vi "LoadImage_Names.vi"(8 "First Image":i32=2098, 9 "Load in PCO Format":bool, 11 "Sample Image":path=path "C:/Analysis_from_Movie_for_RiboTrap_Dieter/Movie_Data_Lorenz/TPA-3rdplasmidconc1to1/tea4s15w_0_003565.tif") -> (0 "Image Filenames":string[](array[string])=["C:\\Analysis_from_Movie_for_RiboTrap_Dieter\\Movie_Data_Lorenz\\TPA-3rdplasmidconc1to1\\tea4s15w_0_002099.tif", "C:\\Analysis_from_Movie_for_RiboTrap_Dieter\\Movie_Data_Lorenz\\TPA-3rdplasmidconc1to1\\tea4s15w_0_002100.tif", "C:\\Analysis_from_Movie_for_RiboTrap_Dieter\\Movie_Data_Lorenz\\TPA-3rdplasmidconc1to1\\tea4s15w_0_002101.tif", "C:\\Analysis_from_Movie_for_RiboTrap_Dieter\\Movie_Data_Lorenz\\TPA-3rdplasmidconc1to1\\tea4s15w_0_002102.tif", "C:\\Analysis_from_Movie_for_RiboTrap_Dieter\\Movie_Data_Lorenz\\TPA-3rdplasmidconc1to1\\tea4s15w_0_002103.tif", "C:\\Analysis_from_Movie_for_RiboTrap_Dieter\\Movie_Data_Lorenz\\TPA-3rdplasmidconc1to1\\tea4s15w_0_002104.tif", "C:\\Analysis_from_Movie_for_RiboTrap_Dieter\\Movie_Data_Lorenz\\TPA-3rdplasmidconc1to1\\tea4s15w_0_002105.tif", "C:\\Analysis_from_Movie_for_RiboTrap_Dieter\\Movie_Data_Lorenz\\TPA-3rdplasmidconc1to1\\tea4s15w_0_002106.tif", "C:\\Analysis_from_Movie_for_RiboTrap_Dieter\\Movie_Data_Lorenz\\TPA-3rdplasmidconc1to1\\tea4s15w_0_002107.tif", "C:\\Analysis_from_Movie_for_RiboTrap_Dieter\\Movie_Data_Lorenz\\TPA-3rdplasmidconc1to1\\tea4s15w_0_002108.tif", "C:\\Analysis_from_Movie_for_RiboTrap_Dieter\\Movie_Data_Lorenz\\TPA-3rdplasmidconc1to1\\tea4s15w_0_002109.tif", "C:\\Analysis_from_Movie_for_RiboTrap_Dieter\\Movie_Data_Lorenz\\TPA-3rdplasmidconc1to1\\tea4s15w_0_002110.tif", "C:\\Analysis_from_Movie_for_RiboTrap_Dieter\\Movie_Data_Lorenz\\TPA-3rdplasmidconc1to1\\tea4s15w_0_002111.tif", "C:\\Analysis_from_Movie_for_RiboTrap_Dieter\\Movie_Data_Lorenz\\TPA-3rdplasmidconc1to1\\tea4s15w_0_002112.tif", "C:\\Analysis_from_Movie_for_RiboTrap_Dieter\\Movie_Data_Lorenz\\TPA-3rdplasmidconc1to1\\tea4s15w_0_002113.tif", "C:\\Analysis_from_Movie_for_RiboTrap_Dieter\\Movie_Data_Lorenz\\TPA-3rdplasmidconc1to1\\tea4s15w_0_002114.tif", "C:\\Analysis_from_Movie_for_RiboTrap_Dieter\\Movie_Data_Lorenz\\TPA-3rdplasmidconc1to1\\tea4s15w_0_002115.tif", "C:\\Analysis_from_Movie_for_RiboTrap_Dieter\\Movie_Data_Lorenz\\TPA-3rdplasmidconc1to1\\tea4s15w_0_002116.tif", "C:\\Analysis_from_Movie_for_RiboTrap_Dieter\\Movie_Data_Lorenz\\TPA-3rdplasmidconc1to1\\tea4s15w_0_002117.tif", "C:\\Analysis_from_Movie_for_RiboTrap_Dieter\\Movie_Data_Lorenz\\TPA-3rdplasmidconc1to1\\tea4s15w_0_002118.tif", "C:\\Analysis_from_Movie_for_RiboTrap_Dieter\\Movie_Data_Lorenz\\TPA-3rdplasmidconc1to1\\tea4s15w_0_002119.tif", "C:\\Analysis_from_Movie_for_RiboTrap_Dieter\\Movie_Data_Lorenz\\TPA-3rdplasmidconc1to1\\tea4s15w_0_002120.tif", "C:\\Analysis_from_Movie_for_RiboTrap_Dieter\\Movie_Data_Lorenz\\TPA-3rdplasmidconc1to1\\tea4s15w_0_002121.tif", "C:\\Analysis_from_Movie_for_RiboTrap_Dieter\\Movie_Data_Lorenz\\TPA-3rdplasmidconc1to1\\tea4s15w_0_002122.tif", "C:\\Analysis_from_Movie_for_RiboTrap_Dieter\\Movie_Data_Lorenz\\TPA-3rdplasmidconc1to1\\tea4s15w_0_002123.tif", "C:\\Analysis_from_Movie_for_RiboTrap_Dieter\\Movie_Data_Lorenz\\TPA-3rdplasmidconc1to1\\tea4s15w_0_002124.tif", "C:\\Analysis_from_Movie_for_RiboTrap_Dieter\\Movie_Data_Lorenz\\TPA-3rdplasmidconc1to1\\tea4s15w_0_002125.tif", "C:\\Analysis_from_Movie_for_RiboTrap_Dieter\\Movie_Data_Lorenz\\TPA-3rdplasmidconc1to1\\tea4s15w_0_002126.tif", "C:\\Analysis_from_Movie_for_RiboTrap_Dieter\\Movie_Data_Lorenz\\TPA-3rdplasmidconc1to1\\tea4s15w_0_002127.tif", "C:\\Analysis_from_Movie_for_RiboTrap_Dieter\\Movie_Data_Lorenz\\TPA-3rdplasmidconc1to1\\tea4s15w_0_002128.tif", "C:\\Analysis_from_Movie_for_RiboTrap_Dieter\\Movie_Data_Lorenz\\TPA-3rdplasmidconc1to1\\tea4s15w_0_002129.tif", "C:\\Analysis_from_Movie_for_RiboTrap_Dieter\\Movie_Data_Lorenz\\TPA-3rdplasmidconc1to1\\tea4s15w_0_002130.tif", "C:\\Analysis_from_Movie_for_RiboTrap_Dieter\\Movie_Data_Lorenz\\TPA-3rdplasmidconc1to1\\tea4s15w_0_002131.tif", "C:\\Analysis_from_Movie_for_RiboTrap_Dieter\\Movie_Data_Lorenz\\TPA-3rdplasmidconc1to1\\tea4s15w_0_002132.tif", "C:\\Analysis_from_Movie_for_RiboTrap_Dieter\\Movie_Data_Lorenz\\TPA-3rdplasmidconc1to1\\tea4s15w_0_002133.tif", "C:\\Analysis_from_Movie_for_RiboTrap_Dieter\\Movie_Data_Lorenz\\TPA-3rdplasmidconc1to1\\tea4s15w_0_002134.tif", "C:\\Analysis_from_Movie_for_RiboTrap_Dieter\\Movie_Data_Lorenz\\TPA-3rdplasmidconc1to1\\tea4s15w_0_002135.tif", "C:\\Analysis_from_Movie_for_RiboTrap_Dieter\\Movie_Data_Lorenz\\TPA-3rdplasmidconc1to1\\tea4s15w_0_002136.tif", "C:\\Analysis_from_Movie_for_RiboTrap_Dieter\\Movie_Data_Lorenz\\TPA-3rdplasmidconc1to1\\tea4s15w_0_002137.tif", "C:\\Analysis_from_Movie_for_RiboTrap_Dieter\\Movie_Data_Lorenz\\TPA-3rdplasmidconc1to1\\tea4s15w_0_002138.tif", "C:\\Analysis_from_Movie_for_RiboTrap_Dieter\\Movie_Data_Lorenz\\TPA-3rdplasmidconc1to1\\tea4s15w_0_002139.tif", "C:\\Analysis_from_Movie_for_RiboTrap_Dieter\\Movie_Data_Lorenz\\TPA-3rdplasmidconc1to1\\tea4s15w_0_002140.tif", "C:\\Analysis_from_Movie_for_RiboTrap_Dieter\\Movie_Data_Lorenz\\TPA-3rdplasmidconc1to1\\tea4s15w_0_002141.tif", "C:\\Analysis_from_Movie_for_RiboTrap_Dieter\\Movie_Data_Lorenz\\TPA-3rdplasmidconc1to1\\tea4s15w_0_002142.tif", "C:\\Analysis_from_Movie_for_RiboTrap_Dieter\\Movie_Data_Lorenz\\TPA-3rdplasmidconc1to1\\tea4s15w_0_002143.tif", "C:\\Analysis_from_Movie_for_RiboTrap_Dieter\\Movie_Data_Lorenz\\TPA-3rdplasmidconc1to1\\tea4s15w_0_002144.tif", "C:\\Analysis_from_Movie_for_RiboTrap_Dieter\\Movie_Data_Lorenz\\TPA-3rdplasmidconc1to1\\tea4s15w_0_002145.tif", "C:\\Analysis_from_Movie_for_RiboTrap_Dieter\\Movie_Data_Lorenz\\TPA-3rdplasmidconc1to1\\tea4s15w_0_002146.tif", "C:\\Analysis_from_Movie_for_RiboTrap_Dieter\\Movie_Data_Lorenz\\TPA-3rdplasmidconc1to1\\tea4s15w_0_002147.tif", "C:\\Analysis_from_Movie_for_RiboTrap_Dieter\\Movie_Data_Lorenz\\TPA-3rdplasmidconc1to1\\tea4s15w_0_002148.tif", "C:\\Analysis_from_Movie_for_RiboTrap_Dieter\\Movie_Data_Lorenz\\TPA-3rdplasmidconc1to1\\tea4s15w_0_002149.tif", "C:\\Analysis_from_Movie_for_RiboTrap_Dieter\\Movie_Data_Lorenz\\TPA-3rdplasmidconc1to1\\tea4s15w_0_002150.tif", "C:\\Analysis_from_Movie_for_RiboTrap_Dieter\\Movie_Data_Lorenz\\TPA-3rdplasmidconc1to1\\tea4s15w_0_002151.tif", "C:\\Analysis_from_Movie_for_RiboTrap_Dieter\\Movie_Data_Lorenz\\TPA-3rdplasmidconc1to1\\tea4s15w_0_002152.tif", "C:\\Analysis_from_Movie_for_RiboTrap_Dieter\\Movie_Data_Lorenz\\TPA-3rdplasmidconc1to1\\tea4s15w_0_002153.tif", "C:\\Analysis_from_Movie_for_RiboTrap_Dieter\\Movie_Data_Lorenz\\TPA-3rdplasmidconc1to1\\tea4s15w_0_002154.tif", "C:\\Analysis_from_Movie_for_RiboTrap_Dieter\\Movie_Data_Lorenz\\TPA-3rdplasmidconc1to1\\tea4s15w_0_002155.tif", "C:\\Analysis_from_Movie_for_RiboTrap_Dieter\\Movie_Data_Lorenz\\TPA-3rdplasmidconc1to1\\tea4s15w_0_002156.tif", "C:\\Analysis_from_Movie_for_RiboTrap_Dieter\\Movie_Data_Lorenz\\TPA-3rdplasmidconc1to1\\tea4s15w_0_002157.tif", "C:\\Analysis_from_Movie_for_RiboTrap_Dieter\\Movie_Data_Lorenz\\TPA-3rdplasmidconc1to1\\tea4s15w_0_002158.tif", "C:\\Analysis_from_Movie_for_RiboTrap_Dieter\\Movie_Data_Lorenz\\TPA-3rdplasmidconc1to1\\tea4s15w_0_002159.tif", "C:\\Analysis_from_Movie_for_RiboTrap_Dieter\\Movie_Data_Lorenz\\TPA-3rdplasmidconc1to1\\tea4s15w_0_002160.tif", "C:\\Analysis_from_Movie_for_RiboTrap_Dieter\\Movie_Data_Lorenz\\TPA-3rdplasmidconc1to1\\tea4s15w_0_002161.tif", "C:\\Analysis_from_Movie_for_RiboTrap_Dieter\\Movie_Data_Lorenz\\TPA-3rdplasmidconc1to1\\tea4s15w_0_002162.tif", "C:\\Analysis_from_Movie_for_RiboTrap_Dieter\\Movie_Data_Lorenz\\TPA-3rdplasmidconc1to1\\tea4s15w_0_002163.tif", "C:\\Analysis_from_Movie_for_RiboTrap_Dieter\\Movie_Data_Lorenz\\TPA-3rdplasmidconc1to1\\tea4s15w_0_002164.tif", "C:\\Analysis_from_Movie_for_RiboTrap_Dieter\\Movie_Data_Lorenz\\TPA-3rdplasmidconc1to1\\tea4s15w_0_002165.tif", "C:\\Analysis_from_Movie_for_RiboTrap_Dieter\\Movie_Data_Lorenz\\TPA-3rdplasmidconc1to1\\tea4s15w_0_002166.tif", "C:\\Analysis_from_Movie_for_RiboTrap_Dieter\\Movie_Data_Lorenz\\TPA-3rdplasmidconc1to1\\tea4s15w_0_002167.tif", "C:\\Analysis_from_Movie_for_RiboTrap_Dieter\\Movie_Data_Lorenz\\TPA-3rdplasmidconc1to1\\tea4s15w_0_002168.tif", "C:\\Analysis_from_Movie_for_RiboTrap_Dieter\\Movie_Data_Lorenz\\TPA-3rdplasmidconc1to1\\tea4s15w_0_002169.tif", "C:\\Analysis_from_Movie_for_RiboTrap_Dieter\\Movie_Data_Lorenz\\TPA-3rdplasmidconc1to1\\tea4s15w_0_002170.tif", "C:\\Analysis_from_Movie_for_RiboTrap_Dieter\\Movie_Data_Lorenz\\TPA-3rdplasmidconc1to1\\tea4s15w_0_002171.tif", "C:\\Analysis_from_Movie_for_RiboTrap_Dieter\\Movie_Data_Lorenz\\TPA-3rdplasmidconc1to1\\tea4s15w_0_002172.tif", "C:\\Analysis_from_Movie_for_RiboTrap_Dieter\\Movie_Data_Lorenz\\TPA-3rdplasmidconc1to1\\tea4s15w_0_002173.tif", "C:\\Analysis_from_Movie_for_RiboTrap_Dieter\\Movie_Data_Lorenz\\TPA-3rdplasmidconc1to1\\tea4s15w_0_002174.tif", "C:\\Analysis_from_Movie_for_RiboTrap_Dieter\\Movie_Data_Lorenz\\TPA-3rdplasmidconc1to1\\tea4s15w_0_002175.tif", "C:\\Analysis_from_Movie_for_RiboTrap_Dieter\\Movie_Data_Lorenz\\TPA-3rdplasmidconc1to1\\tea4s15w_0_002176.tif", "C:\\Analysis_from_Movie_for_RiboTrap_Dieter\\Movie_Data_Lorenz\\TPA-3rdplasmidconc1to1\\tea4s15w_0_002177.tif", "C:\\Analysis_from_Movie_for_RiboTrap_Dieter\\Movie_Data_Lorenz\\TPA-3rdplasmidconc1to1\\tea4s15w_0_002178.tif", "C:\\Analysis_from_Movie_for_RiboTrap_Dieter\\Movie_Data_Lorenz\\TPA-3rdplasmidconc1to1\\tea4s15w_0_002179.tif", "C:\\Analysis_from_Movie_for_RiboTrap_Dieter\\Movie_Data_Lorenz\\TPA-3rdplasmidconc1to1\\tea4s15w_0_002180.tif", "C:\\Analysis_from_Movie_for_RiboTrap_Dieter\\Movie_Data_Lorenz\\TPA-3rdplasmidconc1to1\\tea4s15w_0_002181.tif", "C:\\Analysis_from_Movie_for_RiboTrap_Dieter\\Movie_Data_Lorenz\\TPA-3rdplasmidconc1to1\\tea4s15w_0_002182.tif", "C:\\Analysis_from_Movie_for_RiboTrap_Dieter\\Movie_Data_Lorenz\\TPA-3rdplasmidconc1to1\\tea4s15w_0_002183.tif", "C:\\Analysis_from_Movie_for_RiboTrap_Dieter\\Movie_Data_Lorenz\\TPA-3rdplasmidconc1to1\\tea4s15w_0_002184.tif", "C:\\Analysis_from_Movie_for_RiboTrap_Dieter\\Movie_Data_Lorenz\\TPA-3rdplasmidconc1to1\\tea4s15w_0_002185.tif", "C:\\Analysis_from_Movie_for_RiboTrap_Dieter\\Movie_Data_Lorenz\\TPA-3rdplasmidconc1to1\\tea4s15w_0_002186.tif", "C:\\Analysis_from_Movie_for_RiboTrap_Dieter\\Movie_Data_Lorenz\\TPA-3rdplasmidconc1to1\\tea4s15w_0_002187.tif", "C:\\Analysis_from_Movie_for_RiboTrap_Dieter\\Movie_Data_Lorenz\\TPA-3rdplasmidconc1to1\\tea4s15w_0_002188.tif", "C:\\Analysis_from_Movie_for_RiboTrap_Dieter\\Movie_Data_Lorenz\\TPA-3rdplasmidconc1to1\\tea4s15w_0_002189.tif", "C:\\Analysis_from_Movie_for_RiboTrap_Dieter\\Movie_Data_Lorenz\\TPA-3rdplasmidconc1to1\\tea4s15w_0_002190.tif", "C:\\Analysis_from_Movie_for_RiboTrap_Dieter\\Movie_Data_Lorenz\\TPA-3rdplasmidconc1to1\\tea4s15w_0_002191.tif", "C:\\Analysis_from_Movie_for_RiboTrap_Dieter\\Movie_Data_Lorenz\\TPA-3rdplasmidconc1to1\\tea4s15w_0_002192.tif", "C:\\Analysis_from_Movie_for_RiboTrap_Dieter\\Movie_Data_Lorenz\\TPA-3rdplasmidconc1to1\\tea4s15w_0_002193.tif", "C:\\Analysis_from_Movie_for_RiboTrap_Dieter\\Movie_Data_Lorenz\\TPA-3rdplasmidconc1to1\\tea4s15w_0_002194.tif", "C:\\Analysis_from_Movie_for_RiboTrap_Dieter\\Movie_Data_Lorenz\\TPA-3rdplasmidconc1to1\\tea4s15w_0_002195.tif", "C:\\Analysis_from_Movie_for_RiboTrap_Dieter\\Movie_Data_Lorenz\\TPA-3rdplasmidconc1to1\\tea4s15w_0_002196.tif", "C:\\Analysis_from_Movie_for_RiboTrap_Dieter\\Movie_Data_Lorenz\\TPA-3rdplasmidconc1to1\\tea4s15w_0_002197.tif", "C:\\Analysis_from_Movie_for_RiboTrap_Dieter\\Movie_Data_Lorenz\\TPA-3rdplasmidconc1to1\\tea4s15w_0_002198.tif", "C:\\Analysis_from_Movie_for_RiboTrap_Dieter\\Movie_Data_Lorenz\\TPA-3rdplasmidconc1to1\\tea4s15w_0_002199.tif", "C:\\Analysis_from_Movie_for_RiboTrap_Dieter\\Movie_Data_Lorenz\\TPA-3rdplasmidconc1to1\\tea4s15w_0_002200.tif", "C:\\Analysis_from_Movie_for_RiboTrap_Dieter\\Movie_Data_Lorenz\\TPA-3rdplasmidconc1to1\\tea4s15w_0_002201.tif", "C:\\Analysis_from_Movie_for_RiboTrap_Dieter\\Movie_Data_Lorenz\\TPA-3rdplasmidconc1to1\\tea4s15w_0_002202.tif", "C:\\Analysis_from_Movie_for_RiboTrap_Dieter\\Movie_Data_Lorenz\\TPA-3rdplasmidconc1to1\\tea4s15w_0_002203.tif", "C:\\Analysis_from_Movie_for_RiboTrap_Dieter\\Movie_Data_Lorenz\\TPA-3rdplasmidconc1to1\\tea4s15w_0_002204.tif", "C:\\Analysis_from_Movie_for_RiboTrap_Dieter\\Movie_Data_Lorenz\\TPA-3rdplasmidconc1to1\\tea4s15w_0_002205.tif", "C:\\Analysis_from_Movie_for_RiboTrap_Dieter\\Movie_Data_Lorenz\\TPA-3rdplasmidconc1to1\\tea4s15w_0_002206.tif", "C:\\Analysis_from_Movie_for_RiboTrap_Dieter\\Movie_Data_Lorenz\\TPA-3rdplasmidconc1to1\\tea4s15w_0_002207.tif", "C:\\Analysis_from_Movie_for_RiboTrap_Dieter\\Movie_Data_Lorenz\\TPA-3rdplasmidconc1to1\\tea4s15w_0_002208.tif", "C:\\Analysis_from_Movie_for_RiboTrap_Dieter\\Movie_Data_Lorenz\\TPA-3rdplasmidconc1to1\\tea4s15w_0_002209.tif", "C:\\Analysis_from_Movie_for_RiboTrap_Dieter\\Movie_Data_Lorenz\\TPA-3rdplasmidconc1to1\\tea4s15w_0_002210.tif", "C:\\Analysis_from_Movie_for_RiboTrap_Dieter\\Movie_Data_Lorenz\\TPA-3rdplasmidconc1to1\\tea4s15w_0_002211.tif", "C:\\Analysis_from_Movie_for_RiboTrap_Dieter\\Movie_Data_Lorenz\\TPA-3rdplasmidconc1to1\\tea4s15w_0_002212.tif", "C:\\Analysis_from_Movie_for_RiboTrap_Dieter\\Movie_Data_Lorenz\\TPA-3rdplasmidconc1to1\\tea4s15w_0_002213.tif", "C:\\Analysis_from_Movie_for_RiboTrap_Dieter\\Movie_Data_Lorenz\\TPA-3rdplasmidconc1to1\\tea4s15w_0_002214.tif", "C:\\Analysis_from_Movie_for_RiboTrap_Dieter\\Movie_Data_Lorenz\\TPA-3rdplasmidconc1to1\\tea4s15w_0_002215.tif", "C:\\Analysis_from_Movie_for_RiboTrap_Dieter\\Movie_Data_Lorenz\\TPA-3rdplasmidconc1to1\\tea4s15w_0_002216.tif", "C:\\Analysis_from_Movie_for_RiboTrap_Dieter\\Movie_Data_Lorenz\\TPA-3rdplasmidconc1to1\\tea4s15w_0_002217.tif", "C:\\Analysis_from_Movie_for_RiboTrap_Dieter\\Movie_Data_Lorenz\\TPA-3rdplasmidconc1to1\\tea4s15w_0_002218.tif", "C:\\Analysis_from_Movie_for_RiboTrap_Dieter\\Movie_Data_Lorenz\\TPA-3rdplasmidconc1to1\\tea4s15w_0_002219.tif", "C:\\Analysis_from_Movie_for_RiboTrap_Dieter\\Movie_Data_Lorenz\\TPA-3rdplasmidconc1to1\\tea4s15w_0_002220.tif", "C:\\Analysis_from_Movie_for_RiboTrap_Dieter\\Movie_Data_Lorenz\\TPA-3rdplasmidconc1to1\\tea4s15w_0_002221.tif", "C:\\Analysis_from_Movie_for_RiboTrap_Dieter\\Movie_Data_Lorenz\\TPA-3rdplasmidconc1to1\\tea4s15w_0_002222.tif", "C:\\Analysis_from_Movie_for_RiboTrap_Dieter\\Movie_Data_Lorenz\\TPA-3rdplasmidconc1to1\\tea4s15w_0_002223.tif", "C:\\Analysis_from_Movie_for_RiboTrap_Dieter\\Movie_Data_Lorenz\\TPA-3rdplasmidconc1to1\\tea4s15w_0_002224.tif", "C:\\Analysis_from_Movie_for_RiboTrap_Dieter\\Movie_Data_Lorenz\\TPA-3rdplasmidconc1to1\\tea4s15w_0_002225.tif", "C:\\Analysis_from_Movie_for_RiboTrap_Dieter\\Movie_Data_Lorenz\\TPA-3rdplasmidconc1to1\\tea4s15w_0_002226.tif", "C:\\Analysis_from_Movie_for_RiboTrap_Dieter\\Movie_Data_Lorenz\\TPA-3rdplasmidconc1to1\\tea4s15w_0_002227.tif", "C:\\Analysis_from_Movie_for_RiboTrap_Dieter\\Movie_Data_Lorenz\\TPA-3rdplasmidconc1to1\\tea4s15w_0_002228.tif", "C:\\Analysis_from_Movie_for_RiboTrap_Dieter\\Movie_Data_Lorenz\\TPA-3rdplasmidconc1to1\\tea4s15w_0_002229.tif", "C:\\Analysis_from_Movie_for_RiboTrap_Dieter\\Movie_Data_Lorenz\\TPA-3rdplasmidconc1to1\\tea4s15w_0_002230.tif", "C:\\Analysis_from_Movie_for_RiboTrap_Dieter\\Movie_Data_Lorenz\\TPA-3rdplasmidconc1to1\\tea4s15w_0_002231.tif", "C:\\Analysis_from_Movie_for_RiboTrap_Dieter\\Movie_Data_Lorenz\\TPA-3rdplasmidconc1to1\\tea4s15w_0_002232.tif", "C:\\Analysis_from_Movie_for_RiboTrap_Dieter\\Movie_Data_Lorenz\\TPA-3rdplasmidconc1to1\\tea4s15w_0_002233.tif", "C:\\Analysis_from_Movie_for_RiboTrap_Dieter\\Movie_Data_Lorenz\\TPA-3rdplasmidconc1to1\\tea4s15w_0_002234.tif", "C:\\Analysis_from_Movie_for_RiboTrap_Dieter\\Movie_Data_Lorenz\\TPA-3rdplasmidconc1to1\\tea4s15w_0_002235.tif", "C:\\Analysis_from_Movie_for_RiboTrap_Dieter\\Movie_Data_Lorenz\\TPA-3rdplasmidconc1to1\\tea4s15w_0_002236.tif", "C:\\Analysis_from_Movie_for_RiboTrap_Dieter\\Movie_Data_Lorenz\\TPA-3rdplasmidconc1to1\\tea4s15w_0_002237.tif", "C:\\Analysis_from_Movie_for_RiboTrap_Dieter\\Movie_Data_Lorenz\\TPA-3rdplasmidconc1to1\\tea4s15w_0_002238.tif", "C:\\Analysis_from_Movie_for_RiboTrap_Dieter\\Movie_Data_Lorenz\\TPA-3rdplasmidconc1to1\\tea4s15w_0_002239.tif", "C:\\Analysis_from_Movie_for_RiboTrap_Dieter\\Movie_Data_Lorenz\\TPA-3rdplasmidconc1to1\\tea4s15w_0_002240.tif", "C:\\Analysis_from_Movie_for_RiboTrap_Dieter\\Movie_Data_Lorenz\\TPA-3rdplasmidconc1to1\\tea4s15w_0_002241.tif", "C:\\Analysis_from_Movie_for_RiboTrap_Dieter\\Movie_Data_Lorenz\\TPA-3rdplasmidconc1to1\\tea4s15w_0_002242.tif", "C:\\Analysis_from_Movie_for_RiboTrap_Dieter\\Movie_Data_Lorenz\\TPA-3rdplasmidconc1to1\\tea4s15w_0_002243.tif", "C:\\Analysis_from_Movie_for_RiboTrap_Dieter\\Movie_Data_Lorenz\\TPA-3rdplasmidconc1to1\\tea4s15w_0_002244.tif", "C:\\Analysis_from_Movie_for_RiboTrap_Dieter\\Movie_Data_Lorenz\\TPA-3rdplasmidconc1to1\\tea4s15w_0_002245.tif", "C:\\Analysis_from_Movie_for_RiboTrap_Dieter\\Movie_Data_Lorenz\\TPA-3rdplasmidconc1to1\\tea4s15w_0_002246.tif", "C:\\Analysis_from_Movie_for_RiboTrap_Dieter\\Movie_Data_Lorenz\\TPA-3rdplasmidconc1to1\\tea4s15w_0_002247.tif", "C:\\Analysis_from_Movie_for_RiboTrap_Dieter\\Movie_Data_Lorenz\\TPA-3rdplasmidconc1to1\\tea4s15w_0_002248.tif", "C:\\Analysis_from_Movie_for_RiboTrap_Dieter\\Movie_Data_Lorenz\\TPA-3rdplasmidconc1to1\\tea4s15w_0_002249.tif", "C:\\Analysis_from_Movie_for_RiboTrap_Dieter\\Movie_Data_Lorenz\\TPA-3rdplasmidconc1to1\\tea4s15w_0_002250.tif", "C:\\Analysis_from_Movie_for_RiboTrap_Dieter\\Movie_Data_Lorenz\\TPA-3rdplasmidconc1to1\\tea4s15w_0_002251.tif", "C:\\Analysis_from_Movie_for_RiboTrap_Dieter\\Movie_Data_Lorenz\\TPA-3rdplasmidconc1to1\\tea4s15w_0_002252.tif", "C:\\Analysis_from_Movie_for_RiboTrap_Dieter\\Movie_Data_Lorenz\\TPA-3rdplasmidconc1to1\\tea4s15w_0_002253.tif", "C:\\Analysis_from_Movie_for_RiboTrap_Dieter\\Movie_Data_Lorenz\\TPA-3rdplasmidconc1to1\\tea4s15w_0_002254.tif", "C:\\Analysis_from_Movie_for_RiboTrap_Dieter\\Movie_Data_Lorenz\\TPA-3rdplasmidconc1to1\\tea4s15w_0_002255.tif", "C:\\Analysis_from_Movie_for_RiboTrap_Dieter\\Movie_Data_Lorenz\\TPA-3rdplasmidconc1to1\\tea4s15w_0_002256.tif", "C:\\Analysis_from_Movie_for_RiboTrap_Dieter\\Movie_Data_Lorenz\\TPA-3rdplasmidconc1to1\\tea4s15w_0_002257.tif", "C:\\Analysis_from_Movie_for_RiboTrap_Dieter\\Movie_Data_Lorenz\\TPA-3rdplasmidconc1to1\\tea4s15w_0_002258.tif", "C:\\Analysis_from_Movie_for_RiboTrap_Dieter\\Movie_Data_Lorenz\\TPA-3rdplasmidconc1to1\\tea4s15w_0_002259.tif", "C:\\Analysis_from_Movie_for_RiboTrap_Dieter\\Movie_Data_Lorenz\\TPA-3rdplasmidconc1to1\\tea4s15w_0_002260.tif", "C:\\Analysis_from_Movie_for_RiboTrap_Dieter\\Movie_Data_Lorenz\\TPA-3rdplasmidconc1to1\\tea4s15w_0_002261.tif", "C:\\Analysis_from_Movie_for_RiboTrap_Dieter\\Movie_Data_Lorenz\\TPA-3rdplasmidconc1to1\\tea4s15w_0_002262.tif", "C:\\Analysis_from_Movie_for_RiboTrap_Dieter\\Movie_Data_Lorenz\\TPA-3rdplasmidconc1to1\\tea4s15w_0_002263.tif", "C:\\Analysis_from_Movie_for_RiboTrap_Dieter\\Movie_Data_Lorenz\\TPA-3rdplasmidconc1to1\\tea4s15w_0_002264.tif", "C:\\Analysis_from_Movie_for_RiboTrap_Dieter\\Movie_Data_Lorenz\\TPA-3rdplasmidconc1to1\\tea4s15w_0_002265.tif", "C:\\Analysis_from_Movie_for_RiboTrap_Dieter\\Movie_Data_Lorenz\\TPA-3rdplasmidconc1to1\\tea4s15w_0_002266.tif", "C:\\Analysis_from_Movie_for_RiboTrap_Dieter\\Movie_Data_Lorenz\\TPA-3rdplasmidconc1to1\\tea4s15w_0_002267.tif", "C:\\Analysis_from_Movie_for_RiboTrap_Dieter\\Movie_Data_Lorenz\\TPA-3rdplasmidconc1to1\\tea4s15w_0_002268.tif", "C:\\Analysis_from_Movie_for_RiboTrap_Dieter\\Movie_Data_Lorenz\\TPA-3rdplasmidconc1to1\\tea4s15w_0_002269.tif", "C:\\Analysis_from_Movie_for_RiboTrap_Dieter\\Movie_Data_Lorenz\\TPA-3rdplasmidconc1to1\\tea4s15w_0_002270.tif", "C:\\Analysis_from_Movie_for_RiboTrap_Dieter\\Movie_Data_Lorenz\\TPA-3rdplasmidconc1to1\\tea4s15w_0_002271.tif", "C:\\Analysis_from_Movie_for_RiboTrap_Dieter\\Movie_Data_Lorenz\\TPA-3rdplasmidconc1to1\\tea4s15w_0_002272.tif", "C:\\Analysis_from_Movie_for_RiboTrap_Dieter\\Movie_Data_Lorenz\\TPA-3rdplasmidconc1to1\\tea4s15w_0_002273.tif", "C:\\Analysis_from_Movie_for_RiboTrap_Dieter\\Movie_Data_Lorenz\\TPA-3rdplasmidconc1to1\\tea4s15w_0_002274.tif", "C:\\Analysis_from_Movie_for_RiboTrap_Dieter\\Movie_Data_Lorenz\\TPA-3rdplasmidconc1to1\\tea4s15w_0_002275.tif", "C:\\Analysis_from_Movie_for_RiboTrap_Dieter\\Movie_Data_Lorenz\\TPA-3rdplasmidconc1to1\\tea4s15w_0_002276.tif", "C:\\Analysis_from_Movie_for_RiboTrap_Dieter\\Movie_Data_Lorenz\\TPA-3rdplasmidconc1to1\\tea4s15w_0_002277.tif", "C:\\Analysis_from_Movie_for_RiboTrap_Dieter\\Movie_Data_Lorenz\\TPA-3rdplasmidconc1to1\\tea4s15w_0_002278.tif", "C:\\Analysis_from_Movie_for_RiboTrap_Dieter\\Movie_Data_Lorenz\\TPA-3rdplasmidconc1to1\\tea4s15w_0_002279.tif", "C:\\Analysis_from_Movie_for_RiboTrap_Dieter\\Movie_Data_Lorenz\\TPA-3rdplasmidconc1to1\\tea4s15w_0_002280.tif", "C:\\Analysis_from_Movie_for_RiboTrap_Dieter\\Movie_Data_Lorenz\\TPA-3rdplasmidconc1to1\\tea4s15w_0_002281.tif", "C:\\Analysis_from_Movie_for_RiboTrap_Dieter\\Movie_Data_Lorenz\\TPA-3rdplasmidconc1to1\\tea4s15w_0_002282.tif", "C:\\Analysis_from_Movie_for_RiboTrap_Dieter\\Movie_Data_Lorenz\\TPA-3rdplasmidconc1to1\\tea4s15w_0_002283.tif", "C:\\Analysis_from_Movie_for_RiboTrap_Dieter\\Movie_Data_Lorenz\\TPA-3rdplasmidconc1to1\\tea4s15w_0_002284.tif", "C:\\Analysis_from_Movie_for_RiboTrap_Dieter\\Movie_Data_Lorenz\\TPA-3rdplasmidconc1to1\\tea4s15w_0_002285.tif", "C:\\Analysis_from_Movie_for_RiboTrap_Dieter\\Movie_Data_Lorenz\\TPA-3rdplasmidconc1to1\\tea4s15w_0_002286.tif", "C:\\Analysis_from_Movie_for_RiboTrap_Dieter\\Movie_Data_Lorenz\\TPA-3rdplasmidconc1to1\\tea4s15w_0_002287.tif", "C:\\Analysis_from_Movie_for_RiboTrap_Dieter\\Movie_Data_Lorenz\\TPA-3rdplasmidconc1to1\\tea4s15w_0_002288.tif", "C:\\Analysis_from_Movie_for_RiboTrap_Dieter\\Movie_Data_Lorenz\\TPA-3rdplasmidconc1to1\\tea4s15w_0_002289.tif", "C:\\Analysis_from_Movie_for_RiboTrap_Dieter\\Movie_Data_Lorenz\\TPA-3rdplasmidconc1to1\\tea4s15w_0_002290.tif", "C:\\Analysis_from_Movie_for_RiboTrap_Dieter\\Movie_Data_Lorenz\\TPA-3rdplasmidconc1to1\\tea4s15w_0_002291.tif", "C:\\Analysis_from_Movie_for_RiboTrap_Dieter\\Movie_Data_Lorenz\\TPA-3rdplasmidconc1to1\\tea4s15w_0_002292.tif", "C:\\Analysis_from_Movie_for_RiboTrap_Dieter\\Movie_Data_Lorenz\\TPA-3rdplasmidconc1to1\\tea4s15w_0_002293.tif", "C:\\Analysis_from_Movie_for_RiboTrap_Dieter\\Movie_Data_Lorenz\\TPA-3rdplasmidconc1to1\\tea4s15w_0_002294.tif", "C:\\Analysis_from_Movie_for_RiboTrap_Dieter\\Movie_Data_Lorenz\\TPA-3rdplasmidconc1to1\\tea4s15w_0_002295.tif", "C:\\Analysis_from_Movie_for_RiboTrap_Dieter\\Movie_Data_Lorenz\\TPA-3rdplasmidconc1to1\\tea4s15w_0_002296.tif", "C:\\Analysis_from_Movie_for_RiboTrap_Dieter\\Movie_Data_Lorenz\\TPA-3rdplasmidconc1to1\\tea4s15w_0_002297.tif", "C:\\Analysis_from_Movie_for_RiboTrap_Dieter\\Movie_Data_Lorenz\\TPA-3rdplasmidconc1to1\\tea4s15w_0_002298.tif", "C:\\Analysis_from_Movie_for_RiboTrap_Dieter\\Movie_Data_Lorenz\\TPA-3rdplasmidconc1to1\\tea4s15w_0_002299.tif", "C:\\Analysis_from_Movie_for_RiboTrap_Dieter\\Movie_Data_Lorenz\\TPA-3rdplasmidconc1to1\\tea4s15w_0_002300.tif", "C:\\Analysis_from_Movie_for_RiboTrap_Dieter\\Movie_Data_Lorenz\\TPA-3rdplasmidconc1to1\\tea4s15w_0_002301.tif", "C:\\Analysis_from_Movie_for_RiboTrap_Dieter\\Movie_Data_Lorenz\\TPA-3rdplasmidconc1to1\\tea4s15w_0_002302.tif", "C:\\Analysis_from_Movie_for_RiboTrap_Dieter\\Movie_Data_Lorenz\\TPA-3rdplasmidconc1to1\\tea4s15w_0_002303.tif", "C:\\Analysis_from_Movie_for_RiboTrap_Dieter\\Movie_Data_Lorenz\\TPA-3rdplasmidconc1to1\\tea4s15w_0_002304.tif", "C:\\Analysis_from_Movie_for_RiboTrap_Dieter\\Movie_Data_Lorenz\\TPA-3rdplasmidconc1to1\\tea4s15w_0_002305.tif", "C:\\Analysis_from_Movie_for_RiboTrap_Dieter\\Movie_Data_Lorenz\\TPA-3rdplasmidconc1to1\\tea4s15w_0_002306.tif", "C:\\Analysis_from_Movie_for_RiboTrap_Dieter\\Movie_Data_Lorenz\\TPA-3rdplasmidconc1to1\\tea4s15w_0_002307.tif", "C:\\Analysis_from_Movie_for_RiboTrap_Dieter\\Movie_Data_Lorenz\\TPA-3rdplasmidconc1to1\\tea4s15w_0_002308.tif", "C:\\Analysis_from_Movie_for_RiboTrap_Dieter\\Movie_Data_Lorenz\\TPA-3rdplasmidconc1to1\\tea4s15w_0_002309.tif", "C:\\Analysis_from_Movie_for_RiboTrap_Dieter\\Movie_Data_Lorenz\\TPA-3rdplasmidconc1to1\\tea4s15w_0_002310.tif", "C:\\Analysis_from_Movie_for_RiboTrap_Dieter\\Movie_Data_Lorenz\\TPA-3rdplasmidconc1to1\\tea4s15w_0_002311.tif", "C:\\Analysis_from_Movie_for_RiboTrap_Dieter\\Movie_Data_Lorenz\\TPA-3rdplasmidconc1to1\\tea4s15w_0_002312.tif", "C:\\Analysis_from_Movie_for_RiboTrap_Dieter\\Movie_Data_Lorenz\\TPA-3rdplasmidconc1to1\\tea4s15w_0_002313.tif", "C:\\Analysis_from_Movie_for_RiboTrap_Dieter\\Movie_Data_Lorenz\\TPA-3rdplasmidconc1to1\\tea4s15w_0_002314.tif", "C:\\Analysis_from_Movie_for_RiboTrap_Dieter\\Movie_Data_Lorenz\\TPA-3rdplasmidconc1to1\\tea4s15w_0_002315.tif", "C:\\Analysis_from_Movie_for_RiboTrap_Dieter\\Movie_Data_Lorenz\\TPA-3rdplasmidconc1to1\\tea4s15w_0_002316.tif", "C:\\Analysis_from_Movie_for_RiboTrap_Dieter\\Movie_Data_Lorenz\\TPA-3rdplasmidconc1to1\\tea4s15w_0_002317.tif", "C:\\Analysis_from_Movie_for_RiboTrap_Dieter\\Movie_Data_Lorenz\\TPA-3rdplasmidconc1to1\\tea4s15w_0_002318.tif", "C:\\Analysis_from_Movie_for_RiboTrap_Dieter\\Movie_Data_Lorenz\\TPA-3rdplasmidconc1to1\\tea4s15w_0_002319.tif", "C:\\Analysis_from_Movie_for_RiboTrap_Dieter\\Movie_Data_Lorenz\\TPA-3rdplasmidconc1to1\\tea4s15w_0_002320.tif", "C:\\Analysis_from_Movie_for_RiboTrap_Dieter\\Movie_Data_Lorenz\\TPA-3rdplasmidconc1to1\\tea4s15w_0_002321.tif", "C:\\Analysis_from_Movie_for_RiboTrap_Dieter\\Movie_Data_Lorenz\\TPA-3rdplasmidconc1to1\\tea4s15w_0_002322.tif", "C:\\Analysis_from_Movie_for_RiboTrap_Dieter\\Movie_Data_Lorenz\\TPA-3rdplasmidconc1to1\\tea4s15w_0_002323.tif", "C:\\Analysis_from_Movie_for_RiboTrap_Dieter\\Movie_Data_Lorenz\\TPA-3rdplasmidconc1to1\\tea4s15w_0_002324.tif", "C:\\Analysis_from_Movie_for_RiboTrap_Dieter\\Movie_Data_Lorenz\\TPA-3rdplasmidconc1to1\\tea4s15w_0_002325.tif", "C:\\Analysis_from_Movie_for_RiboTrap_Dieter\\Movie_Data_Lorenz\\TPA-3rdplasmidconc1to1\\tea4s15w_0_002326.tif", "C:\\Analysis_from_Movie_for_RiboTrap_Dieter\\Movie_Data_Lorenz\\TPA-3rdplasmidconc1to1\\tea4s15w_0_002327.tif", "C:\\Analysis_from_Movie_for_RiboTrap_Dieter\\Movie_Data_Lorenz\\TPA-3rdplasmidconc1to1\\tea4s15w_0_002328.tif", "C:\\Analysis_from_Movie_for_RiboTrap_Dieter\\Movie_Data_Lorenz\\TPA-3rdplasmidconc1to1\\tea4s15w_0_002329.tif", "C:\\Analysis_from_Movie_for_RiboTrap_Dieter\\Movie_Data_Lorenz\\TPA-3rdplasmidconc1to1\\tea4s15w_0_002330.tif", "C:\\Analysis_from_Movie_for_RiboTrap_Dieter\\Movie_Data_Lorenz\\TPA-3rdplasmidconc1to1\\tea4s15w_0_002331.tif", "C:\\Analysis_from_Movie_for_RiboTrap_Dieter\\Movie_Data_Lorenz\\TPA-3rdplasmidconc1to1\\tea4s15w_0_002332.tif", "C:\\Analysis_from_Movie_for_RiboTrap_Dieter\\Movie_Data_Lorenz\\TPA-3rdplasmidconc1to1\\tea4s15w_0_002333.tif", "C:\\Analysis_from_Movie_for_RiboTrap_Dieter\\Movie_Data_Lorenz\\TPA-3rdplasmidconc1to1\\tea4s15w_0_002334.tif", "C:\\Analysis_from_Movie_for_RiboTrap_Dieter\\Movie_Data_Lorenz\\TPA-3rdplasmidconc1to1\\tea4s15w_0_002335.tif", "C:\\Analysis_from_Movie_for_RiboTrap_Dieter\\Movie_Data_Lorenz\\TPA-3rdplasmidconc1to1\\tea4s15w_0_002336.tif", "C:\\Analysis_from_Movie_for_RiboTrap_Dieter\\Movie_Data_Lorenz\\TPA-3rdplasmidconc1to1\\tea4s15w_0_002337.tif", "C:\\Analysis_from_Movie_for_RiboTrap_Dieter\\Movie_Data_Lorenz\\TPA-3rdplasmidconc1to1\\tea4s15w_0_002338.tif", "C:\\Analysis_from_Movie_for_RiboTrap_Dieter\\Movie_Data_Lorenz\\TPA-3rdplasmidconc1to1\\tea4s15w_0_002339.tif", "C:\\Analysis_from_Movie_for_RiboTrap_Dieter\\Movie_Data_Lorenz\\TPA-3rdplasmidconc1to1\\tea4s15w_0_002340.tif", "C:\\Analysis_from_Movie_for_RiboTrap_Dieter\\Movie_Data_Lorenz\\TPA-3rdplasmidconc1to1\\tea4s15w_0_002341.tif", "C:\\Analysis_from_Movie_for_RiboTrap_Dieter\\Movie_Data_Lorenz\\TPA-3rdplasmidconc1to1\\tea4s15w_0_002342.tif", "C:\\Analysis_from_Movie_for_RiboTrap_Dieter\\Movie_Data_Lorenz\\TPA-3rdplasmidconc1to1\\tea4s15w_0_002343.tif", "C:\\Analysis_from_Movie_for_RiboTrap_Dieter\\Movie_Data_Lorenz\\TPA-3rdplasmidconc1to1\\tea4s15w_0_002344.tif", "C:\\Analysis_from_Movie_for_RiboTrap_Dieter\\Movie_Data_Lorenz\\TPA-3rdplasmidconc1to1\\tea4s15w_0_002345.tif", "C:\\Analysis_from_Movie_for_RiboTrap_Dieter\\Movie_Data_Lorenz\\TPA-3rdplasmidconc1to1\\tea4s15w_0_002346.tif", "C:\\Analysis_from_Movie_for_RiboTrap_Dieter\\Movie_Data_Lorenz\\TPA-3rdplasmidconc1to1\\tea4s15w_0_002347.tif", "C:\\Analysis_from_Movie_for_RiboTrap_Dieter\\Movie_Data_Lorenz\\TPA-3rdplasmidconc1to1\\tea4s15w_0_002348.tif", "C:\\Analysis_from_Movie_for_RiboTrap_Dieter\\Movie_Data_Lorenz\\TPA-3rdplasmidconc1to1\\tea4s15w_0_002349.tif", "C:\\Analysis_from_Movie_for_RiboTrap_Dieter\\Movie_Data_Lorenz\\TPA-3rdplasmidconc1to1\\tea4s15w_0_002350.tif", "C:\\Analysis_from_Movie_for_RiboTrap_Dieter\\Movie_Data_Lorenz\\TPA-3rdplasmidconc1to1\\tea4s15w_0_002351.tif", "C:\\Analysis_from_Movie_for_RiboTrap_Dieter\\Movie_Data_Lorenz\\TPA-3rdplasmidconc1to1\\tea4s15w_0_002352.tif", "C:\\Analysis_from_Movie_for_RiboTrap_Dieter\\Movie_Data_Lorenz\\TPA-3rdplasmidconc1to1\\tea4s15w_0_002353.tif", "C:\\Analysis_from_Movie_for_RiboTrap_Dieter\\Movie_Data_Lorenz\\TPA-3rdplasmidconc1to1\\tea4s15w_0_002354.tif", "C:\\Analysis_from_Movie_for_RiboTrap_Dieter\\Movie_Data_Lorenz\\TPA-3rdplasmidconc1to1\\tea4s15w_0_002355.tif", "C:\\Analysis_from_Movie_for_RiboTrap_Dieter\\Movie_Data_Lorenz\\TPA-3rdplasmidconc1to1\\tea4s15w_0_002356.tif", "C:\\Analysis_from_Movie_for_RiboTrap_Dieter\\Movie_Data_Lorenz\\TPA-3rdplasmidconc1to1\\tea4s15w_0_002357.tif", "C:\\Analysis_from_Movie_for_RiboTrap_Dieter\\Movie_Data_Lorenz\\TPA-3rdplasmidconc1to1\\tea4s15w_0_002358.tif", "C:\\Analysis_from_Movie_for_RiboTrap_Dieter\\Movie_Data_Lorenz\\TPA-3rdplasmidconc1to1\\tea4s15w_0_002359.tif", "C:\\Analysis_from_Movie_for_RiboTrap_Dieter\\Movie_Data_Lorenz\\TPA-3rdplasmidconc1to1\\tea4s15w_0_002360.tif", "C:\\Analysis_from_Movie_for_RiboTrap_Dieter\\Movie_Data_Lorenz\\TPA-3rdplasmidconc1to1\\tea4s15w_0_002361.tif", "C:\\Analysis_from_Movie_for_RiboTrap_Dieter\\Movie_Data_Lorenz\\TPA-3rdplasmidconc1to1\\tea4s15w_0_002362.tif", "C:\\Analysis_from_Movie_for_RiboTrap_Dieter\\Movie_Data_Lorenz\\TPA-3rdplasmidconc1to1\\tea4s15w_0_002363.tif", "C:\\Analysis_from_Movie_for_RiboTrap_Dieter\\Movie_Data_Lorenz\\TPA-3rdplasmidconc1to1\\tea4s15w_0_002364.tif", "C:\\Analysis_from_Movie_for_RiboTrap_Dieter\\Movie_Data_Lorenz\\TPA-3rdplasmidconc1to1\\tea4s15w_0_002365.tif", "C:\\Analysis_from_Movie_for_RiboTrap_Dieter\\Movie_Data_Lorenz\\TPA-3rdplasmidconc1to1\\tea4s15w_0_002366.tif", "C:\\Analysis_from_Movie_for_RiboTrap_Dieter\\Movie_Data_Lorenz\\TPA-3rdplasmidconc1to1\\tea4s15w_0_002367.tif", "C:\\Analysis_from_Movie_for_RiboTrap_Dieter\\Movie_Data_Lorenz\\TPA-3rdplasmidconc1to1\\tea4s15w_0_002368.tif", "C:\\Analysis_from_Movie_for_RiboTrap_Dieter\\Movie_Data_Lorenz\\TPA-3rdplasmidconc1to1\\tea4s15w_0_002369.tif", "C:\\Analysis_from_Movie_for_RiboTrap_Dieter\\Movie_Data_Lorenz\\TPA-3rdplasmidconc1to1\\tea4s15w_0_002370.tif", "C:\\Analysis_from_Movie_for_RiboTrap_Dieter\\Movie_Data_Lorenz\\TPA-3rdplasmidconc1to1\\tea4s15w_0_002371.tif", "C:\\Analysis_from_Movie_for_RiboTrap_Dieter\\Movie_Data_Lorenz\\TPA-3rdplasmidconc1to1\\tea4s15w_0_002372.tif", "C:\\Analysis_from_Movie_for_RiboTrap_Dieter\\Movie_Data_Lorenz\\TPA-3rdplasmidconc1to1\\tea4s15w_0_002373.tif", "C:\\Analysis_from_Movie_for_RiboTrap_Dieter\\Movie_Data_Lorenz\\TPA-3rdplasmidconc1to1\\tea4s15w_0_002374.tif", "C:\\Analysis_from_Movie_for_RiboTrap_Dieter\\Movie_Data_Lorenz\\TPA-3rdplasmidconc1to1\\tea4s15w_0_002375.tif", "C:\\Analysis_from_Movie_for_RiboTrap_Dieter\\Movie_Data_Lorenz\\TPA-3rdplasmidconc1to1\\tea4s15w_0_002376.tif", "C:\\Analysis_from_Movie_for_RiboTrap_Dieter\\Movie_Data_Lorenz\\TPA-3rdplasmidconc1to1\\tea4s15w_0_002377.tif", "C:\\Analysis_from_Movie_for_RiboTrap_Dieter\\Movie_Data_Lorenz\\TPA-3rdplasmidconc1to1\\tea4s15w_0_002378.tif", "C:\\Analysis_from_Movie_for_RiboTrap_Dieter\\Movie_Data_Lorenz\\TPA-3rdplasmidconc1to1\\tea4s15w_0_002379.tif", "C:\\Analysis_from_Movie_for_RiboTrap_Dieter\\Movie_Data_Lorenz\\TPA-3rdplasmidconc1to1\\tea4s15w_0_002380.tif", "C:\\Analysis_from_Movie_for_RiboTrap_Dieter\\Movie_Data_Lorenz\\TPA-3rdplasmidconc1to1\\tea4s15w_0_002381.tif", "C:\\Analysis_from_Movie_for_RiboTrap_Dieter\\Movie_Data_Lorenz\\TPA-3rdplasmidconc1to1\\tea4s15w_0_002382.tif", "C:\\Analysis_from_Movie_for_RiboTrap_Dieter\\Movie_Data_Lorenz\\TPA-3rdplasmidconc1to1\\tea4s15w_0_002383.tif", "C:\\Analysis_from_Movie_for_RiboTrap_Dieter\\Movie_Data_Lorenz\\TPA-3rdplasmidconc1to1\\tea4s15w_0_002384.tif", "C:\\Analysis_from_Movie_for_RiboTrap_Dieter\\Movie_Data_Lorenz\\TPA-3rdplasmidconc1to1\\tea4s15w_0_002385.tif", "C:\\Analysis_from_Movie_for_RiboTrap_Dieter\\Movie_Data_Lorenz\\TPA-3rdplasmidconc1to1\\tea4s15w_0_002386.tif", "C:\\Analysis_from_Movie_for_RiboTrap_Dieter\\Movie_Data_Lorenz\\TPA-3rdplasmidconc1to1\\tea4s15w_0_002387.tif", "C:\\Analysis_from_Movie_for_RiboTrap_Dieter\\Movie_Data_Lorenz\\TPA-3rdplasmidconc1to1\\tea4s15w_0_002388.tif", "C:\\Analysis_from_Movie_for_RiboTrap_Dieter\\Movie_Data_Lorenz\\TPA-3rdplasmidconc1to1\\tea4s15w_0_002389.tif", "C:\\Analysis_from_Movie_for_RiboTrap_Dieter\\Movie_Data_Lorenz\\TPA-3rdplasmidconc1to1\\tea4s15w_0_002390.tif", "C:\\Analysis_from_Movie_for_RiboTrap_Dieter\\Movie_Data_Lorenz\\TPA-3rdplasmidconc1to1\\tea4s15w_0_002391.tif", "C:\\Analysis_from_Movie_for_RiboTrap_Dieter\\Movie_Data_Lorenz\\TPA-3rdplasmidconc1to1\\tea4s15w_0_002392.tif", "C:\\Analysis_from_Movie_for_RiboTrap_Dieter\\Movie_Data_Lorenz\\TPA-3rdplasmidconc1to1\\tea4s15w_0_002393.tif", "C:\\Analysis_from_Movie_for_RiboTrap_Dieter\\Movie_Data_Lorenz\\TPA-3rdplasmidconc1to1\\tea4s15w_0_002394.tif", "C:\\Analysis_from_Movie_for_RiboTrap_Dieter\\Movie_Data_Lorenz\\TPA-3rdplasmidconc1to1\\tea4s15w_0_002395.tif", "C:\\Analysis_from_Movie_for_RiboTrap_Dieter\\Movie_Data_Lorenz\\TPA-3rdplasmidconc1to1\\tea4s15w_0_002396.tif", "C:\\Analysis_from_Movie_for_RiboTrap_Dieter\\Movie_Data_Lorenz\\TPA-3rdplasmidconc1to1\\tea4s15w_0_002397.tif", "C:\\Analysis_from_Movie_for_RiboTrap_Dieter\\Movie_Data_Lorenz\\TPA-3rdplasmidconc1to1\\tea4s15w_0_002398.tif", "C:\\Analysis_from_Movie_for_RiboTrap_Dieter\\Movie_Data_Lorenz\\TPA-3rdplasmidconc1to1\\tea4s15w_0_002399.tif", "C:\\Analysis_from_Movie_for_RiboTrap_Dieter\\Movie_Data_Lorenz\\TPA-3rdplasmidconc1to1\\tea4s15w_0_002400.tif", "C:\\Analysis_from_Movie_for_RiboTrap_Dieter\\Movie_Data_Lorenz\\TPA-3rdplasmidconc1to1\\tea4s15w_0_002401.tif", "C:\\Analysis_from_Movie_for_RiboTrap_Dieter\\Movie_Data_Lorenz\\TPA-3rdplasmidconc1to1\\tea4s15w_0_002402.tif", "C:\\Analysis_from_Movie_for_RiboTrap_Dieter\\Movie_Data_Lorenz\\TPA-3rdplasmidconc1to1\\tea4s15w_0_002403.tif", "C:\\Analysis_from_Movie_for_RiboTrap_Dieter\\Movie_Data_Lorenz\\TPA-3rdplasmidconc1to1\\tea4s15w_0_002404.tif", "C:\\Analysis_from_Movie_for_RiboTrap_Dieter\\Movie_Data_Lorenz\\TPA-3rdplasmidconc1to1\\tea4s15w_0_002405.tif", "C:\\Analysis_from_Movie_for_RiboTrap_Dieter\\Movie_Data_Lorenz\\TPA-3rdplasmidconc1to1\\tea4s15w_0_002406.tif", "C:\\Analysis_from_Movie_for_RiboTrap_Dieter\\Movie_Data_Lorenz\\TPA-3rdplasmidconc1to1\\tea4s15w_0_002407.tif", "C:\\Analysis_from_Movie_for_RiboTrap_Dieter\\Movie_Data_Lorenz\\TPA-3rdplasmidconc1to1\\tea4s15w_0_002408.tif", "C:\\Analysis_from_Movie_for_RiboTrap_Dieter\\Movie_Data_Lorenz\\TPA-3rdplasmidconc1to1\\tea4s15w_0_002409.tif", "C:\\Analysis_from_Movie_for_RiboTrap_Dieter\\Movie_Data_Lorenz\\TPA-3rdplasmidconc1to1\\tea4s15w_0_002410.tif", "C:\\Analysis_from_Movie_for_RiboTrap_Dieter\\Movie_Data_Lorenz\\TPA-3rdplasmidconc1to1\\tea4s15w_0_002411.tif", "C:\\Analysis_from_Movie_for_RiboTrap_Dieter\\Movie_Data_Lorenz\\TPA-3rdplasmidconc1to1\\tea4s15w_0_002412.tif", "C:\\Analysis_from_Movie_for_RiboTrap_Dieter\\Movie_Data_Lorenz\\TPA-3rdplasmidconc1to1\\tea4s15w_0_002413.tif", "C:\\Analysis_from_Movie_for_RiboTrap_Dieter\\Movie_Data_Lorenz\\TPA-3rdplasmidconc1to1\\tea4s15w_0_002414.tif", "C:\\Analysis_from_Movie_for_RiboTrap_Dieter\\Movie_Data_Lorenz\\TPA-3rdplasmidconc1to1\\tea4s15w_0_002415.tif", "C:\\Analysis_from_Movie_for_RiboTrap_Dieter\\Movie_Data_Lorenz\\TPA-3rdplasmidconc1to1\\tea4s15w_0_002416.tif", "C:\\Analysis_from_Movie_for_RiboTrap_Dieter\\Movie_Data_Lorenz\\TPA-3rdplasmidconc1to1\\tea4s15w_0_002417.tif", "C:\\Analysis_from_Movie_for_RiboTrap_Dieter\\Movie_Data_Lorenz\\TPA-3rdplasmidconc1to1\\tea4s15w_0_002418.tif", "C:\\Analysis_from_Movie_for_RiboTrap_Dieter\\Movie_Data_Lorenz\\TPA-3rdplasmidconc1to1\\tea4s15w_0_002419.tif", "C:\\Analysis_from_Movie_for_RiboTrap_Dieter\\Movie_Data_Lorenz\\TPA-3rdplasmidconc1to1\\tea4s15w_0_002420.tif", "C:\\Analysis_from_Movie_for_RiboTrap_Dieter\\Movie_Data_Lorenz\\TPA-3rdplasmidconc1to1\\tea4s15w_0_002421.tif", "C:\\Analysis_from_Movie_for_RiboTrap_Dieter\\Movie_Data_Lorenz\\TPA-3rdplasmidconc1to1\\tea4s15w_0_002422.tif", "C:\\Analysis_from_Movie_for_RiboTrap_Dieter\\Movie_Data_Lorenz\\TPA-3rdplasmidconc1to1\\tea4s15w_0_002423.tif", "C:\\Analysis_from_Movie_for_RiboTrap_Dieter\\Movie_Data_Lorenz\\TPA-3rdplasmidconc1to1\\tea4s15w_0_002424.tif", "C:\\Analysis_from_Movie_for_RiboTrap_Dieter\\Movie_Data_Lorenz\\TPA-3rdplasmidconc1to1\\tea4s15w_0_002425.tif", "C:\\Analysis_from_Movie_for_RiboTrap_Dieter\\Movie_Data_Lorenz\\TPA-3rdplasmidconc1to1\\tea4s15w_0_002426.tif", "C:\\Analysis_from_Movie_for_RiboTrap_Dieter\\Movie_Data_Lorenz\\TPA-3rdplasmidconc1to1\\tea4s15w_0_002427.tif", "C:\\Analysis_from_Movie_for_RiboTrap_Dieter\\Movie_Data_Lorenz\\TPA-3rdplasmidconc1to1\\tea4s15w_0_002428.tif", "C:\\Analysis_from_Movie_for_RiboTrap_Dieter\\Movie_Data_Lorenz\\TPA-3rdplasmidconc1to1\\tea4s15w_0_002429.tif", "C:\\Analysis_from_Movie_for_RiboTrap_Dieter\\Movie_Data_Lorenz\\TPA-3rdplasmidconc1to1\\tea4s15w_0_002430.tif", "C:\\Analysis_from_Movie_for_RiboTrap_Dieter\\Movie_Data_Lorenz\\TPA-3rdplasmidconc1to1\\tea4s15w_0_002431.tif", "C:\\Analysis_from_Movie_for_RiboTrap_Dieter\\Movie_Data_Lorenz\\TPA-3rdplasmidconc1to1\\tea4s15w_0_002432.tif", "C:\\Analysis_from_Movie_for_RiboTrap_Dieter\\Movie_Data_Lorenz\\TPA-3rdplasmidconc1to1\\tea4s15w_0_002433.tif", "C:\\Analysis_from_Movie_for_RiboTrap_Dieter\\Movie_Data_Lorenz\\TPA-3rdplasmidconc1to1\\tea4s15w_0_002434.tif", "C:\\Analysis_from_Movie_for_RiboTrap_Dieter\\Movie_Data_Lorenz\\TPA-3rdplasmidconc1to1\\tea4s15w_0_002435.tif", "C:\\Analysis_from_Movie_for_RiboTrap_Dieter\\Movie_Data_Lorenz\\TPA-3rdplasmidconc1to1\\tea4s15w_0_002436.tif", "C:\\Analysis_from_Movie_for_RiboTrap_Dieter\\Movie_Data_Lorenz\\TPA-3rdplasmidconc1to1\\tea4s15w_0_002437.tif", "C:\\Analysis_from_Movie_for_RiboTrap_Dieter\\Movie_Data_Lorenz\\TPA-3rdplasmidconc1to1\\tea4s15w_0_002438.tif", "C:\\Analysis_from_Movie_for_RiboTrap_Dieter\\Movie_Data_Lorenz\\TPA-3rdplasmidconc1to1\\tea4s15w_0_002439.tif", "C:\\Analysis_from_Movie_for_RiboTrap_Dieter\\Movie_Data_Lorenz\\TPA-3rdplasmidconc1to1\\tea4s15w_0_002440.tif", "C:\\Analysis_from_Movie_for_RiboTrap_Dieter\\Movie_Data_Lorenz\\TPA-3rdplasmidconc1to1\\tea4s15w_0_002441.tif", "C:\\Analysis_from_Movie_for_RiboTrap_Dieter\\Movie_Data_Lorenz\\TPA-3rdplasmidconc1to1\\tea4s15w_0_002442.tif", "C:\\Analysis_from_Movie_for_RiboTrap_Dieter\\Movie_Data_Lorenz\\TPA-3rdplasmidconc1to1\\tea4s15w_0_002443.tif", "C:\\Analysis_from_Movie_for_RiboTrap_Dieter\\Movie_Data_Lorenz\\TPA-3rdplasmidconc1to1\\tea4s15w_0_002444.tif", "C:\\Analysis_from_Movie_for_RiboTrap_Dieter\\Movie_Data_Lorenz\\TPA-3rdplasmidconc1to1\\tea4s15w_0_002445.tif", "C:\\Analysis_from_Movie_for_RiboTrap_Dieter\\Movie_Data_Lorenz\\TPA-3rdplasmidconc1to1\\tea4s15w_0_002446.tif", "C:\\Analysis_from_Movie_for_RiboTrap_Dieter\\Movie_Data_Lorenz\\TPA-3rdplasmidconc1to1\\tea4s15w_0_002447.tif", "C:\\Analysis_from_Movie_for_RiboTrap_Dieter\\Movie_Data_Lorenz\\TPA-3rdplasmidconc1to1\\tea4s15w_0_002448.tif", "C:\\Analysis_from_Movie_for_RiboTrap_Dieter\\Movie_Data_Lorenz\\TPA-3rdplasmidconc1to1\\tea4s15w_0_002449.tif", "C:\\Analysis_from_Movie_for_RiboTrap_Dieter\\Movie_Data_Lorenz\\TPA-3rdplasmidconc1to1\\tea4s15w_0_002450.tif", "C:\\Analysis_from_Movie_for_RiboTrap_Dieter\\Movie_Data_Lorenz\\TPA-3rdplasmidconc1to1\\tea4s15w_0_002451.tif", "C:\\Analysis_from_Movie_for_RiboTrap_Dieter\\Movie_Data_Lorenz\\TPA-3rdplasmidconc1to1\\tea4s15w_0_002452.tif", "C:\\Analysis_from_Movie_for_RiboTrap_Dieter\\Movie_Data_Lorenz\\TPA-3rdplasmidconc1to1\\tea4s15w_0_002453.tif", "C:\\Analysis_from_Movie_for_RiboTrap_Dieter\\Movie_Data_Lorenz\\TPA-3rdplasmidconc1to1\\tea4s15w_0_002454.tif", "C:\\Analysis_from_Movie_for_RiboTrap_Dieter\\Movie_Data_Lorenz\\TPA-3rdplasmidconc1to1\\tea4s15w_0_002455.tif", "C:\\Analysis_from_Movie_for_RiboTrap_Dieter\\Movie_Data_Lorenz\\TPA-3rdplasmidconc1to1\\tea4s15w_0_002456.tif", "C:\\Analysis_from_Movie_for_RiboTrap_Dieter\\Movie_Data_Lorenz\\TPA-3rdplasmidconc1to1\\tea4s15w_0_002457.tif", "C:\\Analysis_from_Movie_for_RiboTrap_Dieter\\Movie_Data_Lorenz\\TPA-3rdplasmidconc1to1\\tea4s15w_0_002458.tif", "C:\\Analysis_from_Movie_for_RiboTrap_Dieter\\Movie_Data_Lorenz\\TPA-3rdplasmidconc1to1\\tea4s15w_0_002459.tif", "C:\\Analysis_from_Movie_for_RiboTrap_Dieter\\Movie_Data_Lorenz\\TPA-3rdplasmidconc1to1\\tea4s15w_0_002460.tif", "C:\\Analysis_from_Movie_for_RiboTrap_Dieter\\Movie_Data_Lorenz\\TPA-3rdplasmidconc1to1\\tea4s15w_0_002461.tif", "C:\\Analysis_from_Movie_for_RiboTrap_Dieter\\Movie_Data_Lorenz\\TPA-3rdplasmidconc1to1\\tea4s15w_0_002462.tif", "C:\\Analysis_from_Movie_for_RiboTrap_Dieter\\Movie_Data_Lorenz\\TPA-3rdplasmidconc1to1\\tea4s15w_0_002463.tif", "C:\\Analysis_from_Movie_for_RiboTrap_Dieter\\Movie_Data_Lorenz\\TPA-3rdplasmidconc1to1\\tea4s15w_0_002464.tif", "C:\\Analysis_from_Movie_for_RiboTrap_Dieter\\Movie_Data_Lorenz\\TPA-3rdplasmidconc1to1\\tea4s15w_0_002465.tif", "C:\\Analysis_from_Movie_for_RiboTrap_Dieter\\Movie_Data_Lorenz\\TPA-3rdplasmidconc1to1\\tea4s15w_0_002466.tif", "C:\\Analysis_from_Movie_for_RiboTrap_Dieter\\Movie_Data_Lorenz\\TPA-3rdplasmidconc1to1\\tea4s15w_0_002467.tif", "C:\\Analysis_from_Movie_for_RiboTrap_Dieter\\Movie_Data_Lorenz\\TPA-3rdplasmidconc1to1\\tea4s15w_0_002468.tif", "C:\\Analysis_from_Movie_for_RiboTrap_Dieter\\Movie_Data_Lorenz\\TPA-3rdplasmidconc1to1\\tea4s15w_0_002469.tif", "C:\\Analysis_from_Movie_for_RiboTrap_Dieter\\Movie_Data_Lorenz\\TPA-3rdplasmidconc1to1\\tea4s15w_0_002470.tif", "C:\\Analysis_from_Movie_for_RiboTrap_Dieter\\Movie_Data_Lorenz\\TPA-3rdplasmidconc1to1\\tea4s15w_0_002471.tif", "C:\\Analysis_from_Movie_for_RiboTrap_Dieter\\Movie_Data_Lorenz\\TPA-3rdplasmidconc1to1\\tea4s15w_0_002472.tif", "C:\\Analysis_from_Movie_for_RiboTrap_Dieter\\Movie_Data_Lorenz\\TPA-3rdplasmidconc1to1\\tea4s15w_0_002473.tif", "C:\\Analysis_from_Movie_for_RiboTrap_Dieter\\Movie_Data_Lorenz\\TPA-3rdplasmidconc1to1\\tea4s15w_0_002474.tif", "C:\\Analysis_from_Movie_for_RiboTrap_Dieter\\Movie_Data_Lorenz\\TPA-3rdplasmidconc1to1\\tea4s15w_0_002475.tif", "C:\\Analysis_from_Movie_for_RiboTrap_Dieter\\Movie_Data_Lorenz\\TPA-3rdplasmidconc1to1\\tea4s15w_0_002476.tif", "C:\\Analysis_from_Movie_for_RiboTrap_Dieter\\Movie_Data_Lorenz\\TPA-3rdplasmidconc1to1\\tea4s15w_0_002477.tif", "C:\\Analysis_from_Movie_for_RiboTrap_Dieter\\Movie_Data_Lorenz\\TPA-3rdplasmidconc1to1\\tea4s15w_0_002478.tif", "C:\\Analysis_from_Movie_for_RiboTrap_Dieter\\Movie_Data_Lorenz\\TPA-3rdplasmidconc1to1\\tea4s15w_0_002479.tif", "C:\\Analysis_from_Movie_for_RiboTrap_Dieter\\Movie_Data_Lorenz\\TPA-3rdplasmidconc1to1\\tea4s15w_0_002480.tif", "C:\\Analysis_from_Movie_for_RiboTrap_Dieter\\Movie_Data_Lorenz\\TPA-3rdplasmidconc1to1\\tea4s15w_0_002481.tif", "C:\\Analysis_from_Movie_for_RiboTrap_Dieter\\Movie_Data_Lorenz\\TPA-3rdplasmidconc1to1\\tea4s15w_0_002482.tif", "C:\\Analysis_from_Movie_for_RiboTrap_Dieter\\Movie_Data_Lorenz\\TPA-3rdplasmidconc1to1\\tea4s15w_0_002483.tif", "C:\\Analysis_from_Movie_for_RiboTrap_Dieter\\Movie_Data_Lorenz\\TPA-3rdplasmidconc1to1\\tea4s15w_0_002484.tif", "C:\\Analysis_from_Movie_for_RiboTrap_Dieter\\Movie_Data_Lorenz\\TPA-3rdplasmidconc1to1\\tea4s15w_0_002485.tif", "C:\\Analysis_from_Movie_for_RiboTrap_Dieter\\Movie_Data_Lorenz\\TPA-3rdplasmidconc1to1\\tea4s15w_0_002486.tif", "C:\\Analysis_from_Movie_for_RiboTrap_Dieter\\Movie_Data_Lorenz\\TPA-3rdplasmidconc1to1\\tea4s15w_0_002487.tif", "C:\\Analysis_from_Movie_for_RiboTrap_Dieter\\Movie_Data_Lorenz\\TPA-3rdplasmidconc1to1\\tea4s15w_0_002488.tif", "C:\\Analysis_from_Movie_for_RiboTrap_Dieter\\Movie_Data_Lorenz\\TPA-3rdplasmidconc1to1\\tea4s15w_0_002489.tif", "C:\\Analysis_from_Movie_for_RiboTrap_Dieter\\Movie_Data_Lorenz\\TPA-3rdplasmidconc1to1\\tea4s15w_0_002490.tif", "C:\\Analysis_from_Movie_for_RiboTrap_Dieter\\Movie_Data_Lorenz\\TPA-3rdplasmidconc1to1\\tea4s15w_0_002491.tif", "C:\\Analysis_from_Movie_for_RiboTrap_Dieter\\Movie_Data_Lorenz\\TPA-3rdplasmidconc1to1\\tea4s15w_0_002492.tif", "C:\\Analysis_from_Movie_for_RiboTrap_Dieter\\Movie_Data_Lorenz\\TPA-3rdplasmidconc1to1\\tea4s15w_0_002493.tif", "C:\\Analysis_from_Movie_for_RiboTrap_Dieter\\Movie_Data_Lorenz\\TPA-3rdplasmidconc1to1\\tea4s15w_0_002494.tif", "C:\\Analysis_from_Movie_for_RiboTrap_Dieter\\Movie_Data_Lorenz\\TPA-3rdplasmidconc1to1\\tea4s15w_0_002495.tif", "C:\\Analysis_from_Movie_for_RiboTrap_Dieter\\Movie_Data_Lorenz\\TPA-3rdplasmidconc1to1\\tea4s15w_0_002496.tif", "C:\\Analysis_from_Movie_for_RiboTrap_Dieter\\Movie_Data_Lorenz\\TPA-3rdplasmidconc1to1\\tea4s15w_0_002497.tif", "C:\\Analysis_from_Movie_for_RiboTrap_Dieter\\Movie_Data_Lorenz\\TPA-3rdplasmidconc1to1\\tea4s15w_0_002498.tif", "C:\\Analysis_from_Movie_for_RiboTrap_Dieter\\Movie_Data_Lorenz\\TPA-3rdplasmidconc1to1\\tea4s15w_0_002499.tif", "C:\\Analysis_from_Movie_for_RiboTrap_Dieter\\Movie_Data_Lorenz\\TPA-3rdplasmidconc1to1\\tea4s15w_0_002500.tif", "C:\\Analysis_from_Movie_for_RiboTrap_Dieter\\Movie_Data_Lorenz\\TPA-3rdplasmidconc1to1\\tea4s15w_0_002501.tif", "C:\\Analysis_from_Movie_for_RiboTrap_Dieter\\Movie_Data_Lorenz\\TPA-3rdplasmidconc1to1\\tea4s15w_0_002502.tif", "C:\\Analysis_from_Movie_for_RiboTrap_Dieter\\Movie_Data_Lorenz\\TPA-3rdplasmidconc1to1\\tea4s15w_0_002503.tif", "C:\\Analysis_from_Movie_for_RiboTrap_Dieter\\Movie_Data_Lorenz\\TPA-3rdplasmidconc1to1\\tea4s15w_0_002504.tif", "C:\\Analysis_from_Movie_for_RiboTrap_Dieter\\Movie_Data_Lorenz\\TPA-3rdplasmidconc1to1\\tea4s15w_0_002505.tif", "C:\\Analysis_from_Movie_for_RiboTrap_Dieter\\Movie_Data_Lorenz\\TPA-3rdplasmidconc1to1\\tea4s15w_0_002506.tif", "C:\\Analysis_from_Movie_for_RiboTrap_Dieter\\Movie_Data_Lorenz\\TPA-3rdplasmidconc1to1\\tea4s15w_0_002507.tif", "C:\\Analysis_from_Movie_for_RiboTrap_Dieter\\Movie_Data_Lorenz\\TPA-3rdplasmidconc1to1\\tea4s15w_0_002508.tif", "C:\\Analysis_from_Movie_for_RiboTrap_Dieter\\Movie_Data_Lorenz\\TPA-3rdplasmidconc1to1\\tea4s15w_0_002509.tif", "C:\\Analysis_from_Movie_for_RiboTrap_Dieter\\Movie_Data_Lorenz\\TPA-3rdplasmidconc1to1\\tea4s15w_0_002510.tif", "C:\\Analysis_from_Movie_for_RiboTrap_Dieter\\Movie_Data_Lorenz\\TPA-3rdplasmidconc1to1\\tea4s15w_0_002511.tif", "C:\\Analysis_from_Movie_for_RiboTrap_Dieter\\Movie_Data_Lorenz\\TPA-3rdplasmidconc1to1\\tea4s15w_0_002512.tif", "C:\\Analysis_from_Movie_for_RiboTrap_Dieter\\Movie_Data_Lorenz\\TPA-3rdplasmidconc1to1\\tea4s15w_0_002513.tif", "C:\\Analysis_from_Movie_for_RiboTrap_Dieter\\Movie_Data_Lorenz\\TPA-3rdplasmidconc1to1\\tea4s15w_0_002514.tif", "C:\\Analysis_from_Movie_for_RiboTrap_Dieter\\Movie_Data_Lorenz\\TPA-3rdplasmidconc1to1\\tea4s15w_0_002515.tif", "C:\\Analysis_from_Movie_for_RiboTrap_Dieter\\Movie_Data_Lorenz\\TPA-3rdplasmidconc1to1\\tea4s15w_0_002516.tif", "C:\\Analysis_from_Movie_for_RiboTrap_Dieter\\Movie_Data_Lorenz\\TPA-3rdplasmidconc1to1\\tea4s15w_0_002517.tif", "C:\\Analysis_from_Movie_for_RiboTrap_Dieter\\Movie_Data_Lorenz\\TPA-3rdplasmidconc1to1\\tea4s15w_0_002518.tif", "C:\\Analysis_from_Movie_for_RiboTrap_Dieter\\Movie_Data_Lorenz\\TPA-3rdplasmidconc1to1\\tea4s15w_0_002519.tif", "C:\\Analysis_from_Movie_for_RiboTrap_Dieter\\Movie_Data_Lorenz\\TPA-3rdplasmidconc1to1\\tea4s15w_0_002520.tif", "C:\\Analysis_from_Movie_for_RiboTrap_Dieter\\Movie_Data_Lorenz\\TPA-3rdplasmidconc1to1\\tea4s15w_0_002521.tif", "C:\\Analysis_from_Movie_for_RiboTrap_Dieter\\Movie_Data_Lorenz\\TPA-3rdplasmidconc1to1\\tea4s15w_0_002522.tif", "C:\\Analysis_from_Movie_for_RiboTrap_Dieter\\Movie_Data_Lorenz\\TPA-3rdplasmidconc1to1\\tea4s15w_0_002523.tif", "C:\\Analysis_from_Movie_for_RiboTrap_Dieter\\Movie_Data_Lorenz\\TPA-3rdplasmidconc1to1\\tea4s15w_0_002524.tif", "C:\\Analysis_from_Movie_for_RiboTrap_Dieter\\Movie_Data_Lorenz\\TPA-3rdplasmidconc1to1\\tea4s15w_0_002525.tif", "C:\\Analysis_from_Movie_for_RiboTrap_Dieter\\Movie_Data_Lorenz\\TPA-3rdplasmidconc1to1\\tea4s15w_0_002526.tif", "C:\\Analysis_from_Movie_for_RiboTrap_Dieter\\Movie_Data_Lorenz\\TPA-3rdplasmidconc1to1\\tea4s15w_0_002527.tif", "C:\\Analysis_from_Movie_for_RiboTrap_Dieter\\Movie_Data_Lorenz\\TPA-3rdplasmidconc1to1\\tea4s15w_0_002528.tif", "C:\\Analysis_from_Movie_for_RiboTrap_Dieter\\Movie_Data_Lorenz\\TPA-3rdplasmidconc1to1\\tea4s15w_0_002529.tif", "C:\\Analysis_from_Movie_for_RiboTrap_Dieter\\Movie_Data_Lorenz\\TPA-3rdplasmidconc1to1\\tea4s15w_0_002530.tif", "C:\\Analysis_from_Movie_for_RiboTrap_Dieter\\Movie_Data_Lorenz\\TPA-3rdplasmidconc1to1\\tea4s15w_0_002531.tif", "C:\\Analysis_from_Movie_for_RiboTrap_Dieter\\Movie_Data_Lorenz\\TPA-3rdplasmidconc1to1\\tea4s15w_0_002532.tif", "C:\\Analysis_from_Movie_for_RiboTrap_Dieter\\Movie_Data_Lorenz\\TPA-3rdplasmidconc1to1\\tea4s15w_0_002533.tif", "C:\\Analysis_from_Movie_for_RiboTrap_Dieter\\Movie_Data_Lorenz\\TPA-3rdplasmidconc1to1\\tea4s15w_0_002534.tif", "C:\\Analysis_from_Movie_for_RiboTrap_Dieter\\Movie_Data_Lorenz\\TPA-3rdplasmidconc1to1\\tea4s15w_0_002535.tif", "C:\\Analysis_from_Movie_for_RiboTrap_Dieter\\Movie_Data_Lorenz\\TPA-3rdplasmidconc1to1\\tea4s15w_0_002536.tif", "C:\\Analysis_from_Movie_for_RiboTrap_Dieter\\Movie_Data_Lorenz\\TPA-3rdplasmidconc1to1\\tea4s15w_0_002537.tif", "C:\\Analysis_from_Movie_for_RiboTrap_Dieter\\Movie_Data_Lorenz\\TPA-3rdplasmidconc1to1\\tea4s15w_0_002538.tif", "C:\\Analysis_from_Movie_for_RiboTrap_Dieter\\Movie_Data_Lorenz\\TPA-3rdplasmidconc1to1\\tea4s15w_0_002539.tif", "C:\\Analysis_from_Movie_for_RiboTrap_Dieter\\Movie_Data_Lorenz\\TPA-3rdplasmidconc1to1\\tea4s15w_0_002540.tif", "C:\\Analysis_from_Movie_for_RiboTrap_Dieter\\Movie_Data_Lorenz\\TPA-3rdplasmidconc1to1\\tea4s15w_0_002541.tif", "C:\\Analysis_from_Movie_for_RiboTrap_Dieter\\Movie_Data_Lorenz\\TPA-3rdplasmidconc1to1\\tea4s15w_0_002542.tif", "C:\\Analysis_from_Movie_for_RiboTrap_Dieter\\Movie_Data_Lorenz\\TPA-3rdplasmidconc1to1\\tea4s15w_0_002543.tif", "C:\\Analysis_from_Movie_for_RiboTrap_Dieter\\Movie_Data_Lorenz\\TPA-3rdplasmidconc1to1\\tea4s15w_0_002544.tif", "C:\\Analysis_from_Movie_for_RiboTrap_Dieter\\Movie_Data_Lorenz\\TPA-3rdplasmidconc1to1\\tea4s15w_0_002545.tif", "C:\\Analysis_from_Movie_for_RiboTrap_Dieter\\Movie_Data_Lorenz\\TPA-3rdplasmidconc1to1\\tea4s15w_0_002546.tif", "C:\\Analysis_from_Movie_for_RiboTrap_Dieter\\Movie_Data_Lorenz\\TPA-3rdplasmidconc1to1\\tea4s15w_0_002547.tif", "C:\\Analysis_from_Movie_for_RiboTrap_Dieter\\Movie_Data_Lorenz\\TPA-3rdplasmidconc1to1\\tea4s15w_0_002548.tif", "C:\\Analysis_from_Movie_for_RiboTrap_Dieter\\Movie_Data_Lorenz\\TPA-3rdplasmidconc1to1\\tea4s15w_0_002549.tif", "C:\\Analysis_from_Movie_for_RiboTrap_Dieter\\Movie_Data_Lorenz\\TPA-3rdplasmidconc1to1\\tea4s15w_0_002550.tif", "C:\\Analysis_from_Movie_for_RiboTrap_Dieter\\Movie_Data_Lorenz\\TPA-3rdplasmidconc1to1\\tea4s15w_0_002551.tif", "C:\\Analysis_from_Movie_for_RiboTrap_Dieter\\Movie_Data_Lorenz\\TPA-3rdplasmidconc1to1\\tea4s15w_0_002552.tif", "C:\\Analysis_from_Movie_for_RiboTrap_Dieter\\Movie_Data_Lorenz\\TPA-3rdplasmidconc1to1\\tea4s15w_0_002553.tif", "C:\\Analysis_from_Movie_for_RiboTrap_Dieter\\Movie_Data_Lorenz\\TPA-3rdplasmidconc1to1\\tea4s15w_0_002554.tif", "C:\\Analysis_from_Movie_for_RiboTrap_Dieter\\Movie_Data_Lorenz\\TPA-3rdplasmidconc1to1\\tea4s15w_0_002555.tif", "C:\\Analysis_from_Movie_for_RiboTrap_Dieter\\Movie_Data_Lorenz\\TPA-3rdplasmidconc1to1\\tea4s15w_0_002556.tif", "C:\\Analysis_from_Movie_for_RiboTrap_Dieter\\Movie_Data_Lorenz\\TPA-3rdplasmidconc1to1\\tea4s15w_0_002557.tif", "C:\\Analysis_from_Movie_for_RiboTrap_Dieter\\Movie_Data_Lorenz\\TPA-3rdplasmidconc1to1\\tea4s15w_0_002558.tif", "C:\\Analysis_from_Movie_for_RiboTrap_Dieter\\Movie_Data_Lorenz\\TPA-3rdplasmidconc1to1\\tea4s15w_0_002559.tif", "C:\\Analysis_from_Movie_for_RiboTrap_Dieter\\Movie_Data_Lorenz\\TPA-3rdplasmidconc1to1\\tea4s15w_0_002560.tif", "C:\\Analysis_from_Movie_for_RiboTrap_Dieter\\Movie_Data_Lorenz\\TPA-3rdplasmidconc1to1\\tea4s15w_0_002561.tif", "C:\\Analysis_from_Movie_for_RiboTrap_Dieter\\Movie_Data_Lorenz\\TPA-3rdplasmidconc1to1\\tea4s15w_0_002562.tif", "C:\\Analysis_from_Movie_for_RiboTrap_Dieter\\Movie_Data_Lorenz\\TPA-3rdplasmidconc1to1\\tea4s15w_0_002563.tif", "C:\\Analysis_from_Movie_for_RiboTrap_Dieter\\Movie_Data_Lorenz\\TPA-3rdplasmidconc1to1\\tea4s15w_0_002564.tif", "C:\\Analysis_from_Movie_for_RiboTrap_Dieter\\Movie_Data_Lorenz\\TPA-3rdplasmidconc1to1\\tea4s15w_0_002565.tif", "C:\\Analysis_from_Movie_for_RiboTrap_Dieter\\Movie_Data_Lorenz\\TPA-3rdplasmidconc1to1\\tea4s15w_0_002566.tif", "C:\\Analysis_from_Movie_for_RiboTrap_Dieter\\Movie_Data_Lorenz\\TPA-3rdplasmidconc1to1\\tea4s15w_0_002567.tif", "C:\\Analysis_from_Movie_for_RiboTrap_Dieter\\Movie_Data_Lorenz\\TPA-3rdplasmidconc1to1\\tea4s15w_0_002568.tif", "C:\\Analysis_from_Movie_for_RiboTrap_Dieter\\Movie_Data_Lorenz\\TPA-3rdplasmidconc1to1\\tea4s15w_0_002569.tif", "C:\\Analysis_from_Movie_for_RiboTrap_Dieter\\Movie_Data_Lorenz\\TPA-3rdplasmidconc1to1\\tea4s15w_0_002570.tif", "C:\\Analysis_from_Movie_for_RiboTrap_Dieter\\Movie_Data_Lorenz\\TPA-3rdplasmidconc1to1\\tea4s15w_0_002571.tif", "C:\\Analysis_from_Movie_for_RiboTrap_Dieter\\Movie_Data_Lorenz\\TPA-3rdplasmidconc1to1\\tea4s15w_0_002572.tif", "C:\\Analysis_from_Movie_for_RiboTrap_Dieter\\Movie_Data_Lorenz\\TPA-3rdplasmidconc1to1\\tea4s15w_0_002573.tif", "C:\\Analysis_from_Movie_for_RiboTrap_Dieter\\Movie_Data_Lorenz\\TPA-3rdplasmidconc1to1\\tea4s15w_0_002574.tif", "C:\\Analysis_from_Movie_for_RiboTrap_Dieter\\Movie_Data_Lorenz\\TPA-3rdplasmidconc1to1\\tea4s15w_0_002575.tif", "C:\\Analysis_from_Movie_for_RiboTrap_Dieter\\Movie_Data_Lorenz\\TPA-3rdplasmidconc1to1\\tea4s15w_0_002576.tif", "C:\\Analysis_from_Movie_for_RiboTrap_Dieter\\Movie_Data_Lorenz\\TPA-3rdplasmidconc1to1\\tea4s15w_0_002577.tif", "C:\\Analysis_from_Movie_for_RiboTrap_Dieter\\Movie_Data_Lorenz\\TPA-3rdplasmidconc1to1\\tea4s15w_0_002578.tif", "C:\\Analysis_from_Movie_for_RiboTrap_Dieter\\Movie_Data_Lorenz\\TPA-3rdplasmidconc1to1\\tea4s15w_0_002579.tif", "C:\\Analysis_from_Movie_for_RiboTrap_Dieter\\Movie_Data_Lorenz\\TPA-3rdplasmidconc1to1\\tea4s15w_0_002580.tif", "C:\\Analysis_from_Movie_for_RiboTrap_Dieter\\Movie_Data_Lorenz\\TPA-3rdplasmidconc1to1\\tea4s15w_0_002581.tif", "C:\\Analysis_from_Movie_for_RiboTrap_Dieter\\Movie_Data_Lorenz\\TPA-3rdplasmidconc1to1\\tea4s15w_0_002582.tif", "C:\\Analysis_from_Movie_for_RiboTrap_Dieter\\Movie_Data_Lorenz\\TPA-3rdplasmidconc1to1\\tea4s15w_0_002583.tif", "C:\\Analysis_from_Movie_for_RiboTrap_Dieter\\Movie_Data_Lorenz\\TPA-3rdplasmidconc1to1\\tea4s15w_0_002584.tif", "C:\\Analysis_from_Movie_for_RiboTrap_Dieter\\Movie_Data_Lorenz\\TPA-3rdplasmidconc1to1\\tea4s15w_0_002585.tif", "C:\\Analysis_from_Movie_for_RiboTrap_Dieter\\Movie_Data_Lorenz\\TPA-3rdplasmidconc1to1\\tea4s15w_0_002586.tif", "C:\\Analysis_from_Movie_for_RiboTrap_Dieter\\Movie_Data_Lorenz\\TPA-3rdplasmidconc1to1\\tea4s15w_0_002587.tif", "C:\\Analysis_from_Movie_for_RiboTrap_Dieter\\Movie_Data_Lorenz\\TPA-3rdplasmidconc1to1\\tea4s15w_0_002588.tif", "C:\\Analysis_from_Movie_for_RiboTrap_Dieter\\Movie_Data_Lorenz\\TPA-3rdplasmidconc1to1\\tea4s15w_0_002589.tif", "C:\\Analysis_from_Movie_for_RiboTrap_Dieter\\Movie_Data_Lorenz\\TPA-3rdplasmidconc1to1\\tea4s15w_0_002590.tif", "C:\\Analysis_from_Movie_for_RiboTrap_Dieter\\Movie_Data_Lorenz\\TPA-3rdplasmidconc1to1\\tea4s15w_0_002591.tif", "C:\\Analysis_from_Movie_for_RiboTrap_Dieter\\Movie_Data_Lorenz\\TPA-3rdplasmidconc1to1\\tea4s15w_0_002592.tif", "C:\\Analysis_from_Movie_for_RiboTrap_Dieter\\Movie_Data_Lorenz\\TPA-3rdplasmidconc1to1\\tea4s15w_0_002593.tif", "C:\\Analysis_from_Movie_for_RiboTrap_Dieter\\Movie_Data_Lorenz\\TPA-3rdplasmidconc1to1\\tea4s15w_0_002594.tif", "C:\\Analysis_from_Movie_for_RiboTrap_Dieter\\Movie_Data_Lorenz\\TPA-3rdplasmidconc1to1\\tea4s15w_0_002595.tif", "C:\\Analysis_from_Movie_for_RiboTrap_Dieter\\Movie_Data_Lorenz\\TPA-3rdplasmidconc1to1\\tea4s15w_0_002596.tif", "C:\\Analysis_from_Movie_for_RiboTrap_Dieter\\Movie_Data_Lorenz\\TPA-3rdplasmidconc1to1\\tea4s15w_0_002597.tif", "C:\\Analysis_from_Movie_for_RiboTrap_Dieter\\Movie_Data_Lorenz\\TPA-3rdplasmidconc1to1\\tea4s15w_0_002598.tif", "C:\\Analysis_from_Movie_for_RiboTrap_Dieter\\Movie_Data_Lorenz\\TPA-3rdplasmidconc1to1\\tea4s15w_0_002599.tif", "C:\\Analysis_from_Movie_for_RiboTrap_Dieter\\Movie_Data_Lorenz\\TPA-3rdplasmidconc1to1\\tea4s15w_0_002600.tif", "C:\\Analysis_from_Movie_for_RiboTrap_Dieter\\Movie_Data_Lorenz\\TPA-3rdplasmidconc1to1\\tea4s15w_0_002601.tif", "C:\\Analysis_from_Movie_for_RiboTrap_Dieter\\Movie_Data_Lorenz\\TPA-3rdplasmidconc1to1\\tea4s15w_0_002602.tif", "C:\\Analysis_from_Movie_for_RiboTrap_Dieter\\Movie_Data_Lorenz\\TPA-3rdplasmidconc1to1\\tea4s15w_0_002603.tif", "C:\\Analysis_from_Movie_for_RiboTrap_Dieter\\Movie_Data_Lorenz\\TPA-3rdplasmidconc1to1\\tea4s15w_0_002604.tif", "C:\\Analysis_from_Movie_for_RiboTrap_Dieter\\Movie_Data_Lorenz\\TPA-3rdplasmidconc1to1\\tea4s15w_0_002605.tif", "C:\\Analysis_from_Movie_for_RiboTrap_Dieter\\Movie_Data_Lorenz\\TPA-3rdplasmidconc1to1\\tea4s15w_0_002606.tif", "C:\\Analysis_from_Movie_for_RiboTrap_Dieter\\Movie_Data_Lorenz\\TPA-3rdplasmidconc1to1\\tea4s15w_0_002607.tif", "C:\\Analysis_from_Movie_for_RiboTrap_Dieter\\Movie_Data_Lorenz\\TPA-3rdplasmidconc1to1\\tea4s15w_0_002608.tif", "C:\\Analysis_from_Movie_for_RiboTrap_Dieter\\Movie_Data_Lorenz\\TPA-3rdplasmidconc1to1\\tea4s15w_0_002609.tif", "C:\\Analysis_from_Movie_for_RiboTrap_Dieter\\Movie_Data_Lorenz\\TPA-3rdplasmidconc1to1\\tea4s15w_0_002610.tif", "C:\\Analysis_from_Movie_for_RiboTrap_Dieter\\Movie_Data_Lorenz\\TPA-3rdplasmidconc1to1\\tea4s15w_0_002611.tif", "C:\\Analysis_from_Movie_for_RiboTrap_Dieter\\Movie_Data_Lorenz\\TPA-3rdplasmidconc1to1\\tea4s15w_0_002612.tif", "C:\\Analysis_from_Movie_for_RiboTrap_Dieter\\Movie_Data_Lorenz\\TPA-3rdplasmidconc1to1\\tea4s15w_0_002613.tif", "C:\\Analysis_from_Movie_for_RiboTrap_Dieter\\Movie_Data_Lorenz\\TPA-3rdplasmidconc1to1\\tea4s15w_0_002614.tif", "C:\\Analysis_from_Movie_for_RiboTrap_Dieter\\Movie_Data_Lorenz\\TPA-3rdplasmidconc1to1\\tea4s15w_0_002615.tif", "C:\\Analysis_from_Movie_for_RiboTrap_Dieter\\Movie_Data_Lorenz\\TPA-3rdplasmidconc1to1\\tea4s15w_0_002616.tif", "C:\\Analysis_from_Movie_for_RiboTrap_Dieter\\Movie_Data_Lorenz\\TPA-3rdplasmidconc1to1\\tea4s15w_0_002617.tif", "C:\\Analysis_from_Movie_for_RiboTrap_Dieter\\Movie_Data_Lorenz\\TPA-3rdplasmidconc1to1\\tea4s15w_0_002618.tif", "C:\\Analysis_from_Movie_for_RiboTrap_Dieter\\Movie_Data_Lorenz\\TPA-3rdplasmidconc1to1\\tea4s15w_0_002619.tif", "C:\\Analysis_from_Movie_for_RiboTrap_Dieter\\Movie_Data_Lorenz\\TPA-3rdplasmidconc1to1\\tea4s15w_0_002620.tif", "C:\\Analysis_from_Movie_for_RiboTrap_Dieter\\Movie_Data_Lorenz\\TPA-3rdplasmidconc1to1\\tea4s15w_0_002621.tif", "C:\\Analysis_from_Movie_for_RiboTrap_Dieter\\Movie_Data_Lorenz\\TPA-3rdplasmidconc1to1\\tea4s15w_0_002622.tif", "C:\\Analysis_from_Movie_for_RiboTrap_Dieter\\Movie_Data_Lorenz\\TPA-3rdplasmidconc1to1\\tea4s15w_0_002623.tif", "C:\\Analysis_from_Movie_for_RiboTrap_Dieter\\Movie_Data_Lorenz\\TPA-3rdplasmidconc1to1\\tea4s15w_0_002624.tif", "C:\\Analysis_from_Movie_for_RiboTrap_Dieter\\Movie_Data_Lorenz\\TPA-3rdplasmidconc1to1\\tea4s15w_0_002625.tif", "C:\\Analysis_from_Movie_for_RiboTrap_Dieter\\Movie_Data_Lorenz\\TPA-3rdplasmidconc1to1\\tea4s15w_0_002626.tif", "C:\\Analysis_from_Movie_for_RiboTrap_Dieter\\Movie_Data_Lorenz\\TPA-3rdplasmidconc1to1\\tea4s15w_0_002627.tif", "C:\\Analysis_from_Movie_for_RiboTrap_Dieter\\Movie_Data_Lorenz\\TPA-3rdplasmidconc1to1\\tea4s15w_0_002628.tif", "C:\\Analysis_from_Movie_for_RiboTrap_Dieter\\Movie_Data_Lorenz\\TPA-3rdplasmidconc1to1\\tea4s15w_0_002629.tif", "C:\\Analysis_from_Movie_for_RiboTrap_Dieter\\Movie_Data_Lorenz\\TPA-3rdplasmidconc1to1\\tea4s15w_0_002630.tif", "C:\\Analysis_from_Movie_for_RiboTrap_Dieter\\Movie_Data_Lorenz\\TPA-3rdplasmidconc1to1\\tea4s15w_0_002631.tif", "C:\\Analysis_from_Movie_for_RiboTrap_Dieter\\Movie_Data_Lorenz\\TPA-3rdplasmidconc1to1\\tea4s15w_0_002632.tif", "C:\\Analysis_from_Movie_for_RiboTrap_Dieter\\Movie_Data_Lorenz\\TPA-3rdplasmidconc1to1\\tea4s15w_0_002633.tif", "C:\\Analysis_from_Movie_for_RiboTrap_Dieter\\Movie_Data_Lorenz\\TPA-3rdplasmidconc1to1\\tea4s15w_0_002634.tif", "C:\\Analysis_from_Movie_for_RiboTrap_Dieter\\Movie_Data_Lorenz\\TPA-3rdplasmidconc1to1\\tea4s15w_0_002635.tif", "C:\\Analysis_from_Movie_for_RiboTrap_Dieter\\Movie_Data_Lorenz\\TPA-3rdplasmidconc1to1\\tea4s15w_0_002636.tif", "C:\\Analysis_from_Movie_for_RiboTrap_Dieter\\Movie_Data_Lorenz\\TPA-3rdplasmidconc1to1\\tea4s15w_0_002637.tif", "C:\\Analysis_from_Movie_for_RiboTrap_Dieter\\Movie_Data_Lorenz\\TPA-3rdplasmidconc1to1\\tea4s15w_0_002638.tif", "C:\\Analysis_from_Movie_for_RiboTrap_Dieter\\Movie_Data_Lorenz\\TPA-3rdplasmidconc1to1\\tea4s15w_0_002639.tif", "C:\\Analysis_from_Movie_for_RiboTrap_Dieter\\Movie_Data_Lorenz\\TPA-3rdplasmidconc1to1\\tea4s15w_0_002640.tif", "C:\\Analysis_from_Movie_for_RiboTrap_Dieter\\Movie_Data_Lorenz\\TPA-3rdplasmidconc1to1\\tea4s15w_0_002641.tif", "C:\\Analysis_from_Movie_for_RiboTrap_Dieter\\Movie_Data_Lorenz\\TPA-3rdplasmidconc1to1\\tea4s15w_0_002642.tif", "C:\\Analysis_from_Movie_for_RiboTrap_Dieter\\Movie_Data_Lorenz\\TPA-3rdplasmidconc1to1\\tea4s15w_0_002643.tif", "C:\\Analysis_from_Movie_for_RiboTrap_Dieter\\Movie_Data_Lorenz\\TPA-3rdplasmidconc1to1\\tea4s15w_0_002644.tif", "C:\\Analysis_from_Movie_for_RiboTrap_Dieter\\Movie_Data_Lorenz\\TPA-3rdplasmidconc1to1\\tea4s15w_0_002645.tif", "C:\\Analysis_from_Movie_for_RiboTrap_Dieter\\Movie_Data_Lorenz\\TPA-3rdplasmidconc1to1\\tea4s15w_0_002646.tif", "C:\\Analysis_from_Movie_for_RiboTrap_Dieter\\Movie_Data_Lorenz\\TPA-3rdplasmidconc1to1\\tea4s15w_0_002647.tif", "C:\\Analysis_from_Movie_for_RiboTrap_Dieter\\Movie_Data_Lorenz\\TPA-3rdplasmidconc1to1\\tea4s15w_0_002648.tif", "C:\\Analysis_from_Movie_for_RiboTrap_Dieter\\Movie_Data_Lorenz\\TPA-3rdplasmidconc1to1\\tea4s15w_0_002649.tif", "C:\\Analysis_from_Movie_for_RiboTrap_Dieter\\Movie_Data_Lorenz\\TPA-3rdplasmidconc1to1\\tea4s15w_0_002650.tif", "C:\\Analysis_from_Movie_for_RiboTrap_Dieter\\Movie_Data_Lorenz\\TPA-3rdplasmidconc1to1\\tea4s15w_0_002651.tif", "C:\\Analysis_from_Movie_for_RiboTrap_Dieter\\Movie_Data_Lorenz\\TPA-3rdplasmidconc1to1\\tea4s15w_0_002652.tif", "C:\\Analysis_from_Movie_for_RiboTrap_Dieter\\Movie_Data_Lorenz\\TPA-3rdplasmidconc1to1\\tea4s15w_0_002653.tif", "C:\\Analysis_from_Movie_for_RiboTrap_Dieter\\Movie_Data_Lorenz\\TPA-3rdplasmidconc1to1\\tea4s15w_0_002654.tif", "C:\\Analysis_from_Movie_for_RiboTrap_Dieter\\Movie_Data_Lorenz\\TPA-3rdplasmidconc1to1\\tea4s15w_0_002655.tif", "C:\\Analysis_from_Movie_for_RiboTrap_Dieter\\Movie_Data_Lorenz\\TPA-3rdplasmidconc1to1\\tea4s15w_0_002656.tif", "C:\\Analysis_from_Movie_for_RiboTrap_Dieter\\Movie_Data_Lorenz\\TPA-3rdplasmidconc1to1\\tea4s15w_0_002657.tif", "C:\\Analysis_from_Movie_for_RiboTrap_Dieter\\Movie_Data_Lorenz\\TPA-3rdplasmidconc1to1\\tea4s15w_0_002658.tif", "C:\\Analysis_from_Movie_for_RiboTrap_Dieter\\Movie_Data_Lorenz\\TPA-3rdplasmidconc1to1\\tea4s15w_0_002659.tif", "C:\\Analysis_from_Movie_for_RiboTrap_Dieter\\Movie_Data_Lorenz\\TPA-3rdplasmidconc1to1\\tea4s15w_0_002660.tif", "C:\\Analysis_from_Movie_for_RiboTrap_Dieter\\Movie_Data_Lorenz\\TPA-3rdplasmidconc1to1\\tea4s15w_0_002661.tif", "C:\\Analysis_from_Movie_for_RiboTrap_Dieter\\Movie_Data_Lorenz\\TPA-3rdplasmidconc1to1\\tea4s15w_0_002662.tif", "C:\\Analysis_from_Movie_for_RiboTrap_Dieter\\Movie_Data_Lorenz\\TPA-3rdplasmidconc1to1\\tea4s15w_0_002663.tif", "C:\\Analysis_from_Movie_for_RiboTrap_Dieter\\Movie_Data_Lorenz\\TPA-3rdplasmidconc1to1\\tea4s15w_0_002664.tif", "C:\\Analysis_from_Movie_for_RiboTrap_Dieter\\Movie_Data_Lorenz\\TPA-3rdplasmidconc1to1\\tea4s15w_0_002665.tif", "C:\\Analysis_from_Movie_for_RiboTrap_Dieter\\Movie_Data_Lorenz\\TPA-3rdplasmidconc1to1\\tea4s15w_0_002666.tif", "C:\\Analysis_from_Movie_for_RiboTrap_Dieter\\Movie_Data_Lorenz\\TPA-3rdplasmidconc1to1\\tea4s15w_0_002667.tif", "C:\\Analysis_from_Movie_for_RiboTrap_Dieter\\Movie_Data_Lorenz\\TPA-3rdplasmidconc1to1\\tea4s15w_0_002668.tif", "C:\\Analysis_from_Movie_for_RiboTrap_Dieter\\Movie_Data_Lorenz\\TPA-3rdplasmidconc1to1\\tea4s15w_0_002669.tif", "C:\\Analysis_from_Movie_for_RiboTrap_Dieter\\Movie_Data_Lorenz\\TPA-3rdplasmidconc1to1\\tea4s15w_0_002670.tif", "C:\\Analysis_from_Movie_for_RiboTrap_Dieter\\Movie_Data_Lorenz\\TPA-3rdplasmidconc1to1\\tea4s15w_0_002671.tif", "C:\\Analysis_from_Movie_for_RiboTrap_Dieter\\Movie_Data_Lorenz\\TPA-3rdplasmidconc1to1\\tea4s15w_0_002672.tif", "C:\\Analysis_from_Movie_for_RiboTrap_Dieter\\Movie_Data_Lorenz\\TPA-3rdplasmidconc1to1\\tea4s15w_0_002673.tif", "C:\\Analysis_from_Movie_for_RiboTrap_Dieter\\Movie_Data_Lorenz\\TPA-3rdplasmidconc1to1\\tea4s15w_0_002674.tif", "C:\\Analysis_from_Movie_for_RiboTrap_Dieter\\Movie_Data_Lorenz\\TPA-3rdplasmidconc1to1\\tea4s15w_0_002675.tif", "C:\\Analysis_from_Movie_for_RiboTrap_Dieter\\Movie_Data_Lorenz\\TPA-3rdplasmidconc1to1\\tea4s15w_0_002676.tif", "C:\\Analysis_from_Movie_for_RiboTrap_Dieter\\Movie_Data_Lorenz\\TPA-3rdplasmidconc1to1\\tea4s15w_0_002677.tif", "C:\\Analysis_from_Movie_for_RiboTrap_Dieter\\Movie_Data_Lorenz\\TPA-3rdplasmidconc1to1\\tea4s15w_0_002678.tif", "C:\\Analysis_from_Movie_for_RiboTrap_Dieter\\Movie_Data_Lorenz\\TPA-3rdplasmidconc1to1\\tea4s15w_0_002679.tif", "C:\\Analysis_from_Movie_for_RiboTrap_Dieter\\Movie_Data_Lorenz\\TPA-3rdplasmidconc1to1\\tea4s15w_0_002680.tif", "C:\\Analysis_from_Movie_for_RiboTrap_Dieter\\Movie_Data_Lorenz\\TPA-3rdplasmidconc1to1\\tea4s15w_0_002681.tif", "C:\\Analysis_from_Movie_for_RiboTrap_Dieter\\Movie_Data_Lorenz\\TPA-3rdplasmidconc1to1\\tea4s15w_0_002682.tif", "C:\\Analysis_from_Movie_for_RiboTrap_Dieter\\Movie_Data_Lorenz\\TPA-3rdplasmidconc1to1\\tea4s15w_0_002683.tif", "C:\\Analysis_from_Movie_for_RiboTrap_Dieter\\Movie_Data_Lorenz\\TPA-3rdplasmidconc1to1\\tea4s15w_0_002684.tif", "C:\\Analysis_from_Movie_for_RiboTrap_Dieter\\Movie_Data_Lorenz\\TPA-3rdplasmidconc1to1\\tea4s15w_0_002685.tif", "C:\\Analysis_from_Movie_for_RiboTrap_Dieter\\Movie_Data_Lorenz\\TPA-3rdplasmidconc1to1\\tea4s15w_0_002686.tif", "C:\\Analysis_from_Movie_for_RiboTrap_Dieter\\Movie_Data_Lorenz\\TPA-3rdplasmidconc1to1\\tea4s15w_0_002687.tif", "C:\\Analysis_from_Movie_for_RiboTrap_Dieter\\Movie_Data_Lorenz\\TPA-3rdplasmidconc1to1\\tea4s15w_0_002688.tif", "C:\\Analysis_from_Movie_for_RiboTrap_Dieter\\Movie_Data_Lorenz\\TPA-3rdplasmidconc1to1\\tea4s15w_0_002689.tif", "C:\\Analysis_from_Movie_for_RiboTrap_Dieter\\Movie_Data_Lorenz\\TPA-3rdplasmidconc1to1\\tea4s15w_0_002690.tif", "C:\\Analysis_from_Movie_for_RiboTrap_Dieter\\Movie_Data_Lorenz\\TPA-3rdplasmidconc1to1\\tea4s15w_0_002691.tif", "C:\\Analysis_from_Movie_for_RiboTrap_Dieter\\Movie_Data_Lorenz\\TPA-3rdplasmidconc1to1\\tea4s15w_0_002692.tif", "C:\\Analysis_from_Movie_for_RiboTrap_Dieter\\Movie_Data_Lorenz\\TPA-3rdplasmidconc1to1\\tea4s15w_0_002693.tif", "C:\\Analysis_from_Movie_for_RiboTrap_Dieter\\Movie_Data_Lorenz\\TPA-3rdplasmidconc1to1\\tea4s15w_0_002694.tif", "C:\\Analysis_from_Movie_for_RiboTrap_Dieter\\Movie_Data_Lorenz\\TPA-3rdplasmidconc1to1\\tea4s15w_0_002695.tif", "C:\\Analysis_from_Movie_for_RiboTrap_Dieter\\Movie_Data_Lorenz\\TPA-3rdplasmidconc1to1\\tea4s15w_0_002696.tif", "C:\\Analysis_from_Movie_for_RiboTrap_Dieter\\Movie_Data_Lorenz\\TPA-3rdplasmidconc1to1\\tea4s15w_0_002697.tif", "C:\\Analysis_from_Movie_for_RiboTrap_Dieter\\Movie_Data_Lorenz\\TPA-3rdplasmidconc1to1\\tea4s15w_0_002698.tif", "C:\\Analysis_from_Movie_for_RiboTrap_Dieter\\Movie_Data_Lorenz\\TPA-3rdplasmidconc1to1\\tea4s15w_0_002699.tif", "C:\\Analysis_from_Movie_for_RiboTrap_Dieter\\Movie_Data_Lorenz\\TPA-3rdplasmidconc1to1\\tea4s15w_0_002700.tif", "C:\\Analysis_from_Movie_for_RiboTrap_Dieter\\Movie_Data_Lorenz\\TPA-3rdplasmidconc1to1\\tea4s15w_0_002701.tif", "C:\\Analysis_from_Movie_for_RiboTrap_Dieter\\Movie_Data_Lorenz\\TPA-3rdplasmidconc1to1\\tea4s15w_0_002702.tif", "C:\\Analysis_from_Movie_for_RiboTrap_Dieter\\Movie_Data_Lorenz\\TPA-3rdplasmidconc1to1\\tea4s15w_0_002703.tif", "C:\\Analysis_from_Movie_for_RiboTrap_Dieter\\Movie_Data_Lorenz\\TPA-3rdplasmidconc1to1\\tea4s15w_0_002704.tif", "C:\\Analysis_from_Movie_for_RiboTrap_Dieter\\Movie_Data_Lorenz\\TPA-3rdplasmidconc1to1\\tea4s15w_0_002705.tif", "C:\\Analysis_from_Movie_for_RiboTrap_Dieter\\Movie_Data_Lorenz\\TPA-3rdplasmidconc1to1\\tea4s15w_0_002706.tif", "C:\\Analysis_from_Movie_for_RiboTrap_Dieter\\Movie_Data_Lorenz\\TPA-3rdplasmidconc1to1\\tea4s15w_0_002707.tif", "C:\\Analysis_from_Movie_for_RiboTrap_Dieter\\Movie_Data_Lorenz\\TPA-3rdplasmidconc1to1\\tea4s15w_0_002708.tif", "C:\\Analysis_from_Movie_for_RiboTrap_Dieter\\Movie_Data_Lorenz\\TPA-3rdplasmidconc1to1\\tea4s15w_0_002709.tif", "C:\\Analysis_from_Movie_for_RiboTrap_Dieter\\Movie_Data_Lorenz\\TPA-3rdplasmidconc1to1\\tea4s15w_0_002710.tif", "C:\\Analysis_from_Movie_for_RiboTrap_Dieter\\Movie_Data_Lorenz\\TPA-3rdplasmidconc1to1\\tea4s15w_0_002711.tif", "C:\\Analysis_from_Movie_for_RiboTrap_Dieter\\Movie_Data_Lorenz\\TPA-3rdplasmidconc1to1\\tea4s15w_0_002712.tif", "C:\\Analysis_from_Movie_for_RiboTrap_Dieter\\Movie_Data_Lorenz\\TPA-3rdplasmidconc1to1\\tea4s15w_0_002713.tif", "C:\\Analysis_from_Movie_for_RiboTrap_Dieter\\Movie_Data_Lorenz\\TPA-3rdplasmidconc1to1\\tea4s15w_0_002714.tif", "C:\\Analysis_from_Movie_for_RiboTrap_Dieter\\Movie_Data_Lorenz\\TPA-3rdplasmidconc1to1\\tea4s15w_0_002715.tif", "C:\\Analysis_from_Movie_for_RiboTrap_Dieter\\Movie_Data_Lorenz\\TPA-3rdplasmidconc1to1\\tea4s15w_0_002716.tif", "C:\\Analysis_from_Movie_for_RiboTrap_Dieter\\Movie_Data_Lorenz\\TPA-3rdplasmidconc1to1\\tea4s15w_0_002717.tif", "C:\\Analysis_from_Movie_for_RiboTrap_Dieter\\Movie_Data_Lorenz\\TPA-3rdplasmidconc1to1\\tea4s15w_0_002718.tif", "C:\\Analysis_from_Movie_for_RiboTrap_Dieter\\Movie_Data_Lorenz\\TPA-3rdplasmidconc1to1\\tea4s15w_0_002719.tif", "C:\\Analysis_from_Movie_for_RiboTrap_Dieter\\Movie_Data_Lorenz\\TPA-3rdplasmidconc1to1\\tea4s15w_0_002720.tif", "C:\\Analysis_from_Movie_for_RiboTrap_Dieter\\Movie_Data_Lorenz\\TPA-3rdplasmidconc1to1\\tea4s15w_0_002721.tif", "C:\\Analysis_from_Movie_for_RiboTrap_Dieter\\Movie_Data_Lorenz\\TPA-3rdplasmidconc1to1\\tea4s15w_0_002722.tif", "C:\\Analysis_from_Movie_for_RiboTrap_Dieter\\Movie_Data_Lorenz\\TPA-3rdplasmidconc1to1\\tea4s15w_0_002723.tif", "C:\\Analysis_from_Movie_for_RiboTrap_Dieter\\Movie_Data_Lorenz\\TPA-3rdplasmidconc1to1\\tea4s15w_0_002724.tif", "C:\\Analysis_from_Movie_for_RiboTrap_Dieter\\Movie_Data_Lorenz\\TPA-3rdplasmidconc1to1\\tea4s15w_0_002725.tif", "C:\\Analysis_from_Movie_for_RiboTrap_Dieter\\Movie_Data_Lorenz\\TPA-3rdplasmidconc1to1\\tea4s15w_0_002726.tif", "C:\\Analysis_from_Movie_for_RiboTrap_Dieter\\Movie_Data_Lorenz\\TPA-3rdplasmidconc1to1\\tea4s15w_0_002727.tif", "C:\\Analysis_from_Movie_for_RiboTrap_Dieter\\Movie_Data_Lorenz\\TPA-3rdplasmidconc1to1\\tea4s15w_0_002728.tif", "C:\\Analysis_from_Movie_for_RiboTrap_Dieter\\Movie_Data_Lorenz\\TPA-3rdplasmidconc1to1\\tea4s15w_0_002729.tif", "C:\\Analysis_from_Movie_for_RiboTrap_Dieter\\Movie_Data_Lorenz\\TPA-3rdplasmidconc1to1\\tea4s15w_0_002730.tif", "C:\\Analysis_from_Movie_for_RiboTrap_Dieter\\Movie_Data_Lorenz\\TPA-3rdplasmidconc1to1\\tea4s15w_0_002731.tif", "C:\\Analysis_from_Movie_for_RiboTrap_Dieter\\Movie_Data_Lorenz\\TPA-3rdplasmidconc1to1\\tea4s15w_0_002732.tif", "C:\\Analysis_from_Movie_for_RiboTrap_Dieter\\Movie_Data_Lorenz\\TPA-3rdplasmidconc1to1\\tea4s15w_0_002733.tif", "C:\\Analysis_from_Movie_for_RiboTrap_Dieter\\Movie_Data_Lorenz\\TPA-3rdplasmidconc1to1\\tea4s15w_0_002734.tif", "C:\\Analysis_from_Movie_for_RiboTrap_Dieter\\Movie_Data_Lorenz\\TPA-3rdplasmidconc1to1\\tea4s15w_0_002735.tif", "C:\\Analysis_from_Movie_for_RiboTrap_Dieter\\Movie_Data_Lorenz\\TPA-3rdplasmidconc1to1\\tea4s15w_0_002736.tif", "C:\\Analysis_from_Movie_for_RiboTrap_Dieter\\Movie_Data_Lorenz\\TPA-3rdplasmidconc1to1\\tea4s15w_0_002737.tif", "C:\\Analysis_from_Movie_for_RiboTrap_Dieter\\Movie_Data_Lorenz\\TPA-3rdplasmidconc1to1\\tea4s15w_0_002738.tif", "C:\\Analysis_from_Movie_for_RiboTrap_Dieter\\Movie_Data_Lorenz\\TPA-3rdplasmidconc1to1\\tea4s15w_0_002739.tif", "C:\\Analysis_from_Movie_for_RiboTrap_Dieter\\Movie_Data_Lorenz\\TPA-3rdplasmidconc1to1\\tea4s15w_0_002740.tif", "C:\\Analysis_from_Movie_for_RiboTrap_Dieter\\Movie_Data_Lorenz\\TPA-3rdplasmidconc1to1\\tea4s15w_0_002741.tif", "C:\\Analysis_from_Movie_for_RiboTrap_Dieter\\Movie_Data_Lorenz\\TPA-3rdplasmidconc1to1\\tea4s15w_0_002742.tif", "C:\\Analysis_from_Movie_for_RiboTrap_Dieter\\Movie_Data_Lorenz\\TPA-3rdplasmidconc1to1\\tea4s15w_0_002743.tif", "C:\\Analysis_from_Movie_for_RiboTrap_Dieter\\Movie_Data_Lorenz\\TPA-3rdplasmidconc1to1\\tea4s15w_0_002744.tif", "C:\\Analysis_from_Movie_for_RiboTrap_Dieter\\Movie_Data_Lorenz\\TPA-3rdplasmidconc1to1\\tea4s15w_0_002745.tif", "C:\\Analysis_from_Movie_for_RiboTrap_Dieter\\Movie_Data_Lorenz\\TPA-3rdplasmidconc1to1\\tea4s15w_0_002746.tif", "C:\\Analysis_from_Movie_for_RiboTrap_Dieter\\Movie_Data_Lorenz\\TPA-3rdplasmidconc1to1\\tea4s15w_0_002747.tif", "C:\\Analysis_from_Movie_for_RiboTrap_Dieter\\Movie_Data_Lorenz\\TPA-3rdplasmidconc1to1\\tea4s15w_0_002748.tif", "C:\\Analysis_from_Movie_for_RiboTrap_Dieter\\Movie_Data_Lorenz\\TPA-3rdplasmidconc1to1\\tea4s15w_0_002749.tif", "C:\\Analysis_from_Movie_for_RiboTrap_Dieter\\Movie_Data_Lorenz\\TPA-3rdplasmidconc1to1\\tea4s15w_0_002750.tif", "C:\\Analysis_from_Movie_for_RiboTrap_Dieter\\Movie_Data_Lorenz\\TPA-3rdplasmidconc1to1\\tea4s15w_0_002751.tif", "C:\\Analysis_from_Movie_for_RiboTrap_Dieter\\Movie_Data_Lorenz\\TPA-3rdplasmidconc1to1\\tea4s15w_0_002752.tif", "C:\\Analysis_from_Movie_for_RiboTrap_Dieter\\Movie_Data_Lorenz\\TPA-3rdplasmidconc1to1\\tea4s15w_0_002753.tif", "C:\\Analysis_from_Movie_for_RiboTrap_Dieter\\Movie_Data_Lorenz\\TPA-3rdplasmidconc1to1\\tea4s15w_0_002754.tif", "C:\\Analysis_from_Movie_for_RiboTrap_Dieter\\Movie_Data_Lorenz\\TPA-3rdplasmidconc1to1\\tea4s15w_0_002755.tif", "C:\\Analysis_from_Movie_for_RiboTrap_Dieter\\Movie_Data_Lorenz\\TPA-3rdplasmidconc1to1\\tea4s15w_0_002756.tif", "C:\\Analysis_from_Movie_for_RiboTrap_Dieter\\Movie_Data_Lorenz\\TPA-3rdplasmidconc1to1\\tea4s15w_0_002757.tif", "C:\\Analysis_from_Movie_for_RiboTrap_Dieter\\Movie_Data_Lorenz\\TPA-3rdplasmidconc1to1\\tea4s15w_0_002758.tif", "C:\\Analysis_from_Movie_for_RiboTrap_Dieter\\Movie_Data_Lorenz\\TPA-3rdplasmidconc1to1\\tea4s15w_0_002759.tif", "C:\\Analysis_from_Movie_for_RiboTrap_Dieter\\Movie_Data_Lorenz\\TPA-3rdplasmidconc1to1\\tea4s15w_0_002760.tif", "C:\\Analysis_from_Movie_for_RiboTrap_Dieter\\Movie_Data_Lorenz\\TPA-3rdplasmidconc1to1\\tea4s15w_0_002761.tif", "C:\\Analysis_from_Movie_for_RiboTrap_Dieter\\Movie_Data_Lorenz\\TPA-3rdplasmidconc1to1\\tea4s15w_0_002762.tif", "C:\\Analysis_from_Movie_for_RiboTrap_Dieter\\Movie_Data_Lorenz\\TPA-3rdplasmidconc1to1\\tea4s15w_0_002763.tif", "C:\\Analysis_from_Movie_for_RiboTrap_Dieter\\Movie_Data_Lorenz\\TPA-3rdplasmidconc1to1\\tea4s15w_0_002764.tif", "C:\\Analysis_from_Movie_for_RiboTrap_Dieter\\Movie_Data_Lorenz\\TPA-3rdplasmidconc1to1\\tea4s15w_0_002765.tif", "C:\\Analysis_from_Movie_for_RiboTrap_Dieter\\Movie_Data_Lorenz\\TPA-3rdplasmidconc1to1\\tea4s15w_0_002766.tif", "C:\\Analysis_from_Movie_for_RiboTrap_Dieter\\Movie_Data_Lorenz\\TPA-3rdplasmidconc1to1\\tea4s15w_0_002767.tif", "C:\\Analysis_from_Movie_for_RiboTrap_Dieter\\Movie_Data_Lorenz\\TPA-3rdplasmidconc1to1\\tea4s15w_0_002768.tif", "C:\\Analysis_from_Movie_for_RiboTrap_Dieter\\Movie_Data_Lorenz\\TPA-3rdplasmidconc1to1\\tea4s15w_0_002769.tif", "C:\\Analysis_from_Movie_for_RiboTrap_Dieter\\Movie_Data_Lorenz\\TPA-3rdplasmidconc1to1\\tea4s15w_0_002770.tif", "C:\\Analysis_from_Movie_for_RiboTrap_Dieter\\Movie_Data_Lorenz\\TPA-3rdplasmidconc1to1\\tea4s15w_0_002771.tif", "C:\\Analysis_from_Movie_for_RiboTrap_Dieter\\Movie_Data_Lorenz\\TPA-3rdplasmidconc1to1\\tea4s15w_0_002772.tif", "C:\\Analysis_from_Movie_for_RiboTrap_Dieter\\Movie_Data_Lorenz\\TPA-3rdplasmidconc1to1\\tea4s15w_0_002773.tif", "C:\\Analysis_from_Movie_for_RiboTrap_Dieter\\Movie_Data_Lorenz\\TPA-3rdplasmidconc1to1\\tea4s15w_0_002774.tif", "C:\\Analysis_from_Movie_for_RiboTrap_Dieter\\Movie_Data_Lorenz\\TPA-3rdplasmidconc1to1\\tea4s15w_0_002775.tif", "C:\\Analysis_from_Movie_for_RiboTrap_Dieter\\Movie_Data_Lorenz\\TPA-3rdplasmidconc1to1\\tea4s15w_0_002776.tif", "C:\\Analysis_from_Movie_for_RiboTrap_Dieter\\Movie_Data_Lorenz\\TPA-3rdplasmidconc1to1\\tea4s15w_0_002777.tif", "C:\\Analysis_from_Movie_for_RiboTrap_Dieter\\Movie_Data_Lorenz\\TPA-3rdplasmidconc1to1\\tea4s15w_0_002778.tif", "C:\\Analysis_from_Movie_for_RiboTrap_Dieter\\Movie_Data_Lorenz\\TPA-3rdplasmidconc1to1\\tea4s15w_0_002779.tif", "C:\\Analysis_from_Movie_for_RiboTrap_Dieter\\Movie_Data_Lorenz\\TPA-3rdplasmidconc1to1\\tea4s15w_0_002780.tif", "C:\\Analysis_from_Movie_for_RiboTrap_Dieter\\Movie_Data_Lorenz\\TPA-3rdplasmidconc1to1\\tea4s15w_0_002781.tif", "C:\\Analysis_from_Movie_for_RiboTrap_Dieter\\Movie_Data_Lorenz\\TPA-3rdplasmidconc1to1\\tea4s15w_0_002782.tif", "C:\\Analysis_from_Movie_for_RiboTrap_Dieter\\Movie_Data_Lorenz\\TPA-3rdplasmidconc1to1\\tea4s15w_0_002783.tif", "C:\\Analysis_from_Movie_for_RiboTrap_Dieter\\Movie_Data_Lorenz\\TPA-3rdplasmidconc1to1\\tea4s15w_0_002784.tif", "C:\\Analysis_from_Movie_for_RiboTrap_Dieter\\Movie_Data_Lorenz\\TPA-3rdplasmidconc1to1\\tea4s15w_0_002785.tif", "C:\\Analysis_from_Movie_for_RiboTrap_Dieter\\Movie_Data_Lorenz\\TPA-3rdplasmidconc1to1\\tea4s15w_0_002786.tif", "C:\\Analysis_from_Movie_for_RiboTrap_Dieter\\Movie_Data_Lorenz\\TPA-3rdplasmidconc1to1\\tea4s15w_0_002787.tif", "C:\\Analysis_from_Movie_for_RiboTrap_Dieter\\Movie_Data_Lorenz\\TPA-3rdplasmidconc1to1\\tea4s15w_0_002788.tif", "C:\\Analysis_from_Movie_for_RiboTrap_Dieter\\Movie_Data_Lorenz\\TPA-3rdplasmidconc1to1\\tea4s15w_0_002789.tif", "C:\\Analysis_from_Movie_for_RiboTrap_Dieter\\Movie_Data_Lorenz\\TPA-3rdplasmidconc1to1\\tea4s15w_0_002790.tif", "C:\\Analysis_from_Movie_for_RiboTrap_Dieter\\Movie_Data_Lorenz\\TPA-3rdplasmidconc1to1\\tea4s15w_0_002791.tif", "C:\\Analysis_from_Movie_for_RiboTrap_Dieter\\Movie_Data_Lorenz\\TPA-3rdplasmidconc1to1\\tea4s15w_0_002792.tif", "C:\\Analysis_from_Movie_for_RiboTrap_Dieter\\Movie_Data_Lorenz\\TPA-3rdplasmidconc1to1\\tea4s15w_0_002793.tif", "C:\\Analysis_from_Movie_for_RiboTrap_Dieter\\Movie_Data_Lorenz\\TPA-3rdplasmidconc1to1\\tea4s15w_0_002794.tif", "C:\\Analysis_from_Movie_for_RiboTrap_Dieter\\Movie_Data_Lorenz\\TPA-3rdplasmidconc1to1\\tea4s15w_0_002795.tif", "C:\\Analysis_from_Movie_for_RiboTrap_Dieter\\Movie_Data_Lorenz\\TPA-3rdplasmidconc1to1\\tea4s15w_0_002796.tif", "C:\\Analysis_from_Movie_for_RiboTrap_Dieter\\Movie_Data_Lorenz\\TPA-3rdplasmidconc1to1\\tea4s15w_0_002797.tif", "C:\\Analysis_from_Movie_for_RiboTrap_Dieter\\Movie_Data_Lorenz\\TPA-3rdplasmidconc1to1\\tea4s15w_0_002798.tif", "C:\\Analysis_from_Movie_for_RiboTrap_Dieter\\Movie_Data_Lorenz\\TPA-3rdplasmidconc1to1\\tea4s15w_0_002799.tif", "C:\\Analysis_from_Movie_for_RiboTrap_Dieter\\Movie_Data_Lorenz\\TPA-3rdplasmidconc1to1\\tea4s15w_0_002800.tif", "C:\\Analysis_from_Movie_for_RiboTrap_Dieter\\Movie_Data_Lorenz\\TPA-3rdplasmidconc1to1\\tea4s15w_0_002801.tif", "C:\\Analysis_from_Movie_for_RiboTrap_Dieter\\Movie_Data_Lorenz\\TPA-3rdplasmidconc1to1\\tea4s15w_0_002802.tif", "C:\\Analysis_from_Movie_for_RiboTrap_Dieter\\Movie_Data_Lorenz\\TPA-3rdplasmidconc1to1\\tea4s15w_0_002803.tif", "C:\\Analysis_from_Movie_for_RiboTrap_Dieter\\Movie_Data_Lorenz\\TPA-3rdplasmidconc1to1\\tea4s15w_0_002804.tif", "C:\\Analysis_from_Movie_for_RiboTrap_Dieter\\Movie_Data_Lorenz\\TPA-3rdplasmidconc1to1\\tea4s15w_0_002805.tif", "C:\\Analysis_from_Movie_for_RiboTrap_Dieter\\Movie_Data_Lorenz\\TPA-3rdplasmidconc1to1\\tea4s15w_0_002806.tif", "C:\\Analysis_from_Movie_for_RiboTrap_Dieter\\Movie_Data_Lorenz\\TPA-3rdplasmidconc1to1\\tea4s15w_0_002807.tif", "C:\\Analysis_from_Movie_for_RiboTrap_Dieter\\Movie_Data_Lorenz\\TPA-3rdplasmidconc1to1\\tea4s15w_0_002808.tif", "C:\\Analysis_from_Movie_for_RiboTrap_Dieter\\Movie_Data_Lorenz\\TPA-3rdplasmidconc1to1\\tea4s15w_0_002809.tif", "C:\\Analysis_from_Movie_for_RiboTrap_Dieter\\Movie_Data_Lorenz\\TPA-3rdplasmidconc1to1\\tea4s15w_0_002810.tif", "C:\\Analysis_from_Movie_for_RiboTrap_Dieter\\Movie_Data_Lorenz\\TPA-3rdplasmidconc1to1\\tea4s15w_0_002811.tif", "C:\\Analysis_from_Movie_for_RiboTrap_Dieter\\Movie_Data_Lorenz\\TPA-3rdplasmidconc1to1\\tea4s15w_0_002812.tif", "C:\\Analysis_from_Movie_for_RiboTrap_Dieter\\Movie_Data_Lorenz\\TPA-3rdplasmidconc1to1\\tea4s15w_0_002813.tif", "C:\\Analysis_from_Movie_for_RiboTrap_Dieter\\Movie_Data_Lorenz\\TPA-3rdplasmidconc1to1\\tea4s15w_0_002814.tif", "C:\\Analysis_from_Movie_for_RiboTrap_Dieter\\Movie_Data_Lorenz\\TPA-3rdplasmidconc1to1\\tea4s15w_0_002815.tif", "C:\\Analysis_from_Movie_for_RiboTrap_Dieter\\Movie_Data_Lorenz\\TPA-3rdplasmidconc1to1\\tea4s15w_0_002816.tif", "C:\\Analysis_from_Movie_for_RiboTrap_Dieter\\Movie_Data_Lorenz\\TPA-3rdplasmidconc1to1\\tea4s15w_0_002817.tif", "C:\\Analysis_from_Movie_for_RiboTrap_Dieter\\Movie_Data_Lorenz\\TPA-3rdplasmidconc1to1\\tea4s15w_0_002818.tif", "C:\\Analysis_from_Movie_for_RiboTrap_Dieter\\Movie_Data_Lorenz\\TPA-3rdplasmidconc1to1\\tea4s15w_0_002819.tif", "C:\\Analysis_from_Movie_for_RiboTrap_Dieter\\Movie_Data_Lorenz\\TPA-3rdplasmidconc1to1\\tea4s15w_0_002820.tif", "C:\\Analysis_from_Movie_for_RiboTrap_Dieter\\Movie_Data_Lorenz\\TPA-3rdplasmidconc1to1\\tea4s15w_0_002821.tif", "C:\\Analysis_from_Movie_for_RiboTrap_Dieter\\Movie_Data_Lorenz\\TPA-3rdplasmidconc1to1\\tea4s15w_0_002822.tif", "C:\\Analysis_from_Movie_for_RiboTrap_Dieter\\Movie_Data_Lorenz\\TPA-3rdplasmidconc1to1\\tea4s15w_0_002823.tif", "C:\\Analysis_from_Movie_for_RiboTrap_Dieter\\Movie_Data_Lorenz\\TPA-3rdplasmidconc1to1\\tea4s15w_0_002824.tif", "C:\\Analysis_from_Movie_for_RiboTrap_Dieter\\Movie_Data_Lorenz\\TPA-3rdplasmidconc1to1\\tea4s15w_0_002825.tif", "C:\\Analysis_from_Movie_for_RiboTrap_Dieter\\Movie_Data_Lorenz\\TPA-3rdplasmidconc1to1\\tea4s15w_0_002826.tif", "C:\\Analysis_from_Movie_for_RiboTrap_Dieter\\Movie_Data_Lorenz\\TPA-3rdplasmidconc1to1\\tea4s15w_0_002827.tif", "C:\\Analysis_from_Movie_for_RiboTrap_Dieter\\Movie_Data_Lorenz\\TPA-3rdplasmidconc1to1\\tea4s15w_0_002828.tif", "C:\\Analysis_from_Movie_for_RiboTrap_Dieter\\Movie_Data_Lorenz\\TPA-3rdplasmidconc1to1\\tea4s15w_0_002829.tif", "C:\\Analysis_from_Movie_for_RiboTrap_Dieter\\Movie_Data_Lorenz\\TPA-3rdplasmidconc1to1\\tea4s15w_0_002830.tif", "C:\\Analysis_from_Movie_for_RiboTrap_Dieter\\Movie_Data_Lorenz\\TPA-3rdplasmidconc1to1\\tea4s15w_0_002831.tif", "C:\\Analysis_from_Movie_for_RiboTrap_Dieter\\Movie_Data_Lorenz\\TPA-3rdplasmidconc1to1\\tea4s15w_0_002832.tif", "C:\\Analysis_from_Movie_for_RiboTrap_Dieter\\Movie_Data_Lorenz\\TPA-3rdplasmidconc1to1\\tea4s15w_0_002833.tif", "C:\\Analysis_from_Movie_for_RiboTrap_Dieter\\Movie_Data_Lorenz\\TPA-3rdplasmidconc1to1\\tea4s15w_0_002834.tif", "C:\\Analysis_from_Movie_for_RiboTrap_Dieter\\Movie_Data_Lorenz\\TPA-3rdplasmidconc1to1\\tea4s15w_0_002835.tif", "C:\\Analysis_from_Movie_for_RiboTrap_Dieter\\Movie_Data_Lorenz\\TPA-3rdplasmidconc1to1\\tea4s15w_0_002836.tif", "C:\\Analysis_from_Movie_for_RiboTrap_Dieter\\Movie_Data_Lorenz\\TPA-3rdplasmidconc1to1\\tea4s15w_0_002837.tif", "C:\\Analysis_from_Movie_for_RiboTrap_Dieter\\Movie_Data_Lorenz\\TPA-3rdplasmidconc1to1\\tea4s15w_0_002838.tif", "C:\\Analysis_from_Movie_for_RiboTrap_Dieter\\Movie_Data_Lorenz\\TPA-3rdplasmidconc1to1\\tea4s15w_0_002839.tif", "C:\\Analysis_from_Movie_for_RiboTrap_Dieter\\Movie_Data_Lorenz\\TPA-3rdplasmidconc1to1\\tea4s15w_0_002840.tif", "C:\\Analysis_from_Movie_for_RiboTrap_Dieter\\Movie_Data_Lorenz\\TPA-3rdplasmidconc1to1\\tea4s15w_0_002841.tif", "C:\\Analysis_from_Movie_for_RiboTrap_Dieter\\Movie_Data_Lorenz\\TPA-3rdplasmidconc1to1\\tea4s15w_0_002842.tif", "C:\\Analysis_from_Movie_for_RiboTrap_Dieter\\Movie_Data_Lorenz\\TPA-3rdplasmidconc1to1\\tea4s15w_0_002843.tif", "C:\\Analysis_from_Movie_for_RiboTrap_Dieter\\Movie_Data_Lorenz\\TPA-3rdplasmidconc1to1\\tea4s15w_0_002844.tif", "C:\\Analysis_from_Movie_for_RiboTrap_Dieter\\Movie_Data_Lorenz\\TPA-3rdplasmidconc1to1\\tea4s15w_0_002845.tif", "C:\\Analysis_from_Movie_for_RiboTrap_Dieter\\Movie_Data_Lorenz\\TPA-3rdplasmidconc1to1\\tea4s15w_0_002846.tif", "C:\\Analysis_from_Movie_for_RiboTrap_Dieter\\Movie_Data_Lorenz\\TPA-3rdplasmidconc1to1\\tea4s15w_0_002847.tif", "C:\\Analysis_from_Movie_for_RiboTrap_Dieter\\Movie_Data_Lorenz\\TPA-3rdplasmidconc1to1\\tea4s15w_0_002848.tif", "C:\\Analysis_from_Movie_for_RiboTrap_Dieter\\Movie_Data_Lorenz\\TPA-3rdplasmidconc1to1\\tea4s15w_0_002849.tif", "C:\\Analysis_from_Movie_for_RiboTrap_Dieter\\Movie_Data_Lorenz\\TPA-3rdplasmidconc1to1\\tea4s15w_0_002850.tif", "C:\\Analysis_from_Movie_for_RiboTrap_Dieter\\Movie_Data_Lorenz\\TPA-3rdplasmidconc1to1\\tea4s15w_0_002851.tif", "C:\\Analysis_from_Movie_for_RiboTrap_Dieter\\Movie_Data_Lorenz\\TPA-3rdplasmidconc1to1\\tea4s15w_0_002852.tif", "C:\\Analysis_from_Movie_for_RiboTrap_Dieter\\Movie_Data_Lorenz\\TPA-3rdplasmidconc1to1\\tea4s15w_0_002853.tif", "C:\\Analysis_from_Movie_for_RiboTrap_Dieter\\Movie_Data_Lorenz\\TPA-3rdplasmidconc1to1\\tea4s15w_0_002854.tif", "C:\\Analysis_from_Movie_for_RiboTrap_Dieter\\Movie_Data_Lorenz\\TPA-3rdplasmidconc1to1\\tea4s15w_0_002855.tif", "C:\\Analysis_from_Movie_for_RiboTrap_Dieter\\Movie_Data_Lorenz\\TPA-3rdplasmidconc1to1\\tea4s15w_0_002856.tif", "C:\\Analysis_from_Movie_for_RiboTrap_Dieter\\Movie_Data_Lorenz\\TPA-3rdplasmidconc1to1\\tea4s15w_0_002857.tif", "C:\\Analysis_from_Movie_for_RiboTrap_Dieter\\Movie_Data_Lorenz\\TPA-3rdplasmidconc1to1\\tea4s15w_0_002858.tif", "C:\\Analysis_from_Movie_for_RiboTrap_Dieter\\Movie_Data_Lorenz\\TPA-3rdplasmidconc1to1\\tea4s15w_0_002859.tif", "C:\\Analysis_from_Movie_for_RiboTrap_Dieter\\Movie_Data_Lorenz\\TPA-3rdplasmidconc1to1\\tea4s15w_0_002860.tif", "C:\\Analysis_from_Movie_for_RiboTrap_Dieter\\Movie_Data_Lorenz\\TPA-3rdplasmidconc1to1\\tea4s15w_0_002861.tif", "C:\\Analysis_from_Movie_for_RiboTrap_Dieter\\Movie_Data_Lorenz\\TPA-3rdplasmidconc1to1\\tea4s15w_0_002862.tif", "C:\\Analysis_from_Movie_for_RiboTrap_Dieter\\Movie_Data_Lorenz\\TPA-3rdplasmidconc1to1\\tea4s15w_0_002863.tif", "C:\\Analysis_from_Movie_for_RiboTrap_Dieter\\Movie_Data_Lorenz\\TPA-3rdplasmidconc1to1\\tea4s15w_0_002864.tif", "C:\\Analysis_from_Movie_for_RiboTrap_Dieter\\Movie_Data_Lorenz\\TPA-3rdplasmidconc1to1\\tea4s15w_0_002865.tif", "C:\\Analysis_from_Movie_for_RiboTrap_Dieter\\Movie_Data_Lorenz\\TPA-3rdplasmidconc1to1\\tea4s15w_0_002866.tif", "C:\\Analysis_from_Movie_for_RiboTrap_Dieter\\Movie_Data_Lorenz\\TPA-3rdplasmidconc1to1\\tea4s15w_0_002867.tif", "C:\\Analysis_from_Movie_for_RiboTrap_Dieter\\Movie_Data_Lorenz\\TPA-3rdplasmidconc1to1\\tea4s15w_0_002868.tif", "C:\\Analysis_from_Movie_for_RiboTrap_Dieter\\Movie_Data_Lorenz\\TPA-3rdplasmidconc1to1\\tea4s15w_0_002869.tif", "C:\\Analysis_from_Movie_for_RiboTrap_Dieter\\Movie_Data_Lorenz\\TPA-3rdplasmidconc1to1\\tea4s15w_0_002870.tif", "C:\\Analysis_from_Movie_for_RiboTrap_Dieter\\Movie_Data_Lorenz\\TPA-3rdplasmidconc1to1\\tea4s15w_0_002871.tif", "C:\\Analysis_from_Movie_for_RiboTrap_Dieter\\Movie_Data_Lorenz\\TPA-3rdplasmidconc1to1\\tea4s15w_0_002872.tif", "C:\\Analysis_from_Movie_for_RiboTrap_Dieter\\Movie_Data_Lorenz\\TPA-3rdplasmidconc1to1\\tea4s15w_0_002873.tif", "C:\\Analysis_from_Movie_for_RiboTrap_Dieter\\Movie_Data_Lorenz\\TPA-3rdplasmidconc1to1\\tea4s15w_0_002874.tif", "C:\\Analysis_from_Movie_for_RiboTrap_Dieter\\Movie_Data_Lorenz\\TPA-3rdplasmidconc1to1\\tea4s15w_0_002875.tif", "C:\\Analysis_from_Movie_for_RiboTrap_Dieter\\Movie_Data_Lorenz\\TPA-3rdplasmidconc1to1\\tea4s15w_0_002876.tif", "C:\\Analysis_from_Movie_for_RiboTrap_Dieter\\Movie_Data_Lorenz\\TPA-3rdplasmidconc1to1\\tea4s15w_0_002877.tif", "C:\\Analysis_from_Movie_for_RiboTrap_Dieter\\Movie_Data_Lorenz\\TPA-3rdplasmidconc1to1\\tea4s15w_0_002878.tif", "C:\\Analysis_from_Movie_for_RiboTrap_Dieter\\Movie_Data_Lorenz\\TPA-3rdplasmidconc1to1\\tea4s15w_0_002879.tif", "C:\\Analysis_from_Movie_for_RiboTrap_Dieter\\Movie_Data_Lorenz\\TPA-3rdplasmidconc1to1\\tea4s15w_0_002880.tif", "C:\\Analysis_from_Movie_for_RiboTrap_Dieter\\Movie_Data_Lorenz\\TPA-3rdplasmidconc1to1\\tea4s15w_0_002881.tif", "C:\\Analysis_from_Movie_for_RiboTrap_Dieter\\Movie_Data_Lorenz\\TPA-3rdplasmidconc1to1\\tea4s15w_0_002882.tif", "C:\\Analysis_from_Movie_for_RiboTrap_Dieter\\Movie_Data_Lorenz\\TPA-3rdplasmidconc1to1\\tea4s15w_0_002883.tif", "C:\\Analysis_from_Movie_for_RiboTrap_Dieter\\Movie_Data_Lorenz\\TPA-3rdplasmidconc1to1\\tea4s15w_0_002884.tif", "C:\\Analysis_from_Movie_for_RiboTrap_Dieter\\Movie_Data_Lorenz\\TPA-3rdplasmidconc1to1\\tea4s15w_0_002885.tif", "C:\\Analysis_from_Movie_for_RiboTrap_Dieter\\Movie_Data_Lorenz\\TPA-3rdplasmidconc1to1\\tea4s15w_0_002886.tif", "C:\\Analysis_from_Movie_for_RiboTrap_Dieter\\Movie_Data_Lorenz\\TPA-3rdplasmidconc1to1\\tea4s15w_0_002887.tif", "C:\\Analysis_from_Movie_for_RiboTrap_Dieter\\Movie_Data_Lorenz\\TPA-3rdplasmidconc1to1\\tea4s15w_0_002888.tif", "C:\\Analysis_from_Movie_for_RiboTrap_Dieter\\Movie_Data_Lorenz\\TPA-3rdplasmidconc1to1\\tea4s15w_0_002889.tif", "C:\\Analysis_from_Movie_for_RiboTrap_Dieter\\Movie_Data_Lorenz\\TPA-3rdplasmidconc1to1\\tea4s15w_0_002890.tif", "C:\\Analysis_from_Movie_for_RiboTrap_Dieter\\Movie_Data_Lorenz\\TPA-3rdplasmidconc1to1\\tea4s15w_0_002891.tif", "C:\\Analysis_from_Movie_for_RiboTrap_Dieter\\Movie_Data_Lorenz\\TPA-3rdplasmidconc1to1\\tea4s15w_0_002892.tif", "C:\\Analysis_from_Movie_for_RiboTrap_Dieter\\Movie_Data_Lorenz\\TPA-3rdplasmidconc1to1\\tea4s15w_0_002893.tif", "C:\\Analysis_from_Movie_for_RiboTrap_Dieter\\Movie_Data_Lorenz\\TPA-3rdplasmidconc1to1\\tea4s15w_0_002894.tif", "C:\\Analysis_from_Movie_for_RiboTrap_Dieter\\Movie_Data_Lorenz\\TPA-3rdplasmidconc1to1\\tea4s15w_0_002895.tif", "C:\\Analysis_from_Movie_for_RiboTrap_Dieter\\Movie_Data_Lorenz\\TPA-3rdplasmidconc1to1\\tea4s15w_0_002896.tif", "C:\\Analysis_from_Movie_for_RiboTrap_Dieter\\Movie_Data_Lorenz\\TPA-3rdplasmidconc1to1\\tea4s15w_0_002897.tif", "C:\\Analysis_from_Movie_for_RiboTrap_Dieter\\Movie_Data_Lorenz\\TPA-3rdplasmidconc1to1\\tea4s15w_0_002898.tif", "C:\\Analysis_from_Movie_for_RiboTrap_Dieter\\Movie_Data_Lorenz\\TPA-3rdplasmidconc1to1\\tea4s15w_0_002899.tif", "C:\\Analysis_from_Movie_for_RiboTrap_Dieter\\Movie_Data_Lorenz\\TPA-3rdplasmidconc1to1\\tea4s15w_0_002900.tif", "C:\\Analysis_from_Movie_for_RiboTrap_Dieter\\Movie_Data_Lorenz\\TPA-3rdplasmidconc1to1\\tea4s15w_0_002901.tif", "C:\\Analysis_from_Movie_for_RiboTrap_Dieter\\Movie_Data_Lorenz\\TPA-3rdplasmidconc1to1\\tea4s15w_0_002902.tif", "C:\\Analysis_from_Movie_for_RiboTrap_Dieter\\Movie_Data_Lorenz\\TPA-3rdplasmidconc1to1\\tea4s15w_0_002903.tif", "C:\\Analysis_from_Movie_for_RiboTrap_Dieter\\Movie_Data_Lorenz\\TPA-3rdplasmidconc1to1\\tea4s15w_0_002904.tif", "C:\\Analysis_from_Movie_for_RiboTrap_Dieter\\Movie_Data_Lorenz\\TPA-3rdplasmidconc1to1\\tea4s15w_0_002905.tif", "C:\\Analysis_from_Movie_for_RiboTrap_Dieter\\Movie_Data_Lorenz\\TPA-3rdplasmidconc1to1\\tea4s15w_0_002906.tif", "C:\\Analysis_from_Movie_for_RiboTrap_Dieter\\Movie_Data_Lorenz\\TPA-3rdplasmidconc1to1\\tea4s15w_0_002907.tif", "C:\\Analysis_from_Movie_for_RiboTrap_Dieter\\Movie_Data_Lorenz\\TPA-3rdplasmidconc1to1\\tea4s15w_0_002908.tif", "C:\\Analysis_from_Movie_for_RiboTrap_Dieter\\Movie_Data_Lorenz\\TPA-3rdplasmidconc1to1\\tea4s15w_0_002909.tif", "C:\\Analysis_from_Movie_for_RiboTrap_Dieter\\Movie_Data_Lorenz\\TPA-3rdplasmidconc1to1\\tea4s15w_0_002910.tif", "C:\\Analysis_from_Movie_for_RiboTrap_Dieter\\Movie_Data_Lorenz\\TPA-3rdplasmidconc1to1\\tea4s15w_0_002911.tif", "C:\\Analysis_from_Movie_for_RiboTrap_Dieter\\Movie_Data_Lorenz\\TPA-3rdplasmidconc1to1\\tea4s15w_0_002912.tif", "C:\\Analysis_from_Movie_for_RiboTrap_Dieter\\Movie_Data_Lorenz\\TPA-3rdplasmidconc1to1\\tea4s15w_0_002913.tif", "C:\\Analysis_from_Movie_for_RiboTrap_Dieter\\Movie_Data_Lorenz\\TPA-3rdplasmidconc1to1\\tea4s15w_0_002914.tif", "C:\\Analysis_from_Movie_for_RiboTrap_Dieter\\Movie_Data_Lorenz\\TPA-3rdplasmidconc1to1\\tea4s15w_0_002915.tif", "C:\\Analysis_from_Movie_for_RiboTrap_Dieter\\Movie_Data_Lorenz\\TPA-3rdplasmidconc1to1\\tea4s15w_0_002916.tif", "C:\\Analysis_from_Movie_for_RiboTrap_Dieter\\Movie_Data_Lorenz\\TPA-3rdplasmidconc1to1\\tea4s15w_0_002917.tif", "C:\\Analysis_from_Movie_for_RiboTrap_Dieter\\Movie_Data_Lorenz\\TPA-3rdplasmidconc1to1\\tea4s15w_0_002918.tif", "C:\\Analysis_from_Movie_for_RiboTrap_Dieter\\Movie_Data_Lorenz\\TPA-3rdplasmidconc1to1\\tea4s15w_0_002919.tif", "C:\\Analysis_from_Movie_for_RiboTrap_Dieter\\Movie_Data_Lorenz\\TPA-3rdplasmidconc1to1\\tea4s15w_0_002920.tif", "C:\\Analysis_from_Movie_for_RiboTrap_Dieter\\Movie_Data_Lorenz\\TPA-3rdplasmidconc1to1\\tea4s15w_0_002921.tif", "C:\\Analysis_from_Movie_for_RiboTrap_Dieter\\Movie_Data_Lorenz\\TPA-3rdplasmidconc1to1\\tea4s15w_0_002922.tif", "C:\\Analysis_from_Movie_for_RiboTrap_Dieter\\Movie_Data_Lorenz\\TPA-3rdplasmidconc1to1\\tea4s15w_0_002923.tif", "C:\\Analysis_from_Movie_for_RiboTrap_Dieter\\Movie_Data_Lorenz\\TPA-3rdplasmidconc1to1\\tea4s15w_0_002924.tif", "C:\\Analysis_from_Movie_for_RiboTrap_Dieter\\Movie_Data_Lorenz\\TPA-3rdplasmidconc1to1\\tea4s15w_0_002925.tif", "C:\\Analysis_from_Movie_for_RiboTrap_Dieter\\Movie_Data_Lorenz\\TPA-3rdplasmidconc1to1\\tea4s15w_0_002926.tif", "C:\\Analysis_from_Movie_for_RiboTrap_Dieter\\Movie_Data_Lorenz\\TPA-3rdplasmidconc1to1\\tea4s15w_0_002927.tif", "C:\\Analysis_from_Movie_for_RiboTrap_Dieter\\Movie_Data_Lorenz\\TPA-3rdplasmidconc1to1\\tea4s15w_0_002928.tif", "C:\\Analysis_from_Movie_for_RiboTrap_Dieter\\Movie_Data_Lorenz\\TPA-3rdplasmidconc1to1\\tea4s15w_0_002929.tif", "C:\\Analysis_from_Movie_for_RiboTrap_Dieter\\Movie_Data_Lorenz\\TPA-3rdplasmidconc1to1\\tea4s15w_0_002930.tif", "C:\\Analysis_from_Movie_for_RiboTrap_Dieter\\Movie_Data_Lorenz\\TPA-3rdplasmidconc1to1\\tea4s15w_0_002931.tif", "C:\\Analysis_from_Movie_for_RiboTrap_Dieter\\Movie_Data_Lorenz\\TPA-3rdplasmidconc1to1\\tea4s15w_0_002932.tif", "C:\\Analysis_from_Movie_for_RiboTrap_Dieter\\Movie_Data_Lorenz\\TPA-3rdplasmidconc1to1\\tea4s15w_0_002933.tif", "C:\\Analysis_from_Movie_for_RiboTrap_Dieter\\Movie_Data_Lorenz\\TPA-3rdplasmidconc1to1\\tea4s15w_0_002934.tif", "C:\\Analysis_from_Movie_for_RiboTrap_Dieter\\Movie_Data_Lorenz\\TPA-3rdplasmidconc1to1\\tea4s15w_0_002935.tif", "C:\\Analysis_from_Movie_for_RiboTrap_Dieter\\Movie_Data_Lorenz\\TPA-3rdplasmidconc1to1\\tea4s15w_0_002936.tif", "C:\\Analysis_from_Movie_for_RiboTrap_Dieter\\Movie_Data_Lorenz\\TPA-3rdplasmidconc1to1\\tea4s15w_0_002937.tif", "C:\\Analysis_from_Movie_for_RiboTrap_Dieter\\Movie_Data_Lorenz\\TPA-3rdplasmidconc1to1\\tea4s15w_0_002938.tif", "C:\\Analysis_from_Movie_for_RiboTrap_Dieter\\Movie_Data_Lorenz\\TPA-3rdplasmidconc1to1\\tea4s15w_0_002939.tif", "C:\\Analysis_from_Movie_for_RiboTrap_Dieter\\Movie_Data_Lorenz\\TPA-3rdplasmidconc1to1\\tea4s15w_0_002940.tif", "C:\\Analysis_from_Movie_for_RiboTrap_Dieter\\Movie_Data_Lorenz\\TPA-3rdplasmidconc1to1\\tea4s15w_0_002941.tif", "C:\\Analysis_from_Movie_for_RiboTrap_Dieter\\Movie_Data_Lorenz\\TPA-3rdplasmidconc1to1\\tea4s15w_0_002942.tif", "C:\\Analysis_from_Movie_for_RiboTrap_Dieter\\Movie_Data_Lorenz\\TPA-3rdplasmidconc1to1\\tea4s15w_0_002943.tif", "C:\\Analysis_from_Movie_for_RiboTrap_Dieter\\Movie_Data_Lorenz\\TPA-3rdplasmidconc1to1\\tea4s15w_0_002944.tif", "C:\\Analysis_from_Movie_for_RiboTrap_Dieter\\Movie_Data_Lorenz\\TPA-3rdplasmidconc1to1\\tea4s15w_0_002945.tif", "C:\\Analysis_from_Movie_for_RiboTrap_Dieter\\Movie_Data_Lorenz\\TPA-3rdplasmidconc1to1\\tea4s15w_0_002946.tif", "C:\\Analysis_from_Movie_for_RiboTrap_Dieter\\Movie_Data_Lorenz\\TPA-3rdplasmidconc1to1\\tea4s15w_0_002947.tif", "C:\\Analysis_from_Movie_for_RiboTrap_Dieter\\Movie_Data_Lorenz\\TPA-3rdplasmidconc1to1\\tea4s15w_0_002948.tif", "C:\\Analysis_from_Movie_for_RiboTrap_Dieter\\Movie_Data_Lorenz\\TPA-3rdplasmidconc1to1\\tea4s15w_0_002949.tif", "C:\\Analysis_from_Movie_for_RiboTrap_Dieter\\Movie_Data_Lorenz\\TPA-3rdplasmidconc1to1\\tea4s15w_0_002950.tif", "C:\\Analysis_from_Movie_for_RiboTrap_Dieter\\Movie_Data_Lorenz\\TPA-3rdplasmidconc1to1\\tea4s15w_0_002951.tif", "C:\\Analysis_from_Movie_for_RiboTrap_Dieter\\Movie_Data_Lorenz\\TPA-3rdplasmidconc1to1\\tea4s15w_0_002952.tif", "C:\\Analysis_from_Movie_for_RiboTrap_Dieter\\Movie_Data_Lorenz\\TPA-3rdplasmidconc1to1\\tea4s15w_0_002953.tif", "C:\\Analysis_from_Movie_for_RiboTrap_Dieter\\Movie_Data_Lorenz\\TPA-3rdplasmidconc1to1\\tea4s15w_0_002954.tif", "C:\\Analysis_from_Movie_for_RiboTrap_Dieter\\Movie_Data_Lorenz\\TPA-3rdplasmidconc1to1\\tea4s15w_0_002955.tif", "C:\\Analysis_from_Movie_for_RiboTrap_Dieter\\Movie_Data_Lorenz\\TPA-3rdplasmidconc1to1\\tea4s15w_0_002956.tif", "C:\\Analysis_from_Movie_for_RiboTrap_Dieter\\Movie_Data_Lorenz\\TPA-3rdplasmidconc1to1\\tea4s15w_0_002957.tif", "C:\\Analysis_from_Movie_for_RiboTrap_Dieter\\Movie_Data_Lorenz\\TPA-3rdplasmidconc1to1\\tea4s15w_0_002958.tif", "C:\\Analysis_from_Movie_for_RiboTrap_Dieter\\Movie_Data_Lorenz\\TPA-3rdplasmidconc1to1\\tea4s15w_0_002959.tif", "C:\\Analysis_from_Movie_for_RiboTrap_Dieter\\Movie_Data_Lorenz\\TPA-3rdplasmidconc1to1\\tea4s15w_0_002960.tif", "C:\\Analysis_from_Movie_for_RiboTrap_Dieter\\Movie_Data_Lorenz\\TPA-3rdplasmidconc1to1\\tea4s15w_0_002961.tif", "C:\\Analysis_from_Movie_for_RiboTrap_Dieter\\Movie_Data_Lorenz\\TPA-3rdplasmidconc1to1\\tea4s15w_0_002962.tif", "C:\\Analysis_from_Movie_for_RiboTrap_Dieter\\Movie_Data_Lorenz\\TPA-3rdplasmidconc1to1\\tea4s15w_0_002963.tif", "C:\\Analysis_from_Movie_for_RiboTrap_Dieter\\Movie_Data_Lorenz\\TPA-3rdplasmidconc1to1\\tea4s15w_0_002964.tif", "C:\\Analysis_from_Movie_for_RiboTrap_Dieter\\Movie_Data_Lorenz\\TPA-3rdplasmidconc1to1\\tea4s15w_0_002965.tif", "C:\\Analysis_from_Movie_for_RiboTrap_Dieter\\Movie_Data_Lorenz\\TPA-3rdplasmidconc1to1\\tea4s15w_0_002966.tif", "C:\\Analysis_from_Movie_for_RiboTrap_Dieter\\Movie_Data_Lorenz\\TPA-3rdplasmidconc1to1\\tea4s15w_0_002967.tif", "C:\\Analysis_from_Movie_for_RiboTrap_Dieter\\Movie_Data_Lorenz\\TPA-3rdplasmidconc1to1\\tea4s15w_0_002968.tif", "C:\\Analysis_from_Movie_for_RiboTrap_Dieter\\Movie_Data_Lorenz\\TPA-3rdplasmidconc1to1\\tea4s15w_0_002969.tif", "C:\\Analysis_from_Movie_for_RiboTrap_Dieter\\Movie_Data_Lorenz\\TPA-3rdplasmidconc1to1\\tea4s15w_0_002970.tif", "C:\\Analysis_from_Movie_for_RiboTrap_Dieter\\Movie_Data_Lorenz\\TPA-3rdplasmidconc1to1\\tea4s15w_0_002971.tif", "C:\\Analysis_from_Movie_for_RiboTrap_Dieter\\Movie_Data_Lorenz\\TPA-3rdplasmidconc1to1\\tea4s15w_0_002972.tif", "C:\\Analysis_from_Movie_for_RiboTrap_Dieter\\Movie_Data_Lorenz\\TPA-3rdplasmidconc1to1\\tea4s15w_0_002973.tif", "C:\\Analysis_from_Movie_for_RiboTrap_Dieter\\Movie_Data_Lorenz\\TPA-3rdplasmidconc1to1\\tea4s15w_0_002974.tif", "C:\\Analysis_from_Movie_for_RiboTrap_Dieter\\Movie_Data_Lorenz\\TPA-3rdplasmidconc1to1\\tea4s15w_0_002975.tif", "C:\\Analysis_from_Movie_for_RiboTrap_Dieter\\Movie_Data_Lorenz\\TPA-3rdplasmidconc1to1\\tea4s15w_0_002976.tif", "C:\\Analysis_from_Movie_for_RiboTrap_Dieter\\Movie_Data_Lorenz\\TPA-3rdplasmidconc1to1\\tea4s15w_0_002977.tif", "C:\\Analysis_from_Movie_for_RiboTrap_Dieter\\Movie_Data_Lorenz\\TPA-3rdplasmidconc1to1\\tea4s15w_0_002978.tif", "C:\\Analysis_from_Movie_for_RiboTrap_Dieter\\Movie_Data_Lorenz\\TPA-3rdplasmidconc1to1\\tea4s15w_0_002979.tif", "C:\\Analysis_from_Movie_for_RiboTrap_Dieter\\Movie_Data_Lorenz\\TPA-3rdplasmidconc1to1\\tea4s15w_0_002980.tif", "C:\\Analysis_from_Movie_for_RiboTrap_Dieter\\Movie_Data_Lorenz\\TPA-3rdplasmidconc1to1\\tea4s15w_0_002981.tif", "C:\\Analysis_from_Movie_for_RiboTrap_Dieter\\Movie_Data_Lorenz\\TPA-3rdplasmidconc1to1\\tea4s15w_0_002982.tif", "C:\\Analysis_from_Movie_for_RiboTrap_Dieter\\Movie_Data_Lorenz\\TPA-3rdplasmidconc1to1\\tea4s15w_0_002983.tif", "C:\\Analysis_from_Movie_for_RiboTrap_Dieter\\Movie_Data_Lorenz\\TPA-3rdplasmidconc1to1\\tea4s15w_0_002984.tif", "C:\\Analysis_from_Movie_for_RiboTrap_Dieter\\Movie_Data_Lorenz\\TPA-3rdplasmidconc1to1\\tea4s15w_0_002985.tif", "C:\\Analysis_from_Movie_for_RiboTrap_Dieter\\Movie_Data_Lorenz\\TPA-3rdplasmidconc1to1\\tea4s15w_0_002986.tif", "C:\\Analysis_from_Movie_for_RiboTrap_Dieter\\Movie_Data_Lorenz\\TPA-3rdplasmidconc1to1\\tea4s15w_0_002987.tif", "C:\\Analysis_from_Movie_for_RiboTrap_Dieter\\Movie_Data_Lorenz\\TPA-3rdplasmidconc1to1\\tea4s15w_0_002988.tif", "C:\\Analysis_from_Movie_for_RiboTrap_Dieter\\Movie_Data_Lorenz\\TPA-3rdplasmidconc1to1\\tea4s15w_0_002989.tif", "C:\\Analysis_from_Movie_for_RiboTrap_Dieter\\Movie_Data_Lorenz\\TPA-3rdplasmidconc1to1\\tea4s15w_0_002990.tif", "C:\\Analysis_from_Movie_for_RiboTrap_Dieter\\Movie_Data_Lorenz\\TPA-3rdplasmidconc1to1\\tea4s15w_0_002991.tif", "C:\\Analysis_from_Movie_for_RiboTrap_Dieter\\Movie_Data_Lorenz\\TPA-3rdplasmidconc1to1\\tea4s15w_0_002992.tif", "C:\\Analysis_from_Movie_for_RiboTrap_Dieter\\Movie_Data_Lorenz\\TPA-3rdplasmidconc1to1\\tea4s15w_0_002993.tif", "C:\\Analysis_from_Movie_for_RiboTrap_Dieter\\Movie_Data_Lorenz\\TPA-3rdplasmidconc1to1\\tea4s15w_0_002994.tif", "C:\\Analysis_from_Movie_for_RiboTrap_Dieter\\Movie_Data_Lorenz\\TPA-3rdplasmidconc1to1\\tea4s15w_0_002995.tif", "C:\\Analysis_from_Movie_for_RiboTrap_Dieter\\Movie_Data_Lorenz\\TPA-3rdplasmidconc1to1\\tea4s15w_0_002996.tif", "C:\\Analysis_from_Movie_for_RiboTrap_Dieter\\Movie_Data_Lorenz\\TPA-3rdplasmidconc1to1\\tea4s15w_0_002997.tif", "C:\\Analysis_from_Movie_for_RiboTrap_Dieter\\Movie_Data_Lorenz\\TPA-3rdplasmidconc1to1\\tea4s15w_0_002998.tif", "C:\\Analysis_from_Movie_for_RiboTrap_Dieter\\Movie_Data_Lorenz\\TPA-3rdplasmidconc1to1\\tea4s15w_0_002999.tif", "C:\\Analysis_from_Movie_for_RiboTrap_Dieter\\Movie_Data_Lorenz\\TPA-3rdplasmidconc1to1\\tea4s15w_0_003000.tif", "C:\\Analysis_from_Movie_for_RiboTrap_Dieter\\Movie_Data_Lorenz\\TPA-3rdplasmidconc1to1\\tea4s15w_0_003001.tif", "C:\\Analysis_from_Movie_for_RiboTrap_Dieter\\Movie_Data_Lorenz\\TPA-3rdplasmidconc1to1\\tea4s15w_0_003002.tif", "C:\\Analysis_from_Movie_for_RiboTrap_Dieter\\Movie_Data_Lorenz\\TPA-3rdplasmidconc1to1\\tea4s15w_0_003003.tif", "C:\\Analysis_from_Movie_for_RiboTrap_Dieter\\Movie_Data_Lorenz\\TPA-3rdplasmidconc1to1\\tea4s15w_0_003004.tif", "C:\\Analysis_from_Movie_for_RiboTrap_Dieter\\Movie_Data_Lorenz\\TPA-3rdplasmidconc1to1\\tea4s15w_0_003005.tif", "C:\\Analysis_from_Movie_for_RiboTrap_Dieter\\Movie_Data_Lorenz\\TPA-3rdplasmidconc1to1\\tea4s15w_0_003006.tif", "C:\\Analysis_from_Movie_for_RiboTrap_Dieter\\Movie_Data_Lorenz\\TPA-3rdplasmidconc1to1\\tea4s15w_0_003007.tif", "C:\\Analysis_from_Movie_for_RiboTrap_Dieter\\Movie_Data_Lorenz\\TPA-3rdplasmidconc1to1\\tea4s15w_0_003008.tif", "C:\\Analysis_from_Movie_for_RiboTrap_Dieter\\Movie_Data_Lorenz\\TPA-3rdplasmidconc1to1\\tea4s15w_0_003009.tif", "C:\\Analysis_from_Movie_for_RiboTrap_Dieter\\Movie_Data_Lorenz\\TPA-3rdplasmidconc1to1\\tea4s15w_0_003010.tif", "C:\\Analysis_from_Movie_for_RiboTrap_Dieter\\Movie_Data_Lorenz\\TPA-3rdplasmidconc1to1\\tea4s15w_0_003011.tif", "C:\\Analysis_from_Movie_for_RiboTrap_Dieter\\Movie_Data_Lorenz\\TPA-3rdplasmidconc1to1\\tea4s15w_0_003012.tif", "C:\\Analysis_from_Movie_for_RiboTrap_Dieter\\Movie_Data_Lorenz\\TPA-3rdplasmidconc1to1\\tea4s15w_0_003013.tif", "C:\\Analysis_from_Movie_for_RiboTrap_Dieter\\Movie_Data_Lorenz\\TPA-3rdplasmidconc1to1\\tea4s15w_0_003014.tif", "C:\\Analysis_from_Movie_for_RiboTrap_Dieter\\Movie_Data_Lorenz\\TPA-3rdplasmidconc1to1\\tea4s15w_0_003015.tif", "C:\\Analysis_from_Movie_for_RiboTrap_Dieter\\Movie_Data_Lorenz\\TPA-3rdplasmidconc1to1\\tea4s15w_0_003016.tif", "C:\\Analysis_from_Movie_for_RiboTrap_Dieter\\Movie_Data_Lorenz\\TPA-3rdplasmidconc1to1\\tea4s15w_0_003017.tif", "C:\\Analysis_from_Movie_for_RiboTrap_Dieter\\Movie_Data_Lorenz\\TPA-3rdplasmidconc1to1\\tea4s15w_0_003018.tif", "C:\\Analysis_from_Movie_for_RiboTrap_Dieter\\Movie_Data_Lorenz\\TPA-3rdplasmidconc1to1\\tea4s15w_0_003019.tif", "C:\\Analysis_from_Movie_for_RiboTrap_Dieter\\Movie_Data_Lorenz\\TPA-3rdplasmidconc1to1\\tea4s15w_0_003020.tif", "C:\\Analysis_from_Movie_for_RiboTrap_Dieter\\Movie_Data_Lorenz\\TPA-3rdplasmidconc1to1\\tea4s15w_0_003021.tif", "C:\\Analysis_from_Movie_for_RiboTrap_Dieter\\Movie_Data_Lorenz\\TPA-3rdplasmidconc1to1\\tea4s15w_0_003022.tif", "C:\\Analysis_from_Movie_for_RiboTrap_Dieter\\Movie_Data_Lorenz\\TPA-3rdplasmidconc1to1\\tea4s15w_0_003023.tif", "C:\\Analysis_from_Movie_for_RiboTrap_Dieter\\Movie_Data_Lorenz\\TPA-3rdplasmidconc1to1\\tea4s15w_0_003024.tif", "C:\\Analysis_from_Movie_for_RiboTrap_Dieter\\Movie_Data_Lorenz\\TPA-3rdplasmidconc1to1\\tea4s15w_0_003025.tif", "C:\\Analysis_from_Movie_for_RiboTrap_Dieter\\Movie_Data_Lorenz\\TPA-3rdplasmidconc1to1\\tea4s15w_0_003026.tif", "C:\\Analysis_from_Movie_for_RiboTrap_Dieter\\Movie_Data_Lorenz\\TPA-3rdplasmidconc1to1\\tea4s15w_0_003027.tif", "C:\\Analysis_from_Movie_for_RiboTrap_Dieter\\Movie_Data_Lorenz\\TPA-3rdplasmidconc1to1\\tea4s15w_0_003028.tif", "C:\\Analysis_from_Movie_for_RiboTrap_Dieter\\Movie_Data_Lorenz\\TPA-3rdplasmidconc1to1\\tea4s15w_0_003029.tif", "C:\\Analysis_from_Movie_for_RiboTrap_Dieter\\Movie_Data_Lorenz\\TPA-3rdplasmidconc1to1\\tea4s15w_0_003030.tif", "C:\\Analysis_from_Movie_for_RiboTrap_Dieter\\Movie_Data_Lorenz\\TPA-3rdplasmidconc1to1\\tea4s15w_0_003031.tif", "C:\\Analysis_from_Movie_for_RiboTrap_Dieter\\Movie_Data_Lorenz\\TPA-3rdplasmidconc1to1\\tea4s15w_0_003032.tif", "C:\\Analysis_from_Movie_for_RiboTrap_Dieter\\Movie_Data_Lorenz\\TPA-3rdplasmidconc1to1\\tea4s15w_0_003033.tif", "C:\\Analysis_from_Movie_for_RiboTrap_Dieter\\Movie_Data_Lorenz\\TPA-3rdplasmidconc1to1\\tea4s15w_0_003034.tif", "C:\\Analysis_from_Movie_for_RiboTrap_Dieter\\Movie_Data_Lorenz\\TPA-3rdplasmidconc1to1\\tea4s15w_0_003035.tif", "C:\\Analysis_from_Movie_for_RiboTrap_Dieter\\Movie_Data_Lorenz\\TPA-3rdplasmidconc1to1\\tea4s15w_0_003036.tif", "C:\\Analysis_from_Movie_for_RiboTrap_Dieter\\Movie_Data_Lorenz\\TPA-3rdplasmidconc1to1\\tea4s15w_0_003037.tif", "C:\\Analysis_from_Movie_for_RiboTrap_Dieter\\Movie_Data_Lorenz\\TPA-3rdplasmidconc1to1\\tea4s15w_0_003038.tif", "C:\\Analysis_from_Movie_for_RiboTrap_Dieter\\Movie_Data_Lorenz\\TPA-3rdplasmidconc1to1\\tea4s15w_0_003039.tif", "C:\\Analysis_from_Movie_for_RiboTrap_Dieter\\Movie_Data_Lorenz\\TPA-3rdplasmidconc1to1\\tea4s15w_0_003040.tif", "C:\\Analysis_from_Movie_for_RiboTrap_Dieter\\Movie_Data_Lorenz\\TPA-3rdplasmidconc1to1\\tea4s15w_0_003041.tif", "C:\\Analysis_from_Movie_for_RiboTrap_Dieter\\Movie_Data_Lorenz\\TPA-3rdplasmidconc1to1\\tea4s15w_0_003042.tif", "C:\\Analysis_from_Movie_for_RiboTrap_Dieter\\Movie_Data_Lorenz\\TPA-3rdplasmidconc1to1\\tea4s15w_0_003043.tif", "C:\\Analysis_from_Movie_for_RiboTrap_Dieter\\Movie_Data_Lorenz\\TPA-3rdplasmidconc1to1\\tea4s15w_0_003044.tif", "C:\\Analysis_from_Movie_for_RiboTrap_Dieter\\Movie_Data_Lorenz\\TPA-3rdplasmidconc1to1\\tea4s15w_0_003045.tif", "C:\\Analysis_from_Movie_for_RiboTrap_Dieter\\Movie_Data_Lorenz\\TPA-3rdplasmidconc1to1\\tea4s15w_0_003046.tif", "C:\\Analysis_from_Movie_for_RiboTrap_Dieter\\Movie_Data_Lorenz\\TPA-3rdplasmidconc1to1\\tea4s15w_0_003047.tif", "C:\\Analysis_from_Movie_for_RiboTrap_Dieter\\Movie_Data_Lorenz\\TPA-3rdplasmidconc1to1\\tea4s15w_0_003048.tif", "C:\\Analysis_from_Movie_for_RiboTrap_Dieter\\Movie_Data_Lorenz\\TPA-3rdplasmidconc1to1\\tea4s15w_0_003049.tif", "C:\\Analysis_from_Movie_for_RiboTrap_Dieter\\Movie_Data_Lorenz\\TPA-3rdplasmidconc1to1\\tea4s15w_0_003050.tif", "C:\\Analysis_from_Movie_for_RiboTrap_Dieter\\Movie_Data_Lorenz\\TPA-3rdplasmidconc1to1\\tea4s15w_0_003051.tif", "C:\\Analysis_from_Movie_for_RiboTrap_Dieter\\Movie_Data_Lorenz\\TPA-3rdplasmidconc1to1\\tea4s15w_0_003052.tif", "C:\\Analysis_from_Movie_for_RiboTrap_Dieter\\Movie_Data_Lorenz\\TPA-3rdplasmidconc1to1\\tea4s15w_0_003053.tif", "C:\\Analysis_from_Movie_for_RiboTrap_Dieter\\Movie_Data_Lorenz\\TPA-3rdplasmidconc1to1\\tea4s15w_0_003054.tif", "C:\\Analysis_from_Movie_for_RiboTrap_Dieter\\Movie_Data_Lorenz\\TPA-3rdplasmidconc1to1\\tea4s15w_0_003055.tif", "C:\\Analysis_from_Movie_for_RiboTrap_Dieter\\Movie_Data_Lorenz\\TPA-3rdplasmidconc1to1\\tea4s15w_0_003056.tif", "C:\\Analysis_from_Movie_for_RiboTrap_Dieter\\Movie_Data_Lorenz\\TPA-3rdplasmidconc1to1\\tea4s15w_0_003057.tif", "C:\\Analysis_from_Movie_for_RiboTrap_Dieter\\Movie_Data_Lorenz\\TPA-3rdplasmidconc1to1\\tea4s15w_0_003058.tif", "C:\\Analysis_from_Movie_for_RiboTrap_Dieter\\Movie_Data_Lorenz\\TPA-3rdplasmidconc1to1\\tea4s15w_0_003059.tif", "C:\\Analysis_from_Movie_for_RiboTrap_Dieter\\Movie_Data_Lorenz\\TPA-3rdplasmidconc1to1\\tea4s15w_0_003060.tif", "C:\\Analysis_from_Movie_for_RiboTrap_Dieter\\Movie_Data_Lorenz\\TPA-3rdplasmidconc1to1\\tea4s15w_0_003061.tif", "C:\\Analysis_from_Movie_for_RiboTrap_Dieter\\Movie_Data_Lorenz\\TPA-3rdplasmidconc1to1\\tea4s15w_0_003062.tif", "C:\\Analysis_from_Movie_for_RiboTrap_Dieter\\Movie_Data_Lorenz\\TPA-3rdplasmidconc1to1\\tea4s15w_0_003063.tif", "C:\\Analysis_from_Movie_for_RiboTrap_Dieter\\Movie_Data_Lorenz\\TPA-3rdplasmidconc1to1\\tea4s15w_0_003064.tif", "C:\\Analysis_from_Movie_for_RiboTrap_Dieter\\Movie_Data_Lorenz\\TPA-3rdplasmidconc1to1\\tea4s15w_0_003065.tif", "C:\\Analysis_from_Movie_for_RiboTrap_Dieter\\Movie_Data_Lorenz\\TPA-3rdplasmidconc1to1\\tea4s15w_0_003066.tif", "C:\\Analysis_from_Movie_for_RiboTrap_Dieter\\Movie_Data_Lorenz\\TPA-3rdplasmidconc1to1\\tea4s15w_0_003067.tif", "C:\\Analysis_from_Movie_for_RiboTrap_Dieter\\Movie_Data_Lorenz\\TPA-3rdplasmidconc1to1\\tea4s15w_0_003068.tif", "C:\\Analysis_from_Movie_for_RiboTrap_Dieter\\Movie_Data_Lorenz\\TPA-3rdplasmidconc1to1\\tea4s15w_0_003069.tif", "C:\\Analysis_from_Movie_for_RiboTrap_Dieter\\Movie_Data_Lorenz\\TPA-3rdplasmidconc1to1\\tea4s15w_0_003070.tif", "C:\\Analysis_from_Movie_for_RiboTrap_Dieter\\Movie_Data_Lorenz\\TPA-3rdplasmidconc1to1\\tea4s15w_0_003071.tif", "C:\\Analysis_from_Movie_for_RiboTrap_Dieter\\Movie_Data_Lorenz\\TPA-3rdplasmidconc1to1\\tea4s15w_0_003072.tif", "C:\\Analysis_from_Movie_for_RiboTrap_Dieter\\Movie_Data_Lorenz\\TPA-3rdplasmidconc1to1\\tea4s15w_0_003073.tif", "C:\\Analysis_from_Movie_for_RiboTrap_Dieter\\Movie_Data_Lorenz\\TPA-3rdplasmidconc1to1\\tea4s15w_0_003074.tif", "C:\\Analysis_from_Movie_for_RiboTrap_Dieter\\Movie_Data_Lorenz\\TPA-3rdplasmidconc1to1\\tea4s15w_0_003075.tif", "C:\\Analysis_from_Movie_for_RiboTrap_Dieter\\Movie_Data_Lorenz\\TPA-3rdplasmidconc1to1\\tea4s15w_0_003076.tif", "C:\\Analysis_from_Movie_for_RiboTrap_Dieter\\Movie_Data_Lorenz\\TPA-3rdplasmidconc1to1\\tea4s15w_0_003077.tif", "C:\\Analysis_from_Movie_for_RiboTrap_Dieter\\Movie_Data_Lorenz\\TPA-3rdplasmidconc1to1\\tea4s15w_0_003078.tif", "C:\\Analysis_from_Movie_for_RiboTrap_Dieter\\Movie_Data_Lorenz\\TPA-3rdplasmidconc1to1\\tea4s15w_0_003079.tif", "C:\\Analysis_from_Movie_for_RiboTrap_Dieter\\Movie_Data_Lorenz\\TPA-3rdplasmidconc1to1\\tea4s15w_0_003080.tif", "C:\\Analysis_from_Movie_for_RiboTrap_Dieter\\Movie_Data_Lorenz\\TPA-3rdplasmidconc1to1\\tea4s15w_0_003081.tif", "C:\\Analysis_from_Movie_for_RiboTrap_Dieter\\Movie_Data_Lorenz\\TPA-3rdplasmidconc1to1\\tea4s15w_0_003082.tif", "C:\\Analysis_from_Movie_for_RiboTrap_Dieter\\Movie_Data_Lorenz\\TPA-3rdplasmidconc1to1\\tea4s15w_0_003083.tif", "C:\\Analysis_from_Movie_for_RiboTrap_Dieter\\Movie_Data_Lorenz\\TPA-3rdplasmidconc1to1\\tea4s15w_0_003084.tif", "C:\\Analysis_from_Movie_for_RiboTrap_Dieter\\Movie_Data_Lorenz\\TPA-3rdplasmidconc1to1\\tea4s15w_0_003085.tif", "C:\\Analysis_from_Movie_for_RiboTrap_Dieter\\Movie_Data_Lorenz\\TPA-3rdplasmidconc1to1\\tea4s15w_0_003086.tif", "C:\\Analysis_from_Movie_for_RiboTrap_Dieter\\Movie_Data_Lorenz\\TPA-3rdplasmidconc1to1\\tea4s15w_0_003087.tif", "C:\\Analysis_from_Movie_for_RiboTrap_Dieter\\Movie_Data_Lorenz\\TPA-3rdplasmidconc1to1\\tea4s15w_0_003088.tif", "C:\\Analysis_from_Movie_for_RiboTrap_Dieter\\Movie_Data_Lorenz\\TPA-3rdplasmidconc1to1\\tea4s15w_0_003089.tif", "C:\\Analysis_from_Movie_for_RiboTrap_Dieter\\Movie_Data_Lorenz\\TPA-3rdplasmidconc1to1\\tea4s15w_0_003090.tif", "C:\\Analysis_from_Movie_for_RiboTrap_Dieter\\Movie_Data_Lorenz\\TPA-3rdplasmidconc1to1\\tea4s15w_0_003091.tif", "C:\\Analysis_from_Movie_for_RiboTrap_Dieter\\Movie_Data_Lorenz\\TPA-3rdplasmidconc1to1\\tea4s15w_0_003092.tif", "C:\\Analysis_from_Movie_for_RiboTrap_Dieter\\Movie_Data_Lorenz\\TPA-3rdplasmidconc1to1\\tea4s15w_0_003093.tif", "C:\\Analysis_from_Movie_for_RiboTrap_Dieter\\Movie_Data_Lorenz\\TPA-3rdplasmidconc1to1\\tea4s15w_0_003094.tif", "C:\\Analysis_from_Movie_for_RiboTrap_Dieter\\Movie_Data_Lorenz\\TPA-3rdplasmidconc1to1\\tea4s15w_0_003095.tif", "C:\\Analysis_from_Movie_for_RiboTrap_Dieter\\Movie_Data_Lorenz\\TPA-3rdplasmidconc1to1\\tea4s15w_0_003096.tif", "C:\\Analysis_from_Movie_for_RiboTrap_Dieter\\Movie_Data_Lorenz\\TPA-3rdplasmidconc1to1\\tea4s15w_0_003097.tif", "C:\\Analysis_from_Movie_for_RiboTrap_Dieter\\Movie_Data_Lorenz\\TPA-3rdplasmidconc1to1\\tea4s15w_0_003098.tif", "C:\\Analysis_from_Movie_for_RiboTrap_Dieter\\Movie_Data_Lorenz\\TPA-3rdplasmidconc1to1\\tea4s15w_0_003099.tif", "C:\\Analysis_from_Movie_for_RiboTrap_Dieter\\Movie_Data_Lorenz\\TPA-3rdplasmidconc1to1\\tea4s15w_0_003100.tif", "C:\\Analysis_from_Movie_for_RiboTrap_Dieter\\Movie_Data_Lorenz\\TPA-3rdplasmidconc1to1\\tea4s15w_0_003101.tif", "C:\\Analysis_from_Movie_for_RiboTrap_Dieter\\Movie_Data_Lorenz\\TPA-3rdplasmidconc1to1\\tea4s15w_0_003102.tif", "C:\\Analysis_from_Movie_for_RiboTrap_Dieter\\Movie_Data_Lorenz\\TPA-3rdplasmidconc1to1\\tea4s15w_0_003103.tif", "C:\\Analysis_from_Movie_for_RiboTrap_Dieter\\Movie_Data_Lorenz\\TPA-3rdplasmidconc1to1\\tea4s15w_0_003104.tif", "C:\\Analysis_from_Movie_for_RiboTrap_Dieter\\Movie_Data_Lorenz\\TPA-3rdplasmidconc1to1\\tea4s15w_0_003105.tif", "C:\\Analysis_from_Movie_for_RiboTrap_Dieter\\Movie_Data_Lorenz\\TPA-3rdplasmidconc1to1\\tea4s15w_0_003106.tif", "C:\\Analysis_from_Movie_for_RiboTrap_Dieter\\Movie_Data_Lorenz\\TPA-3rdplasmidconc1to1\\tea4s15w_0_003107.tif", "C:\\Analysis_from_Movie_for_RiboTrap_Dieter\\Movie_Data_Lorenz\\TPA-3rdplasmidconc1to1\\tea4s15w_0_003108.tif", "C:\\Analysis_from_Movie_for_RiboTrap_Dieter\\Movie_Data_Lorenz\\TPA-3rdplasmidconc1to1\\tea4s15w_0_003109.tif", "C:\\Analysis_from_Movie_for_RiboTrap_Dieter\\Movie_Data_Lorenz\\TPA-3rdplasmidconc1to1\\tea4s15w_0_003110.tif", "C:\\Analysis_from_Movie_for_RiboTrap_Dieter\\Movie_Data_Lorenz\\TPA-3rdplasmidconc1to1\\tea4s15w_0_003111.tif", "C:\\Analysis_from_Movie_for_RiboTrap_Dieter\\Movie_Data_Lorenz\\TPA-3rdplasmidconc1to1\\tea4s15w_0_003112.tif", "C:\\Analysis_from_Movie_for_RiboTrap_Dieter\\Movie_Data_Lorenz\\TPA-3rdplasmidconc1to1\\tea4s15w_0_003113.tif", "C:\\Analysis_from_Movie_for_RiboTrap_Dieter\\Movie_Data_Lorenz\\TPA-3rdplasmidconc1to1\\tea4s15w_0_003114.tif", "C:\\Analysis_from_Movie_for_RiboTrap_Dieter\\Movie_Data_Lorenz\\TPA-3rdplasmidconc1to1\\tea4s15w_0_003115.tif", "C:\\Analysis_from_Movie_for_RiboTrap_Dieter\\Movie_Data_Lorenz\\TPA-3rdplasmidconc1to1\\tea4s15w_0_003116.tif", "C:\\Analysis_from_Movie_for_RiboTrap_Dieter\\Movie_Data_Lorenz\\TPA-3rdplasmidconc1to1\\tea4s15w_0_003117.tif", "C:\\Analysis_from_Movie_for_RiboTrap_Dieter\\Movie_Data_Lorenz\\TPA-3rdplasmidconc1to1\\tea4s15w_0_003118.tif", "C:\\Analysis_from_Movie_for_RiboTrap_Dieter\\Movie_Data_Lorenz\\TPA-3rdplasmidconc1to1\\tea4s15w_0_003119.tif", "C:\\Analysis_from_Movie_for_RiboTrap_Dieter\\Movie_Data_Lorenz\\TPA-3rdplasmidconc1to1\\tea4s15w_0_003120.tif", "C:\\Analysis_from_Movie_for_RiboTrap_Dieter\\Movie_Data_Lorenz\\TPA-3rdplasmidconc1to1\\tea4s15w_0_003121.tif", "C:\\Analysis_from_Movie_for_RiboTrap_Dieter\\Movie_Data_Lorenz\\TPA-3rdplasmidconc1to1\\tea4s15w_0_003122.tif", "C:\\Analysis_from_Movie_for_RiboTrap_Dieter\\Movie_Data_Lorenz\\TPA-3rdplasmidconc1to1\\tea4s15w_0_003123.tif", "C:\\Analysis_from_Movie_for_RiboTrap_Dieter\\Movie_Data_Lorenz\\TPA-3rdplasmidconc1to1\\tea4s15w_0_003124.tif", "C:\\Analysis_from_Movie_for_RiboTrap_Dieter\\Movie_Data_Lorenz\\TPA-3rdplasmidconc1to1\\tea4s15w_0_003125.tif", "C:\\Analysis_from_Movie_for_RiboTrap_Dieter\\Movie_Data_Lorenz\\TPA-3rdplasmidconc1to1\\tea4s15w_0_003126.tif", "C:\\Analysis_from_Movie_for_RiboTrap_Dieter\\Movie_Data_Lorenz\\TPA-3rdplasmidconc1to1\\tea4s15w_0_003127.tif", "C:\\Analysis_from_Movie_for_RiboTrap_Dieter\\Movie_Data_Lorenz\\TPA-3rdplasmidconc1to1\\tea4s15w_0_003128.tif", "C:\\Analysis_from_Movie_for_RiboTrap_Dieter\\Movie_Data_Lorenz\\TPA-3rdplasmidconc1to1\\tea4s15w_0_003129.tif", "C:\\Analysis_from_Movie_for_RiboTrap_Dieter\\Movie_Data_Lorenz\\TPA-3rdplasmidconc1to1\\tea4s15w_0_003130.tif", "C:\\Analysis_from_Movie_for_RiboTrap_Dieter\\Movie_Data_Lorenz\\TPA-3rdplasmidconc1to1\\tea4s15w_0_003131.tif", "C:\\Analysis_from_Movie_for_RiboTrap_Dieter\\Movie_Data_Lorenz\\TPA-3rdplasmidconc1to1\\tea4s15w_0_003132.tif", "C:\\Analysis_from_Movie_for_RiboTrap_Dieter\\Movie_Data_Lorenz\\TPA-3rdplasmidconc1to1\\tea4s15w_0_003133.tif", "C:\\Analysis_from_Movie_for_RiboTrap_Dieter\\Movie_Data_Lorenz\\TPA-3rdplasmidconc1to1\\tea4s15w_0_003134.tif", "C:\\Analysis_from_Movie_for_RiboTrap_Dieter\\Movie_Data_Lorenz\\TPA-3rdplasmidconc1to1\\tea4s15w_0_003135.tif", "C:\\Analysis_from_Movie_for_RiboTrap_Dieter\\Movie_Data_Lorenz\\TPA-3rdplasmidconc1to1\\tea4s15w_0_003136.tif", "C:\\Analysis_from_Movie_for_RiboTrap_Dieter\\Movie_Data_Lorenz\\TPA-3rdplasmidconc1to1\\tea4s15w_0_003137.tif", "C:\\Analysis_from_Movie_for_RiboTrap_Dieter\\Movie_Data_Lorenz\\TPA-3rdplasmidconc1to1\\tea4s15w_0_003138.tif", "C:\\Analysis_from_Movie_for_RiboTrap_Dieter\\Movie_Data_Lorenz\\TPA-3rdplasmidconc1to1\\tea4s15w_0_003139.tif", "C:\\Analysis_from_Movie_for_RiboTrap_Dieter\\Movie_Data_Lorenz\\TPA-3rdplasmidconc1to1\\tea4s15w_0_003140.tif", "C:\\Analysis_from_Movie_for_RiboTrap_Dieter\\Movie_Data_Lorenz\\TPA-3rdplasmidconc1to1\\tea4s15w_0_003141.tif", "C:\\Analysis_from_Movie_for_RiboTrap_Dieter\\Movie_Data_Lorenz\\TPA-3rdplasmidconc1to1\\tea4s15w_0_003142.tif", "C:\\Analysis_from_Movie_for_RiboTrap_Dieter\\Movie_Data_Lorenz\\TPA-3rdplasmidconc1to1\\tea4s15w_0_003143.tif", "C:\\Analysis_from_Movie_for_RiboTrap_Dieter\\Movie_Data_Lorenz\\TPA-3rdplasmidconc1to1\\tea4s15w_0_003144.tif", "C:\\Analysis_from_Movie_for_RiboTrap_Dieter\\Movie_Data_Lorenz\\TPA-3rdplasmidconc1to1\\tea4s15w_0_003145.tif", "C:\\Analysis_from_Movie_for_RiboTrap_Dieter\\Movie_Data_Lorenz\\TPA-3rdplasmidconc1to1\\tea4s15w_0_003146.tif", "C:\\Analysis_from_Movie_for_RiboTrap_Dieter\\Movie_Data_Lorenz\\TPA-3rdplasmidconc1to1\\tea4s15w_0_003147.tif", "C:\\Analysis_from_Movie_for_RiboTrap_Dieter\\Movie_Data_Lorenz\\TPA-3rdplasmidconc1to1\\tea4s15w_0_003148.tif", "C:\\Analysis_from_Movie_for_RiboTrap_Dieter\\Movie_Data_Lorenz\\TPA-3rdplasmidconc1to1\\tea4s15w_0_003149.tif", "C:\\Analysis_from_Movie_for_RiboTrap_Dieter\\Movie_Data_Lorenz\\TPA-3rdplasmidconc1to1\\tea4s15w_0_003150.tif", "C:\\Analysis_from_Movie_for_RiboTrap_Dieter\\Movie_Data_Lorenz\\TPA-3rdplasmidconc1to1\\tea4s15w_0_003151.tif", "C:\\Analysis_from_Movie_for_RiboTrap_Dieter\\Movie_Data_Lorenz\\TPA-3rdplasmidconc1to1\\tea4s15w_0_003152.tif", "C:\\Analysis_from_Movie_for_RiboTrap_Dieter\\Movie_Data_Lorenz\\TPA-3rdplasmidconc1to1\\tea4s15w_0_003153.tif", "C:\\Analysis_from_Movie_for_RiboTrap_Dieter\\Movie_Data_Lorenz\\TPA-3rdplasmidconc1to1\\tea4s15w_0_003154.tif", "C:\\Analysis_from_Movie_for_RiboTrap_Dieter\\Movie_Data_Lorenz\\TPA-3rdplasmidconc1to1\\tea4s15w_0_003155.tif", "C:\\Analysis_from_Movie_for_RiboTrap_Dieter\\Movie_Data_Lorenz\\TPA-3rdplasmidconc1to1\\tea4s15w_0_003156.tif", "C:\\Analysis_from_Movie_for_RiboTrap_Dieter\\Movie_Data_Lorenz\\TPA-3rdplasmidconc1to1\\tea4s15w_0_003157.tif", "C:\\Analysis_from_Movie_for_RiboTrap_Dieter\\Movie_Data_Lorenz\\TPA-3rdplasmidconc1to1\\tea4s15w_0_003158.tif", "C:\\Analysis_from_Movie_for_RiboTrap_Dieter\\Movie_Data_Lorenz\\TPA-3rdplasmidconc1to1\\tea4s15w_0_003159.tif", "C:\\Analysis_from_Movie_for_RiboTrap_Dieter\\Movie_Data_Lorenz\\TPA-3rdplasmidconc1to1\\tea4s15w_0_003160.tif", "C:\\Analysis_from_Movie_for_RiboTrap_Dieter\\Movie_Data_Lorenz\\TPA-3rdplasmidconc1to1\\tea4s15w_0_003161.tif", "C:\\Analysis_from_Movie_for_RiboTrap_Dieter\\Movie_Data_Lorenz\\TPA-3rdplasmidconc1to1\\tea4s15w_0_003162.tif", "C:\\Analysis_from_Movie_for_RiboTrap_Dieter\\Movie_Data_Lorenz\\TPA-3rdplasmidconc1to1\\tea4s15w_0_003163.tif", "C:\\Analysis_from_Movie_for_RiboTrap_Dieter\\Movie_Data_Lorenz\\TPA-3rdplasmidconc1to1\\tea4s15w_0_003164.tif", "C:\\Analysis_from_Movie_for_RiboTrap_Dieter\\Movie_Data_Lorenz\\TPA-3rdplasmidconc1to1\\tea4s15w_0_003165.tif", "C:\\Analysis_from_Movie_for_RiboTrap_Dieter\\Movie_Data_Lorenz\\TPA-3rdplasmidconc1to1\\tea4s15w_0_003166.tif", "C:\\Analysis_from_Movie_for_RiboTrap_Dieter\\Movie_Data_Lorenz\\TPA-3rdplasmidconc1to1\\tea4s15w_0_003167.tif", "C:\\Analysis_from_Movie_for_RiboTrap_Dieter\\Movie_Data_Lorenz\\TPA-3rdplasmidconc1to1\\tea4s15w_0_003168.tif", "C:\\Analysis_from_Movie_for_RiboTrap_Dieter\\Movie_Data_Lorenz\\TPA-3rdplasmidconc1to1\\tea4s15w_0_003169.tif", "C:\\Analysis_from_Movie_for_RiboTrap_Dieter\\Movie_Data_Lorenz\\TPA-3rdplasmidconc1to1\\tea4s15w_0_003170.tif", "C:\\Analysis_from_Movie_for_RiboTrap_Dieter\\Movie_Data_Lorenz\\TPA-3rdplasmidconc1to1\\tea4s15w_0_003171.tif", "C:\\Analysis_from_Movie_for_RiboTrap_Dieter\\Movie_Data_Lorenz\\TPA-3rdplasmidconc1to1\\tea4s15w_0_003172.tif", "C:\\Analysis_from_Movie_for_RiboTrap_Dieter\\Movie_Data_Lorenz\\TPA-3rdplasmidconc1to1\\tea4s15w_0_003173.tif", "C:\\Analysis_from_Movie_for_RiboTrap_Dieter\\Movie_Data_Lorenz\\TPA-3rdplasmidconc1to1\\tea4s15w_0_003174.tif", "C:\\Analysis_from_Movie_for_RiboTrap_Dieter\\Movie_Data_Lorenz\\TPA-3rdplasmidconc1to1\\tea4s15w_0_003175.tif", "C:\\Analysis_from_Movie_for_RiboTrap_Dieter\\Movie_Data_Lorenz\\TPA-3rdplasmidconc1to1\\tea4s15w_0_003176.tif", "C:\\Analysis_from_Movie_for_RiboTrap_Dieter\\Movie_Data_Lorenz\\TPA-3rdplasmidconc1to1\\tea4s15w_0_003177.tif", "C:\\Analysis_from_Movie_for_RiboTrap_Dieter\\Movie_Data_Lorenz\\TPA-3rdplasmidconc1to1\\tea4s15w_0_003178.tif", "C:\\Analysis_from_Movie_for_RiboTrap_Dieter\\Movie_Data_Lorenz\\TPA-3rdplasmidconc1to1\\tea4s15w_0_003179.tif", "C:\\Analysis_from_Movie_for_RiboTrap_Dieter\\Movie_Data_Lorenz\\TPA-3rdplasmidconc1to1\\tea4s15w_0_003180.tif", "C:\\Analysis_from_Movie_for_RiboTrap_Dieter\\Movie_Data_Lorenz\\TPA-3rdplasmidconc1to1\\tea4s15w_0_003181.tif", "C:\\Analysis_from_Movie_for_RiboTrap_Dieter\\Movie_Data_Lorenz\\TPA-3rdplasmidconc1to1\\tea4s15w_0_003182.tif", "C:\\Analysis_from_Movie_for_RiboTrap_Dieter\\Movie_Data_Lorenz\\TPA-3rdplasmidconc1to1\\tea4s15w_0_003183.tif", "C:\\Analysis_from_Movie_for_RiboTrap_Dieter\\Movie_Data_Lorenz\\TPA-3rdplasmidconc1to1\\tea4s15w_0_003184.tif", "C:\\Analysis_from_Movie_for_RiboTrap_Dieter\\Movie_Data_Lorenz\\TPA-3rdplasmidconc1to1\\tea4s15w_0_003185.tif", "C:\\Analysis_from_Movie_for_RiboTrap_Dieter\\Movie_Data_Lorenz\\TPA-3rdplasmidconc1to1\\tea4s15w_0_003186.tif", "C:\\Analysis_from_Movie_for_RiboTrap_Dieter\\Movie_Data_Lorenz\\TPA-3rdplasmidconc1to1\\tea4s15w_0_003187.tif", "C:\\Analysis_from_Movie_for_RiboTrap_Dieter\\Movie_Data_Lorenz\\TPA-3rdplasmidconc1to1\\tea4s15w_0_003188.tif", "C:\\Analysis_from_Movie_for_RiboTrap_Dieter\\Movie_Data_Lorenz\\TPA-3rdplasmidconc1to1\\tea4s15w_0_003189.tif", "C:\\Analysis_from_Movie_for_RiboTrap_Dieter\\Movie_Data_Lorenz\\TPA-3rdplasmidconc1to1\\tea4s15w_0_003190.tif", "C:\\Analysis_from_Movie_for_RiboTrap_Dieter\\Movie_Data_Lorenz\\TPA-3rdplasmidconc1to1\\tea4s15w_0_003191.tif", "C:\\Analysis_from_Movie_for_RiboTrap_Dieter\\Movie_Data_Lorenz\\TPA-3rdplasmidconc1to1\\tea4s15w_0_003192.tif", "C:\\Analysis_from_Movie_for_RiboTrap_Dieter\\Movie_Data_Lorenz\\TPA-3rdplasmidconc1to1\\tea4s15w_0_003193.tif", "C:\\Analysis_from_Movie_for_RiboTrap_Dieter\\Movie_Data_Lorenz\\TPA-3rdplasmidconc1to1\\tea4s15w_0_003194.tif", "C:\\Analysis_from_Movie_for_RiboTrap_Dieter\\Movie_Data_Lorenz\\TPA-3rdplasmidconc1to1\\tea4s15w_0_003195.tif", "C:\\Analysis_from_Movie_for_RiboTrap_Dieter\\Movie_Data_Lorenz\\TPA-3rdplasmidconc1to1\\tea4s15w_0_003196.tif", "C:\\Analysis_from_Movie_for_RiboTrap_Dieter\\Movie_Data_Lorenz\\TPA-3rdplasmidconc1to1\\tea4s15w_0_003197.tif", "C:\\Analysis_from_Movie_for_RiboTrap_Dieter\\Movie_Data_Lorenz\\TPA-3rdplasmidconc1to1\\tea4s15w_0_003198.tif", "C:\\Analysis_from_Movie_for_RiboTrap_Dieter\\Movie_Data_Lorenz\\TPA-3rdplasmidconc1to1\\tea4s15w_0_003199.tif", "C:\\Analysis_from_Movie_for_RiboTrap_Dieter\\Movie_Data_Lorenz\\TPA-3rdplasmidconc1to1\\tea4s15w_0_003200.tif", "C:\\Analysis_from_Movie_for_RiboTrap_Dieter\\Movie_Data_Lorenz\\TPA-3rdplasmidconc1to1\\tea4s15w_0_003201.tif", "C:\\Analysis_from_Movie_for_RiboTrap_Dieter\\Movie_Data_Lorenz\\TPA-3rdplasmidconc1to1\\tea4s15w_0_003202.tif", "C:\\Analysis_from_Movie_for_RiboTrap_Dieter\\Movie_Data_Lorenz\\TPA-3rdplasmidconc1to1\\tea4s15w_0_003203.tif", "C:\\Analysis_from_Movie_for_RiboTrap_Dieter\\Movie_Data_Lorenz\\TPA-3rdplasmidconc1to1\\tea4s15w_0_003204.tif", "C:\\Analysis_from_Movie_for_RiboTrap_Dieter\\Movie_Data_Lorenz\\TPA-3rdplasmidconc1to1\\tea4s15w_0_003205.tif", "C:\\Analysis_from_Movie_for_RiboTrap_Dieter\\Movie_Data_Lorenz\\TPA-3rdplasmidconc1to1\\tea4s15w_0_003206.tif", "C:\\Analysis_from_Movie_for_RiboTrap_Dieter\\Movie_Data_Lorenz\\TPA-3rdplasmidconc1to1\\tea4s15w_0_003207.tif", "C:\\Analysis_from_Movie_for_RiboTrap_Dieter\\Movie_Data_Lorenz\\TPA-3rdplasmidconc1to1\\tea4s15w_0_003208.tif", "C:\\Analysis_from_Movie_for_RiboTrap_Dieter\\Movie_Data_Lorenz\\TPA-3rdplasmidconc1to1\\tea4s15w_0_003209.tif", "C:\\Analysis_from_Movie_for_RiboTrap_Dieter\\Movie_Data_Lorenz\\TPA-3rdplasmidconc1to1\\tea4s15w_0_003210.tif", "C:\\Analysis_from_Movie_for_RiboTrap_Dieter\\Movie_Data_Lorenz\\TPA-3rdplasmidconc1to1\\tea4s15w_0_003211.tif", "C:\\Analysis_from_Movie_for_RiboTrap_Dieter\\Movie_Data_Lorenz\\TPA-3rdplasmidconc1to1\\tea4s15w_0_003212.tif", "C:\\Analysis_from_Movie_for_RiboTrap_Dieter\\Movie_Data_Lorenz\\TPA-3rdplasmidconc1to1\\tea4s15w_0_003213.tif", "C:\\Analysis_from_Movie_for_RiboTrap_Dieter\\Movie_Data_Lorenz\\TPA-3rdplasmidconc1to1\\tea4s15w_0_003214.tif", "C:\\Analysis_from_Movie_for_RiboTrap_Dieter\\Movie_Data_Lorenz\\TPA-3rdplasmidconc1to1\\tea4s15w_0_003215.tif", "C:\\Analysis_from_Movie_for_RiboTrap_Dieter\\Movie_Data_Lorenz\\TPA-3rdplasmidconc1to1\\tea4s15w_0_003216.tif", "C:\\Analysis_from_Movie_for_RiboTrap_Dieter\\Movie_Data_Lorenz\\TPA-3rdplasmidconc1to1\\tea4s15w_0_003217.tif", "C:\\Analysis_from_Movie_for_RiboTrap_Dieter\\Movie_Data_Lorenz\\TPA-3rdplasmidconc1to1\\tea4s15w_0_003218.tif", "C:\\Analysis_from_Movie_for_RiboTrap_Dieter\\Movie_Data_Lorenz\\TPA-3rdplasmidconc1to1\\tea4s15w_0_003219.tif", "C:\\Analysis_from_Movie_for_RiboTrap_Dieter\\Movie_Data_Lorenz\\TPA-3rdplasmidconc1to1\\tea4s15w_0_003220.tif", "C:\\Analysis_from_Movie_for_RiboTrap_Dieter\\Movie_Data_Lorenz\\TPA-3rdplasmidconc1to1\\tea4s15w_0_003221.tif", "C:\\Analysis_from_Movie_for_RiboTrap_Dieter\\Movie_Data_Lorenz\\TPA-3rdplasmidconc1to1\\tea4s15w_0_003222.tif", "C:\\Analysis_from_Movie_for_RiboTrap_Dieter\\Movie_Data_Lorenz\\TPA-3rdplasmidconc1to1\\tea4s15w_0_003223.tif", "C:\\Analysis_from_Movie_for_RiboTrap_Dieter\\Movie_Data_Lorenz\\TPA-3rdplasmidconc1to1\\tea4s15w_0_003224.tif", "C:\\Analysis_from_Movie_for_RiboTrap_Dieter\\Movie_Data_Lorenz\\TPA-3rdplasmidconc1to1\\tea4s15w_0_003225.tif", "C:\\Analysis_from_Movie_for_RiboTrap_Dieter\\Movie_Data_Lorenz\\TPA-3rdplasmidconc1to1\\tea4s15w_0_003226.tif", "C:\\Analysis_from_Movie_for_RiboTrap_Dieter\\Movie_Data_Lorenz\\TPA-3rdplasmidconc1to1\\tea4s15w_0_003227.tif", "C:\\Analysis_from_Movie_for_RiboTrap_Dieter\\Movie_Data_Lorenz\\TPA-3rdplasmidconc1to1\\tea4s15w_0_003228.tif", "C:\\Analysis_from_Movie_for_RiboTrap_Dieter\\Movie_Data_Lorenz\\TPA-3rdplasmidconc1to1\\tea4s15w_0_003229.tif", "C:\\Analysis_from_Movie_for_RiboTrap_Dieter\\Movie_Data_Lorenz\\TPA-3rdplasmidconc1to1\\tea4s15w_0_003230.tif", "C:\\Analysis_from_Movie_for_RiboTrap_Dieter\\Movie_Data_Lorenz\\TPA-3rdplasmidconc1to1\\tea4s15w_0_003231.tif", "C:\\Analysis_from_Movie_for_RiboTrap_Dieter\\Movie_Data_Lorenz\\TPA-3rdplasmidconc1to1\\tea4s15w_0_003232.tif", "C:\\Analysis_from_Movie_for_RiboTrap_Dieter\\Movie_Data_Lorenz\\TPA-3rdplasmidconc1to1\\tea4s15w_0_003233.tif", "C:\\Analysis_from_Movie_for_RiboTrap_Dieter\\Movie_Data_Lorenz\\TPA-3rdplasmidconc1to1\\tea4s15w_0_003234.tif", "C:\\Analysis_from_Movie_for_RiboTrap_Dieter\\Movie_Data_Lorenz\\TPA-3rdplasmidconc1to1\\tea4s15w_0_003235.tif", "C:\\Analysis_from_Movie_for_RiboTrap_Dieter\\Movie_Data_Lorenz\\TPA-3rdplasmidconc1to1\\tea4s15w_0_003236.tif", "C:\\Analysis_from_Movie_for_RiboTrap_Dieter\\Movie_Data_Lorenz\\TPA-3rdplasmidconc1to1\\tea4s15w_0_003237.tif", "C:\\Analysis_from_Movie_for_RiboTrap_Dieter\\Movie_Data_Lorenz\\TPA-3rdplasmidconc1to1\\tea4s15w_0_003238.tif", "C:\\Analysis_from_Movie_for_RiboTrap_Dieter\\Movie_Data_Lorenz\\TPA-3rdplasmidconc1to1\\tea4s15w_0_003239.tif", "C:\\Analysis_from_Movie_for_RiboTrap_Dieter\\Movie_Data_Lorenz\\TPA-3rdplasmidconc1to1\\tea4s15w_0_003240.tif", "C:\\Analysis_from_Movie_for_RiboTrap_Dieter\\Movie_Data_Lorenz\\TPA-3rdplasmidconc1to1\\tea4s15w_0_003241.tif", "C:\\Analysis_from_Movie_for_RiboTrap_Dieter\\Movie_Data_Lorenz\\TPA-3rdplasmidconc1to1\\tea4s15w_0_003242.tif", "C:\\Analysis_from_Movie_for_RiboTrap_Dieter\\Movie_Data_Lorenz\\TPA-3rdplasmidconc1to1\\tea4s15w_0_003243.tif", "C:\\Analysis_from_Movie_for_RiboTrap_Dieter\\Movie_Data_Lorenz\\TPA-3rdplasmidconc1to1\\tea4s15w_0_003244.tif", "C:\\Analysis_from_Movie_for_RiboTrap_Dieter\\Movie_Data_Lorenz\\TPA-3rdplasmidconc1to1\\tea4s15w_0_003245.tif", "C:\\Analysis_from_Movie_for_RiboTrap_Dieter\\Movie_Data_Lorenz\\TPA-3rdplasmidconc1to1\\tea4s15w_0_003246.tif", "C:\\Analysis_from_Movie_for_RiboTrap_Dieter\\Movie_Data_Lorenz\\TPA-3rdplasmidconc1to1\\tea4s15w_0_003247.tif", "C:\\Analysis_from_Movie_for_RiboTrap_Dieter\\Movie_Data_Lorenz\\TPA-3rdplasmidconc1to1\\tea4s15w_0_003248.tif", "C:\\Analysis_from_Movie_for_RiboTrap_Dieter\\Movie_Data_Lorenz\\TPA-3rdplasmidconc1to1\\tea4s15w_0_003249.tif", "C:\\Analysis_from_Movie_for_RiboTrap_Dieter\\Movie_Data_Lorenz\\TPA-3rdplasmidconc1to1\\tea4s15w_0_003250.tif", "C:\\Analysis_from_Movie_for_RiboTrap_Dieter\\Movie_Data_Lorenz\\TPA-3rdplasmidconc1to1\\tea4s15w_0_003251.tif", "C:\\Analysis_from_Movie_for_RiboTrap_Dieter\\Movie_Data_Lorenz\\TPA-3rdplasmidconc1to1\\tea4s15w_0_003252.tif", "C:\\Analysis_from_Movie_for_RiboTrap_Dieter\\Movie_Data_Lorenz\\TPA-3rdplasmidconc1to1\\tea4s15w_0_003253.tif", "C:\\Analysis_from_Movie_for_RiboTrap_Dieter\\Movie_Data_Lorenz\\TPA-3rdplasmidconc1to1\\tea4s15w_0_003254.tif", "C:\\Analysis_from_Movie_for_RiboTrap_Dieter\\Movie_Data_Lorenz\\TPA-3rdplasmidconc1to1\\tea4s15w_0_003255.tif", "C:\\Analysis_from_Movie_for_RiboTrap_Dieter\\Movie_Data_Lorenz\\TPA-3rdplasmidconc1to1\\tea4s15w_0_003256.tif", "C:\\Analysis_from_Movie_for_RiboTrap_Dieter\\Movie_Data_Lorenz\\TPA-3rdplasmidconc1to1\\tea4s15w_0_003257.tif", "C:\\Analysis_from_Movie_for_RiboTrap_Dieter\\Movie_Data_Lorenz\\TPA-3rdplasmidconc1to1\\tea4s15w_0_003258.tif", "C:\\Analysis_from_Movie_for_RiboTrap_Dieter\\Movie_Data_Lorenz\\TPA-3rdplasmidconc1to1\\tea4s15w_0_003259.tif", "C:\\Analysis_from_Movie_for_RiboTrap_Dieter\\Movie_Data_Lorenz\\TPA-3rdplasmidconc1to1\\tea4s15w_0_003260.tif", "C:\\Analysis_from_Movie_for_RiboTrap_Dieter\\Movie_Data_Lorenz\\TPA-3rdplasmidconc1to1\\tea4s15w_0_003261.tif", "C:\\Analysis_from_Movie_for_RiboTrap_Dieter\\Movie_Data_Lorenz\\TPA-3rdplasmidconc1to1\\tea4s15w_0_003262.tif", "C:\\Analysis_from_Movie_for_RiboTrap_Dieter\\Movie_Data_Lorenz\\TPA-3rdplasmidconc1to1\\tea4s15w_0_003263.tif", "C:\\Analysis_from_Movie_for_RiboTrap_Dieter\\Movie_Data_Lorenz\\TPA-3rdplasmidconc1to1\\tea4s15w_0_003264.tif", "C:\\Analysis_from_Movie_for_RiboTrap_Dieter\\Movie_Data_Lorenz\\TPA-3rdplasmidconc1to1\\tea4s15w_0_003265.tif", "C:\\Analysis_from_Movie_for_RiboTrap_Dieter\\Movie_Data_Lorenz\\TPA-3rdplasmidconc1to1\\tea4s15w_0_003266.tif", "C:\\Analysis_from_Movie_for_RiboTrap_Dieter\\Movie_Data_Lorenz\\TPA-3rdplasmidconc1to1\\tea4s15w_0_003267.tif", "C:\\Analysis_from_Movie_for_RiboTrap_Dieter\\Movie_Data_Lorenz\\TPA-3rdplasmidconc1to1\\tea4s15w_0_003268.tif", "C:\\Analysis_from_Movie_for_RiboTrap_Dieter\\Movie_Data_Lorenz\\TPA-3rdplasmidconc1to1\\tea4s15w_0_003269.tif", "C:\\Analysis_from_Movie_for_RiboTrap_Dieter\\Movie_Data_Lorenz\\TPA-3rdplasmidconc1to1\\tea4s15w_0_003270.tif", "C:\\Analysis_from_Movie_for_RiboTrap_Dieter\\Movie_Data_Lorenz\\TPA-3rdplasmidconc1to1\\tea4s15w_0_003271.tif", "C:\\Analysis_from_Movie_for_RiboTrap_Dieter\\Movie_Data_Lorenz\\TPA-3rdplasmidconc1to1\\tea4s15w_0_003272.tif", "C:\\Analysis_from_Movie_for_RiboTrap_Dieter\\Movie_Data_Lorenz\\TPA-3rdplasmidconc1to1\\tea4s15w_0_003273.tif", "C:\\Analysis_from_Movie_for_RiboTrap_Dieter\\Movie_Data_Lorenz\\TPA-3rdplasmidconc1to1\\tea4s15w_0_003274.tif", "C:\\Analysis_from_Movie_for_RiboTrap_Dieter\\Movie_Data_Lorenz\\TPA-3rdplasmidconc1to1\\tea4s15w_0_003275.tif", "C:\\Analysis_from_Movie_for_RiboTrap_Dieter\\Movie_Data_Lorenz\\TPA-3rdplasmidconc1to1\\tea4s15w_0_003276.tif", "C:\\Analysis_from_Movie_for_RiboTrap_Dieter\\Movie_Data_Lorenz\\TPA-3rdplasmidconc1to1\\tea4s15w_0_003277.tif", "C:\\Analysis_from_Movie_for_RiboTrap_Dieter\\Movie_Data_Lorenz\\TPA-3rdplasmidconc1to1\\tea4s15w_0_003278.tif", "C:\\Analysis_from_Movie_for_RiboTrap_Dieter\\Movie_Data_Lorenz\\TPA-3rdplasmidconc1to1\\tea4s15w_0_003279.tif", "C:\\Analysis_from_Movie_for_RiboTrap_Dieter\\Movie_Data_Lorenz\\TPA-3rdplasmidconc1to1\\tea4s15w_0_003280.tif", "C:\\Analysis_from_Movie_for_RiboTrap_Dieter\\Movie_Data_Lorenz\\TPA-3rdplasmidconc1to1\\tea4s15w_0_003281.tif", "C:\\Analysis_from_Movie_for_RiboTrap_Dieter\\Movie_Data_Lorenz\\TPA-3rdplasmidconc1to1\\tea4s15w_0_003282.tif", "C:\\Analysis_from_Movie_for_RiboTrap_Dieter\\Movie_Data_Lorenz\\TPA-3rdplasmidconc1to1\\tea4s15w_0_003283.tif", "C:\\Analysis_from_Movie_for_RiboTrap_Dieter\\Movie_Data_Lorenz\\TPA-3rdplasmidconc1to1\\tea4s15w_0_003284.tif", "C:\\Analysis_from_Movie_for_RiboTrap_Dieter\\Movie_Data_Lorenz\\TPA-3rdplasmidconc1to1\\tea4s15w_0_003285.tif", "C:\\Analysis_from_Movie_for_RiboTrap_Dieter\\Movie_Data_Lorenz\\TPA-3rdplasmidconc1to1\\tea4s15w_0_003286.tif", "C:\\Analysis_from_Movie_for_RiboTrap_Dieter\\Movie_Data_Lorenz\\TPA-3rdplasmidconc1to1\\tea4s15w_0_003287.tif", "C:\\Analysis_from_Movie_for_RiboTrap_Dieter\\Movie_Data_Lorenz\\TPA-3rdplasmidconc1to1\\tea4s15w_0_003288.tif", "C:\\Analysis_from_Movie_for_RiboTrap_Dieter\\Movie_Data_Lorenz\\TPA-3rdplasmidconc1to1\\tea4s15w_0_003289.tif", "C:\\Analysis_from_Movie_for_RiboTrap_Dieter\\Movie_Data_Lorenz\\TPA-3rdplasmidconc1to1\\tea4s15w_0_003290.tif", "C:\\Analysis_from_Movie_for_RiboTrap_Dieter\\Movie_Data_Lorenz\\TPA-3rdplasmidconc1to1\\tea4s15w_0_003291.tif", "C:\\Analysis_from_Movie_for_RiboTrap_Dieter\\Movie_Data_Lorenz\\TPA-3rdplasmidconc1to1\\tea4s15w_0_003292.tif", "C:\\Analysis_from_Movie_for_RiboTrap_Dieter\\Movie_Data_Lorenz\\TPA-3rdplasmidconc1to1\\tea4s15w_0_003293.tif", "C:\\Analysis_from_Movie_for_RiboTrap_Dieter\\Movie_Data_Lorenz\\TPA-3rdplasmidconc1to1\\tea4s15w_0_003294.tif", "C:\\Analysis_from_Movie_for_RiboTrap_Dieter\\Movie_Data_Lorenz\\TPA-3rdplasmidconc1to1\\tea4s15w_0_003295.tif", "C:\\Analysis_from_Movie_for_RiboTrap_Dieter\\Movie_Data_Lorenz\\TPA-3rdplasmidconc1to1\\tea4s15w_0_003296.tif", "C:\\Analysis_from_Movie_for_RiboTrap_Dieter\\Movie_Data_Lorenz\\TPA-3rdplasmidconc1to1\\tea4s15w_0_003297.tif", "C:\\Analysis_from_Movie_for_RiboTrap_Dieter\\Movie_Data_Lorenz\\TPA-3rdplasmidconc1to1\\tea4s15w_0_003298.tif", "C:\\Analysis_from_Movie_for_RiboTrap_Dieter\\Movie_Data_Lorenz\\TPA-3rdplasmidconc1to1\\tea4s15w_0_003299.tif", "C:\\Analysis_from_Movie_for_RiboTrap_Dieter\\Movie_Data_Lorenz\\TPA-3rdplasmidconc1to1\\tea4s15w_0_003300.tif", "C:\\Analysis_from_Movie_for_RiboTrap_Dieter\\Movie_Data_Lorenz\\TPA-3rdplasmidconc1to1\\tea4s15w_0_003301.tif", "C:\\Analysis_from_Movie_for_RiboTrap_Dieter\\Movie_Data_Lorenz\\TPA-3rdplasmidconc1to1\\tea4s15w_0_003302.tif", "C:\\Analysis_from_Movie_for_RiboTrap_Dieter\\Movie_Data_Lorenz\\TPA-3rdplasmidconc1to1\\tea4s15w_0_003303.tif", "C:\\Analysis_from_Movie_for_RiboTrap_Dieter\\Movie_Data_Lorenz\\TPA-3rdplasmidconc1to1\\tea4s15w_0_003304.tif", "C:\\Analysis_from_Movie_for_RiboTrap_Dieter\\Movie_Data_Lorenz\\TPA-3rdplasmidconc1to1\\tea4s15w_0_003305.tif", "C:\\Analysis_from_Movie_for_RiboTrap_Dieter\\Movie_Data_Lorenz\\TPA-3rdplasmidconc1to1\\tea4s15w_0_003306.tif", "C:\\Analysis_from_Movie_for_RiboTrap_Dieter\\Movie_Data_Lorenz\\TPA-3rdplasmidconc1to1\\tea4s15w_0_003307.tif", "C:\\Analysis_from_Movie_for_RiboTrap_Dieter\\Movie_Data_Lorenz\\TPA-3rdplasmidconc1to1\\tea4s15w_0_003308.tif", "C:\\Analysis_from_Movie_for_RiboTrap_Dieter\\Movie_Data_Lorenz\\TPA-3rdplasmidconc1to1\\tea4s15w_0_003309.tif", "C:\\Analysis_from_Movie_for_RiboTrap_Dieter\\Movie_Data_Lorenz\\TPA-3rdplasmidconc1to1\\tea4s15w_0_003310.tif", "C:\\Analysis_from_Movie_for_RiboTrap_Dieter\\Movie_Data_Lorenz\\TPA-3rdplasmidconc1to1\\tea4s15w_0_003311.tif", "C:\\Analysis_from_Movie_for_RiboTrap_Dieter\\Movie_Data_Lorenz\\TPA-3rdplasmidconc1to1\\tea4s15w_0_003312.tif", "C:\\Analysis_from_Movie_for_RiboTrap_Dieter\\Movie_Data_Lorenz\\TPA-3rdplasmidconc1to1\\tea4s15w_0_003313.tif", "C:\\Analysis_from_Movie_for_RiboTrap_Dieter\\Movie_Data_Lorenz\\TPA-3rdplasmidconc1to1\\tea4s15w_0_003314.tif", "C:\\Analysis_from_Movie_for_RiboTrap_Dieter\\Movie_Data_Lorenz\\TPA-3rdplasmidconc1to1\\tea4s15w_0_003315.tif", "C:\\Analysis_from_Movie_for_RiboTrap_Dieter\\Movie_Data_Lorenz\\TPA-3rdplasmidconc1to1\\tea4s15w_0_003316.tif", "C:\\Analysis_from_Movie_for_RiboTrap_Dieter\\Movie_Data_Lorenz\\TPA-3rdplasmidconc1to1\\tea4s15w_0_003317.tif", "C:\\Analysis_from_Movie_for_RiboTrap_Dieter\\Movie_Data_Lorenz\\TPA-3rdplasmidconc1to1\\tea4s15w_0_003318.tif", "C:\\Analysis_from_Movie_for_RiboTrap_Dieter\\Movie_Data_Lorenz\\TPA-3rdplasmidconc1to1\\tea4s15w_0_003319.tif", "C:\\Analysis_from_Movie_for_RiboTrap_Dieter\\Movie_Data_Lorenz\\TPA-3rdplasmidconc1to1\\tea4s15w_0_003320.tif", "C:\\Analysis_from_Movie_for_RiboTrap_Dieter\\Movie_Data_Lorenz\\TPA-3rdplasmidconc1to1\\tea4s15w_0_003321.tif", "C:\\Analysis_from_Movie_for_RiboTrap_Dieter\\Movie_Data_Lorenz\\TPA-3rdplasmidconc1to1\\tea4s15w_0_003322.tif", "C:\\Analysis_from_Movie_for_RiboTrap_Dieter\\Movie_Data_Lorenz\\TPA-3rdplasmidconc1to1\\tea4s15w_0_003323.tif", "C:\\Analysis_from_Movie_for_RiboTrap_Dieter\\Movie_Data_Lorenz\\TPA-3rdplasmidconc1to1\\tea4s15w_0_003324.tif", "C:\\Analysis_from_Movie_for_RiboTrap_Dieter\\Movie_Data_Lorenz\\TPA-3rdplasmidconc1to1\\tea4s15w_0_003325.tif", "C:\\Analysis_from_Movie_for_RiboTrap_Dieter\\Movie_Data_Lorenz\\TPA-3rdplasmidconc1to1\\tea4s15w_0_003326.tif", "C:\\Analysis_from_Movie_for_RiboTrap_Dieter\\Movie_Data_Lorenz\\TPA-3rdplasmidconc1to1\\tea4s15w_0_003327.tif", "C:\\Analysis_from_Movie_for_RiboTrap_Dieter\\Movie_Data_Lorenz\\TPA-3rdplasmidconc1to1\\tea4s15w_0_003328.tif", "C:\\Analysis_from_Movie_for_RiboTrap_Dieter\\Movie_Data_Lorenz\\TPA-3rdplasmidconc1to1\\tea4s15w_0_003329.tif", "C:\\Analysis_from_Movie_for_RiboTrap_Dieter\\Movie_Data_Lorenz\\TPA-3rdplasmidconc1to1\\tea4s15w_0_003330.tif", "C:\\Analysis_from_Movie_for_RiboTrap_Dieter\\Movie_Data_Lorenz\\TPA-3rdplasmidconc1to1\\tea4s15w_0_003331.tif", "C:\\Analysis_from_Movie_for_RiboTrap_Dieter\\Movie_Data_Lorenz\\TPA-3rdplasmidconc1to1\\tea4s15w_0_003332.tif", "C:\\Analysis_from_Movie_for_RiboTrap_Dieter\\Movie_Data_Lorenz\\TPA-3rdplasmidconc1to1\\tea4s15w_0_003333.tif", "C:\\Analysis_from_Movie_for_RiboTrap_Dieter\\Movie_Data_Lorenz\\TPA-3rdplasmidconc1to1\\tea4s15w_0_003334.tif", "C:\\Analysis_from_Movie_for_RiboTrap_Dieter\\Movie_Data_Lorenz\\TPA-3rdplasmidconc1to1\\tea4s15w_0_003335.tif", "C:\\Analysis_from_Movie_for_RiboTrap_Dieter\\Movie_Data_Lorenz\\TPA-3rdplasmidconc1to1\\tea4s15w_0_003336.tif", "C:\\Analysis_from_Movie_for_RiboTrap_Dieter\\Movie_Data_Lorenz\\TPA-3rdplasmidconc1to1\\tea4s15w_0_003337.tif", "C:\\Analysis_from_Movie_for_RiboTrap_Dieter\\Movie_Data_Lorenz\\TPA-3rdplasmidconc1to1\\tea4s15w_0_003338.tif", "C:\\Analysis_from_Movie_for_RiboTrap_Dieter\\Movie_Data_Lorenz\\TPA-3rdplasmidconc1to1\\tea4s15w_0_003339.tif", "C:\\Analysis_from_Movie_for_RiboTrap_Dieter\\Movie_Data_Lorenz\\TPA-3rdplasmidconc1to1\\tea4s15w_0_003340.tif", "C:\\Analysis_from_Movie_for_RiboTrap_Dieter\\Movie_Data_Lorenz\\TPA-3rdplasmidconc1to1\\tea4s15w_0_003341.tif", "C:\\Analysis_from_Movie_for_RiboTrap_Dieter\\Movie_Data_Lorenz\\TPA-3rdplasmidconc1to1\\tea4s15w_0_003342.tif", "C:\\Analysis_from_Movie_for_RiboTrap_Dieter\\Movie_Data_Lorenz\\TPA-3rdplasmidconc1to1\\tea4s15w_0_003343.tif", "C:\\Analysis_from_Movie_for_RiboTrap_Dieter\\Movie_Data_Lorenz\\TPA-3rdplasmidconc1to1\\tea4s15w_0_003344.tif", "C:\\Analysis_from_Movie_for_RiboTrap_Dieter\\Movie_Data_Lorenz\\TPA-3rdplasmidconc1to1\\tea4s15w_0_003345.tif", "C:\\Analysis_from_Movie_for_RiboTrap_Dieter\\Movie_Data_Lorenz\\TPA-3rdplasmidconc1to1\\tea4s15w_0_003346.tif", "C:\\Analysis_from_Movie_for_RiboTrap_Dieter\\Movie_Data_Lorenz\\TPA-3rdplasmidconc1to1\\tea4s15w_0_003347.tif", "C:\\Analysis_from_Movie_for_RiboTrap_Dieter\\Movie_Data_Lorenz\\TPA-3rdplasmidconc1to1\\tea4s15w_0_003348.tif", "C:\\Analysis_from_Movie_for_RiboTrap_Dieter\\Movie_Data_Lorenz\\TPA-3rdplasmidconc1to1\\tea4s15w_0_003349.tif", "C:\\Analysis_from_Movie_for_RiboTrap_Dieter\\Movie_Data_Lorenz\\TPA-3rdplasmidconc1to1\\tea4s15w_0_003350.tif", "C:\\Analysis_from_Movie_for_RiboTrap_Dieter\\Movie_Data_Lorenz\\TPA-3rdplasmidconc1to1\\tea4s15w_0_003351.tif", "C:\\Analysis_from_Movie_for_RiboTrap_Dieter\\Movie_Data_Lorenz\\TPA-3rdplasmidconc1to1\\tea4s15w_0_003352.tif", "C:\\Analysis_from_Movie_for_RiboTrap_Dieter\\Movie_Data_Lorenz\\TPA-3rdplasmidconc1to1\\tea4s15w_0_003353.tif", "C:\\Analysis_from_Movie_for_RiboTrap_Dieter\\Movie_Data_Lorenz\\TPA-3rdplasmidconc1to1\\tea4s15w_0_003354.tif", "C:\\Analysis_from_Movie_for_RiboTrap_Dieter\\Movie_Data_Lorenz\\TPA-3rdplasmidconc1to1\\tea4s15w_0_003355.tif", "C:\\Analysis_from_Movie_for_RiboTrap_Dieter\\Movie_Data_Lorenz\\TPA-3rdplasmidconc1to1\\tea4s15w_0_003356.tif", "C:\\Analysis_from_Movie_for_RiboTrap_Dieter\\Movie_Data_Lorenz\\TPA-3rdplasmidconc1to1\\tea4s15w_0_003357.tif", "C:\\Analysis_from_Movie_for_RiboTrap_Dieter\\Movie_Data_Lorenz\\TPA-3rdplasmidconc1to1\\tea4s15w_0_003358.tif", "C:\\Analysis_from_Movie_for_RiboTrap_Dieter\\Movie_Data_Lorenz\\TPA-3rdplasmidconc1to1\\tea4s15w_0_003359.tif", "C:\\Analysis_from_Movie_for_RiboTrap_Dieter\\Movie_Data_Lorenz\\TPA-3rdplasmidconc1to1\\tea4s15w_0_003360.tif", "C:\\Analysis_from_Movie_for_RiboTrap_Dieter\\Movie_Data_Lorenz\\TPA-3rdplasmidconc1to1\\tea4s15w_0_003361.tif", "C:\\Analysis_from_Movie_for_RiboTrap_Dieter\\Movie_Data_Lorenz\\TPA-3rdplasmidconc1to1\\tea4s15w_0_003362.tif", "C:\\Analysis_from_Movie_for_RiboTrap_Dieter\\Movie_Data_Lorenz\\TPA-3rdplasmidconc1to1\\tea4s15w_0_003363.tif", "C:\\Analysis_from_Movie_for_RiboTrap_Dieter\\Movie_Data_Lorenz\\TPA-3rdplasmidconc1to1\\tea4s15w_0_003364.tif", "C:\\Analysis_from_Movie_for_RiboTrap_Dieter\\Movie_Data_Lorenz\\TPA-3rdplasmidconc1to1\\tea4s15w_0_003365.tif", "C:\\Analysis_from_Movie_for_RiboTrap_Dieter\\Movie_Data_Lorenz\\TPA-3rdplasmidconc1to1\\tea4s15w_0_003366.tif", "C:\\Analysis_from_Movie_for_RiboTrap_Dieter\\Movie_Data_Lorenz\\TPA-3rdplasmidconc1to1\\tea4s15w_0_003367.tif", "C:\\Analysis_from_Movie_for_RiboTrap_Dieter\\Movie_Data_Lorenz\\TPA-3rdplasmidconc1to1\\tea4s15w_0_003368.tif", "C:\\Analysis_from_Movie_for_RiboTrap_Dieter\\Movie_Data_Lorenz\\TPA-3rdplasmidconc1to1\\tea4s15w_0_003369.tif", "C:\\Analysis_from_Movie_for_RiboTrap_Dieter\\Movie_Data_Lorenz\\TPA-3rdplasmidconc1to1\\tea4s15w_0_003370.tif", "C:\\Analysis_from_Movie_for_RiboTrap_Dieter\\Movie_Data_Lorenz\\TPA-3rdplasmidconc1to1\\tea4s15w_0_003371.tif", "C:\\Analysis_from_Movie_for_RiboTrap_Dieter\\Movie_Data_Lorenz\\TPA-3rdplasmidconc1to1\\tea4s15w_0_003372.tif", "C:\\Analysis_from_Movie_for_RiboTrap_Dieter\\Movie_Data_Lorenz\\TPA-3rdplasmidconc1to1\\tea4s15w_0_003373.tif", "C:\\Analysis_from_Movie_for_RiboTrap_Dieter\\Movie_Data_Lorenz\\TPA-3rdplasmidconc1to1\\tea4s15w_0_003374.tif", "C:\\Analysis_from_Movie_for_RiboTrap_Dieter\\Movie_Data_Lorenz\\TPA-3rdplasmidconc1to1\\tea4s15w_0_003375.tif", "C:\\Analysis_from_Movie_for_RiboTrap_Dieter\\Movie_Data_Lorenz\\TPA-3rdplasmidconc1to1\\tea4s15w_0_003376.tif", "C:\\Analysis_from_Movie_for_RiboTrap_Dieter\\Movie_Data_Lorenz\\TPA-3rdplasmidconc1to1\\tea4s15w_0_003377.tif", "C:\\Analysis_from_Movie_for_RiboTrap_Dieter\\Movie_Data_Lorenz\\TPA-3rdplasmidconc1to1\\tea4s15w_0_003378.tif", "C:\\Analysis_from_Movie_for_RiboTrap_Dieter\\Movie_Data_Lorenz\\TPA-3rdplasmidconc1to1\\tea4s15w_0_003379.tif", "C:\\Analysis_from_Movie_for_RiboTrap_Dieter\\Movie_Data_Lorenz\\TPA-3rdplasmidconc1to1\\tea4s15w_0_003380.tif", "C:\\Analysis_from_Movie_for_RiboTrap_Dieter\\Movie_Data_Lorenz\\TPA-3rdplasmidconc1to1\\tea4s15w_0_003381.tif", "C:\\Analysis_from_Movie_for_RiboTrap_Dieter\\Movie_Data_Lorenz\\TPA-3rdplasmidconc1to1\\tea4s15w_0_003382.tif", "C:\\Analysis_from_Movie_for_RiboTrap_Dieter\\Movie_Data_Lorenz\\TPA-3rdplasmidconc1to1\\tea4s15w_0_003383.tif", "C:\\Analysis_from_Movie_for_RiboTrap_Dieter\\Movie_Data_Lorenz\\TPA-3rdplasmidconc1to1\\tea4s15w_0_003384.tif", "C:\\Analysis_from_Movie_for_RiboTrap_Dieter\\Movie_Data_Lorenz\\TPA-3rdplasmidconc1to1\\tea4s15w_0_003385.tif", "C:\\Analysis_from_Movie_for_RiboTrap_Dieter\\Movie_Data_Lorenz\\TPA-3rdplasmidconc1to1\\tea4s15w_0_003386.tif", "C:\\Analysis_from_Movie_for_RiboTrap_Dieter\\Movie_Data_Lorenz\\TPA-3rdplasmidconc1to1\\tea4s15w_0_003387.tif", "C:\\Analysis_from_Movie_for_RiboTrap_Dieter\\Movie_Data_Lorenz\\TPA-3rdplasmidconc1to1\\tea4s15w_0_003388.tif", "C:\\Analysis_from_Movie_for_RiboTrap_Dieter\\Movie_Data_Lorenz\\TPA-3rdplasmidconc1to1\\tea4s15w_0_003389.tif", "C:\\Analysis_from_Movie_for_RiboTrap_Dieter\\Movie_Data_Lorenz\\TPA-3rdplasmidconc1to1\\tea4s15w_0_003390.tif", "C:\\Analysis_from_Movie_for_RiboTrap_Dieter\\Movie_Data_Lorenz\\TPA-3rdplasmidconc1to1\\tea4s15w_0_003391.tif", "C:\\Analysis_from_Movie_for_RiboTrap_Dieter\\Movie_Data_Lorenz\\TPA-3rdplasmidconc1to1\\tea4s15w_0_003392.tif", "C:\\Analysis_from_Movie_for_RiboTrap_Dieter\\Movie_Data_Lorenz\\TPA-3rdplasmidconc1to1\\tea4s15w_0_003393.tif", "C:\\Analysis_from_Movie_for_RiboTrap_Dieter\\Movie_Data_Lorenz\\TPA-3rdplasmidconc1to1\\tea4s15w_0_003394.tif", "C:\\Analysis_from_Movie_for_RiboTrap_Dieter\\Movie_Data_Lorenz\\TPA-3rdplasmidconc1to1\\tea4s15w_0_003395.tif", "C:\\Analysis_from_Movie_for_RiboTrap_Dieter\\Movie_Data_Lorenz\\TPA-3rdplasmidconc1to1\\tea4s15w_0_003396.tif", "C:\\Analysis_from_Movie_for_RiboTrap_Dieter\\Movie_Data_Lorenz\\TPA-3rdplasmidconc1to1\\tea4s15w_0_003397.tif", "C:\\Analysis_from_Movie_for_RiboTrap_Dieter\\Movie_Data_Lorenz\\TPA-3rdplasmidconc1to1\\tea4s15w_0_003398.tif", "C:\\Analysis_from_Movie_for_RiboTrap_Dieter\\Movie_Data_Lorenz\\TPA-3rdplasmidconc1to1\\tea4s15w_0_003399.tif", "C:\\Analysis_from_Movie_for_RiboTrap_Dieter\\Movie_Data_Lorenz\\TPA-3rdplasmidconc1to1\\tea4s15w_0_003400.tif", "C:\\Analysis_from_Movie_for_RiboTrap_Dieter\\Movie_Data_Lorenz\\TPA-3rdplasmidconc1to1\\tea4s15w_0_003401.tif", "C:\\Analysis_from_Movie_for_RiboTrap_Dieter\\Movie_Data_Lorenz\\TPA-3rdplasmidconc1to1\\tea4s15w_0_003402.tif", "C:\\Analysis_from_Movie_for_RiboTrap_Dieter\\Movie_Data_Lorenz\\TPA-3rdplasmidconc1to1\\tea4s15w_0_003403.tif", "C:\\Analysis_from_Movie_for_RiboTrap_Dieter\\Movie_Data_Lorenz\\TPA-3rdplasmidconc1to1\\tea4s15w_0_003404.tif", "C:\\Analysis_from_Movie_for_RiboTrap_Dieter\\Movie_Data_Lorenz\\TPA-3rdplasmidconc1to1\\tea4s15w_0_003405.tif", "C:\\Analysis_from_Movie_for_RiboTrap_Dieter\\Movie_Data_Lorenz\\TPA-3rdplasmidconc1to1\\tea4s15w_0_003406.tif", "C:\\Analysis_from_Movie_for_RiboTrap_Dieter\\Movie_Data_Lorenz\\TPA-3rdplasmidconc1to1\\tea4s15w_0_003407.tif", "C:\\Analysis_from_Movie_for_RiboTrap_Dieter\\Movie_Data_Lorenz\\TPA-3rdplasmidconc1to1\\tea4s15w_0_003408.tif", "C:\\Analysis_from_Movie_for_RiboTrap_Dieter\\Movie_Data_Lorenz\\TPA-3rdplasmidconc1to1\\tea4s15w_0_003409.tif", "C:\\Analysis_from_Movie_for_RiboTrap_Dieter\\Movie_Data_Lorenz\\TPA-3rdplasmidconc1to1\\tea4s15w_0_003410.tif", "C:\\Analysis_from_Movie_for_RiboTrap_Dieter\\Movie_Data_Lorenz\\TPA-3rdplasmidconc1to1\\tea4s15w_0_003411.tif", "C:\\Analysis_from_Movie_for_RiboTrap_Dieter\\Movie_Data_Lorenz\\TPA-3rdplasmidconc1to1\\tea4s15w_0_003412.tif", "C:\\Analysis_from_Movie_for_RiboTrap_Dieter\\Movie_Data_Lorenz\\TPA-3rdplasmidconc1to1\\tea4s15w_0_003413.tif", "C:\\Analysis_from_Movie_for_RiboTrap_Dieter\\Movie_Data_Lorenz\\TPA-3rdplasmidconc1to1\\tea4s15w_0_003414.tif", "C:\\Analysis_from_Movie_for_RiboTrap_Dieter\\Movie_Data_Lorenz\\TPA-3rdplasmidconc1to1\\tea4s15w_0_003415.tif", "C:\\Analysis_from_Movie_for_RiboTrap_Dieter\\Movie_Data_Lorenz\\TPA-3rdplasmidconc1to1\\tea4s15w_0_003416.tif", "C:\\Analysis_from_Movie_for_RiboTrap_Dieter\\Movie_Data_Lorenz\\TPA-3rdplasmidconc1to1\\tea4s15w_0_003417.tif", "C:\\Analysis_from_Movie_for_RiboTrap_Dieter\\Movie_Data_Lorenz\\TPA-3rdplasmidconc1to1\\tea4s15w_0_003418.tif", "C:\\Analysis_from_Movie_for_RiboTrap_Dieter\\Movie_Data_Lorenz\\TPA-3rdplasmidconc1to1\\tea4s15w_0_003419.tif", "C:\\Analysis_from_Movie_for_RiboTrap_Dieter\\Movie_Data_Lorenz\\TPA-3rdplasmidconc1to1\\tea4s15w_0_003420.tif", "C:\\Analysis_from_Movie_for_RiboTrap_Dieter\\Movie_Data_Lorenz\\TPA-3rdplasmidconc1to1\\tea4s15w_0_003421.tif", "C:\\Analysis_from_Movie_for_RiboTrap_Dieter\\Movie_Data_Lorenz\\TPA-3rdplasmidconc1to1\\tea4s15w_0_003422.tif", "C:\\Analysis_from_Movie_for_RiboTrap_Dieter\\Movie_Data_Lorenz\\TPA-3rdplasmidconc1to1\\tea4s15w_0_003423.tif", "C:\\Analysis_from_Movie_for_RiboTrap_Dieter\\Movie_Data_Lorenz\\TPA-3rdplasmidconc1to1\\tea4s15w_0_003424.tif", "C:\\Analysis_from_Movie_for_RiboTrap_Dieter\\Movie_Data_Lorenz\\TPA-3rdplasmidconc1to1\\tea4s15w_0_003425.tif", "C:\\Analysis_from_Movie_for_RiboTrap_Dieter\\Movie_Data_Lorenz\\TPA-3rdplasmidconc1to1\\tea4s15w_0_003426.tif", "C:\\Analysis_from_Movie_for_RiboTrap_Dieter\\Movie_Data_Lorenz\\TPA-3rdplasmidconc1to1\\tea4s15w_0_003427.tif", "C:\\Analysis_from_Movie_for_RiboTrap_Dieter\\Movie_Data_Lorenz\\TPA-3rdplasmidconc1to1\\tea4s15w_0_003428.tif", "C:\\Analysis_from_Movie_for_RiboTrap_Dieter\\Movie_Data_Lorenz\\TPA-3rdplasmidconc1to1\\tea4s15w_0_003429.tif", "C:\\Analysis_from_Movie_for_RiboTrap_Dieter\\Movie_Data_Lorenz\\TPA-3rdplasmidconc1to1\\tea4s15w_0_003430.tif", "C:\\Analysis_from_Movie_for_RiboTrap_Dieter\\Movie_Data_Lorenz\\TPA-3rdplasmidconc1to1\\tea4s15w_0_003431.tif", "C:\\Analysis_from_Movie_for_RiboTrap_Dieter\\Movie_Data_Lorenz\\TPA-3rdplasmidconc1to1\\tea4s15w_0_003432.tif", "C:\\Analysis_from_Movie_for_RiboTrap_Dieter\\Movie_Data_Lorenz\\TPA-3rdplasmidconc1to1\\tea4s15w_0_003433.tif", "C:\\Analysis_from_Movie_for_RiboTrap_Dieter\\Movie_Data_Lorenz\\TPA-3rdplasmidconc1to1\\tea4s15w_0_003434.tif", "C:\\Analysis_from_Movie_for_RiboTrap_Dieter\\Movie_Data_Lorenz\\TPA-3rdplasmidconc1to1\\tea4s15w_0_003435.tif", "C:\\Analysis_from_Movie_for_RiboTrap_Dieter\\Movie_Data_Lorenz\\TPA-3rdplasmidconc1to1\\tea4s15w_0_003436.tif", "C:\\Analysis_from_Movie_for_RiboTrap_Dieter\\Movie_Data_Lorenz\\TPA-3rdplasmidconc1to1\\tea4s15w_0_003437.tif", "C:\\Analysis_from_Movie_for_RiboTrap_Dieter\\Movie_Data_Lorenz\\TPA-3rdplasmidconc1to1\\tea4s15w_0_003438.tif", "C:\\Analysis_from_Movie_for_RiboTrap_Dieter\\Movie_Data_Lorenz\\TPA-3rdplasmidconc1to1\\tea4s15w_0_003439.tif", "C:\\Analysis_from_Movie_for_RiboTrap_Dieter\\Movie_Data_Lorenz\\TPA-3rdplasmidconc1to1\\tea4s15w_0_003440.tif", "C:\\Analysis_from_Movie_for_RiboTrap_Dieter\\Movie_Data_Lorenz\\TPA-3rdplasmidconc1to1\\tea4s15w_0_003441.tif", "C:\\Analysis_from_Movie_for_RiboTrap_Dieter\\Movie_Data_Lorenz\\TPA-3rdplasmidconc1to1\\tea4s15w_0_003442.tif", "C:\\Analysis_from_Movie_for_RiboTrap_Dieter\\Movie_Data_Lorenz\\TPA-3rdplasmidconc1to1\\tea4s15w_0_003443.tif", "C:\\Analysis_from_Movie_for_RiboTrap_Dieter\\Movie_Data_Lorenz\\TPA-3rdplasmidconc1to1\\tea4s15w_0_003444.tif", "C:\\Analysis_from_Movie_for_RiboTrap_Dieter\\Movie_Data_Lorenz\\TPA-3rdplasmidconc1to1\\tea4s15w_0_003445.tif", "C:\\Analysis_from_Movie_for_RiboTrap_Dieter\\Movie_Data_Lorenz\\TPA-3rdplasmidconc1to1\\tea4s15w_0_003446.tif", "C:\\Analysis_from_Movie_for_RiboTrap_Dieter\\Movie_Data_Lorenz\\TPA-3rdplasmidconc1to1\\tea4s15w_0_003447.tif", "C:\\Analysis_from_Movie_for_RiboTrap_Dieter\\Movie_Data_Lorenz\\TPA-3rdplasmidconc1to1\\tea4s15w_0_003448.tif", "C:\\Analysis_from_Movie_for_RiboTrap_Dieter\\Movie_Data_Lorenz\\TPA-3rdplasmidconc1to1\\tea4s15w_0_003449.tif", "C:\\Analysis_from_Movie_for_RiboTrap_Dieter\\Movie_Data_Lorenz\\TPA-3rdplasmidconc1to1\\tea4s15w_0_003450.tif", "C:\\Analysis_from_Movie_for_RiboTrap_Dieter\\Movie_Data_Lorenz\\TPA-3rdplasmidconc1to1\\tea4s15w_0_003451.tif", "C:\\Analysis_from_Movie_for_RiboTrap_Dieter\\Movie_Data_Lorenz\\TPA-3rdplasmidconc1to1\\tea4s15w_0_003452.tif", "C:\\Analysis_from_Movie_for_RiboTrap_Dieter\\Movie_Data_Lorenz\\TPA-3rdplasmidconc1to1\\tea4s15w_0_003453.tif", "C:\\Analysis_from_Movie_for_RiboTrap_Dieter\\Movie_Data_Lorenz\\TPA-3rdplasmidconc1to1\\tea4s15w_0_003454.tif", "C:\\Analysis_from_Movie_for_RiboTrap_Dieter\\Movie_Data_Lorenz\\TPA-3rdplasmidconc1to1\\tea4s15w_0_003455.tif", "C:\\Analysis_from_Movie_for_RiboTrap_Dieter\\Movie_Data_Lorenz\\TPA-3rdplasmidconc1to1\\tea4s15w_0_003456.tif", "C:\\Analysis_from_Movie_for_RiboTrap_Dieter\\Movie_Data_Lorenz\\TPA-3rdplasmidconc1to1\\tea4s15w_0_003457.tif", "C:\\Analysis_from_Movie_for_RiboTrap_Dieter\\Movie_Data_Lorenz\\TPA-3rdplasmidconc1to1\\tea4s15w_0_003458.tif", "C:\\Analysis_from_Movie_for_RiboTrap_Dieter\\Movie_Data_Lorenz\\TPA-3rdplasmidconc1to1\\tea4s15w_0_003459.tif", "C:\\Analysis_from_Movie_for_RiboTrap_Dieter\\Movie_Data_Lorenz\\TPA-3rdplasmidconc1to1\\tea4s15w_0_003460.tif", "C:\\Analysis_from_Movie_for_RiboTrap_Dieter\\Movie_Data_Lorenz\\TPA-3rdplasmidconc1to1\\tea4s15w_0_003461.tif", "C:\\Analysis_from_Movie_for_RiboTrap_Dieter\\Movie_Data_Lorenz\\TPA-3rdplasmidconc1to1\\tea4s15w_0_003462.tif", "C:\\Analysis_from_Movie_for_RiboTrap_Dieter\\Movie_Data_Lorenz\\TPA-3rdplasmidconc1to1\\tea4s15w_0_003463.tif", "C:\\Analysis_from_Movie_for_RiboTrap_Dieter\\Movie_Data_Lorenz\\TPA-3rdplasmidconc1to1\\tea4s15w_0_003464.tif", "C:\\Analysis_from_Movie_for_RiboTrap_Dieter\\Movie_Data_Lorenz\\TPA-3rdplasmidconc1to1\\tea4s15w_0_003465.tif", "C:\\Analysis_from_Movie_for_RiboTrap_Dieter\\Movie_Data_Lorenz\\TPA-3rdplasmidconc1to1\\tea4s15w_0_003466.tif", "C:\\Analysis_from_Movie_for_RiboTrap_Dieter\\Movie_Data_Lorenz\\TPA-3rdplasmidconc1to1\\tea4s15w_0_003467.tif", "C:\\Analysis_from_Movie_for_RiboTrap_Dieter\\Movie_Data_Lorenz\\TPA-3rdplasmidconc1to1\\tea4s15w_0_003468.tif", "C:\\Analysis_from_Movie_for_RiboTrap_Dieter\\Movie_Data_Lorenz\\TPA-3rdplasmidconc1to1\\tea4s15w_0_003469.tif", "C:\\Analysis_from_Movie_for_RiboTrap_Dieter\\Movie_Data_Lorenz\\TPA-3rdplasmidconc1to1\\tea4s15w_0_003470.tif", "C:\\Analysis_from_Movie_for_RiboTrap_Dieter\\Movie_Data_Lorenz\\TPA-3rdplasmidconc1to1\\tea4s15w_0_003471.tif", "C:\\Analysis_from_Movie_for_RiboTrap_Dieter\\Movie_Data_Lorenz\\TPA-3rdplasmidconc1to1\\tea4s15w_0_003472.tif", "C:\\Analysis_from_Movie_for_RiboTrap_Dieter\\Movie_Data_Lorenz\\TPA-3rdplasmidconc1to1\\tea4s15w_0_003473.tif", "C:\\Analysis_from_Movie_for_RiboTrap_Dieter\\Movie_Data_Lorenz\\TPA-3rdplasmidconc1to1\\tea4s15w_0_003474.tif", "C:\\Analysis_from_Movie_for_RiboTrap_Dieter\\Movie_Data_Lorenz\\TPA-3rdplasmidconc1to1\\tea4s15w_0_003475.tif", "C:\\Analysis_from_Movie_for_RiboTrap_Dieter\\Movie_Data_Lorenz\\TPA-3rdplasmidconc1to1\\tea4s15w_0_003476.tif", "C:\\Analysis_from_Movie_for_RiboTrap_Dieter\\Movie_Data_Lorenz\\TPA-3rdplasmidconc1to1\\tea4s15w_0_003477.tif", "C:\\Analysis_from_Movie_for_RiboTrap_Dieter\\Movie_Data_Lorenz\\TPA-3rdplasmidconc1to1\\tea4s15w_0_003478.tif", "C:\\Analysis_from_Movie_for_RiboTrap_Dieter\\Movie_Data_Lorenz\\TPA-3rdplasmidconc1to1\\tea4s15w_0_003479.tif", "C:\\Analysis_from_Movie_for_RiboTrap_Dieter\\Movie_Data_Lorenz\\TPA-3rdplasmidconc1to1\\tea4s15w_0_003480.tif", "C:\\Analysis_from_Movie_for_RiboTrap_Dieter\\Movie_Data_Lorenz\\TPA-3rdplasmidconc1to1\\tea4s15w_0_003481.tif", "C:\\Analysis_from_Movie_for_RiboTrap_Dieter\\Movie_Data_Lorenz\\TPA-3rdplasmidconc1to1\\tea4s15w_0_003482.tif", "C:\\Analysis_from_Movie_for_RiboTrap_Dieter\\Movie_Data_Lorenz\\TPA-3rdplasmidconc1to1\\tea4s15w_0_003483.tif", "C:\\Analysis_from_Movie_for_RiboTrap_Dieter\\Movie_Data_Lorenz\\TPA-3rdplasmidconc1to1\\tea4s15w_0_003484.tif", "C:\\Analysis_from_Movie_for_RiboTrap_Dieter\\Movie_Data_Lorenz\\TPA-3rdplasmidconc1to1\\tea4s15w_0_003485.tif", "C:\\Analysis_from_Movie_for_RiboTrap_Dieter\\Movie_Data_Lorenz\\TPA-3rdplasmidconc1to1\\tea4s15w_0_003486.tif", "C:\\Analysis_from_Movie_for_RiboTrap_Dieter\\Movie_Data_Lorenz\\TPA-3rdplasmidconc1to1\\tea4s15w_0_003487.tif", "C:\\Analysis_from_Movie_for_RiboTrap_Dieter\\Movie_Data_Lorenz\\TPA-3rdplasmidconc1to1\\tea4s15w_0_003488.tif", "C:\\Analysis_from_Movie_for_RiboTrap_Dieter\\Movie_Data_Lorenz\\TPA-3rdplasmidconc1to1\\tea4s15w_0_003489.tif", "C:\\Analysis_from_Movie_for_RiboTrap_Dieter\\Movie_Data_Lorenz\\TPA-3rdplasmidconc1to1\\tea4s15w_0_003490.tif", "C:\\Analysis_from_Movie_for_RiboTrap_Dieter\\Movie_Data_Lorenz\\TPA-3rdplasmidconc1to1\\tea4s15w_0_003491.tif", "C:\\Analysis_from_Movie_for_RiboTrap_Dieter\\Movie_Data_Lorenz\\TPA-3rdplasmidconc1to1\\tea4s15w_0_003492.tif", "C:\\Analysis_from_Movie_for_RiboTrap_Dieter\\Movie_Data_Lorenz\\TPA-3rdplasmidconc1to1\\tea4s15w_0_003493.tif", "C:\\Analysis_from_Movie_for_RiboTrap_Dieter\\Movie_Data_Lorenz\\TPA-3rdplasmidconc1to1\\tea4s15w_0_003494.tif", "C:\\Analysis_from_Movie_for_RiboTrap_Dieter\\Movie_Data_Lorenz\\TPA-3rdplasmidconc1to1\\tea4s15w_0_003495.tif", "C:\\Analysis_from_Movie_for_RiboTrap_Dieter\\Movie_Data_Lorenz\\TPA-3rdplasmidconc1to1\\tea4s15w_0_003496.tif", "C:\\Analysis_from_Movie_for_RiboTrap_Dieter\\Movie_Data_Lorenz\\TPA-3rdplasmidconc1to1\\tea4s15w_0_003497.tif", "C:\\Analysis_from_Movie_for_RiboTrap_Dieter\\Movie_Data_Lorenz\\TPA-3rdplasmidconc1to1\\tea4s15w_0_003498.tif", "C:\\Analysis_from_Movie_for_RiboTrap_Dieter\\Movie_Data_Lorenz\\TPA-3rdplasmidconc1to1\\tea4s15w_0_003499.tif", "C:\\Analysis_from_Movie_for_RiboTrap_Dieter\\Movie_Data_Lorenz\\TPA-3rdplasmidconc1to1\\tea4s15w_0_003500.tif", "C:\\Analysis_from_Movie_for_RiboTrap_Dieter\\Movie_Data_Lorenz\\TPA-3rdplasmidconc1to1\\tea4s15w_0_003501.tif", "C:\\Analysis_from_Movie_for_RiboTrap_Dieter\\Movie_Data_Lorenz\\TPA-3rdplasmidconc1to1\\tea4s15w_0_003502.tif", "C:\\Analysis_from_Movie_for_RiboTrap_Dieter\\Movie_Data_Lorenz\\TPA-3rdplasmidconc1to1\\tea4s15w_0_003503.tif", "C:\\Analysis_from_Movie_for_RiboTrap_Dieter\\Movie_Data_Lorenz\\TPA-3rdplasmidconc1to1\\tea4s15w_0_003504.tif", "C:\\Analysis_from_Movie_for_RiboTrap_Dieter\\Movie_Data_Lorenz\\TPA-3rdplasmidconc1to1\\tea4s15w_0_003505.tif", "C:\\Analysis_from_Movie_for_RiboTrap_Dieter\\Movie_Data_Lorenz\\TPA-3rdplasmidconc1to1\\tea4s15w_0_003506.tif", "C:\\Analysis_from_Movie_for_RiboTrap_Dieter\\Movie_Data_Lorenz\\TPA-3rdplasmidconc1to1\\tea4s15w_0_003507.tif", "C:\\Analysis_from_Movie_for_RiboTrap_Dieter\\Movie_Data_Lorenz\\TPA-3rdplasmidconc1to1\\tea4s15w_0_003508.tif", "C:\\Analysis_from_Movie_for_RiboTrap_Dieter\\Movie_Data_Lorenz\\TPA-3rdplasmidconc1to1\\tea4s15w_0_003509.tif", "C:\\Analysis_from_Movie_for_RiboTrap_Dieter\\Movie_Data_Lorenz\\TPA-3rdplasmidconc1to1\\tea4s15w_0_003510.tif", "C:\\Analysis_from_Movie_for_RiboTrap_Dieter\\Movie_Data_Lorenz\\TPA-3rdplasmidconc1to1\\tea4s15w_0_003511.tif", "C:\\Analysis_from_Movie_for_RiboTrap_Dieter\\Movie_Data_Lorenz\\TPA-3rdplasmidconc1to1\\tea4s15w_0_003512.tif", "C:\\Analysis_from_Movie_for_RiboTrap_Dieter\\Movie_Data_Lorenz\\TPA-3rdplasmidconc1to1\\tea4s15w_0_003513.tif", "C:\\Analysis_from_Movie_for_RiboTrap_Dieter\\Movie_Data_Lorenz\\TPA-3rdplasmidconc1to1\\tea4s15w_0_003514.tif", "C:\\Analysis_from_Movie_for_RiboTrap_Dieter\\Movie_Data_Lorenz\\TPA-3rdplasmidconc1to1\\tea4s15w_0_003515.tif", "C:\\Analysis_from_Movie_for_RiboTrap_Dieter\\Movie_Data_Lorenz\\TPA-3rdplasmidconc1to1\\tea4s15w_0_003516.tif", "C:\\Analysis_from_Movie_for_RiboTrap_Dieter\\Movie_Data_Lorenz\\TPA-3rdplasmidconc1to1\\tea4s15w_0_003517.tif", "C:\\Analysis_from_Movie_for_RiboTrap_Dieter\\Movie_Data_Lorenz\\TPA-3rdplasmidconc1to1\\tea4s15w_0_003518.tif", "C:\\Analysis_from_Movie_for_RiboTrap_Dieter\\Movie_Data_Lorenz\\TPA-3rdplasmidconc1to1\\tea4s15w_0_003519.tif", "C:\\Analysis_from_Movie_for_RiboTrap_Dieter\\Movie_Data_Lorenz\\TPA-3rdplasmidconc1to1\\tea4s15w_0_003520.tif", "C:\\Analysis_from_Movie_for_RiboTrap_Dieter\\Movie_Data_Lorenz\\TPA-3rdplasmidconc1to1\\tea4s15w_0_003521.tif", "C:\\Analysis_from_Movie_for_RiboTrap_Dieter\\Movie_Data_Lorenz\\TPA-3rdplasmidconc1to1\\tea4s15w_0_003522.tif", "C:\\Analysis_from_Movie_for_RiboTrap_Dieter\\Movie_Data_Lorenz\\TPA-3rdplasmidconc1to1\\tea4s15w_0_003523.tif", "C:\\Analysis_from_Movie_for_RiboTrap_Dieter\\Movie_Data_Lorenz\\TPA-3rdplasmidconc1to1\\tea4s15w_0_003524.tif", "C:\\Analysis_from_Movie_for_RiboTrap_Dieter\\Movie_Data_Lorenz\\TPA-3rdplasmidconc1to1\\tea4s15w_0_003525.tif", "C:\\Analysis_from_Movie_for_RiboTrap_Dieter\\Movie_Data_Lorenz\\TPA-3rdplasmidconc1to1\\tea4s15w_0_003526.tif", "C:\\Analysis_from_Movie_for_RiboTrap_Dieter\\Movie_Data_Lorenz\\TPA-3rdplasmidconc1to1\\tea4s15w_0_003527.tif", "C:\\Analysis_from_Movie_for_RiboTrap_Dieter\\Movie_Data_Lorenz\\TPA-3rdplasmidconc1to1\\tea4s15w_0_003528.tif", "C:\\Analysis_from_Movie_for_RiboTrap_Dieter\\Movie_Data_Lorenz\\TPA-3rdplasmidconc1to1\\tea4s15w_0_003529.tif", "C:\\Analysis_from_Movie_for_RiboTrap_Dieter\\Movie_Data_Lorenz\\TPA-3rdplasmidconc1to1\\tea4s15w_0_003530.tif", "C:\\Analysis_from_Movie_for_RiboTrap_Dieter\\Movie_Data_Lorenz\\TPA-3rdplasmidconc1to1\\tea4s15w_0_003531.tif", "C:\\Analysis_from_Movie_for_RiboTrap_Dieter\\Movie_Data_Lorenz\\TPA-3rdplasmidconc1to1\\tea4s15w_0_003532.tif", "C:\\Analysis_from_Movie_for_RiboTrap_Dieter\\Movie_Data_Lorenz\\TPA-3rdplasmidconc1to1\\tea4s15w_0_003533.tif", "C:\\Analysis_from_Movie_for_RiboTrap_Dieter\\Movie_Data_Lorenz\\TPA-3rdplasmidconc1to1\\tea4s15w_0_003534.tif", "C:\\Analysis_from_Movie_for_RiboTrap_Dieter\\Movie_Data_Lorenz\\TPA-3rdplasmidconc1to1\\tea4s15w_0_003535.tif", "C:\\Analysis_from_Movie_for_RiboTrap_Dieter\\Movie_Data_Lorenz\\TPA-3rdplasmidconc1to1\\tea4s15w_0_003536.tif", "C:\\Analysis_from_Movie_for_RiboTrap_Dieter\\Movie_Data_Lorenz\\TPA-3rdplasmidconc1to1\\tea4s15w_0_003537.tif", "C:\\Analysis_from_Movie_for_RiboTrap_Dieter\\Movie_Data_Lorenz\\TPA-3rdplasmidconc1to1\\tea4s15w_0_003538.tif", "C:\\Analysis_from_Movie_for_RiboTrap_Dieter\\Movie_Data_Lorenz\\TPA-3rdplasmidconc1to1\\tea4s15w_0_003539.tif", "C:\\Analysis_from_Movie_for_RiboTrap_Dieter\\Movie_Data_Lorenz\\TPA-3rdplasmidconc1to1\\tea4s15w_0_003540.tif", "C:\\Analysis_from_Movie_for_RiboTrap_Dieter\\Movie_Data_Lorenz\\TPA-3rdplasmidconc1to1\\tea4s15w_0_003541.tif", "C:\\Analysis_from_Movie_for_RiboTrap_Dieter\\Movie_Data_Lorenz\\TPA-3rdplasmidconc1to1\\tea4s15w_0_003542.tif", "C:\\Analysis_from_Movie_for_RiboTrap_Dieter\\Movie_Data_Lorenz\\TPA-3rdplasmidconc1to1\\tea4s15w_0_003543.tif", "C:\\Analysis_from_Movie_for_RiboTrap_Dieter\\Movie_Data_Lorenz\\TPA-3rdplasmidconc1to1\\tea4s15w_0_003544.tif", "C:\\Analysis_from_Movie_for_RiboTrap_Dieter\\Movie_Data_Lorenz\\TPA-3rdplasmidconc1to1\\tea4s15w_0_003545.tif", "C:\\Analysis_from_Movie_for_RiboTrap_Dieter\\Movie_Data_Lorenz\\TPA-3rdplasmidconc1to1\\tea4s15w_0_003546.tif", "C:\\Analysis_from_Movie_for_RiboTrap_Dieter\\Movie_Data_Lorenz\\TPA-3rdplasmidconc1to1\\tea4s15w_0_003547.tif", "C:\\Analysis_from_Movie_for_RiboTrap_Dieter\\Movie_Data_Lorenz\\TPA-3rdplasmidconc1to1\\tea4s15w_0_003548.tif", "C:\\Analysis_from_Movie_for_RiboTrap_Dieter\\Movie_Data_Lorenz\\TPA-3rdplasmidconc1to1\\tea4s15w_0_003549.tif", "C:\\Analysis_from_Movie_for_RiboTrap_Dieter\\Movie_Data_Lorenz\\TPA-3rdplasmidconc1to1\\tea4s15w_0_003550.tif", "C:\\Analysis_from_Movie_for_RiboTrap_Dieter\\Movie_Data_Lorenz\\TPA-3rdplasmidconc1to1\\tea4s15w_0_003551.tif", "C:\\Analysis_from_Movie_for_RiboTrap_Dieter\\Movie_Data_Lorenz\\TPA-3rdplasmidconc1to1\\tea4s15w_0_003552.tif", "C:\\Analysis_from_Movie_for_RiboTrap_Dieter\\Movie_Data_Lorenz\\TPA-3rdplasmidconc1to1\\tea4s15w_0_003553.tif", "C:\\Analysis_from_Movie_for_RiboTrap_Dieter\\Movie_Data_Lorenz\\TPA-3rdplasmidconc1to1\\tea4s15w_0_003554.tif", "C:\\Analysis_from_Movie_for_RiboTrap_Dieter\\Movie_Data_Lorenz\\TPA-3rdplasmidconc1to1\\tea4s15w_0_003555.tif", "C:\\Analysis_from_Movie_for_RiboTrap_Dieter\\Movie_Data_Lorenz\\TPA-3rdplasmidconc1to1\\tea4s15w_0_003556.tif", "C:\\Analysis_from_Movie_for_RiboTrap_Dieter\\Movie_Data_Lorenz\\TPA-3rdplasmidconc1to1\\tea4s15w_0_003557.tif", "C:\\Analysis_from_Movie_for_RiboTrap_Dieter\\Movie_Data_Lorenz\\TPA-3rdplasmidconc1to1\\tea4s15w_0_003558.tif", "C:\\Analysis_from_Movie_for_RiboTrap_Dieter\\Movie_Data_Lorenz\\TPA-3rdplasmidconc1to1\\tea4s15w_0_003559.tif", "C:\\Analysis_from_Movie_for_RiboTrap_Dieter\\Movie_Data_Lorenz\\TPA-3rdplasmidconc1to1\\tea4s15w_0_003560.tif", "C:\\Analysis_from_Movie_for_RiboTrap_Dieter\\Movie_Data_Lorenz\\TPA-3rdplasmidconc1to1\\tea4s15w_0_003561.tif", "C:\\Analysis_from_Movie_for_RiboTrap_Dieter\\Movie_Data_Lorenz\\TPA-3rdplasmidconc1to1\\tea4s15w_0_003562.tif", "C:\\Analysis_from_Movie_for_RiboTrap_Dieter\\Movie_Data_Lorenz\\TPA-3rdplasmidconc1to1\\tea4s15w_0_003563.tif", "C:\\Analysis_from_Movie_for_RiboTrap_Dieter\\Movie_Data_Lorenz\\TPA-3rdplasmidconc1to1\\tea4s15w_0_003564.tif", "C:\\Analysis_from_Movie_for_RiboTrap_Dieter\\Movie_Data_Lorenz\\TPA-3rdplasmidconc1to1\\tea4s15w_0_003565.tif"], 1 "Paths":path[](array[path])=[path "C:/Analysis_from_Movie_for_RiboTrap_Dieter/Movie_Data_Lorenz/TPA-3rdplasmidconc1to1/tea4s15w_0_002099.tif", path "C:/Analysis_from_Movie_for_RiboTrap_Dieter/Movie_Data_Lorenz/TPA-3rdplasmidconc1to1/tea4s15w_0_002100.tif", path "C:/Analysis_from_Movie_for_RiboTrap_Dieter/Movie_Data_Lorenz/TPA-3rdplasmidconc1to1/tea4s15w_0_002101.tif", path "C:/Analysis_from_Movie_for_RiboTrap_Dieter/Movie_Data_Lorenz/TPA-3rdplasmidconc1to1/tea4s15w_0_002102.tif", path "C:/Analysis_from_Movie_for_RiboTrap_Dieter/Movie_Data_Lorenz/TPA-3rdplasmidconc1to1/tea4s15w_0_002103.tif", path "C:/Analysis_from_Movie_for_RiboTrap_Dieter/Movie_Data_Lorenz/TPA-3rdplasmidconc1to1/tea4s15w_0_002104.tif", path "C:/Analysis_from_Movie_for_RiboTrap_Dieter/Movie_Data_Lorenz/TPA-3rdplasmidconc1to1/tea4s15w_0_002105.tif", path "C:/Analysis_from_Movie_for_RiboTrap_Dieter/Movie_Data_Lorenz/TPA-3rdplasmidconc1to1/tea4s15w_0_002106.tif", path "C:/Analysis_from_Movie_for_RiboTrap_Dieter/Movie_Data_Lorenz/TPA-3rdplasmidconc1to1/tea4s15w_0_002107.tif", path "C:/Analysis_from_Movie_for_RiboTrap_Dieter/Movie_Data_Lorenz/TPA-3rdplasmidconc1to1/tea4s15w_0_002108.tif", path "C:/Analysis_from_Movie_for_RiboTrap_Dieter/Movie_Data_Lorenz/TPA-3rdplasmidconc1to1/tea4s15w_0_002109.tif", path "C:/Analysis_from_Movie_for_RiboTrap_Dieter/Movie_Data_Lorenz/TPA-3rdplasmidconc1to1/tea4s15w_0_002110.tif", path "C:/Analysis_from_Movie_for_RiboTrap_Dieter/Movie_Data_Lorenz/TPA-3rdplasmidconc1to1/tea4s15w_0_002111.tif", path "C:/Analysis_from_Movie_for_RiboTrap_Dieter/Movie_Data_Lorenz/TPA-3rdplasmidconc1to1/tea4s15w_0_002112.tif", path "C:/Analysis_from_Movie_for_RiboTrap_Dieter/Movie_Data_Lorenz/TPA-3rdplasmidconc1to1/tea4s15w_0_002113.tif", path "C:/Analysis_from_Movie_for_RiboTrap_Dieter/Movie_Data_Lorenz/TPA-3rdplasmidconc1to1/tea4s15w_0_002114.tif", path "C:/Analysis_from_Movie_for_RiboTrap_Dieter/Movie_Data_Lorenz/TPA-3rdplasmidconc1to1/tea4s15w_0_002115.tif", path "C:/Analysis_from_Movie_for_RiboTrap_Dieter/Movie_Data_Lorenz/TPA-3rdplasmidconc1to1/tea4s15w_0_002116.tif", path "C:/Analysis_from_Movie_for_RiboTrap_Dieter/Movie_Data_Lorenz/TPA-3rdplasmidconc1to1/tea4s15w_0_002117.tif", path "C:/Analysis_from_Movie_for_RiboTrap_Dieter/Movie_Data_Lorenz/TPA-3rdplasmidconc1to1/tea4s15w_0_002118.tif", path "C:/Analysis_from_Movie_for_RiboTrap_Dieter/Movie_Data_Lorenz/TPA-3rdplasmidconc1to1/tea4s15w_0_002119.tif", path "C:/Analysis_from_Movie_for_RiboTrap_Dieter/Movie_Data_Lorenz/TPA-3rdplasmidconc1to1/tea4s15w_0_002120.tif", path "C:/Analysis_from_Movie_for_RiboTrap_Dieter/Movie_Data_Lorenz/TPA-3rdplasmidconc1to1/tea4s15w_0_002121.tif", path "C:/Analysis_from_Movie_for_RiboTrap_Dieter/Movie_Data_Lorenz/TPA-3rdplasmidconc1to1/tea4s15w_0_002122.tif", path "C:/Analysis_from_Movie_for_RiboTrap_Dieter/Movie_Data_Lorenz/TPA-3rdplasmidconc1to1/tea4s15w_0_002123.tif", path "C:/Analysis_from_Movie_for_RiboTrap_Dieter/Movie_Data_Lorenz/TPA-3rdplasmidconc1to1/tea4s15w_0_002124.tif", path "C:/Analysis_from_Movie_for_RiboTrap_Dieter/Movie_Data_Lorenz/TPA-3rdplasmidconc1to1/tea4s15w_0_002125.tif", path "C:/Analysis_from_Movie_for_RiboTrap_Dieter/Movie_Data_Lorenz/TPA-3rdplasmidconc1to1/tea4s15w_0_002126.tif", path "C:/Analysis_from_Movie_for_RiboTrap_Dieter/Movie_Data_Lorenz/TPA-3rdplasmidconc1to1/tea4s15w_0_002127.tif", path "C:/Analysis_from_Movie_for_RiboTrap_Dieter/Movie_Data_Lorenz/TPA-3rdplasmidconc1to1/tea4s15w_0_002128.tif", path "C:/Analysis_from_Movie_for_RiboTrap_Dieter/Movie_Data_Lorenz/TPA-3rdplasmidconc1to1/tea4s15w_0_002129.tif", path "C:/Analysis_from_Movie_for_RiboTrap_Dieter/Movie_Data_Lorenz/TPA-3rdplasmidconc1to1/tea4s15w_0_002130.tif", path "C:/Analysis_from_Movie_for_RiboTrap_Dieter/Movie_Data_Lorenz/TPA-3rdplasmidconc1to1/tea4s15w_0_002131.tif", path "C:/Analysis_from_Movie_for_RiboTrap_Dieter/Movie_Data_Lorenz/TPA-3rdplasmidconc1to1/tea4s15w_0_002132.tif", path "C:/Analysis_from_Movie_for_RiboTrap_Dieter/Movie_Data_Lorenz/TPA-3rdplasmidconc1to1/tea4s15w_0_002133.tif", path "C:/Analysis_from_Movie_for_RiboTrap_Dieter/Movie_Data_Lorenz/TPA-3rdplasmidconc1to1/tea4s15w_0_002134.tif", path "C:/Analysis_from_Movie_for_RiboTrap_Dieter/Movie_Data_Lorenz/TPA-3rdplasmidconc1to1/tea4s15w_0_002135.tif", path "C:/Analysis_from_Movie_for_RiboTrap_Dieter/Movie_Data_Lorenz/TPA-3rdplasmidconc1to1/tea4s15w_0_002136.tif", path "C:/Analysis_from_Movie_for_RiboTrap_Dieter/Movie_Data_Lorenz/TPA-3rdplasmidconc1to1/tea4s15w_0_002137.tif", path "C:/Analysis_from_Movie_for_RiboTrap_Dieter/Movie_Data_Lorenz/TPA-3rdplasmidconc1to1/tea4s15w_0_002138.tif", path "C:/Analysis_from_Movie_for_RiboTrap_Dieter/Movie_Data_Lorenz/TPA-3rdplasmidconc1to1/tea4s15w_0_002139.tif", path "C:/Analysis_from_Movie_for_RiboTrap_Dieter/Movie_Data_Lorenz/TPA-3rdplasmidconc1to1/tea4s15w_0_002140.tif", path "C:/Analysis_from_Movie_for_RiboTrap_Dieter/Movie_Data_Lorenz/TPA-3rdplasmidconc1to1/tea4s15w_0_002141.tif", path "C:/Analysis_from_Movie_for_RiboTrap_Dieter/Movie_Data_Lorenz/TPA-3rdplasmidconc1to1/tea4s15w_0_002142.tif", path "C:/Analysis_from_Movie_for_RiboTrap_Dieter/Movie_Data_Lorenz/TPA-3rdplasmidconc1to1/tea4s15w_0_002143.tif", path "C:/Analysis_from_Movie_for_RiboTrap_Dieter/Movie_Data_Lorenz/TPA-3rdplasmidconc1to1/tea4s15w_0_002144.tif", path "C:/Analysis_from_Movie_for_RiboTrap_Dieter/Movie_Data_Lorenz/TPA-3rdplasmidconc1to1/tea4s15w_0_002145.tif", path "C:/Analysis_from_Movie_for_RiboTrap_Dieter/Movie_Data_Lorenz/TPA-3rdplasmidconc1to1/tea4s15w_0_002146.tif", path "C:/Analysis_from_Movie_for_RiboTrap_Dieter/Movie_Data_Lorenz/TPA-3rdplasmidconc1to1/tea4s15w_0_002147.tif", path "C:/Analysis_from_Movie_for_RiboTrap_Dieter/Movie_Data_Lorenz/TPA-3rdplasmidconc1to1/tea4s15w_0_002148.tif", path "C:/Analysis_from_Movie_for_RiboTrap_Dieter/Movie_Data_Lorenz/TPA-3rdplasmidconc1to1/tea4s15w_0_002149.tif", path "C:/Analysis_from_Movie_for_RiboTrap_Dieter/Movie_Data_Lorenz/TPA-3rdplasmidconc1to1/tea4s15w_0_002150.tif", path "C:/Analysis_from_Movie_for_RiboTrap_Dieter/Movie_Data_Lorenz/TPA-3rdplasmidconc1to1/tea4s15w_0_002151.tif", path "C:/Analysis_from_Movie_for_RiboTrap_Dieter/Movie_Data_Lorenz/TPA-3rdplasmidconc1to1/tea4s15w_0_002152.tif", path "C:/Analysis_from_Movie_for_RiboTrap_Dieter/Movie_Data_Lorenz/TPA-3rdplasmidconc1to1/tea4s15w_0_002153.tif", path "C:/Analysis_from_Movie_for_RiboTrap_Dieter/Movie_Data_Lorenz/TPA-3rdplasmidconc1to1/tea4s15w_0_002154.tif", path "C:/Analysis_from_Movie_for_RiboTrap_Dieter/Movie_Data_Lorenz/TPA-3rdplasmidconc1to1/tea4s15w_0_002155.tif", path "C:/Analysis_from_Movie_for_RiboTrap_Dieter/Movie_Data_Lorenz/TPA-3rdplasmidconc1to1/tea4s15w_0_002156.tif", path "C:/Analysis_from_Movie_for_RiboTrap_Dieter/Movie_Data_Lorenz/TPA-3rdplasmidconc1to1/tea4s15w_0_002157.tif", path "C:/Analysis_from_Movie_for_RiboTrap_Dieter/Movie_Data_Lorenz/TPA-3rdplasmidconc1to1/tea4s15w_0_002158.tif", path "C:/Analysis_from_Movie_for_RiboTrap_Dieter/Movie_Data_Lorenz/TPA-3rdplasmidconc1to1/tea4s15w_0_002159.tif", path "C:/Analysis_from_Movie_for_RiboTrap_Dieter/Movie_Data_Lorenz/TPA-3rdplasmidconc1to1/tea4s15w_0_002160.tif", path "C:/Analysis_from_Movie_for_RiboTrap_Dieter/Movie_Data_Lorenz/TPA-3rdplasmidconc1to1/tea4s15w_0_002161.tif", path "C:/Analysis_from_Movie_for_RiboTrap_Dieter/Movie_Data_Lorenz/TPA-3rdplasmidconc1to1/tea4s15w_0_002162.tif", path "C:/Analysis_from_Movie_for_RiboTrap_Dieter/Movie_Data_Lorenz/TPA-3rdplasmidconc1to1/tea4s15w_0_002163.tif", path "C:/Analysis_from_Movie_for_RiboTrap_Dieter/Movie_Data_Lorenz/TPA-3rdplasmidconc1to1/tea4s15w_0_002164.tif", path "C:/Analysis_from_Movie_for_RiboTrap_Dieter/Movie_Data_Lorenz/TPA-3rdplasmidconc1to1/tea4s15w_0_002165.tif", path "C:/Analysis_from_Movie_for_RiboTrap_Dieter/Movie_Data_Lorenz/TPA-3rdplasmidconc1to1/tea4s15w_0_002166.tif", path "C:/Analysis_from_Movie_for_RiboTrap_Dieter/Movie_Data_Lorenz/TPA-3rdplasmidconc1to1/tea4s15w_0_002167.tif", path "C:/Analysis_from_Movie_for_RiboTrap_Dieter/Movie_Data_Lorenz/TPA-3rdplasmidconc1to1/tea4s15w_0_002168.tif", path "C:/Analysis_from_Movie_for_RiboTrap_Dieter/Movie_Data_Lorenz/TPA-3rdplasmidconc1to1/tea4s15w_0_002169.tif", path "C:/Analysis_from_Movie_for_RiboTrap_Dieter/Movie_Data_Lorenz/TPA-3rdplasmidconc1to1/tea4s15w_0_002170.tif", path "C:/Analysis_from_Movie_for_RiboTrap_Dieter/Movie_Data_Lorenz/TPA-3rdplasmidconc1to1/tea4s15w_0_002171.tif", path "C:/Analysis_from_Movie_for_RiboTrap_Dieter/Movie_Data_Lorenz/TPA-3rdplasmidconc1to1/tea4s15w_0_002172.tif", path "C:/Analysis_from_Movie_for_RiboTrap_Dieter/Movie_Data_Lorenz/TPA-3rdplasmidconc1to1/tea4s15w_0_002173.tif", path "C:/Analysis_from_Movie_for_RiboTrap_Dieter/Movie_Data_Lorenz/TPA-3rdplasmidconc1to1/tea4s15w_0_002174.tif", path "C:/Analysis_from_Movie_for_RiboTrap_Dieter/Movie_Data_Lorenz/TPA-3rdplasmidconc1to1/tea4s15w_0_002175.tif", path "C:/Analysis_from_Movie_for_RiboTrap_Dieter/Movie_Data_Lorenz/TPA-3rdplasmidconc1to1/tea4s15w_0_002176.tif", path "C:/Analysis_from_Movie_for_RiboTrap_Dieter/Movie_Data_Lorenz/TPA-3rdplasmidconc1to1/tea4s15w_0_002177.tif", path "C:/Analysis_from_Movie_for_RiboTrap_Dieter/Movie_Data_Lorenz/TPA-3rdplasmidconc1to1/tea4s15w_0_002178.tif", path "C:/Analysis_from_Movie_for_RiboTrap_Dieter/Movie_Data_Lorenz/TPA-3rdplasmidconc1to1/tea4s15w_0_002179.tif", path "C:/Analysis_from_Movie_for_RiboTrap_Dieter/Movie_Data_Lorenz/TPA-3rdplasmidconc1to1/tea4s15w_0_002180.tif", path "C:/Analysis_from_Movie_for_RiboTrap_Dieter/Movie_Data_Lorenz/TPA-3rdplasmidconc1to1/tea4s15w_0_002181.tif", path "C:/Analysis_from_Movie_for_RiboTrap_Dieter/Movie_Data_Lorenz/TPA-3rdplasmidconc1to1/tea4s15w_0_002182.tif", path "C:/Analysis_from_Movie_for_RiboTrap_Dieter/Movie_Data_Lorenz/TPA-3rdplasmidconc1to1/tea4s15w_0_002183.tif", path "C:/Analysis_from_Movie_for_RiboTrap_Dieter/Movie_Data_Lorenz/TPA-3rdplasmidconc1to1/tea4s15w_0_002184.tif", path "C:/Analysis_from_Movie_for_RiboTrap_Dieter/Movie_Data_Lorenz/TPA-3rdplasmidconc1to1/tea4s15w_0_002185.tif", path "C:/Analysis_from_Movie_for_RiboTrap_Dieter/Movie_Data_Lorenz/TPA-3rdplasmidconc1to1/tea4s15w_0_002186.tif", path "C:/Analysis_from_Movie_for_RiboTrap_Dieter/Movie_Data_Lorenz/TPA-3rdplasmidconc1to1/tea4s15w_0_002187.tif", path "C:/Analysis_from_Movie_for_RiboTrap_Dieter/Movie_Data_Lorenz/TPA-3rdplasmidconc1to1/tea4s15w_0_002188.tif", path "C:/Analysis_from_Movie_for_RiboTrap_Dieter/Movie_Data_Lorenz/TPA-3rdplasmidconc1to1/tea4s15w_0_002189.tif", path "C:/Analysis_from_Movie_for_RiboTrap_Dieter/Movie_Data_Lorenz/TPA-3rdplasmidconc1to1/tea4s15w_0_002190.tif", path "C:/Analysis_from_Movie_for_RiboTrap_Dieter/Movie_Data_Lorenz/TPA-3rdplasmidconc1to1/tea4s15w_0_002191.tif", path "C:/Analysis_from_Movie_for_RiboTrap_Dieter/Movie_Data_Lorenz/TPA-3rdplasmidconc1to1/tea4s15w_0_002192.tif", path "C:/Analysis_from_Movie_for_RiboTrap_Dieter/Movie_Data_Lorenz/TPA-3rdplasmidconc1to1/tea4s15w_0_002193.tif", path "C:/Analysis_from_Movie_for_RiboTrap_Dieter/Movie_Data_Lorenz/TPA-3rdplasmidconc1to1/tea4s15w_0_002194.tif", path "C:/Analysis_from_Movie_for_RiboTrap_Dieter/Movie_Data_Lorenz/TPA-3rdplasmidconc1to1/tea4s15w_0_002195.tif", path "C:/Analysis_from_Movie_for_RiboTrap_Dieter/Movie_Data_Lorenz/TPA-3rdplasmidconc1to1/tea4s15w_0_002196.tif", path "C:/Analysis_from_Movie_for_RiboTrap_Dieter/Movie_Data_Lorenz/TPA-3rdplasmidconc1to1/tea4s15w_0_002197.tif", path "C:/Analysis_from_Movie_for_RiboTrap_Dieter/Movie_Data_Lorenz/TPA-3rdplasmidconc1to1/tea4s15w_0_002198.tif", path "C:/Analysis_from_Movie_for_RiboTrap_Dieter/Movie_Data_Lorenz/TPA-3rdplasmidconc1to1/tea4s15w_0_002199.tif", path "C:/Analysis_from_Movie_for_RiboTrap_Dieter/Movie_Data_Lorenz/TPA-3rdplasmidconc1to1/tea4s15w_0_002200.tif", path "C:/Analysis_from_Movie_for_RiboTrap_Dieter/Movie_Data_Lorenz/TPA-3rdplasmidconc1to1/tea4s15w_0_002201.tif", path "C:/Analysis_from_Movie_for_RiboTrap_Dieter/Movie_Data_Lorenz/TPA-3rdplasmidconc1to1/tea4s15w_0_002202.tif", path "C:/Analysis_from_Movie_for_RiboTrap_Dieter/Movie_Data_Lorenz/TPA-3rdplasmidconc1to1/tea4s15w_0_002203.tif", path "C:/Analysis_from_Movie_for_RiboTrap_Dieter/Movie_Data_Lorenz/TPA-3rdplasmidconc1to1/tea4s15w_0_002204.tif", path "C:/Analysis_from_Movie_for_RiboTrap_Dieter/Movie_Data_Lorenz/TPA-3rdplasmidconc1to1/tea4s15w_0_002205.tif", path "C:/Analysis_from_Movie_for_RiboTrap_Dieter/Movie_Data_Lorenz/TPA-3rdplasmidconc1to1/tea4s15w_0_002206.tif", path "C:/Analysis_from_Movie_for_RiboTrap_Dieter/Movie_Data_Lorenz/TPA-3rdplasmidconc1to1/tea4s15w_0_002207.tif", path "C:/Analysis_from_Movie_for_RiboTrap_Dieter/Movie_Data_Lorenz/TPA-3rdplasmidconc1to1/tea4s15w_0_002208.tif", path "C:/Analysis_from_Movie_for_RiboTrap_Dieter/Movie_Data_Lorenz/TPA-3rdplasmidconc1to1/tea4s15w_0_002209.tif", path "C:/Analysis_from_Movie_for_RiboTrap_Dieter/Movie_Data_Lorenz/TPA-3rdplasmidconc1to1/tea4s15w_0_002210.tif", path "C:/Analysis_from_Movie_for_RiboTrap_Dieter/Movie_Data_Lorenz/TPA-3rdplasmidconc1to1/tea4s15w_0_002211.tif", path "C:/Analysis_from_Movie_for_RiboTrap_Dieter/Movie_Data_Lorenz/TPA-3rdplasmidconc1to1/tea4s15w_0_002212.tif", path "C:/Analysis_from_Movie_for_RiboTrap_Dieter/Movie_Data_Lorenz/TPA-3rdplasmidconc1to1/tea4s15w_0_002213.tif", path "C:/Analysis_from_Movie_for_RiboTrap_Dieter/Movie_Data_Lorenz/TPA-3rdplasmidconc1to1/tea4s15w_0_002214.tif", path "C:/Analysis_from_Movie_for_RiboTrap_Dieter/Movie_Data_Lorenz/TPA-3rdplasmidconc1to1/tea4s15w_0_002215.tif", path "C:/Analysis_from_Movie_for_RiboTrap_Dieter/Movie_Data_Lorenz/TPA-3rdplasmidconc1to1/tea4s15w_0_002216.tif", path "C:/Analysis_from_Movie_for_RiboTrap_Dieter/Movie_Data_Lorenz/TPA-3rdplasmidconc1to1/tea4s15w_0_002217.tif", path "C:/Analysis_from_Movie_for_RiboTrap_Dieter/Movie_Data_Lorenz/TPA-3rdplasmidconc1to1/tea4s15w_0_002218.tif", path "C:/Analysis_from_Movie_for_RiboTrap_Dieter/Movie_Data_Lorenz/TPA-3rdplasmidconc1to1/tea4s15w_0_002219.tif", path "C:/Analysis_from_Movie_for_RiboTrap_Dieter/Movie_Data_Lorenz/TPA-3rdplasmidconc1to1/tea4s15w_0_002220.tif", path "C:/Analysis_from_Movie_for_RiboTrap_Dieter/Movie_Data_Lorenz/TPA-3rdplasmidconc1to1/tea4s15w_0_002221.tif", path "C:/Analysis_from_Movie_for_RiboTrap_Dieter/Movie_Data_Lorenz/TPA-3rdplasmidconc1to1/tea4s15w_0_002222.tif", path "C:/Analysis_from_Movie_for_RiboTrap_Dieter/Movie_Data_Lorenz/TPA-3rdplasmidconc1to1/tea4s15w_0_002223.tif", path "C:/Analysis_from_Movie_for_RiboTrap_Dieter/Movie_Data_Lorenz/TPA-3rdplasmidconc1to1/tea4s15w_0_002224.tif", path "C:/Analysis_from_Movie_for_RiboTrap_Dieter/Movie_Data_Lorenz/TPA-3rdplasmidconc1to1/tea4s15w_0_002225.tif", path "C:/Analysis_from_Movie_for_RiboTrap_Dieter/Movie_Data_Lorenz/TPA-3rdplasmidconc1to1/tea4s15w_0_002226.tif", path "C:/Analysis_from_Movie_for_RiboTrap_Dieter/Movie_Data_Lorenz/TPA-3rdplasmidconc1to1/tea4s15w_0_002227.tif", path "C:/Analysis_from_Movie_for_RiboTrap_Dieter/Movie_Data_Lorenz/TPA-3rdplasmidconc1to1/tea4s15w_0_002228.tif", path "C:/Analysis_from_Movie_for_RiboTrap_Dieter/Movie_Data_Lorenz/TPA-3rdplasmidconc1to1/tea4s15w_0_002229.tif", path "C:/Analysis_from_Movie_for_RiboTrap_Dieter/Movie_Data_Lorenz/TPA-3rdplasmidconc1to1/tea4s15w_0_002230.tif", path "C:/Analysis_from_Movie_for_RiboTrap_Dieter/Movie_Data_Lorenz/TPA-3rdplasmidconc1to1/tea4s15w_0_002231.tif", path "C:/Analysis_from_Movie_for_RiboTrap_Dieter/Movie_Data_Lorenz/TPA-3rdplasmidconc1to1/tea4s15w_0_002232.tif", path "C:/Analysis_from_Movie_for_RiboTrap_Dieter/Movie_Data_Lorenz/TPA-3rdplasmidconc1to1/tea4s15w_0_002233.tif", path "C:/Analysis_from_Movie_for_RiboTrap_Dieter/Movie_Data_Lorenz/TPA-3rdplasmidconc1to1/tea4s15w_0_002234.tif", path "C:/Analysis_from_Movie_for_RiboTrap_Dieter/Movie_Data_Lorenz/TPA-3rdplasmidconc1to1/tea4s15w_0_002235.tif", path "C:/Analysis_from_Movie_for_RiboTrap_Dieter/Movie_Data_Lorenz/TPA-3rdplasmidconc1to1/tea4s15w_0_002236.tif", path "C:/Analysis_from_Movie_for_RiboTrap_Dieter/Movie_Data_Lorenz/TPA-3rdplasmidconc1to1/tea4s15w_0_002237.tif", path "C:/Analysis_from_Movie_for_RiboTrap_Dieter/Movie_Data_Lorenz/TPA-3rdplasmidconc1to1/tea4s15w_0_002238.tif", path "C:/Analysis_from_Movie_for_RiboTrap_Dieter/Movie_Data_Lorenz/TPA-3rdplasmidconc1to1/tea4s15w_0_002239.tif", path "C:/Analysis_from_Movie_for_RiboTrap_Dieter/Movie_Data_Lorenz/TPA-3rdplasmidconc1to1/tea4s15w_0_002240.tif", path "C:/Analysis_from_Movie_for_RiboTrap_Dieter/Movie_Data_Lorenz/TPA-3rdplasmidconc1to1/tea4s15w_0_002241.tif", path "C:/Analysis_from_Movie_for_RiboTrap_Dieter/Movie_Data_Lorenz/TPA-3rdplasmidconc1to1/tea4s15w_0_002242.tif", path "C:/Analysis_from_Movie_for_RiboTrap_Dieter/Movie_Data_Lorenz/TPA-3rdplasmidconc1to1/tea4s15w_0_002243.tif", path "C:/Analysis_from_Movie_for_RiboTrap_Dieter/Movie_Data_Lorenz/TPA-3rdplasmidconc1to1/tea4s15w_0_002244.tif", path "C:/Analysis_from_Movie_for_RiboTrap_Dieter/Movie_Data_Lorenz/TPA-3rdplasmidconc1to1/tea4s15w_0_002245.tif", path "C:/Analysis_from_Movie_for_RiboTrap_Dieter/Movie_Data_Lorenz/TPA-3rdplasmidconc1to1/tea4s15w_0_002246.tif", path "C:/Analysis_from_Movie_for_RiboTrap_Dieter/Movie_Data_Lorenz/TPA-3rdplasmidconc1to1/tea4s15w_0_002247.tif", path "C:/Analysis_from_Movie_for_RiboTrap_Dieter/Movie_Data_Lorenz/TPA-3rdplasmidconc1to1/tea4s15w_0_002248.tif", path "C:/Analysis_from_Movie_for_RiboTrap_Dieter/Movie_Data_Lorenz/TPA-3rdplasmidconc1to1/tea4s15w_0_002249.tif", path "C:/Analysis_from_Movie_for_RiboTrap_Dieter/Movie_Data_Lorenz/TPA-3rdplasmidconc1to1/tea4s15w_0_002250.tif", path "C:/Analysis_from_Movie_for_RiboTrap_Dieter/Movie_Data_Lorenz/TPA-3rdplasmidconc1to1/tea4s15w_0_002251.tif", path "C:/Analysis_from_Movie_for_RiboTrap_Dieter/Movie_Data_Lorenz/TPA-3rdplasmidconc1to1/tea4s15w_0_002252.tif", path "C:/Analysis_from_Movie_for_RiboTrap_Dieter/Movie_Data_Lorenz/TPA-3rdplasmidconc1to1/tea4s15w_0_002253.tif", path "C:/Analysis_from_Movie_for_RiboTrap_Dieter/Movie_Data_Lorenz/TPA-3rdplasmidconc1to1/tea4s15w_0_002254.tif", path "C:/Analysis_from_Movie_for_RiboTrap_Dieter/Movie_Data_Lorenz/TPA-3rdplasmidconc1to1/tea4s15w_0_002255.tif", path "C:/Analysis_from_Movie_for_RiboTrap_Dieter/Movie_Data_Lorenz/TPA-3rdplasmidconc1to1/tea4s15w_0_002256.tif", path "C:/Analysis_from_Movie_for_RiboTrap_Dieter/Movie_Data_Lorenz/TPA-3rdplasmidconc1to1/tea4s15w_0_002257.tif", path "C:/Analysis_from_Movie_for_RiboTrap_Dieter/Movie_Data_Lorenz/TPA-3rdplasmidconc1to1/tea4s15w_0_002258.tif", path "C:/Analysis_from_Movie_for_RiboTrap_Dieter/Movie_Data_Lorenz/TPA-3rdplasmidconc1to1/tea4s15w_0_002259.tif", path "C:/Analysis_from_Movie_for_RiboTrap_Dieter/Movie_Data_Lorenz/TPA-3rdplasmidconc1to1/tea4s15w_0_002260.tif", path "C:/Analysis_from_Movie_for_RiboTrap_Dieter/Movie_Data_Lorenz/TPA-3rdplasmidconc1to1/tea4s15w_0_002261.tif", path "C:/Analysis_from_Movie_for_RiboTrap_Dieter/Movie_Data_Lorenz/TPA-3rdplasmidconc1to1/tea4s15w_0_002262.tif", path "C:/Analysis_from_Movie_for_RiboTrap_Dieter/Movie_Data_Lorenz/TPA-3rdplasmidconc1to1/tea4s15w_0_002263.tif", path "C:/Analysis_from_Movie_for_RiboTrap_Dieter/Movie_Data_Lorenz/TPA-3rdplasmidconc1to1/tea4s15w_0_002264.tif", path "C:/Analysis_from_Movie_for_RiboTrap_Dieter/Movie_Data_Lorenz/TPA-3rdplasmidconc1to1/tea4s15w_0_002265.tif", path "C:/Analysis_from_Movie_for_RiboTrap_Dieter/Movie_Data_Lorenz/TPA-3rdplasmidconc1to1/tea4s15w_0_002266.tif", path "C:/Analysis_from_Movie_for_RiboTrap_Dieter/Movie_Data_Lorenz/TPA-3rdplasmidconc1to1/tea4s15w_0_002267.tif", path "C:/Analysis_from_Movie_for_RiboTrap_Dieter/Movie_Data_Lorenz/TPA-3rdplasmidconc1to1/tea4s15w_0_002268.tif", path "C:/Analysis_from_Movie_for_RiboTrap_Dieter/Movie_Data_Lorenz/TPA-3rdplasmidconc1to1/tea4s15w_0_002269.tif", path "C:/Analysis_from_Movie_for_RiboTrap_Dieter/Movie_Data_Lorenz/TPA-3rdplasmidconc1to1/tea4s15w_0_002270.tif", path "C:/Analysis_from_Movie_for_RiboTrap_Dieter/Movie_Data_Lorenz/TPA-3rdplasmidconc1to1/tea4s15w_0_002271.tif", path "C:/Analysis_from_Movie_for_RiboTrap_Dieter/Movie_Data_Lorenz/TPA-3rdplasmidconc1to1/tea4s15w_0_002272.tif", path "C:/Analysis_from_Movie_for_RiboTrap_Dieter/Movie_Data_Lorenz/TPA-3rdplasmidconc1to1/tea4s15w_0_002273.tif", path "C:/Analysis_from_Movie_for_RiboTrap_Dieter/Movie_Data_Lorenz/TPA-3rdplasmidconc1to1/tea4s15w_0_002274.tif", path "C:/Analysis_from_Movie_for_RiboTrap_Dieter/Movie_Data_Lorenz/TPA-3rdplasmidconc1to1/tea4s15w_0_002275.tif", path "C:/Analysis_from_Movie_for_RiboTrap_Dieter/Movie_Data_Lorenz/TPA-3rdplasmidconc1to1/tea4s15w_0_002276.tif", path "C:/Analysis_from_Movie_for_RiboTrap_Dieter/Movie_Data_Lorenz/TPA-3rdplasmidconc1to1/tea4s15w_0_002277.tif", path "C:/Analysis_from_Movie_for_RiboTrap_Dieter/Movie_Data_Lorenz/TPA-3rdplasmidconc1to1/tea4s15w_0_002278.tif", path "C:/Analysis_from_Movie_for_RiboTrap_Dieter/Movie_Data_Lorenz/TPA-3rdplasmidconc1to1/tea4s15w_0_002279.tif", path "C:/Analysis_from_Movie_for_RiboTrap_Dieter/Movie_Data_Lorenz/TPA-3rdplasmidconc1to1/tea4s15w_0_002280.tif", path "C:/Analysis_from_Movie_for_RiboTrap_Dieter/Movie_Data_Lorenz/TPA-3rdplasmidconc1to1/tea4s15w_0_002281.tif", path "C:/Analysis_from_Movie_for_RiboTrap_Dieter/Movie_Data_Lorenz/TPA-3rdplasmidconc1to1/tea4s15w_0_002282.tif", path "C:/Analysis_from_Movie_for_RiboTrap_Dieter/Movie_Data_Lorenz/TPA-3rdplasmidconc1to1/tea4s15w_0_002283.tif", path "C:/Analysis_from_Movie_for_RiboTrap_Dieter/Movie_Data_Lorenz/TPA-3rdplasmidconc1to1/tea4s15w_0_002284.tif", path "C:/Analysis_from_Movie_for_RiboTrap_Dieter/Movie_Data_Lorenz/TPA-3rdplasmidconc1to1/tea4s15w_0_002285.tif", path "C:/Analysis_from_Movie_for_RiboTrap_Dieter/Movie_Data_Lorenz/TPA-3rdplasmidconc1to1/tea4s15w_0_002286.tif", path "C:/Analysis_from_Movie_for_RiboTrap_Dieter/Movie_Data_Lorenz/TPA-3rdplasmidconc1to1/tea4s15w_0_002287.tif", path "C:/Analysis_from_Movie_for_RiboTrap_Dieter/Movie_Data_Lorenz/TPA-3rdplasmidconc1to1/tea4s15w_0_002288.tif", path "C:/Analysis_from_Movie_for_RiboTrap_Dieter/Movie_Data_Lorenz/TPA-3rdplasmidconc1to1/tea4s15w_0_002289.tif", path "C:/Analysis_from_Movie_for_RiboTrap_Dieter/Movie_Data_Lorenz/TPA-3rdplasmidconc1to1/tea4s15w_0_002290.tif", path "C:/Analysis_from_Movie_for_RiboTrap_Dieter/Movie_Data_Lorenz/TPA-3rdplasmidconc1to1/tea4s15w_0_002291.tif", path "C:/Analysis_from_Movie_for_RiboTrap_Dieter/Movie_Data_Lorenz/TPA-3rdplasmidconc1to1/tea4s15w_0_002292.tif", path "C:/Analysis_from_Movie_for_RiboTrap_Dieter/Movie_Data_Lorenz/TPA-3rdplasmidconc1to1/tea4s15w_0_002293.tif", path "C:/Analysis_from_Movie_for_RiboTrap_Dieter/Movie_Data_Lorenz/TPA-3rdplasmidconc1to1/tea4s15w_0_002294.tif", path "C:/Analysis_from_Movie_for_RiboTrap_Dieter/Movie_Data_Lorenz/TPA-3rdplasmidconc1to1/tea4s15w_0_002295.tif", path "C:/Analysis_from_Movie_for_RiboTrap_Dieter/Movie_Data_Lorenz/TPA-3rdplasmidconc1to1/tea4s15w_0_002296.tif", path "C:/Analysis_from_Movie_for_RiboTrap_Dieter/Movie_Data_Lorenz/TPA-3rdplasmidconc1to1/tea4s15w_0_002297.tif", path "C:/Analysis_from_Movie_for_RiboTrap_Dieter/Movie_Data_Lorenz/TPA-3rdplasmidconc1to1/tea4s15w_0_002298.tif", path "C:/Analysis_from_Movie_for_RiboTrap_Dieter/Movie_Data_Lorenz/TPA-3rdplasmidconc1to1/tea4s15w_0_002299.tif", path "C:/Analysis_from_Movie_for_RiboTrap_Dieter/Movie_Data_Lorenz/TPA-3rdplasmidconc1to1/tea4s15w_0_002300.tif", path "C:/Analysis_from_Movie_for_RiboTrap_Dieter/Movie_Data_Lorenz/TPA-3rdplasmidconc1to1/tea4s15w_0_002301.tif", path "C:/Analysis_from_Movie_for_RiboTrap_Dieter/Movie_Data_Lorenz/TPA-3rdplasmidconc1to1/tea4s15w_0_002302.tif", path "C:/Analysis_from_Movie_for_RiboTrap_Dieter/Movie_Data_Lorenz/TPA-3rdplasmidconc1to1/tea4s15w_0_002303.tif", path "C:/Analysis_from_Movie_for_RiboTrap_Dieter/Movie_Data_Lorenz/TPA-3rdplasmidconc1to1/tea4s15w_0_002304.tif", path "C:/Analysis_from_Movie_for_RiboTrap_Dieter/Movie_Data_Lorenz/TPA-3rdplasmidconc1to1/tea4s15w_0_002305.tif", path "C:/Analysis_from_Movie_for_RiboTrap_Dieter/Movie_Data_Lorenz/TPA-3rdplasmidconc1to1/tea4s15w_0_002306.tif", path "C:/Analysis_from_Movie_for_RiboTrap_Dieter/Movie_Data_Lorenz/TPA-3rdplasmidconc1to1/tea4s15w_0_002307.tif", path "C:/Analysis_from_Movie_for_RiboTrap_Dieter/Movie_Data_Lorenz/TPA-3rdplasmidconc1to1/tea4s15w_0_002308.tif", path "C:/Analysis_from_Movie_for_RiboTrap_Dieter/Movie_Data_Lorenz/TPA-3rdplasmidconc1to1/tea4s15w_0_002309.tif", path "C:/Analysis_from_Movie_for_RiboTrap_Dieter/Movie_Data_Lorenz/TPA-3rdplasmidconc1to1/tea4s15w_0_002310.tif", path "C:/Analysis_from_Movie_for_RiboTrap_Dieter/Movie_Data_Lorenz/TPA-3rdplasmidconc1to1/tea4s15w_0_002311.tif", path "C:/Analysis_from_Movie_for_RiboTrap_Dieter/Movie_Data_Lorenz/TPA-3rdplasmidconc1to1/tea4s15w_0_002312.tif", path "C:/Analysis_from_Movie_for_RiboTrap_Dieter/Movie_Data_Lorenz/TPA-3rdplasmidconc1to1/tea4s15w_0_002313.tif", path "C:/Analysis_from_Movie_for_RiboTrap_Dieter/Movie_Data_Lorenz/TPA-3rdplasmidconc1to1/tea4s15w_0_002314.tif", path "C:/Analysis_from_Movie_for_RiboTrap_Dieter/Movie_Data_Lorenz/TPA-3rdplasmidconc1to1/tea4s15w_0_002315.tif", path "C:/Analysis_from_Movie_for_RiboTrap_Dieter/Movie_Data_Lorenz/TPA-3rdplasmidconc1to1/tea4s15w_0_002316.tif", path "C:/Analysis_from_Movie_for_RiboTrap_Dieter/Movie_Data_Lorenz/TPA-3rdplasmidconc1to1/tea4s15w_0_002317.tif", path "C:/Analysis_from_Movie_for_RiboTrap_Dieter/Movie_Data_Lorenz/TPA-3rdplasmidconc1to1/tea4s15w_0_002318.tif", path "C:/Analysis_from_Movie_for_RiboTrap_Dieter/Movie_Data_Lorenz/TPA-3rdplasmidconc1to1/tea4s15w_0_002319.tif", path "C:/Analysis_from_Movie_for_RiboTrap_Dieter/Movie_Data_Lorenz/TPA-3rdplasmidconc1to1/tea4s15w_0_002320.tif", path "C:/Analysis_from_Movie_for_RiboTrap_Dieter/Movie_Data_Lorenz/TPA-3rdplasmidconc1to1/tea4s15w_0_002321.tif", path "C:/Analysis_from_Movie_for_RiboTrap_Dieter/Movie_Data_Lorenz/TPA-3rdplasmidconc1to1/tea4s15w_0_002322.tif", path "C:/Analysis_from_Movie_for_RiboTrap_Dieter/Movie_Data_Lorenz/TPA-3rdplasmidconc1to1/tea4s15w_0_002323.tif", path "C:/Analysis_from_Movie_for_RiboTrap_Dieter/Movie_Data_Lorenz/TPA-3rdplasmidconc1to1/tea4s15w_0_002324.tif", path "C:/Analysis_from_Movie_for_RiboTrap_Dieter/Movie_Data_Lorenz/TPA-3rdplasmidconc1to1/tea4s15w_0_002325.tif", path "C:/Analysis_from_Movie_for_RiboTrap_Dieter/Movie_Data_Lorenz/TPA-3rdplasmidconc1to1/tea4s15w_0_002326.tif", path "C:/Analysis_from_Movie_for_RiboTrap_Dieter/Movie_Data_Lorenz/TPA-3rdplasmidconc1to1/tea4s15w_0_002327.tif", path "C:/Analysis_from_Movie_for_RiboTrap_Dieter/Movie_Data_Lorenz/TPA-3rdplasmidconc1to1/tea4s15w_0_002328.tif", path "C:/Analysis_from_Movie_for_RiboTrap_Dieter/Movie_Data_Lorenz/TPA-3rdplasmidconc1to1/tea4s15w_0_002329.tif", path "C:/Analysis_from_Movie_for_RiboTrap_Dieter/Movie_Data_Lorenz/TPA-3rdplasmidconc1to1/tea4s15w_0_002330.tif", path "C:/Analysis_from_Movie_for_RiboTrap_Dieter/Movie_Data_Lorenz/TPA-3rdplasmidconc1to1/tea4s15w_0_002331.tif", path "C:/Analysis_from_Movie_for_RiboTrap_Dieter/Movie_Data_Lorenz/TPA-3rdplasmidconc1to1/tea4s15w_0_002332.tif", path "C:/Analysis_from_Movie_for_RiboTrap_Dieter/Movie_Data_Lorenz/TPA-3rdplasmidconc1to1/tea4s15w_0_002333.tif", path "C:/Analysis_from_Movie_for_RiboTrap_Dieter/Movie_Data_Lorenz/TPA-3rdplasmidconc1to1/tea4s15w_0_002334.tif", path "C:/Analysis_from_Movie_for_RiboTrap_Dieter/Movie_Data_Lorenz/TPA-3rdplasmidconc1to1/tea4s15w_0_002335.tif", path "C:/Analysis_from_Movie_for_RiboTrap_Dieter/Movie_Data_Lorenz/TPA-3rdplasmidconc1to1/tea4s15w_0_002336.tif", path "C:/Analysis_from_Movie_for_RiboTrap_Dieter/Movie_Data_Lorenz/TPA-3rdplasmidconc1to1/tea4s15w_0_002337.tif", path "C:/Analysis_from_Movie_for_RiboTrap_Dieter/Movie_Data_Lorenz/TPA-3rdplasmidconc1to1/tea4s15w_0_002338.tif", path "C:/Analysis_from_Movie_for_RiboTrap_Dieter/Movie_Data_Lorenz/TPA-3rdplasmidconc1to1/tea4s15w_0_002339.tif", path "C:/Analysis_from_Movie_for_RiboTrap_Dieter/Movie_Data_Lorenz/TPA-3rdplasmidconc1to1/tea4s15w_0_002340.tif", path "C:/Analysis_from_Movie_for_RiboTrap_Dieter/Movie_Data_Lorenz/TPA-3rdplasmidconc1to1/tea4s15w_0_002341.tif", path "C:/Analysis_from_Movie_for_RiboTrap_Dieter/Movie_Data_Lorenz/TPA-3rdplasmidconc1to1/tea4s15w_0_002342.tif", path "C:/Analysis_from_Movie_for_RiboTrap_Dieter/Movie_Data_Lorenz/TPA-3rdplasmidconc1to1/tea4s15w_0_002343.tif", path "C:/Analysis_from_Movie_for_RiboTrap_Dieter/Movie_Data_Lorenz/TPA-3rdplasmidconc1to1/tea4s15w_0_002344.tif", path "C:/Analysis_from_Movie_for_RiboTrap_Dieter/Movie_Data_Lorenz/TPA-3rdplasmidconc1to1/tea4s15w_0_002345.tif", path "C:/Analysis_from_Movie_for_RiboTrap_Dieter/Movie_Data_Lorenz/TPA-3rdplasmidconc1to1/tea4s15w_0_002346.tif", path "C:/Analysis_from_Movie_for_RiboTrap_Dieter/Movie_Data_Lorenz/TPA-3rdplasmidconc1to1/tea4s15w_0_002347.tif", path "C:/Analysis_from_Movie_for_RiboTrap_Dieter/Movie_Data_Lorenz/TPA-3rdplasmidconc1to1/tea4s15w_0_002348.tif", path "C:/Analysis_from_Movie_for_RiboTrap_Dieter/Movie_Data_Lorenz/TPA-3rdplasmidconc1to1/tea4s15w_0_002349.tif", path "C:/Analysis_from_Movie_for_RiboTrap_Dieter/Movie_Data_Lorenz/TPA-3rdplasmidconc1to1/tea4s15w_0_002350.tif", path "C:/Analysis_from_Movie_for_RiboTrap_Dieter/Movie_Data_Lorenz/TPA-3rdplasmidconc1to1/tea4s15w_0_002351.tif", path "C:/Analysis_from_Movie_for_RiboTrap_Dieter/Movie_Data_Lorenz/TPA-3rdplasmidconc1to1/tea4s15w_0_002352.tif", path "C:/Analysis_from_Movie_for_RiboTrap_Dieter/Movie_Data_Lorenz/TPA-3rdplasmidconc1to1/tea4s15w_0_002353.tif", path "C:/Analysis_from_Movie_for_RiboTrap_Dieter/Movie_Data_Lorenz/TPA-3rdplasmidconc1to1/tea4s15w_0_002354.tif", path "C:/Analysis_from_Movie_for_RiboTrap_Dieter/Movie_Data_Lorenz/TPA-3rdplasmidconc1to1/tea4s15w_0_002355.tif", path "C:/Analysis_from_Movie_for_RiboTrap_Dieter/Movie_Data_Lorenz/TPA-3rdplasmidconc1to1/tea4s15w_0_002356.tif", path "C:/Analysis_from_Movie_for_RiboTrap_Dieter/Movie_Data_Lorenz/TPA-3rdplasmidconc1to1/tea4s15w_0_002357.tif", path "C:/Analysis_from_Movie_for_RiboTrap_Dieter/Movie_Data_Lorenz/TPA-3rdplasmidconc1to1/tea4s15w_0_002358.tif", path "C:/Analysis_from_Movie_for_RiboTrap_Dieter/Movie_Data_Lorenz/TPA-3rdplasmidconc1to1/tea4s15w_0_002359.tif", path "C:/Analysis_from_Movie_for_RiboTrap_Dieter/Movie_Data_Lorenz/TPA-3rdplasmidconc1to1/tea4s15w_0_002360.tif", path "C:/Analysis_from_Movie_for_RiboTrap_Dieter/Movie_Data_Lorenz/TPA-3rdplasmidconc1to1/tea4s15w_0_002361.tif", path "C:/Analysis_from_Movie_for_RiboTrap_Dieter/Movie_Data_Lorenz/TPA-3rdplasmidconc1to1/tea4s15w_0_002362.tif", path "C:/Analysis_from_Movie_for_RiboTrap_Dieter/Movie_Data_Lorenz/TPA-3rdplasmidconc1to1/tea4s15w_0_002363.tif", path "C:/Analysis_from_Movie_for_RiboTrap_Dieter/Movie_Data_Lorenz/TPA-3rdplasmidconc1to1/tea4s15w_0_002364.tif", path "C:/Analysis_from_Movie_for_RiboTrap_Dieter/Movie_Data_Lorenz/TPA-3rdplasmidconc1to1/tea4s15w_0_002365.tif", path "C:/Analysis_from_Movie_for_RiboTrap_Dieter/Movie_Data_Lorenz/TPA-3rdplasmidconc1to1/tea4s15w_0_002366.tif", path "C:/Analysis_from_Movie_for_RiboTrap_Dieter/Movie_Data_Lorenz/TPA-3rdplasmidconc1to1/tea4s15w_0_002367.tif", path "C:/Analysis_from_Movie_for_RiboTrap_Dieter/Movie_Data_Lorenz/TPA-3rdplasmidconc1to1/tea4s15w_0_002368.tif", path "C:/Analysis_from_Movie_for_RiboTrap_Dieter/Movie_Data_Lorenz/TPA-3rdplasmidconc1to1/tea4s15w_0_002369.tif", path "C:/Analysis_from_Movie_for_RiboTrap_Dieter/Movie_Data_Lorenz/TPA-3rdplasmidconc1to1/tea4s15w_0_002370.tif", path "C:/Analysis_from_Movie_for_RiboTrap_Dieter/Movie_Data_Lorenz/TPA-3rdplasmidconc1to1/tea4s15w_0_002371.tif", path "C:/Analysis_from_Movie_for_RiboTrap_Dieter/Movie_Data_Lorenz/TPA-3rdplasmidconc1to1/tea4s15w_0_002372.tif", path "C:/Analysis_from_Movie_for_RiboTrap_Dieter/Movie_Data_Lorenz/TPA-3rdplasmidconc1to1/tea4s15w_0_002373.tif", path "C:/Analysis_from_Movie_for_RiboTrap_Dieter/Movie_Data_Lorenz/TPA-3rdplasmidconc1to1/tea4s15w_0_002374.tif", path "C:/Analysis_from_Movie_for_RiboTrap_Dieter/Movie_Data_Lorenz/TPA-3rdplasmidconc1to1/tea4s15w_0_002375.tif", path "C:/Analysis_from_Movie_for_RiboTrap_Dieter/Movie_Data_Lorenz/TPA-3rdplasmidconc1to1/tea4s15w_0_002376.tif", path "C:/Analysis_from_Movie_for_RiboTrap_Dieter/Movie_Data_Lorenz/TPA-3rdplasmidconc1to1/tea4s15w_0_002377.tif", path "C:/Analysis_from_Movie_for_RiboTrap_Dieter/Movie_Data_Lorenz/TPA-3rdplasmidconc1to1/tea4s15w_0_002378.tif", path "C:/Analysis_from_Movie_for_RiboTrap_Dieter/Movie_Data_Lorenz/TPA-3rdplasmidconc1to1/tea4s15w_0_002379.tif", path "C:/Analysis_from_Movie_for_RiboTrap_Dieter/Movie_Data_Lorenz/TPA-3rdplasmidconc1to1/tea4s15w_0_002380.tif", path "C:/Analysis_from_Movie_for_RiboTrap_Dieter/Movie_Data_Lorenz/TPA-3rdplasmidconc1to1/tea4s15w_0_002381.tif", path "C:/Analysis_from_Movie_for_RiboTrap_Dieter/Movie_Data_Lorenz/TPA-3rdplasmidconc1to1/tea4s15w_0_002382.tif", path "C:/Analysis_from_Movie_for_RiboTrap_Dieter/Movie_Data_Lorenz/TPA-3rdplasmidconc1to1/tea4s15w_0_002383.tif", path "C:/Analysis_from_Movie_for_RiboTrap_Dieter/Movie_Data_Lorenz/TPA-3rdplasmidconc1to1/tea4s15w_0_002384.tif", path "C:/Analysis_from_Movie_for_RiboTrap_Dieter/Movie_Data_Lorenz/TPA-3rdplasmidconc1to1/tea4s15w_0_002385.tif", path "C:/Analysis_from_Movie_for_RiboTrap_Dieter/Movie_Data_Lorenz/TPA-3rdplasmidconc1to1/tea4s15w_0_002386.tif", path "C:/Analysis_from_Movie_for_RiboTrap_Dieter/Movie_Data_Lorenz/TPA-3rdplasmidconc1to1/tea4s15w_0_002387.tif", path "C:/Analysis_from_Movie_for_RiboTrap_Dieter/Movie_Data_Lorenz/TPA-3rdplasmidconc1to1/tea4s15w_0_002388.tif", path "C:/Analysis_from_Movie_for_RiboTrap_Dieter/Movie_Data_Lorenz/TPA-3rdplasmidconc1to1/tea4s15w_0_002389.tif", path "C:/Analysis_from_Movie_for_RiboTrap_Dieter/Movie_Data_Lorenz/TPA-3rdplasmidconc1to1/tea4s15w_0_002390.tif", path "C:/Analysis_from_Movie_for_RiboTrap_Dieter/Movie_Data_Lorenz/TPA-3rdplasmidconc1to1/tea4s15w_0_002391.tif", path "C:/Analysis_from_Movie_for_RiboTrap_Dieter/Movie_Data_Lorenz/TPA-3rdplasmidconc1to1/tea4s15w_0_002392.tif", path "C:/Analysis_from_Movie_for_RiboTrap_Dieter/Movie_Data_Lorenz/TPA-3rdplasmidconc1to1/tea4s15w_0_002393.tif", path "C:/Analysis_from_Movie_for_RiboTrap_Dieter/Movie_Data_Lorenz/TPA-3rdplasmidconc1to1/tea4s15w_0_002394.tif", path "C:/Analysis_from_Movie_for_RiboTrap_Dieter/Movie_Data_Lorenz/TPA-3rdplasmidconc1to1/tea4s15w_0_002395.tif", path "C:/Analysis_from_Movie_for_RiboTrap_Dieter/Movie_Data_Lorenz/TPA-3rdplasmidconc1to1/tea4s15w_0_002396.tif", path "C:/Analysis_from_Movie_for_RiboTrap_Dieter/Movie_Data_Lorenz/TPA-3rdplasmidconc1to1/tea4s15w_0_002397.tif", path "C:/Analysis_from_Movie_for_RiboTrap_Dieter/Movie_Data_Lorenz/TPA-3rdplasmidconc1to1/tea4s15w_0_002398.tif", path "C:/Analysis_from_Movie_for_RiboTrap_Dieter/Movie_Data_Lorenz/TPA-3rdplasmidconc1to1/tea4s15w_0_002399.tif", path "C:/Analysis_from_Movie_for_RiboTrap_Dieter/Movie_Data_Lorenz/TPA-3rdplasmidconc1to1/tea4s15w_0_002400.tif", path "C:/Analysis_from_Movie_for_RiboTrap_Dieter/Movie_Data_Lorenz/TPA-3rdplasmidconc1to1/tea4s15w_0_002401.tif", path "C:/Analysis_from_Movie_for_RiboTrap_Dieter/Movie_Data_Lorenz/TPA-3rdplasmidconc1to1/tea4s15w_0_002402.tif", path "C:/Analysis_from_Movie_for_RiboTrap_Dieter/Movie_Data_Lorenz/TPA-3rdplasmidconc1to1/tea4s15w_0_002403.tif", path "C:/Analysis_from_Movie_for_RiboTrap_Dieter/Movie_Data_Lorenz/TPA-3rdplasmidconc1to1/tea4s15w_0_002404.tif", path "C:/Analysis_from_Movie_for_RiboTrap_Dieter/Movie_Data_Lorenz/TPA-3rdplasmidconc1to1/tea4s15w_0_002405.tif", path "C:/Analysis_from_Movie_for_RiboTrap_Dieter/Movie_Data_Lorenz/TPA-3rdplasmidconc1to1/tea4s15w_0_002406.tif", path "C:/Analysis_from_Movie_for_RiboTrap_Dieter/Movie_Data_Lorenz/TPA-3rdplasmidconc1to1/tea4s15w_0_002407.tif", path "C:/Analysis_from_Movie_for_RiboTrap_Dieter/Movie_Data_Lorenz/TPA-3rdplasmidconc1to1/tea4s15w_0_002408.tif", path "C:/Analysis_from_Movie_for_RiboTrap_Dieter/Movie_Data_Lorenz/TPA-3rdplasmidconc1to1/tea4s15w_0_002409.tif", path "C:/Analysis_from_Movie_for_RiboTrap_Dieter/Movie_Data_Lorenz/TPA-3rdplasmidconc1to1/tea4s15w_0_002410.tif", path "C:/Analysis_from_Movie_for_RiboTrap_Dieter/Movie_Data_Lorenz/TPA-3rdplasmidconc1to1/tea4s15w_0_002411.tif", path "C:/Analysis_from_Movie_for_RiboTrap_Dieter/Movie_Data_Lorenz/TPA-3rdplasmidconc1to1/tea4s15w_0_002412.tif", path "C:/Analysis_from_Movie_for_RiboTrap_Dieter/Movie_Data_Lorenz/TPA-3rdplasmidconc1to1/tea4s15w_0_002413.tif", path "C:/Analysis_from_Movie_for_RiboTrap_Dieter/Movie_Data_Lorenz/TPA-3rdplasmidconc1to1/tea4s15w_0_002414.tif", path "C:/Analysis_from_Movie_for_RiboTrap_Dieter/Movie_Data_Lorenz/TPA-3rdplasmidconc1to1/tea4s15w_0_002415.tif", path "C:/Analysis_from_Movie_for_RiboTrap_Dieter/Movie_Data_Lorenz/TPA-3rdplasmidconc1to1/tea4s15w_0_002416.tif", path "C:/Analysis_from_Movie_for_RiboTrap_Dieter/Movie_Data_Lorenz/TPA-3rdplasmidconc1to1/tea4s15w_0_002417.tif", path "C:/Analysis_from_Movie_for_RiboTrap_Dieter/Movie_Data_Lorenz/TPA-3rdplasmidconc1to1/tea4s15w_0_002418.tif", path "C:/Analysis_from_Movie_for_RiboTrap_Dieter/Movie_Data_Lorenz/TPA-3rdplasmidconc1to1/tea4s15w_0_002419.tif", path "C:/Analysis_from_Movie_for_RiboTrap_Dieter/Movie_Data_Lorenz/TPA-3rdplasmidconc1to1/tea4s15w_0_002420.tif", path "C:/Analysis_from_Movie_for_RiboTrap_Dieter/Movie_Data_Lorenz/TPA-3rdplasmidconc1to1/tea4s15w_0_002421.tif", path "C:/Analysis_from_Movie_for_RiboTrap_Dieter/Movie_Data_Lorenz/TPA-3rdplasmidconc1to1/tea4s15w_0_002422.tif", path "C:/Analysis_from_Movie_for_RiboTrap_Dieter/Movie_Data_Lorenz/TPA-3rdplasmidconc1to1/tea4s15w_0_002423.tif", path "C:/Analysis_from_Movie_for_RiboTrap_Dieter/Movie_Data_Lorenz/TPA-3rdplasmidconc1to1/tea4s15w_0_002424.tif", path "C:/Analysis_from_Movie_for_RiboTrap_Dieter/Movie_Data_Lorenz/TPA-3rdplasmidconc1to1/tea4s15w_0_002425.tif", path "C:/Analysis_from_Movie_for_RiboTrap_Dieter/Movie_Data_Lorenz/TPA-3rdplasmidconc1to1/tea4s15w_0_002426.tif", path "C:/Analysis_from_Movie_for_RiboTrap_Dieter/Movie_Data_Lorenz/TPA-3rdplasmidconc1to1/tea4s15w_0_002427.tif", path "C:/Analysis_from_Movie_for_RiboTrap_Dieter/Movie_Data_Lorenz/TPA-3rdplasmidconc1to1/tea4s15w_0_002428.tif", path "C:/Analysis_from_Movie_for_RiboTrap_Dieter/Movie_Data_Lorenz/TPA-3rdplasmidconc1to1/tea4s15w_0_002429.tif", path "C:/Analysis_from_Movie_for_RiboTrap_Dieter/Movie_Data_Lorenz/TPA-3rdplasmidconc1to1/tea4s15w_0_002430.tif", path "C:/Analysis_from_Movie_for_RiboTrap_Dieter/Movie_Data_Lorenz/TPA-3rdplasmidconc1to1/tea4s15w_0_002431.tif", path "C:/Analysis_from_Movie_for_RiboTrap_Dieter/Movie_Data_Lorenz/TPA-3rdplasmidconc1to1/tea4s15w_0_002432.tif", path "C:/Analysis_from_Movie_for_RiboTrap_Dieter/Movie_Data_Lorenz/TPA-3rdplasmidconc1to1/tea4s15w_0_002433.tif", path "C:/Analysis_from_Movie_for_RiboTrap_Dieter/Movie_Data_Lorenz/TPA-3rdplasmidconc1to1/tea4s15w_0_002434.tif", path "C:/Analysis_from_Movie_for_RiboTrap_Dieter/Movie_Data_Lorenz/TPA-3rdplasmidconc1to1/tea4s15w_0_002435.tif", path "C:/Analysis_from_Movie_for_RiboTrap_Dieter/Movie_Data_Lorenz/TPA-3rdplasmidconc1to1/tea4s15w_0_002436.tif", path "C:/Analysis_from_Movie_for_RiboTrap_Dieter/Movie_Data_Lorenz/TPA-3rdplasmidconc1to1/tea4s15w_0_002437.tif", path "C:/Analysis_from_Movie_for_RiboTrap_Dieter/Movie_Data_Lorenz/TPA-3rdplasmidconc1to1/tea4s15w_0_002438.tif", path "C:/Analysis_from_Movie_for_RiboTrap_Dieter/Movie_Data_Lorenz/TPA-3rdplasmidconc1to1/tea4s15w_0_002439.tif", path "C:/Analysis_from_Movie_for_RiboTrap_Dieter/Movie_Data_Lorenz/TPA-3rdplasmidconc1to1/tea4s15w_0_002440.tif", path "C:/Analysis_from_Movie_for_RiboTrap_Dieter/Movie_Data_Lorenz/TPA-3rdplasmidconc1to1/tea4s15w_0_002441.tif", path "C:/Analysis_from_Movie_for_RiboTrap_Dieter/Movie_Data_Lorenz/TPA-3rdplasmidconc1to1/tea4s15w_0_002442.tif", path "C:/Analysis_from_Movie_for_RiboTrap_Dieter/Movie_Data_Lorenz/TPA-3rdplasmidconc1to1/tea4s15w_0_002443.tif", path "C:/Analysis_from_Movie_for_RiboTrap_Dieter/Movie_Data_Lorenz/TPA-3rdplasmidconc1to1/tea4s15w_0_002444.tif", path "C:/Analysis_from_Movie_for_RiboTrap_Dieter/Movie_Data_Lorenz/TPA-3rdplasmidconc1to1/tea4s15w_0_002445.tif", path "C:/Analysis_from_Movie_for_RiboTrap_Dieter/Movie_Data_Lorenz/TPA-3rdplasmidconc1to1/tea4s15w_0_002446.tif", path "C:/Analysis_from_Movie_for_RiboTrap_Dieter/Movie_Data_Lorenz/TPA-3rdplasmidconc1to1/tea4s15w_0_002447.tif", path "C:/Analysis_from_Movie_for_RiboTrap_Dieter/Movie_Data_Lorenz/TPA-3rdplasmidconc1to1/tea4s15w_0_002448.tif", path "C:/Analysis_from_Movie_for_RiboTrap_Dieter/Movie_Data_Lorenz/TPA-3rdplasmidconc1to1/tea4s15w_0_002449.tif", path "C:/Analysis_from_Movie_for_RiboTrap_Dieter/Movie_Data_Lorenz/TPA-3rdplasmidconc1to1/tea4s15w_0_002450.tif", path "C:/Analysis_from_Movie_for_RiboTrap_Dieter/Movie_Data_Lorenz/TPA-3rdplasmidconc1to1/tea4s15w_0_002451.tif", path "C:/Analysis_from_Movie_for_RiboTrap_Dieter/Movie_Data_Lorenz/TPA-3rdplasmidconc1to1/tea4s15w_0_002452.tif", path "C:/Analysis_from_Movie_for_RiboTrap_Dieter/Movie_Data_Lorenz/TPA-3rdplasmidconc1to1/tea4s15w_0_002453.tif", path "C:/Analysis_from_Movie_for_RiboTrap_Dieter/Movie_Data_Lorenz/TPA-3rdplasmidconc1to1/tea4s15w_0_002454.tif", path "C:/Analysis_from_Movie_for_RiboTrap_Dieter/Movie_Data_Lorenz/TPA-3rdplasmidconc1to1/tea4s15w_0_002455.tif", path "C:/Analysis_from_Movie_for_RiboTrap_Dieter/Movie_Data_Lorenz/TPA-3rdplasmidconc1to1/tea4s15w_0_002456.tif", path "C:/Analysis_from_Movie_for_RiboTrap_Dieter/Movie_Data_Lorenz/TPA-3rdplasmidconc1to1/tea4s15w_0_002457.tif", path "C:/Analysis_from_Movie_for_RiboTrap_Dieter/Movie_Data_Lorenz/TPA-3rdplasmidconc1to1/tea4s15w_0_002458.tif", path "C:/Analysis_from_Movie_for_RiboTrap_Dieter/Movie_Data_Lorenz/TPA-3rdplasmidconc1to1/tea4s15w_0_002459.tif", path "C:/Analysis_from_Movie_for_RiboTrap_Dieter/Movie_Data_Lorenz/TPA-3rdplasmidconc1to1/tea4s15w_0_002460.tif", path "C:/Analysis_from_Movie_for_RiboTrap_Dieter/Movie_Data_Lorenz/TPA-3rdplasmidconc1to1/tea4s15w_0_002461.tif", path "C:/Analysis_from_Movie_for_RiboTrap_Dieter/Movie_Data_Lorenz/TPA-3rdplasmidconc1to1/tea4s15w_0_002462.tif", path "C:/Analysis_from_Movie_for_RiboTrap_Dieter/Movie_Data_Lorenz/TPA-3rdplasmidconc1to1/tea4s15w_0_002463.tif", path "C:/Analysis_from_Movie_for_RiboTrap_Dieter/Movie_Data_Lorenz/TPA-3rdplasmidconc1to1/tea4s15w_0_002464.tif", path "C:/Analysis_from_Movie_for_RiboTrap_Dieter/Movie_Data_Lorenz/TPA-3rdplasmidconc1to1/tea4s15w_0_002465.tif", path "C:/Analysis_from_Movie_for_RiboTrap_Dieter/Movie_Data_Lorenz/TPA-3rdplasmidconc1to1/tea4s15w_0_002466.tif", path "C:/Analysis_from_Movie_for_RiboTrap_Dieter/Movie_Data_Lorenz/TPA-3rdplasmidconc1to1/tea4s15w_0_002467.tif", path "C:/Analysis_from_Movie_for_RiboTrap_Dieter/Movie_Data_Lorenz/TPA-3rdplasmidconc1to1/tea4s15w_0_002468.tif", path "C:/Analysis_from_Movie_for_RiboTrap_Dieter/Movie_Data_Lorenz/TPA-3rdplasmidconc1to1/tea4s15w_0_002469.tif", path "C:/Analysis_from_Movie_for_RiboTrap_Dieter/Movie_Data_Lorenz/TPA-3rdplasmidconc1to1/tea4s15w_0_002470.tif", path "C:/Analysis_from_Movie_for_RiboTrap_Dieter/Movie_Data_Lorenz/TPA-3rdplasmidconc1to1/tea4s15w_0_002471.tif", path "C:/Analysis_from_Movie_for_RiboTrap_Dieter/Movie_Data_Lorenz/TPA-3rdplasmidconc1to1/tea4s15w_0_002472.tif", path "C:/Analysis_from_Movie_for_RiboTrap_Dieter/Movie_Data_Lorenz/TPA-3rdplasmidconc1to1/tea4s15w_0_002473.tif", path "C:/Analysis_from_Movie_for_RiboTrap_Dieter/Movie_Data_Lorenz/TPA-3rdplasmidconc1to1/tea4s15w_0_002474.tif", path "C:/Analysis_from_Movie_for_RiboTrap_Dieter/Movie_Data_Lorenz/TPA-3rdplasmidconc1to1/tea4s15w_0_002475.tif", path "C:/Analysis_from_Movie_for_RiboTrap_Dieter/Movie_Data_Lorenz/TPA-3rdplasmidconc1to1/tea4s15w_0_002476.tif", path "C:/Analysis_from_Movie_for_RiboTrap_Dieter/Movie_Data_Lorenz/TPA-3rdplasmidconc1to1/tea4s15w_0_002477.tif", path "C:/Analysis_from_Movie_for_RiboTrap_Dieter/Movie_Data_Lorenz/TPA-3rdplasmidconc1to1/tea4s15w_0_002478.tif", path "C:/Analysis_from_Movie_for_RiboTrap_Dieter/Movie_Data_Lorenz/TPA-3rdplasmidconc1to1/tea4s15w_0_002479.tif", path "C:/Analysis_from_Movie_for_RiboTrap_Dieter/Movie_Data_Lorenz/TPA-3rdplasmidconc1to1/tea4s15w_0_002480.tif", path "C:/Analysis_from_Movie_for_RiboTrap_Dieter/Movie_Data_Lorenz/TPA-3rdplasmidconc1to1/tea4s15w_0_002481.tif", path "C:/Analysis_from_Movie_for_RiboTrap_Dieter/Movie_Data_Lorenz/TPA-3rdplasmidconc1to1/tea4s15w_0_002482.tif", path "C:/Analysis_from_Movie_for_RiboTrap_Dieter/Movie_Data_Lorenz/TPA-3rdplasmidconc1to1/tea4s15w_0_002483.tif", path "C:/Analysis_from_Movie_for_RiboTrap_Dieter/Movie_Data_Lorenz/TPA-3rdplasmidconc1to1/tea4s15w_0_002484.tif", path "C:/Analysis_from_Movie_for_RiboTrap_Dieter/Movie_Data_Lorenz/TPA-3rdplasmidconc1to1/tea4s15w_0_002485.tif", path "C:/Analysis_from_Movie_for_RiboTrap_Dieter/Movie_Data_Lorenz/TPA-3rdplasmidconc1to1/tea4s15w_0_002486.tif", path "C:/Analysis_from_Movie_for_RiboTrap_Dieter/Movie_Data_Lorenz/TPA-3rdplasmidconc1to1/tea4s15w_0_002487.tif", path "C:/Analysis_from_Movie_for_RiboTrap_Dieter/Movie_Data_Lorenz/TPA-3rdplasmidconc1to1/tea4s15w_0_002488.tif", path "C:/Analysis_from_Movie_for_RiboTrap_Dieter/Movie_Data_Lorenz/TPA-3rdplasmidconc1to1/tea4s15w_0_002489.tif", path "C:/Analysis_from_Movie_for_RiboTrap_Dieter/Movie_Data_Lorenz/TPA-3rdplasmidconc1to1/tea4s15w_0_002490.tif", path "C:/Analysis_from_Movie_for_RiboTrap_Dieter/Movie_Data_Lorenz/TPA-3rdplasmidconc1to1/tea4s15w_0_002491.tif", path "C:/Analysis_from_Movie_for_RiboTrap_Dieter/Movie_Data_Lorenz/TPA-3rdplasmidconc1to1/tea4s15w_0_002492.tif", path "C:/Analysis_from_Movie_for_RiboTrap_Dieter/Movie_Data_Lorenz/TPA-3rdplasmidconc1to1/tea4s15w_0_002493.tif", path "C:/Analysis_from_Movie_for_RiboTrap_Dieter/Movie_Data_Lorenz/TPA-3rdplasmidconc1to1/tea4s15w_0_002494.tif", path "C:/Analysis_from_Movie_for_RiboTrap_Dieter/Movie_Data_Lorenz/TPA-3rdplasmidconc1to1/tea4s15w_0_002495.tif", path "C:/Analysis_from_Movie_for_RiboTrap_Dieter/Movie_Data_Lorenz/TPA-3rdplasmidconc1to1/tea4s15w_0_002496.tif", path "C:/Analysis_from_Movie_for_RiboTrap_Dieter/Movie_Data_Lorenz/TPA-3rdplasmidconc1to1/tea4s15w_0_002497.tif", path "C:/Analysis_from_Movie_for_RiboTrap_Dieter/Movie_Data_Lorenz/TPA-3rdplasmidconc1to1/tea4s15w_0_002498.tif", path "C:/Analysis_from_Movie_for_RiboTrap_Dieter/Movie_Data_Lorenz/TPA-3rdplasmidconc1to1/tea4s15w_0_002499.tif", path "C:/Analysis_from_Movie_for_RiboTrap_Dieter/Movie_Data_Lorenz/TPA-3rdplasmidconc1to1/tea4s15w_0_002500.tif", path "C:/Analysis_from_Movie_for_RiboTrap_Dieter/Movie_Data_Lorenz/TPA-3rdplasmidconc1to1/tea4s15w_0_002501.tif", path "C:/Analysis_from_Movie_for_RiboTrap_Dieter/Movie_Data_Lorenz/TPA-3rdplasmidconc1to1/tea4s15w_0_002502.tif", path "C:/Analysis_from_Movie_for_RiboTrap_Dieter/Movie_Data_Lorenz/TPA-3rdplasmidconc1to1/tea4s15w_0_002503.tif", path "C:/Analysis_from_Movie_for_RiboTrap_Dieter/Movie_Data_Lorenz/TPA-3rdplasmidconc1to1/tea4s15w_0_002504.tif", path "C:/Analysis_from_Movie_for_RiboTrap_Dieter/Movie_Data_Lorenz/TPA-3rdplasmidconc1to1/tea4s15w_0_002505.tif", path "C:/Analysis_from_Movie_for_RiboTrap_Dieter/Movie_Data_Lorenz/TPA-3rdplasmidconc1to1/tea4s15w_0_002506.tif", path "C:/Analysis_from_Movie_for_RiboTrap_Dieter/Movie_Data_Lorenz/TPA-3rdplasmidconc1to1/tea4s15w_0_002507.tif", path "C:/Analysis_from_Movie_for_RiboTrap_Dieter/Movie_Data_Lorenz/TPA-3rdplasmidconc1to1/tea4s15w_0_002508.tif", path "C:/Analysis_from_Movie_for_RiboTrap_Dieter/Movie_Data_Lorenz/TPA-3rdplasmidconc1to1/tea4s15w_0_002509.tif", path "C:/Analysis_from_Movie_for_RiboTrap_Dieter/Movie_Data_Lorenz/TPA-3rdplasmidconc1to1/tea4s15w_0_002510.tif", path "C:/Analysis_from_Movie_for_RiboTrap_Dieter/Movie_Data_Lorenz/TPA-3rdplasmidconc1to1/tea4s15w_0_002511.tif", path "C:/Analysis_from_Movie_for_RiboTrap_Dieter/Movie_Data_Lorenz/TPA-3rdplasmidconc1to1/tea4s15w_0_002512.tif", path "C:/Analysis_from_Movie_for_RiboTrap_Dieter/Movie_Data_Lorenz/TPA-3rdplasmidconc1to1/tea4s15w_0_002513.tif", path "C:/Analysis_from_Movie_for_RiboTrap_Dieter/Movie_Data_Lorenz/TPA-3rdplasmidconc1to1/tea4s15w_0_002514.tif", path "C:/Analysis_from_Movie_for_RiboTrap_Dieter/Movie_Data_Lorenz/TPA-3rdplasmidconc1to1/tea4s15w_0_002515.tif", path "C:/Analysis_from_Movie_for_RiboTrap_Dieter/Movie_Data_Lorenz/TPA-3rdplasmidconc1to1/tea4s15w_0_002516.tif", path "C:/Analysis_from_Movie_for_RiboTrap_Dieter/Movie_Data_Lorenz/TPA-3rdplasmidconc1to1/tea4s15w_0_002517.tif", path "C:/Analysis_from_Movie_for_RiboTrap_Dieter/Movie_Data_Lorenz/TPA-3rdplasmidconc1to1/tea4s15w_0_002518.tif", path "C:/Analysis_from_Movie_for_RiboTrap_Dieter/Movie_Data_Lorenz/TPA-3rdplasmidconc1to1/tea4s15w_0_002519.tif", path "C:/Analysis_from_Movie_for_RiboTrap_Dieter/Movie_Data_Lorenz/TPA-3rdplasmidconc1to1/tea4s15w_0_002520.tif", path "C:/Analysis_from_Movie_for_RiboTrap_Dieter/Movie_Data_Lorenz/TPA-3rdplasmidconc1to1/tea4s15w_0_002521.tif", path "C:/Analysis_from_Movie_for_RiboTrap_Dieter/Movie_Data_Lorenz/TPA-3rdplasmidconc1to1/tea4s15w_0_002522.tif", path "C:/Analysis_from_Movie_for_RiboTrap_Dieter/Movie_Data_Lorenz/TPA-3rdplasmidconc1to1/tea4s15w_0_002523.tif", path "C:/Analysis_from_Movie_for_RiboTrap_Dieter/Movie_Data_Lorenz/TPA-3rdplasmidconc1to1/tea4s15w_0_002524.tif", path "C:/Analysis_from_Movie_for_RiboTrap_Dieter/Movie_Data_Lorenz/TPA-3rdplasmidconc1to1/tea4s15w_0_002525.tif", path "C:/Analysis_from_Movie_for_RiboTrap_Dieter/Movie_Data_Lorenz/TPA-3rdplasmidconc1to1/tea4s15w_0_002526.tif", path "C:/Analysis_from_Movie_for_RiboTrap_Dieter/Movie_Data_Lorenz/TPA-3rdplasmidconc1to1/tea4s15w_0_002527.tif", path "C:/Analysis_from_Movie_for_RiboTrap_Dieter/Movie_Data_Lorenz/TPA-3rdplasmidconc1to1/tea4s15w_0_002528.tif", path "C:/Analysis_from_Movie_for_RiboTrap_Dieter/Movie_Data_Lorenz/TPA-3rdplasmidconc1to1/tea4s15w_0_002529.tif", path "C:/Analysis_from_Movie_for_RiboTrap_Dieter/Movie_Data_Lorenz/TPA-3rdplasmidconc1to1/tea4s15w_0_002530.tif", path "C:/Analysis_from_Movie_for_RiboTrap_Dieter/Movie_Data_Lorenz/TPA-3rdplasmidconc1to1/tea4s15w_0_002531.tif", path "C:/Analysis_from_Movie_for_RiboTrap_Dieter/Movie_Data_Lorenz/TPA-3rdplasmidconc1to1/tea4s15w_0_002532.tif", path "C:/Analysis_from_Movie_for_RiboTrap_Dieter/Movie_Data_Lorenz/TPA-3rdplasmidconc1to1/tea4s15w_0_002533.tif", path "C:/Analysis_from_Movie_for_RiboTrap_Dieter/Movie_Data_Lorenz/TPA-3rdplasmidconc1to1/tea4s15w_0_002534.tif", path "C:/Analysis_from_Movie_for_RiboTrap_Dieter/Movie_Data_Lorenz/TPA-3rdplasmidconc1to1/tea4s15w_0_002535.tif", path "C:/Analysis_from_Movie_for_RiboTrap_Dieter/Movie_Data_Lorenz/TPA-3rdplasmidconc1to1/tea4s15w_0_002536.tif", path "C:/Analysis_from_Movie_for_RiboTrap_Dieter/Movie_Data_Lorenz/TPA-3rdplasmidconc1to1/tea4s15w_0_002537.tif", path "C:/Analysis_from_Movie_for_RiboTrap_Dieter/Movie_Data_Lorenz/TPA-3rdplasmidconc1to1/tea4s15w_0_002538.tif", path "C:/Analysis_from_Movie_for_RiboTrap_Dieter/Movie_Data_Lorenz/TPA-3rdplasmidconc1to1/tea4s15w_0_002539.tif", path "C:/Analysis_from_Movie_for_RiboTrap_Dieter/Movie_Data_Lorenz/TPA-3rdplasmidconc1to1/tea4s15w_0_002540.tif", path "C:/Analysis_from_Movie_for_RiboTrap_Dieter/Movie_Data_Lorenz/TPA-3rdplasmidconc1to1/tea4s15w_0_002541.tif", path "C:/Analysis_from_Movie_for_RiboTrap_Dieter/Movie_Data_Lorenz/TPA-3rdplasmidconc1to1/tea4s15w_0_002542.tif", path "C:/Analysis_from_Movie_for_RiboTrap_Dieter/Movie_Data_Lorenz/TPA-3rdplasmidconc1to1/tea4s15w_0_002543.tif", path "C:/Analysis_from_Movie_for_RiboTrap_Dieter/Movie_Data_Lorenz/TPA-3rdplasmidconc1to1/tea4s15w_0_002544.tif", path "C:/Analysis_from_Movie_for_RiboTrap_Dieter/Movie_Data_Lorenz/TPA-3rdplasmidconc1to1/tea4s15w_0_002545.tif", path "C:/Analysis_from_Movie_for_RiboTrap_Dieter/Movie_Data_Lorenz/TPA-3rdplasmidconc1to1/tea4s15w_0_002546.tif", path "C:/Analysis_from_Movie_for_RiboTrap_Dieter/Movie_Data_Lorenz/TPA-3rdplasmidconc1to1/tea4s15w_0_002547.tif", path "C:/Analysis_from_Movie_for_RiboTrap_Dieter/Movie_Data_Lorenz/TPA-3rdplasmidconc1to1/tea4s15w_0_002548.tif", path "C:/Analysis_from_Movie_for_RiboTrap_Dieter/Movie_Data_Lorenz/TPA-3rdplasmidconc1to1/tea4s15w_0_002549.tif", path "C:/Analysis_from_Movie_for_RiboTrap_Dieter/Movie_Data_Lorenz/TPA-3rdplasmidconc1to1/tea4s15w_0_002550.tif", path "C:/Analysis_from_Movie_for_RiboTrap_Dieter/Movie_Data_Lorenz/TPA-3rdplasmidconc1to1/tea4s15w_0_002551.tif", path "C:/Analysis_from_Movie_for_RiboTrap_Dieter/Movie_Data_Lorenz/TPA-3rdplasmidconc1to1/tea4s15w_0_002552.tif", path "C:/Analysis_from_Movie_for_RiboTrap_Dieter/Movie_Data_Lorenz/TPA-3rdplasmidconc1to1/tea4s15w_0_002553.tif", path "C:/Analysis_from_Movie_for_RiboTrap_Dieter/Movie_Data_Lorenz/TPA-3rdplasmidconc1to1/tea4s15w_0_002554.tif", path "C:/Analysis_from_Movie_for_RiboTrap_Dieter/Movie_Data_Lorenz/TPA-3rdplasmidconc1to1/tea4s15w_0_002555.tif", path "C:/Analysis_from_Movie_for_RiboTrap_Dieter/Movie_Data_Lorenz/TPA-3rdplasmidconc1to1/tea4s15w_0_002556.tif", path "C:/Analysis_from_Movie_for_RiboTrap_Dieter/Movie_Data_Lorenz/TPA-3rdplasmidconc1to1/tea4s15w_0_002557.tif", path "C:/Analysis_from_Movie_for_RiboTrap_Dieter/Movie_Data_Lorenz/TPA-3rdplasmidconc1to1/tea4s15w_0_002558.tif", path "C:/Analysis_from_Movie_for_RiboTrap_Dieter/Movie_Data_Lorenz/TPA-3rdplasmidconc1to1/tea4s15w_0_002559.tif", path "C:/Analysis_from_Movie_for_RiboTrap_Dieter/Movie_Data_Lorenz/TPA-3rdplasmidconc1to1/tea4s15w_0_002560.tif", path "C:/Analysis_from_Movie_for_RiboTrap_Dieter/Movie_Data_Lorenz/TPA-3rdplasmidconc1to1/tea4s15w_0_002561.tif", path "C:/Analysis_from_Movie_for_RiboTrap_Dieter/Movie_Data_Lorenz/TPA-3rdplasmidconc1to1/tea4s15w_0_002562.tif", path "C:/Analysis_from_Movie_for_RiboTrap_Dieter/Movie_Data_Lorenz/TPA-3rdplasmidconc1to1/tea4s15w_0_002563.tif", path "C:/Analysis_from_Movie_for_RiboTrap_Dieter/Movie_Data_Lorenz/TPA-3rdplasmidconc1to1/tea4s15w_0_002564.tif", path "C:/Analysis_from_Movie_for_RiboTrap_Dieter/Movie_Data_Lorenz/TPA-3rdplasmidconc1to1/tea4s15w_0_002565.tif", path "C:/Analysis_from_Movie_for_RiboTrap_Dieter/Movie_Data_Lorenz/TPA-3rdplasmidconc1to1/tea4s15w_0_002566.tif", path "C:/Analysis_from_Movie_for_RiboTrap_Dieter/Movie_Data_Lorenz/TPA-3rdplasmidconc1to1/tea4s15w_0_002567.tif", path "C:/Analysis_from_Movie_for_RiboTrap_Dieter/Movie_Data_Lorenz/TPA-3rdplasmidconc1to1/tea4s15w_0_002568.tif", path "C:/Analysis_from_Movie_for_RiboTrap_Dieter/Movie_Data_Lorenz/TPA-3rdplasmidconc1to1/tea4s15w_0_002569.tif", path "C:/Analysis_from_Movie_for_RiboTrap_Dieter/Movie_Data_Lorenz/TPA-3rdplasmidconc1to1/tea4s15w_0_002570.tif", path "C:/Analysis_from_Movie_for_RiboTrap_Dieter/Movie_Data_Lorenz/TPA-3rdplasmidconc1to1/tea4s15w_0_002571.tif", path "C:/Analysis_from_Movie_for_RiboTrap_Dieter/Movie_Data_Lorenz/TPA-3rdplasmidconc1to1/tea4s15w_0_002572.tif", path "C:/Analysis_from_Movie_for_RiboTrap_Dieter/Movie_Data_Lorenz/TPA-3rdplasmidconc1to1/tea4s15w_0_002573.tif", path "C:/Analysis_from_Movie_for_RiboTrap_Dieter/Movie_Data_Lorenz/TPA-3rdplasmidconc1to1/tea4s15w_0_002574.tif", path "C:/Analysis_from_Movie_for_RiboTrap_Dieter/Movie_Data_Lorenz/TPA-3rdplasmidconc1to1/tea4s15w_0_002575.tif", path "C:/Analysis_from_Movie_for_RiboTrap_Dieter/Movie_Data_Lorenz/TPA-3rdplasmidconc1to1/tea4s15w_0_002576.tif", path "C:/Analysis_from_Movie_for_RiboTrap_Dieter/Movie_Data_Lorenz/TPA-3rdplasmidconc1to1/tea4s15w_0_002577.tif", path "C:/Analysis_from_Movie_for_RiboTrap_Dieter/Movie_Data_Lorenz/TPA-3rdplasmidconc1to1/tea4s15w_0_002578.tif", path "C:/Analysis_from_Movie_for_RiboTrap_Dieter/Movie_Data_Lorenz/TPA-3rdplasmidconc1to1/tea4s15w_0_002579.tif", path "C:/Analysis_from_Movie_for_RiboTrap_Dieter/Movie_Data_Lorenz/TPA-3rdplasmidconc1to1/tea4s15w_0_002580.tif", path "C:/Analysis_from_Movie_for_RiboTrap_Dieter/Movie_Data_Lorenz/TPA-3rdplasmidconc1to1/tea4s15w_0_002581.tif", path "C:/Analysis_from_Movie_for_RiboTrap_Dieter/Movie_Data_Lorenz/TPA-3rdplasmidconc1to1/tea4s15w_0_002582.tif", path "C:/Analysis_from_Movie_for_RiboTrap_Dieter/Movie_Data_Lorenz/TPA-3rdplasmidconc1to1/tea4s15w_0_002583.tif", path "C:/Analysis_from_Movie_for_RiboTrap_Dieter/Movie_Data_Lorenz/TPA-3rdplasmidconc1to1/tea4s15w_0_002584.tif", path "C:/Analysis_from_Movie_for_RiboTrap_Dieter/Movie_Data_Lorenz/TPA-3rdplasmidconc1to1/tea4s15w_0_002585.tif", path "C:/Analysis_from_Movie_for_RiboTrap_Dieter/Movie_Data_Lorenz/TPA-3rdplasmidconc1to1/tea4s15w_0_002586.tif", path "C:/Analysis_from_Movie_for_RiboTrap_Dieter/Movie_Data_Lorenz/TPA-3rdplasmidconc1to1/tea4s15w_0_002587.tif", path "C:/Analysis_from_Movie_for_RiboTrap_Dieter/Movie_Data_Lorenz/TPA-3rdplasmidconc1to1/tea4s15w_0_002588.tif", path "C:/Analysis_from_Movie_for_RiboTrap_Dieter/Movie_Data_Lorenz/TPA-3rdplasmidconc1to1/tea4s15w_0_002589.tif", path "C:/Analysis_from_Movie_for_RiboTrap_Dieter/Movie_Data_Lorenz/TPA-3rdplasmidconc1to1/tea4s15w_0_002590.tif", path "C:/Analysis_from_Movie_for_RiboTrap_Dieter/Movie_Data_Lorenz/TPA-3rdplasmidconc1to1/tea4s15w_0_002591.tif", path "C:/Analysis_from_Movie_for_RiboTrap_Dieter/Movie_Data_Lorenz/TPA-3rdplasmidconc1to1/tea4s15w_0_002592.tif", path "C:/Analysis_from_Movie_for_RiboTrap_Dieter/Movie_Data_Lorenz/TPA-3rdplasmidconc1to1/tea4s15w_0_002593.tif", path "C:/Analysis_from_Movie_for_RiboTrap_Dieter/Movie_Data_Lorenz/TPA-3rdplasmidconc1to1/tea4s15w_0_002594.tif", path "C:/Analysis_from_Movie_for_RiboTrap_Dieter/Movie_Data_Lorenz/TPA-3rdplasmidconc1to1/tea4s15w_0_002595.tif", path "C:/Analysis_from_Movie_for_RiboTrap_Dieter/Movie_Data_Lorenz/TPA-3rdplasmidconc1to1/tea4s15w_0_002596.tif", path "C:/Analysis_from_Movie_for_RiboTrap_Dieter/Movie_Data_Lorenz/TPA-3rdplasmidconc1to1/tea4s15w_0_002597.tif", path "C:/Analysis_from_Movie_for_RiboTrap_Dieter/Movie_Data_Lorenz/TPA-3rdplasmidconc1to1/tea4s15w_0_002598.tif", path "C:/Analysis_from_Movie_for_RiboTrap_Dieter/Movie_Data_Lorenz/TPA-3rdplasmidconc1to1/tea4s15w_0_002599.tif", path "C:/Analysis_from_Movie_for_RiboTrap_Dieter/Movie_Data_Lorenz/TPA-3rdplasmidconc1to1/tea4s15w_0_002600.tif", path "C:/Analysis_from_Movie_for_RiboTrap_Dieter/Movie_Data_Lorenz/TPA-3rdplasmidconc1to1/tea4s15w_0_002601.tif", path "C:/Analysis_from_Movie_for_RiboTrap_Dieter/Movie_Data_Lorenz/TPA-3rdplasmidconc1to1/tea4s15w_0_002602.tif", path "C:/Analysis_from_Movie_for_RiboTrap_Dieter/Movie_Data_Lorenz/TPA-3rdplasmidconc1to1/tea4s15w_0_002603.tif", path "C:/Analysis_from_Movie_for_RiboTrap_Dieter/Movie_Data_Lorenz/TPA-3rdplasmidconc1to1/tea4s15w_0_002604.tif", path "C:/Analysis_from_Movie_for_RiboTrap_Dieter/Movie_Data_Lorenz/TPA-3rdplasmidconc1to1/tea4s15w_0_002605.tif", path "C:/Analysis_from_Movie_for_RiboTrap_Dieter/Movie_Data_Lorenz/TPA-3rdplasmidconc1to1/tea4s15w_0_002606.tif", path "C:/Analysis_from_Movie_for_RiboTrap_Dieter/Movie_Data_Lorenz/TPA-3rdplasmidconc1to1/tea4s15w_0_002607.tif", path "C:/Analysis_from_Movie_for_RiboTrap_Dieter/Movie_Data_Lorenz/TPA-3rdplasmidconc1to1/tea4s15w_0_002608.tif", path "C:/Analysis_from_Movie_for_RiboTrap_Dieter/Movie_Data_Lorenz/TPA-3rdplasmidconc1to1/tea4s15w_0_002609.tif", path "C:/Analysis_from_Movie_for_RiboTrap_Dieter/Movie_Data_Lorenz/TPA-3rdplasmidconc1to1/tea4s15w_0_002610.tif", path "C:/Analysis_from_Movie_for_RiboTrap_Dieter/Movie_Data_Lorenz/TPA-3rdplasmidconc1to1/tea4s15w_0_002611.tif", path "C:/Analysis_from_Movie_for_RiboTrap_Dieter/Movie_Data_Lorenz/TPA-3rdplasmidconc1to1/tea4s15w_0_002612.tif", path "C:/Analysis_from_Movie_for_RiboTrap_Dieter/Movie_Data_Lorenz/TPA-3rdplasmidconc1to1/tea4s15w_0_002613.tif", path "C:/Analysis_from_Movie_for_RiboTrap_Dieter/Movie_Data_Lorenz/TPA-3rdplasmidconc1to1/tea4s15w_0_002614.tif", path "C:/Analysis_from_Movie_for_RiboTrap_Dieter/Movie_Data_Lorenz/TPA-3rdplasmidconc1to1/tea4s15w_0_002615.tif", path "C:/Analysis_from_Movie_for_RiboTrap_Dieter/Movie_Data_Lorenz/TPA-3rdplasmidconc1to1/tea4s15w_0_002616.tif", path "C:/Analysis_from_Movie_for_RiboTrap_Dieter/Movie_Data_Lorenz/TPA-3rdplasmidconc1to1/tea4s15w_0_002617.tif", path "C:/Analysis_from_Movie_for_RiboTrap_Dieter/Movie_Data_Lorenz/TPA-3rdplasmidconc1to1/tea4s15w_0_002618.tif", path "C:/Analysis_from_Movie_for_RiboTrap_Dieter/Movie_Data_Lorenz/TPA-3rdplasmidconc1to1/tea4s15w_0_002619.tif", path "C:/Analysis_from_Movie_for_RiboTrap_Dieter/Movie_Data_Lorenz/TPA-3rdplasmidconc1to1/tea4s15w_0_002620.tif", path "C:/Analysis_from_Movie_for_RiboTrap_Dieter/Movie_Data_Lorenz/TPA-3rdplasmidconc1to1/tea4s15w_0_002621.tif", path "C:/Analysis_from_Movie_for_RiboTrap_Dieter/Movie_Data_Lorenz/TPA-3rdplasmidconc1to1/tea4s15w_0_002622.tif", path "C:/Analysis_from_Movie_for_RiboTrap_Dieter/Movie_Data_Lorenz/TPA-3rdplasmidconc1to1/tea4s15w_0_002623.tif", path "C:/Analysis_from_Movie_for_RiboTrap_Dieter/Movie_Data_Lorenz/TPA-3rdplasmidconc1to1/tea4s15w_0_002624.tif", path "C:/Analysis_from_Movie_for_RiboTrap_Dieter/Movie_Data_Lorenz/TPA-3rdplasmidconc1to1/tea4s15w_0_002625.tif", path "C:/Analysis_from_Movie_for_RiboTrap_Dieter/Movie_Data_Lorenz/TPA-3rdplasmidconc1to1/tea4s15w_0_002626.tif", path "C:/Analysis_from_Movie_for_RiboTrap_Dieter/Movie_Data_Lorenz/TPA-3rdplasmidconc1to1/tea4s15w_0_002627.tif", path "C:/Analysis_from_Movie_for_RiboTrap_Dieter/Movie_Data_Lorenz/TPA-3rdplasmidconc1to1/tea4s15w_0_002628.tif", path "C:/Analysis_from_Movie_for_RiboTrap_Dieter/Movie_Data_Lorenz/TPA-3rdplasmidconc1to1/tea4s15w_0_002629.tif", path "C:/Analysis_from_Movie_for_RiboTrap_Dieter/Movie_Data_Lorenz/TPA-3rdplasmidconc1to1/tea4s15w_0_002630.tif", path "C:/Analysis_from_Movie_for_RiboTrap_Dieter/Movie_Data_Lorenz/TPA-3rdplasmidconc1to1/tea4s15w_0_002631.tif", path "C:/Analysis_from_Movie_for_RiboTrap_Dieter/Movie_Data_Lorenz/TPA-3rdplasmidconc1to1/tea4s15w_0_002632.tif", path "C:/Analysis_from_Movie_for_RiboTrap_Dieter/Movie_Data_Lorenz/TPA-3rdplasmidconc1to1/tea4s15w_0_002633.tif", path "C:/Analysis_from_Movie_for_RiboTrap_Dieter/Movie_Data_Lorenz/TPA-3rdplasmidconc1to1/tea4s15w_0_002634.tif", path "C:/Analysis_from_Movie_for_RiboTrap_Dieter/Movie_Data_Lorenz/TPA-3rdplasmidconc1to1/tea4s15w_0_002635.tif", path "C:/Analysis_from_Movie_for_RiboTrap_Dieter/Movie_Data_Lorenz/TPA-3rdplasmidconc1to1/tea4s15w_0_002636.tif", path "C:/Analysis_from_Movie_for_RiboTrap_Dieter/Movie_Data_Lorenz/TPA-3rdplasmidconc1to1/tea4s15w_0_002637.tif", path "C:/Analysis_from_Movie_for_RiboTrap_Dieter/Movie_Data_Lorenz/TPA-3rdplasmidconc1to1/tea4s15w_0_002638.tif", path "C:/Analysis_from_Movie_for_RiboTrap_Dieter/Movie_Data_Lorenz/TPA-3rdplasmidconc1to1/tea4s15w_0_002639.tif", path "C:/Analysis_from_Movie_for_RiboTrap_Dieter/Movie_Data_Lorenz/TPA-3rdplasmidconc1to1/tea4s15w_0_002640.tif", path "C:/Analysis_from_Movie_for_RiboTrap_Dieter/Movie_Data_Lorenz/TPA-3rdplasmidconc1to1/tea4s15w_0_002641.tif", path "C:/Analysis_from_Movie_for_RiboTrap_Dieter/Movie_Data_Lorenz/TPA-3rdplasmidconc1to1/tea4s15w_0_002642.tif", path "C:/Analysis_from_Movie_for_RiboTrap_Dieter/Movie_Data_Lorenz/TPA-3rdplasmidconc1to1/tea4s15w_0_002643.tif", path "C:/Analysis_from_Movie_for_RiboTrap_Dieter/Movie_Data_Lorenz/TPA-3rdplasmidconc1to1/tea4s15w_0_002644.tif", path "C:/Analysis_from_Movie_for_RiboTrap_Dieter/Movie_Data_Lorenz/TPA-3rdplasmidconc1to1/tea4s15w_0_002645.tif", path "C:/Analysis_from_Movie_for_RiboTrap_Dieter/Movie_Data_Lorenz/TPA-3rdplasmidconc1to1/tea4s15w_0_002646.tif", path "C:/Analysis_from_Movie_for_RiboTrap_Dieter/Movie_Data_Lorenz/TPA-3rdplasmidconc1to1/tea4s15w_0_002647.tif", path "C:/Analysis_from_Movie_for_RiboTrap_Dieter/Movie_Data_Lorenz/TPA-3rdplasmidconc1to1/tea4s15w_0_002648.tif", path "C:/Analysis_from_Movie_for_RiboTrap_Dieter/Movie_Data_Lorenz/TPA-3rdplasmidconc1to1/tea4s15w_0_002649.tif", path "C:/Analysis_from_Movie_for_RiboTrap_Dieter/Movie_Data_Lorenz/TPA-3rdplasmidconc1to1/tea4s15w_0_002650.tif", path "C:/Analysis_from_Movie_for_RiboTrap_Dieter/Movie_Data_Lorenz/TPA-3rdplasmidconc1to1/tea4s15w_0_002651.tif", path "C:/Analysis_from_Movie_for_RiboTrap_Dieter/Movie_Data_Lorenz/TPA-3rdplasmidconc1to1/tea4s15w_0_002652.tif", path "C:/Analysis_from_Movie_for_RiboTrap_Dieter/Movie_Data_Lorenz/TPA-3rdplasmidconc1to1/tea4s15w_0_002653.tif", path "C:/Analysis_from_Movie_for_RiboTrap_Dieter/Movie_Data_Lorenz/TPA-3rdplasmidconc1to1/tea4s15w_0_002654.tif", path "C:/Analysis_from_Movie_for_RiboTrap_Dieter/Movie_Data_Lorenz/TPA-3rdplasmidconc1to1/tea4s15w_0_002655.tif", path "C:/Analysis_from_Movie_for_RiboTrap_Dieter/Movie_Data_Lorenz/TPA-3rdplasmidconc1to1/tea4s15w_0_002656.tif", path "C:/Analysis_from_Movie_for_RiboTrap_Dieter/Movie_Data_Lorenz/TPA-3rdplasmidconc1to1/tea4s15w_0_002657.tif", path "C:/Analysis_from_Movie_for_RiboTrap_Dieter/Movie_Data_Lorenz/TPA-3rdplasmidconc1to1/tea4s15w_0_002658.tif", path "C:/Analysis_from_Movie_for_RiboTrap_Dieter/Movie_Data_Lorenz/TPA-3rdplasmidconc1to1/tea4s15w_0_002659.tif", path "C:/Analysis_from_Movie_for_RiboTrap_Dieter/Movie_Data_Lorenz/TPA-3rdplasmidconc1to1/tea4s15w_0_002660.tif", path "C:/Analysis_from_Movie_for_RiboTrap_Dieter/Movie_Data_Lorenz/TPA-3rdplasmidconc1to1/tea4s15w_0_002661.tif", path "C:/Analysis_from_Movie_for_RiboTrap_Dieter/Movie_Data_Lorenz/TPA-3rdplasmidconc1to1/tea4s15w_0_002662.tif", path "C:/Analysis_from_Movie_for_RiboTrap_Dieter/Movie_Data_Lorenz/TPA-3rdplasmidconc1to1/tea4s15w_0_002663.tif", path "C:/Analysis_from_Movie_for_RiboTrap_Dieter/Movie_Data_Lorenz/TPA-3rdplasmidconc1to1/tea4s15w_0_002664.tif", path "C:/Analysis_from_Movie_for_RiboTrap_Dieter/Movie_Data_Lorenz/TPA-3rdplasmidconc1to1/tea4s15w_0_002665.tif", path "C:/Analysis_from_Movie_for_RiboTrap_Dieter/Movie_Data_Lorenz/TPA-3rdplasmidconc1to1/tea4s15w_0_002666.tif", path "C:/Analysis_from_Movie_for_RiboTrap_Dieter/Movie_Data_Lorenz/TPA-3rdplasmidconc1to1/tea4s15w_0_002667.tif", path "C:/Analysis_from_Movie_for_RiboTrap_Dieter/Movie_Data_Lorenz/TPA-3rdplasmidconc1to1/tea4s15w_0_002668.tif", path "C:/Analysis_from_Movie_for_RiboTrap_Dieter/Movie_Data_Lorenz/TPA-3rdplasmidconc1to1/tea4s15w_0_002669.tif", path "C:/Analysis_from_Movie_for_RiboTrap_Dieter/Movie_Data_Lorenz/TPA-3rdplasmidconc1to1/tea4s15w_0_002670.tif", path "C:/Analysis_from_Movie_for_RiboTrap_Dieter/Movie_Data_Lorenz/TPA-3rdplasmidconc1to1/tea4s15w_0_002671.tif", path "C:/Analysis_from_Movie_for_RiboTrap_Dieter/Movie_Data_Lorenz/TPA-3rdplasmidconc1to1/tea4s15w_0_002672.tif", path "C:/Analysis_from_Movie_for_RiboTrap_Dieter/Movie_Data_Lorenz/TPA-3rdplasmidconc1to1/tea4s15w_0_002673.tif", path "C:/Analysis_from_Movie_for_RiboTrap_Dieter/Movie_Data_Lorenz/TPA-3rdplasmidconc1to1/tea4s15w_0_002674.tif", path "C:/Analysis_from_Movie_for_RiboTrap_Dieter/Movie_Data_Lorenz/TPA-3rdplasmidconc1to1/tea4s15w_0_002675.tif", path "C:/Analysis_from_Movie_for_RiboTrap_Dieter/Movie_Data_Lorenz/TPA-3rdplasmidconc1to1/tea4s15w_0_002676.tif", path "C:/Analysis_from_Movie_for_RiboTrap_Dieter/Movie_Data_Lorenz/TPA-3rdplasmidconc1to1/tea4s15w_0_002677.tif", path "C:/Analysis_from_Movie_for_RiboTrap_Dieter/Movie_Data_Lorenz/TPA-3rdplasmidconc1to1/tea4s15w_0_002678.tif", path "C:/Analysis_from_Movie_for_RiboTrap_Dieter/Movie_Data_Lorenz/TPA-3rdplasmidconc1to1/tea4s15w_0_002679.tif", path "C:/Analysis_from_Movie_for_RiboTrap_Dieter/Movie_Data_Lorenz/TPA-3rdplasmidconc1to1/tea4s15w_0_002680.tif", path "C:/Analysis_from_Movie_for_RiboTrap_Dieter/Movie_Data_Lorenz/TPA-3rdplasmidconc1to1/tea4s15w_0_002681.tif", path "C:/Analysis_from_Movie_for_RiboTrap_Dieter/Movie_Data_Lorenz/TPA-3rdplasmidconc1to1/tea4s15w_0_002682.tif", path "C:/Analysis_from_Movie_for_RiboTrap_Dieter/Movie_Data_Lorenz/TPA-3rdplasmidconc1to1/tea4s15w_0_002683.tif", path "C:/Analysis_from_Movie_for_RiboTrap_Dieter/Movie_Data_Lorenz/TPA-3rdplasmidconc1to1/tea4s15w_0_002684.tif", path "C:/Analysis_from_Movie_for_RiboTrap_Dieter/Movie_Data_Lorenz/TPA-3rdplasmidconc1to1/tea4s15w_0_002685.tif", path "C:/Analysis_from_Movie_for_RiboTrap_Dieter/Movie_Data_Lorenz/TPA-3rdplasmidconc1to1/tea4s15w_0_002686.tif", path "C:/Analysis_from_Movie_for_RiboTrap_Dieter/Movie_Data_Lorenz/TPA-3rdplasmidconc1to1/tea4s15w_0_002687.tif", path "C:/Analysis_from_Movie_for_RiboTrap_Dieter/Movie_Data_Lorenz/TPA-3rdplasmidconc1to1/tea4s15w_0_002688.tif", path "C:/Analysis_from_Movie_for_RiboTrap_Dieter/Movie_Data_Lorenz/TPA-3rdplasmidconc1to1/tea4s15w_0_002689.tif", path "C:/Analysis_from_Movie_for_RiboTrap_Dieter/Movie_Data_Lorenz/TPA-3rdplasmidconc1to1/tea4s15w_0_002690.tif", path "C:/Analysis_from_Movie_for_RiboTrap_Dieter/Movie_Data_Lorenz/TPA-3rdplasmidconc1to1/tea4s15w_0_002691.tif", path "C:/Analysis_from_Movie_for_RiboTrap_Dieter/Movie_Data_Lorenz/TPA-3rdplasmidconc1to1/tea4s15w_0_002692.tif", path "C:/Analysis_from_Movie_for_RiboTrap_Dieter/Movie_Data_Lorenz/TPA-3rdplasmidconc1to1/tea4s15w_0_002693.tif", path "C:/Analysis_from_Movie_for_RiboTrap_Dieter/Movie_Data_Lorenz/TPA-3rdplasmidconc1to1/tea4s15w_0_002694.tif", path "C:/Analysis_from_Movie_for_RiboTrap_Dieter/Movie_Data_Lorenz/TPA-3rdplasmidconc1to1/tea4s15w_0_002695.tif", path "C:/Analysis_from_Movie_for_RiboTrap_Dieter/Movie_Data_Lorenz/TPA-3rdplasmidconc1to1/tea4s15w_0_002696.tif", path "C:/Analysis_from_Movie_for_RiboTrap_Dieter/Movie_Data_Lorenz/TPA-3rdplasmidconc1to1/tea4s15w_0_002697.tif", path "C:/Analysis_from_Movie_for_RiboTrap_Dieter/Movie_Data_Lorenz/TPA-3rdplasmidconc1to1/tea4s15w_0_002698.tif", path "C:/Analysis_from_Movie_for_RiboTrap_Dieter/Movie_Data_Lorenz/TPA-3rdplasmidconc1to1/tea4s15w_0_002699.tif", path "C:/Analysis_from_Movie_for_RiboTrap_Dieter/Movie_Data_Lorenz/TPA-3rdplasmidconc1to1/tea4s15w_0_002700.tif", path "C:/Analysis_from_Movie_for_RiboTrap_Dieter/Movie_Data_Lorenz/TPA-3rdplasmidconc1to1/tea4s15w_0_002701.tif", path "C:/Analysis_from_Movie_for_RiboTrap_Dieter/Movie_Data_Lorenz/TPA-3rdplasmidconc1to1/tea4s15w_0_002702.tif", path "C:/Analysis_from_Movie_for_RiboTrap_Dieter/Movie_Data_Lorenz/TPA-3rdplasmidconc1to1/tea4s15w_0_002703.tif", path "C:/Analysis_from_Movie_for_RiboTrap_Dieter/Movie_Data_Lorenz/TPA-3rdplasmidconc1to1/tea4s15w_0_002704.tif", path "C:/Analysis_from_Movie_for_RiboTrap_Dieter/Movie_Data_Lorenz/TPA-3rdplasmidconc1to1/tea4s15w_0_002705.tif", path "C:/Analysis_from_Movie_for_RiboTrap_Dieter/Movie_Data_Lorenz/TPA-3rdplasmidconc1to1/tea4s15w_0_002706.tif", path "C:/Analysis_from_Movie_for_RiboTrap_Dieter/Movie_Data_Lorenz/TPA-3rdplasmidconc1to1/tea4s15w_0_002707.tif", path "C:/Analysis_from_Movie_for_RiboTrap_Dieter/Movie_Data_Lorenz/TPA-3rdplasmidconc1to1/tea4s15w_0_002708.tif", path "C:/Analysis_from_Movie_for_RiboTrap_Dieter/Movie_Data_Lorenz/TPA-3rdplasmidconc1to1/tea4s15w_0_002709.tif", path "C:/Analysis_from_Movie_for_RiboTrap_Dieter/Movie_Data_Lorenz/TPA-3rdplasmidconc1to1/tea4s15w_0_002710.tif", path "C:/Analysis_from_Movie_for_RiboTrap_Dieter/Movie_Data_Lorenz/TPA-3rdplasmidconc1to1/tea4s15w_0_002711.tif", path "C:/Analysis_from_Movie_for_RiboTrap_Dieter/Movie_Data_Lorenz/TPA-3rdplasmidconc1to1/tea4s15w_0_002712.tif", path "C:/Analysis_from_Movie_for_RiboTrap_Dieter/Movie_Data_Lorenz/TPA-3rdplasmidconc1to1/tea4s15w_0_002713.tif", path "C:/Analysis_from_Movie_for_RiboTrap_Dieter/Movie_Data_Lorenz/TPA-3rdplasmidconc1to1/tea4s15w_0_002714.tif", path "C:/Analysis_from_Movie_for_RiboTrap_Dieter/Movie_Data_Lorenz/TPA-3rdplasmidconc1to1/tea4s15w_0_002715.tif", path "C:/Analysis_from_Movie_for_RiboTrap_Dieter/Movie_Data_Lorenz/TPA-3rdplasmidconc1to1/tea4s15w_0_002716.tif", path "C:/Analysis_from_Movie_for_RiboTrap_Dieter/Movie_Data_Lorenz/TPA-3rdplasmidconc1to1/tea4s15w_0_002717.tif", path "C:/Analysis_from_Movie_for_RiboTrap_Dieter/Movie_Data_Lorenz/TPA-3rdplasmidconc1to1/tea4s15w_0_002718.tif", path "C:/Analysis_from_Movie_for_RiboTrap_Dieter/Movie_Data_Lorenz/TPA-3rdplasmidconc1to1/tea4s15w_0_002719.tif", path "C:/Analysis_from_Movie_for_RiboTrap_Dieter/Movie_Data_Lorenz/TPA-3rdplasmidconc1to1/tea4s15w_0_002720.tif", path "C:/Analysis_from_Movie_for_RiboTrap_Dieter/Movie_Data_Lorenz/TPA-3rdplasmidconc1to1/tea4s15w_0_002721.tif", path "C:/Analysis_from_Movie_for_RiboTrap_Dieter/Movie_Data_Lorenz/TPA-3rdplasmidconc1to1/tea4s15w_0_002722.tif", path "C:/Analysis_from_Movie_for_RiboTrap_Dieter/Movie_Data_Lorenz/TPA-3rdplasmidconc1to1/tea4s15w_0_002723.tif", path "C:/Analysis_from_Movie_for_RiboTrap_Dieter/Movie_Data_Lorenz/TPA-3rdplasmidconc1to1/tea4s15w_0_002724.tif", path "C:/Analysis_from_Movie_for_RiboTrap_Dieter/Movie_Data_Lorenz/TPA-3rdplasmidconc1to1/tea4s15w_0_002725.tif", path "C:/Analysis_from_Movie_for_RiboTrap_Dieter/Movie_Data_Lorenz/TPA-3rdplasmidconc1to1/tea4s15w_0_002726.tif", path "C:/Analysis_from_Movie_for_RiboTrap_Dieter/Movie_Data_Lorenz/TPA-3rdplasmidconc1to1/tea4s15w_0_002727.tif", path "C:/Analysis_from_Movie_for_RiboTrap_Dieter/Movie_Data_Lorenz/TPA-3rdplasmidconc1to1/tea4s15w_0_002728.tif", path "C:/Analysis_from_Movie_for_RiboTrap_Dieter/Movie_Data_Lorenz/TPA-3rdplasmidconc1to1/tea4s15w_0_002729.tif", path "C:/Analysis_from_Movie_for_RiboTrap_Dieter/Movie_Data_Lorenz/TPA-3rdplasmidconc1to1/tea4s15w_0_002730.tif", path "C:/Analysis_from_Movie_for_RiboTrap_Dieter/Movie_Data_Lorenz/TPA-3rdplasmidconc1to1/tea4s15w_0_002731.tif", path "C:/Analysis_from_Movie_for_RiboTrap_Dieter/Movie_Data_Lorenz/TPA-3rdplasmidconc1to1/tea4s15w_0_002732.tif", path "C:/Analysis_from_Movie_for_RiboTrap_Dieter/Movie_Data_Lorenz/TPA-3rdplasmidconc1to1/tea4s15w_0_002733.tif", path "C:/Analysis_from_Movie_for_RiboTrap_Dieter/Movie_Data_Lorenz/TPA-3rdplasmidconc1to1/tea4s15w_0_002734.tif", path "C:/Analysis_from_Movie_for_RiboTrap_Dieter/Movie_Data_Lorenz/TPA-3rdplasmidconc1to1/tea4s15w_0_002735.tif", path "C:/Analysis_from_Movie_for_RiboTrap_Dieter/Movie_Data_Lorenz/TPA-3rdplasmidconc1to1/tea4s15w_0_002736.tif", path "C:/Analysis_from_Movie_for_RiboTrap_Dieter/Movie_Data_Lorenz/TPA-3rdplasmidconc1to1/tea4s15w_0_002737.tif", path "C:/Analysis_from_Movie_for_RiboTrap_Dieter/Movie_Data_Lorenz/TPA-3rdplasmidconc1to1/tea4s15w_0_002738.tif", path "C:/Analysis_from_Movie_for_RiboTrap_Dieter/Movie_Data_Lorenz/TPA-3rdplasmidconc1to1/tea4s15w_0_002739.tif", path "C:/Analysis_from_Movie_for_RiboTrap_Dieter/Movie_Data_Lorenz/TPA-3rdplasmidconc1to1/tea4s15w_0_002740.tif", path "C:/Analysis_from_Movie_for_RiboTrap_Dieter/Movie_Data_Lorenz/TPA-3rdplasmidconc1to1/tea4s15w_0_002741.tif", path "C:/Analysis_from_Movie_for_RiboTrap_Dieter/Movie_Data_Lorenz/TPA-3rdplasmidconc1to1/tea4s15w_0_002742.tif", path "C:/Analysis_from_Movie_for_RiboTrap_Dieter/Movie_Data_Lorenz/TPA-3rdplasmidconc1to1/tea4s15w_0_002743.tif", path "C:/Analysis_from_Movie_for_RiboTrap_Dieter/Movie_Data_Lorenz/TPA-3rdplasmidconc1to1/tea4s15w_0_002744.tif", path "C:/Analysis_from_Movie_for_RiboTrap_Dieter/Movie_Data_Lorenz/TPA-3rdplasmidconc1to1/tea4s15w_0_002745.tif", path "C:/Analysis_from_Movie_for_RiboTrap_Dieter/Movie_Data_Lorenz/TPA-3rdplasmidconc1to1/tea4s15w_0_002746.tif", path "C:/Analysis_from_Movie_for_RiboTrap_Dieter/Movie_Data_Lorenz/TPA-3rdplasmidconc1to1/tea4s15w_0_002747.tif", path "C:/Analysis_from_Movie_for_RiboTrap_Dieter/Movie_Data_Lorenz/TPA-3rdplasmidconc1to1/tea4s15w_0_002748.tif", path "C:/Analysis_from_Movie_for_RiboTrap_Dieter/Movie_Data_Lorenz/TPA-3rdplasmidconc1to1/tea4s15w_0_002749.tif", path "C:/Analysis_from_Movie_for_RiboTrap_Dieter/Movie_Data_Lorenz/TPA-3rdplasmidconc1to1/tea4s15w_0_002750.tif", path "C:/Analysis_from_Movie_for_RiboTrap_Dieter/Movie_Data_Lorenz/TPA-3rdplasmidconc1to1/tea4s15w_0_002751.tif", path "C:/Analysis_from_Movie_for_RiboTrap_Dieter/Movie_Data_Lorenz/TPA-3rdplasmidconc1to1/tea4s15w_0_002752.tif", path "C:/Analysis_from_Movie_for_RiboTrap_Dieter/Movie_Data_Lorenz/TPA-3rdplasmidconc1to1/tea4s15w_0_002753.tif", path "C:/Analysis_from_Movie_for_RiboTrap_Dieter/Movie_Data_Lorenz/TPA-3rdplasmidconc1to1/tea4s15w_0_002754.tif", path "C:/Analysis_from_Movie_for_RiboTrap_Dieter/Movie_Data_Lorenz/TPA-3rdplasmidconc1to1/tea4s15w_0_002755.tif", path "C:/Analysis_from_Movie_for_RiboTrap_Dieter/Movie_Data_Lorenz/TPA-3rdplasmidconc1to1/tea4s15w_0_002756.tif", path "C:/Analysis_from_Movie_for_RiboTrap_Dieter/Movie_Data_Lorenz/TPA-3rdplasmidconc1to1/tea4s15w_0_002757.tif", path "C:/Analysis_from_Movie_for_RiboTrap_Dieter/Movie_Data_Lorenz/TPA-3rdplasmidconc1to1/tea4s15w_0_002758.tif", path "C:/Analysis_from_Movie_for_RiboTrap_Dieter/Movie_Data_Lorenz/TPA-3rdplasmidconc1to1/tea4s15w_0_002759.tif", path "C:/Analysis_from_Movie_for_RiboTrap_Dieter/Movie_Data_Lorenz/TPA-3rdplasmidconc1to1/tea4s15w_0_002760.tif", path "C:/Analysis_from_Movie_for_RiboTrap_Dieter/Movie_Data_Lorenz/TPA-3rdplasmidconc1to1/tea4s15w_0_002761.tif", path "C:/Analysis_from_Movie_for_RiboTrap_Dieter/Movie_Data_Lorenz/TPA-3rdplasmidconc1to1/tea4s15w_0_002762.tif", path "C:/Analysis_from_Movie_for_RiboTrap_Dieter/Movie_Data_Lorenz/TPA-3rdplasmidconc1to1/tea4s15w_0_002763.tif", path "C:/Analysis_from_Movie_for_RiboTrap_Dieter/Movie_Data_Lorenz/TPA-3rdplasmidconc1to1/tea4s15w_0_002764.tif", path "C:/Analysis_from_Movie_for_RiboTrap_Dieter/Movie_Data_Lorenz/TPA-3rdplasmidconc1to1/tea4s15w_0_002765.tif", path "C:/Analysis_from_Movie_for_RiboTrap_Dieter/Movie_Data_Lorenz/TPA-3rdplasmidconc1to1/tea4s15w_0_002766.tif", path "C:/Analysis_from_Movie_for_RiboTrap_Dieter/Movie_Data_Lorenz/TPA-3rdplasmidconc1to1/tea4s15w_0_002767.tif", path "C:/Analysis_from_Movie_for_RiboTrap_Dieter/Movie_Data_Lorenz/TPA-3rdplasmidconc1to1/tea4s15w_0_002768.tif", path "C:/Analysis_from_Movie_for_RiboTrap_Dieter/Movie_Data_Lorenz/TPA-3rdplasmidconc1to1/tea4s15w_0_002769.tif", path "C:/Analysis_from_Movie_for_RiboTrap_Dieter/Movie_Data_Lorenz/TPA-3rdplasmidconc1to1/tea4s15w_0_002770.tif", path "C:/Analysis_from_Movie_for_RiboTrap_Dieter/Movie_Data_Lorenz/TPA-3rdplasmidconc1to1/tea4s15w_0_002771.tif", path "C:/Analysis_from_Movie_for_RiboTrap_Dieter/Movie_Data_Lorenz/TPA-3rdplasmidconc1to1/tea4s15w_0_002772.tif", path "C:/Analysis_from_Movie_for_RiboTrap_Dieter/Movie_Data_Lorenz/TPA-3rdplasmidconc1to1/tea4s15w_0_002773.tif", path "C:/Analysis_from_Movie_for_RiboTrap_Dieter/Movie_Data_Lorenz/TPA-3rdplasmidconc1to1/tea4s15w_0_002774.tif", path "C:/Analysis_from_Movie_for_RiboTrap_Dieter/Movie_Data_Lorenz/TPA-3rdplasmidconc1to1/tea4s15w_0_002775.tif", path "C:/Analysis_from_Movie_for_RiboTrap_Dieter/Movie_Data_Lorenz/TPA-3rdplasmidconc1to1/tea4s15w_0_002776.tif", path "C:/Analysis_from_Movie_for_RiboTrap_Dieter/Movie_Data_Lorenz/TPA-3rdplasmidconc1to1/tea4s15w_0_002777.tif", path "C:/Analysis_from_Movie_for_RiboTrap_Dieter/Movie_Data_Lorenz/TPA-3rdplasmidconc1to1/tea4s15w_0_002778.tif", path "C:/Analysis_from_Movie_for_RiboTrap_Dieter/Movie_Data_Lorenz/TPA-3rdplasmidconc1to1/tea4s15w_0_002779.tif", path "C:/Analysis_from_Movie_for_RiboTrap_Dieter/Movie_Data_Lorenz/TPA-3rdplasmidconc1to1/tea4s15w_0_002780.tif", path "C:/Analysis_from_Movie_for_RiboTrap_Dieter/Movie_Data_Lorenz/TPA-3rdplasmidconc1to1/tea4s15w_0_002781.tif", path "C:/Analysis_from_Movie_for_RiboTrap_Dieter/Movie_Data_Lorenz/TPA-3rdplasmidconc1to1/tea4s15w_0_002782.tif", path "C:/Analysis_from_Movie_for_RiboTrap_Dieter/Movie_Data_Lorenz/TPA-3rdplasmidconc1to1/tea4s15w_0_002783.tif", path "C:/Analysis_from_Movie_for_RiboTrap_Dieter/Movie_Data_Lorenz/TPA-3rdplasmidconc1to1/tea4s15w_0_002784.tif", path "C:/Analysis_from_Movie_for_RiboTrap_Dieter/Movie_Data_Lorenz/TPA-3rdplasmidconc1to1/tea4s15w_0_002785.tif", path "C:/Analysis_from_Movie_for_RiboTrap_Dieter/Movie_Data_Lorenz/TPA-3rdplasmidconc1to1/tea4s15w_0_002786.tif", path "C:/Analysis_from_Movie_for_RiboTrap_Dieter/Movie_Data_Lorenz/TPA-3rdplasmidconc1to1/tea4s15w_0_002787.tif", path "C:/Analysis_from_Movie_for_RiboTrap_Dieter/Movie_Data_Lorenz/TPA-3rdplasmidconc1to1/tea4s15w_0_002788.tif", path "C:/Analysis_from_Movie_for_RiboTrap_Dieter/Movie_Data_Lorenz/TPA-3rdplasmidconc1to1/tea4s15w_0_002789.tif", path "C:/Analysis_from_Movie_for_RiboTrap_Dieter/Movie_Data_Lorenz/TPA-3rdplasmidconc1to1/tea4s15w_0_002790.tif", path "C:/Analysis_from_Movie_for_RiboTrap_Dieter/Movie_Data_Lorenz/TPA-3rdplasmidconc1to1/tea4s15w_0_002791.tif", path "C:/Analysis_from_Movie_for_RiboTrap_Dieter/Movie_Data_Lorenz/TPA-3rdplasmidconc1to1/tea4s15w_0_002792.tif", path "C:/Analysis_from_Movie_for_RiboTrap_Dieter/Movie_Data_Lorenz/TPA-3rdplasmidconc1to1/tea4s15w_0_002793.tif", path "C:/Analysis_from_Movie_for_RiboTrap_Dieter/Movie_Data_Lorenz/TPA-3rdplasmidconc1to1/tea4s15w_0_002794.tif", path "C:/Analysis_from_Movie_for_RiboTrap_Dieter/Movie_Data_Lorenz/TPA-3rdplasmidconc1to1/tea4s15w_0_002795.tif", path "C:/Analysis_from_Movie_for_RiboTrap_Dieter/Movie_Data_Lorenz/TPA-3rdplasmidconc1to1/tea4s15w_0_002796.tif", path "C:/Analysis_from_Movie_for_RiboTrap_Dieter/Movie_Data_Lorenz/TPA-3rdplasmidconc1to1/tea4s15w_0_002797.tif", path "C:/Analysis_from_Movie_for_RiboTrap_Dieter/Movie_Data_Lorenz/TPA-3rdplasmidconc1to1/tea4s15w_0_002798.tif", path "C:/Analysis_from_Movie_for_RiboTrap_Dieter/Movie_Data_Lorenz/TPA-3rdplasmidconc1to1/tea4s15w_0_002799.tif", path "C:/Analysis_from_Movie_for_RiboTrap_Dieter/Movie_Data_Lorenz/TPA-3rdplasmidconc1to1/tea4s15w_0_002800.tif", path "C:/Analysis_from_Movie_for_RiboTrap_Dieter/Movie_Data_Lorenz/TPA-3rdplasmidconc1to1/tea4s15w_0_002801.tif", path "C:/Analysis_from_Movie_for_RiboTrap_Dieter/Movie_Data_Lorenz/TPA-3rdplasmidconc1to1/tea4s15w_0_002802.tif", path "C:/Analysis_from_Movie_for_RiboTrap_Dieter/Movie_Data_Lorenz/TPA-3rdplasmidconc1to1/tea4s15w_0_002803.tif", path "C:/Analysis_from_Movie_for_RiboTrap_Dieter/Movie_Data_Lorenz/TPA-3rdplasmidconc1to1/tea4s15w_0_002804.tif", path "C:/Analysis_from_Movie_for_RiboTrap_Dieter/Movie_Data_Lorenz/TPA-3rdplasmidconc1to1/tea4s15w_0_002805.tif", path "C:/Analysis_from_Movie_for_RiboTrap_Dieter/Movie_Data_Lorenz/TPA-3rdplasmidconc1to1/tea4s15w_0_002806.tif", path "C:/Analysis_from_Movie_for_RiboTrap_Dieter/Movie_Data_Lorenz/TPA-3rdplasmidconc1to1/tea4s15w_0_002807.tif", path "C:/Analysis_from_Movie_for_RiboTrap_Dieter/Movie_Data_Lorenz/TPA-3rdplasmidconc1to1/tea4s15w_0_002808.tif", path "C:/Analysis_from_Movie_for_RiboTrap_Dieter/Movie_Data_Lorenz/TPA-3rdplasmidconc1to1/tea4s15w_0_002809.tif", path "C:/Analysis_from_Movie_for_RiboTrap_Dieter/Movie_Data_Lorenz/TPA-3rdplasmidconc1to1/tea4s15w_0_002810.tif", path "C:/Analysis_from_Movie_for_RiboTrap_Dieter/Movie_Data_Lorenz/TPA-3rdplasmidconc1to1/tea4s15w_0_002811.tif", path "C:/Analysis_from_Movie_for_RiboTrap_Dieter/Movie_Data_Lorenz/TPA-3rdplasmidconc1to1/tea4s15w_0_002812.tif", path "C:/Analysis_from_Movie_for_RiboTrap_Dieter/Movie_Data_Lorenz/TPA-3rdplasmidconc1to1/tea4s15w_0_002813.tif", path "C:/Analysis_from_Movie_for_RiboTrap_Dieter/Movie_Data_Lorenz/TPA-3rdplasmidconc1to1/tea4s15w_0_002814.tif", path "C:/Analysis_from_Movie_for_RiboTrap_Dieter/Movie_Data_Lorenz/TPA-3rdplasmidconc1to1/tea4s15w_0_002815.tif", path "C:/Analysis_from_Movie_for_RiboTrap_Dieter/Movie_Data_Lorenz/TPA-3rdplasmidconc1to1/tea4s15w_0_002816.tif", path "C:/Analysis_from_Movie_for_RiboTrap_Dieter/Movie_Data_Lorenz/TPA-3rdplasmidconc1to1/tea4s15w_0_002817.tif", path "C:/Analysis_from_Movie_for_RiboTrap_Dieter/Movie_Data_Lorenz/TPA-3rdplasmidconc1to1/tea4s15w_0_002818.tif", path "C:/Analysis_from_Movie_for_RiboTrap_Dieter/Movie_Data_Lorenz/TPA-3rdplasmidconc1to1/tea4s15w_0_002819.tif", path "C:/Analysis_from_Movie_for_RiboTrap_Dieter/Movie_Data_Lorenz/TPA-3rdplasmidconc1to1/tea4s15w_0_002820.tif", path "C:/Analysis_from_Movie_for_RiboTrap_Dieter/Movie_Data_Lorenz/TPA-3rdplasmidconc1to1/tea4s15w_0_002821.tif", path "C:/Analysis_from_Movie_for_RiboTrap_Dieter/Movie_Data_Lorenz/TPA-3rdplasmidconc1to1/tea4s15w_0_002822.tif", path "C:/Analysis_from_Movie_for_RiboTrap_Dieter/Movie_Data_Lorenz/TPA-3rdplasmidconc1to1/tea4s15w_0_002823.tif", path "C:/Analysis_from_Movie_for_RiboTrap_Dieter/Movie_Data_Lorenz/TPA-3rdplasmidconc1to1/tea4s15w_0_002824.tif", path "C:/Analysis_from_Movie_for_RiboTrap_Dieter/Movie_Data_Lorenz/TPA-3rdplasmidconc1to1/tea4s15w_0_002825.tif", path "C:/Analysis_from_Movie_for_RiboTrap_Dieter/Movie_Data_Lorenz/TPA-3rdplasmidconc1to1/tea4s15w_0_002826.tif", path "C:/Analysis_from_Movie_for_RiboTrap_Dieter/Movie_Data_Lorenz/TPA-3rdplasmidconc1to1/tea4s15w_0_002827.tif", path "C:/Analysis_from_Movie_for_RiboTrap_Dieter/Movie_Data_Lorenz/TPA-3rdplasmidconc1to1/tea4s15w_0_002828.tif", path "C:/Analysis_from_Movie_for_RiboTrap_Dieter/Movie_Data_Lorenz/TPA-3rdplasmidconc1to1/tea4s15w_0_002829.tif", path "C:/Analysis_from_Movie_for_RiboTrap_Dieter/Movie_Data_Lorenz/TPA-3rdplasmidconc1to1/tea4s15w_0_002830.tif", path "C:/Analysis_from_Movie_for_RiboTrap_Dieter/Movie_Data_Lorenz/TPA-3rdplasmidconc1to1/tea4s15w_0_002831.tif", path "C:/Analysis_from_Movie_for_RiboTrap_Dieter/Movie_Data_Lorenz/TPA-3rdplasmidconc1to1/tea4s15w_0_002832.tif", path "C:/Analysis_from_Movie_for_RiboTrap_Dieter/Movie_Data_Lorenz/TPA-3rdplasmidconc1to1/tea4s15w_0_002833.tif", path "C:/Analysis_from_Movie_for_RiboTrap_Dieter/Movie_Data_Lorenz/TPA-3rdplasmidconc1to1/tea4s15w_0_002834.tif", path "C:/Analysis_from_Movie_for_RiboTrap_Dieter/Movie_Data_Lorenz/TPA-3rdplasmidconc1to1/tea4s15w_0_002835.tif", path "C:/Analysis_from_Movie_for_RiboTrap_Dieter/Movie_Data_Lorenz/TPA-3rdplasmidconc1to1/tea4s15w_0_002836.tif", path "C:/Analysis_from_Movie_for_RiboTrap_Dieter/Movie_Data_Lorenz/TPA-3rdplasmidconc1to1/tea4s15w_0_002837.tif", path "C:/Analysis_from_Movie_for_RiboTrap_Dieter/Movie_Data_Lorenz/TPA-3rdplasmidconc1to1/tea4s15w_0_002838.tif", path "C:/Analysis_from_Movie_for_RiboTrap_Dieter/Movie_Data_Lorenz/TPA-3rdplasmidconc1to1/tea4s15w_0_002839.tif", path "C:/Analysis_from_Movie_for_RiboTrap_Dieter/Movie_Data_Lorenz/TPA-3rdplasmidconc1to1/tea4s15w_0_002840.tif", path "C:/Analysis_from_Movie_for_RiboTrap_Dieter/Movie_Data_Lorenz/TPA-3rdplasmidconc1to1/tea4s15w_0_002841.tif", path "C:/Analysis_from_Movie_for_RiboTrap_Dieter/Movie_Data_Lorenz/TPA-3rdplasmidconc1to1/tea4s15w_0_002842.tif", path "C:/Analysis_from_Movie_for_RiboTrap_Dieter/Movie_Data_Lorenz/TPA-3rdplasmidconc1to1/tea4s15w_0_002843.tif", path "C:/Analysis_from_Movie_for_RiboTrap_Dieter/Movie_Data_Lorenz/TPA-3rdplasmidconc1to1/tea4s15w_0_002844.tif", path "C:/Analysis_from_Movie_for_RiboTrap_Dieter/Movie_Data_Lorenz/TPA-3rdplasmidconc1to1/tea4s15w_0_002845.tif", path "C:/Analysis_from_Movie_for_RiboTrap_Dieter/Movie_Data_Lorenz/TPA-3rdplasmidconc1to1/tea4s15w_0_002846.tif", path "C:/Analysis_from_Movie_for_RiboTrap_Dieter/Movie_Data_Lorenz/TPA-3rdplasmidconc1to1/tea4s15w_0_002847.tif", path "C:/Analysis_from_Movie_for_RiboTrap_Dieter/Movie_Data_Lorenz/TPA-3rdplasmidconc1to1/tea4s15w_0_002848.tif", path "C:/Analysis_from_Movie_for_RiboTrap_Dieter/Movie_Data_Lorenz/TPA-3rdplasmidconc1to1/tea4s15w_0_002849.tif", path "C:/Analysis_from_Movie_for_RiboTrap_Dieter/Movie_Data_Lorenz/TPA-3rdplasmidconc1to1/tea4s15w_0_002850.tif", path "C:/Analysis_from_Movie_for_RiboTrap_Dieter/Movie_Data_Lorenz/TPA-3rdplasmidconc1to1/tea4s15w_0_002851.tif", path "C:/Analysis_from_Movie_for_RiboTrap_Dieter/Movie_Data_Lorenz/TPA-3rdplasmidconc1to1/tea4s15w_0_002852.tif", path "C:/Analysis_from_Movie_for_RiboTrap_Dieter/Movie_Data_Lorenz/TPA-3rdplasmidconc1to1/tea4s15w_0_002853.tif", path "C:/Analysis_from_Movie_for_RiboTrap_Dieter/Movie_Data_Lorenz/TPA-3rdplasmidconc1to1/tea4s15w_0_002854.tif", path "C:/Analysis_from_Movie_for_RiboTrap_Dieter/Movie_Data_Lorenz/TPA-3rdplasmidconc1to1/tea4s15w_0_002855.tif", path "C:/Analysis_from_Movie_for_RiboTrap_Dieter/Movie_Data_Lorenz/TPA-3rdplasmidconc1to1/tea4s15w_0_002856.tif", path "C:/Analysis_from_Movie_for_RiboTrap_Dieter/Movie_Data_Lorenz/TPA-3rdplasmidconc1to1/tea4s15w_0_002857.tif", path "C:/Analysis_from_Movie_for_RiboTrap_Dieter/Movie_Data_Lorenz/TPA-3rdplasmidconc1to1/tea4s15w_0_002858.tif", path "C:/Analysis_from_Movie_for_RiboTrap_Dieter/Movie_Data_Lorenz/TPA-3rdplasmidconc1to1/tea4s15w_0_002859.tif", path "C:/Analysis_from_Movie_for_RiboTrap_Dieter/Movie_Data_Lorenz/TPA-3rdplasmidconc1to1/tea4s15w_0_002860.tif", path "C:/Analysis_from_Movie_for_RiboTrap_Dieter/Movie_Data_Lorenz/TPA-3rdplasmidconc1to1/tea4s15w_0_002861.tif", path "C:/Analysis_from_Movie_for_RiboTrap_Dieter/Movie_Data_Lorenz/TPA-3rdplasmidconc1to1/tea4s15w_0_002862.tif", path "C:/Analysis_from_Movie_for_RiboTrap_Dieter/Movie_Data_Lorenz/TPA-3rdplasmidconc1to1/tea4s15w_0_002863.tif", path "C:/Analysis_from_Movie_for_RiboTrap_Dieter/Movie_Data_Lorenz/TPA-3rdplasmidconc1to1/tea4s15w_0_002864.tif", path "C:/Analysis_from_Movie_for_RiboTrap_Dieter/Movie_Data_Lorenz/TPA-3rdplasmidconc1to1/tea4s15w_0_002865.tif", path "C:/Analysis_from_Movie_for_RiboTrap_Dieter/Movie_Data_Lorenz/TPA-3rdplasmidconc1to1/tea4s15w_0_002866.tif", path "C:/Analysis_from_Movie_for_RiboTrap_Dieter/Movie_Data_Lorenz/TPA-3rdplasmidconc1to1/tea4s15w_0_002867.tif", path "C:/Analysis_from_Movie_for_RiboTrap_Dieter/Movie_Data_Lorenz/TPA-3rdplasmidconc1to1/tea4s15w_0_002868.tif", path "C:/Analysis_from_Movie_for_RiboTrap_Dieter/Movie_Data_Lorenz/TPA-3rdplasmidconc1to1/tea4s15w_0_002869.tif", path "C:/Analysis_from_Movie_for_RiboTrap_Dieter/Movie_Data_Lorenz/TPA-3rdplasmidconc1to1/tea4s15w_0_002870.tif", path "C:/Analysis_from_Movie_for_RiboTrap_Dieter/Movie_Data_Lorenz/TPA-3rdplasmidconc1to1/tea4s15w_0_002871.tif", path "C:/Analysis_from_Movie_for_RiboTrap_Dieter/Movie_Data_Lorenz/TPA-3rdplasmidconc1to1/tea4s15w_0_002872.tif", path "C:/Analysis_from_Movie_for_RiboTrap_Dieter/Movie_Data_Lorenz/TPA-3rdplasmidconc1to1/tea4s15w_0_002873.tif", path "C:/Analysis_from_Movie_for_RiboTrap_Dieter/Movie_Data_Lorenz/TPA-3rdplasmidconc1to1/tea4s15w_0_002874.tif", path "C:/Analysis_from_Movie_for_RiboTrap_Dieter/Movie_Data_Lorenz/TPA-3rdplasmidconc1to1/tea4s15w_0_002875.tif", path "C:/Analysis_from_Movie_for_RiboTrap_Dieter/Movie_Data_Lorenz/TPA-3rdplasmidconc1to1/tea4s15w_0_002876.tif", path "C:/Analysis_from_Movie_for_RiboTrap_Dieter/Movie_Data_Lorenz/TPA-3rdplasmidconc1to1/tea4s15w_0_002877.tif", path "C:/Analysis_from_Movie_for_RiboTrap_Dieter/Movie_Data_Lorenz/TPA-3rdplasmidconc1to1/tea4s15w_0_002878.tif", path "C:/Analysis_from_Movie_for_RiboTrap_Dieter/Movie_Data_Lorenz/TPA-3rdplasmidconc1to1/tea4s15w_0_002879.tif", path "C:/Analysis_from_Movie_for_RiboTrap_Dieter/Movie_Data_Lorenz/TPA-3rdplasmidconc1to1/tea4s15w_0_002880.tif", path "C:/Analysis_from_Movie_for_RiboTrap_Dieter/Movie_Data_Lorenz/TPA-3rdplasmidconc1to1/tea4s15w_0_002881.tif", path "C:/Analysis_from_Movie_for_RiboTrap_Dieter/Movie_Data_Lorenz/TPA-3rdplasmidconc1to1/tea4s15w_0_002882.tif", path "C:/Analysis_from_Movie_for_RiboTrap_Dieter/Movie_Data_Lorenz/TPA-3rdplasmidconc1to1/tea4s15w_0_002883.tif", path "C:/Analysis_from_Movie_for_RiboTrap_Dieter/Movie_Data_Lorenz/TPA-3rdplasmidconc1to1/tea4s15w_0_002884.tif", path "C:/Analysis_from_Movie_for_RiboTrap_Dieter/Movie_Data_Lorenz/TPA-3rdplasmidconc1to1/tea4s15w_0_002885.tif", path "C:/Analysis_from_Movie_for_RiboTrap_Dieter/Movie_Data_Lorenz/TPA-3rdplasmidconc1to1/tea4s15w_0_002886.tif", path "C:/Analysis_from_Movie_for_RiboTrap_Dieter/Movie_Data_Lorenz/TPA-3rdplasmidconc1to1/tea4s15w_0_002887.tif", path "C:/Analysis_from_Movie_for_RiboTrap_Dieter/Movie_Data_Lorenz/TPA-3rdplasmidconc1to1/tea4s15w_0_002888.tif", path "C:/Analysis_from_Movie_for_RiboTrap_Dieter/Movie_Data_Lorenz/TPA-3rdplasmidconc1to1/tea4s15w_0_002889.tif", path "C:/Analysis_from_Movie_for_RiboTrap_Dieter/Movie_Data_Lorenz/TPA-3rdplasmidconc1to1/tea4s15w_0_002890.tif", path "C:/Analysis_from_Movie_for_RiboTrap_Dieter/Movie_Data_Lorenz/TPA-3rdplasmidconc1to1/tea4s15w_0_002891.tif", path "C:/Analysis_from_Movie_for_RiboTrap_Dieter/Movie_Data_Lorenz/TPA-3rdplasmidconc1to1/tea4s15w_0_002892.tif", path "C:/Analysis_from_Movie_for_RiboTrap_Dieter/Movie_Data_Lorenz/TPA-3rdplasmidconc1to1/tea4s15w_0_002893.tif", path "C:/Analysis_from_Movie_for_RiboTrap_Dieter/Movie_Data_Lorenz/TPA-3rdplasmidconc1to1/tea4s15w_0_002894.tif", path "C:/Analysis_from_Movie_for_RiboTrap_Dieter/Movie_Data_Lorenz/TPA-3rdplasmidconc1to1/tea4s15w_0_002895.tif", path "C:/Analysis_from_Movie_for_RiboTrap_Dieter/Movie_Data_Lorenz/TPA-3rdplasmidconc1to1/tea4s15w_0_002896.tif", path "C:/Analysis_from_Movie_for_RiboTrap_Dieter/Movie_Data_Lorenz/TPA-3rdplasmidconc1to1/tea4s15w_0_002897.tif", path "C:/Analysis_from_Movie_for_RiboTrap_Dieter/Movie_Data_Lorenz/TPA-3rdplasmidconc1to1/tea4s15w_0_002898.tif", path "C:/Analysis_from_Movie_for_RiboTrap_Dieter/Movie_Data_Lorenz/TPA-3rdplasmidconc1to1/tea4s15w_0_002899.tif", path "C:/Analysis_from_Movie_for_RiboTrap_Dieter/Movie_Data_Lorenz/TPA-3rdplasmidconc1to1/tea4s15w_0_002900.tif", path "C:/Analysis_from_Movie_for_RiboTrap_Dieter/Movie_Data_Lorenz/TPA-3rdplasmidconc1to1/tea4s15w_0_002901.tif", path "C:/Analysis_from_Movie_for_RiboTrap_Dieter/Movie_Data_Lorenz/TPA-3rdplasmidconc1to1/tea4s15w_0_002902.tif", path "C:/Analysis_from_Movie_for_RiboTrap_Dieter/Movie_Data_Lorenz/TPA-3rdplasmidconc1to1/tea4s15w_0_002903.tif", path "C:/Analysis_from_Movie_for_RiboTrap_Dieter/Movie_Data_Lorenz/TPA-3rdplasmidconc1to1/tea4s15w_0_002904.tif", path "C:/Analysis_from_Movie_for_RiboTrap_Dieter/Movie_Data_Lorenz/TPA-3rdplasmidconc1to1/tea4s15w_0_002905.tif", path "C:/Analysis_from_Movie_for_RiboTrap_Dieter/Movie_Data_Lorenz/TPA-3rdplasmidconc1to1/tea4s15w_0_002906.tif", path "C:/Analysis_from_Movie_for_RiboTrap_Dieter/Movie_Data_Lorenz/TPA-3rdplasmidconc1to1/tea4s15w_0_002907.tif", path "C:/Analysis_from_Movie_for_RiboTrap_Dieter/Movie_Data_Lorenz/TPA-3rdplasmidconc1to1/tea4s15w_0_002908.tif", path "C:/Analysis_from_Movie_for_RiboTrap_Dieter/Movie_Data_Lorenz/TPA-3rdplasmidconc1to1/tea4s15w_0_002909.tif", path "C:/Analysis_from_Movie_for_RiboTrap_Dieter/Movie_Data_Lorenz/TPA-3rdplasmidconc1to1/tea4s15w_0_002910.tif", path "C:/Analysis_from_Movie_for_RiboTrap_Dieter/Movie_Data_Lorenz/TPA-3rdplasmidconc1to1/tea4s15w_0_002911.tif", path "C:/Analysis_from_Movie_for_RiboTrap_Dieter/Movie_Data_Lorenz/TPA-3rdplasmidconc1to1/tea4s15w_0_002912.tif", path "C:/Analysis_from_Movie_for_RiboTrap_Dieter/Movie_Data_Lorenz/TPA-3rdplasmidconc1to1/tea4s15w_0_002913.tif", path "C:/Analysis_from_Movie_for_RiboTrap_Dieter/Movie_Data_Lorenz/TPA-3rdplasmidconc1to1/tea4s15w_0_002914.tif", path "C:/Analysis_from_Movie_for_RiboTrap_Dieter/Movie_Data_Lorenz/TPA-3rdplasmidconc1to1/tea4s15w_0_002915.tif", path "C:/Analysis_from_Movie_for_RiboTrap_Dieter/Movie_Data_Lorenz/TPA-3rdplasmidconc1to1/tea4s15w_0_002916.tif", path "C:/Analysis_from_Movie_for_RiboTrap_Dieter/Movie_Data_Lorenz/TPA-3rdplasmidconc1to1/tea4s15w_0_002917.tif", path "C:/Analysis_from_Movie_for_RiboTrap_Dieter/Movie_Data_Lorenz/TPA-3rdplasmidconc1to1/tea4s15w_0_002918.tif", path "C:/Analysis_from_Movie_for_RiboTrap_Dieter/Movie_Data_Lorenz/TPA-3rdplasmidconc1to1/tea4s15w_0_002919.tif", path "C:/Analysis_from_Movie_for_RiboTrap_Dieter/Movie_Data_Lorenz/TPA-3rdplasmidconc1to1/tea4s15w_0_002920.tif", path "C:/Analysis_from_Movie_for_RiboTrap_Dieter/Movie_Data_Lorenz/TPA-3rdplasmidconc1to1/tea4s15w_0_002921.tif", path "C:/Analysis_from_Movie_for_RiboTrap_Dieter/Movie_Data_Lorenz/TPA-3rdplasmidconc1to1/tea4s15w_0_002922.tif", path "C:/Analysis_from_Movie_for_RiboTrap_Dieter/Movie_Data_Lorenz/TPA-3rdplasmidconc1to1/tea4s15w_0_002923.tif", path "C:/Analysis_from_Movie_for_RiboTrap_Dieter/Movie_Data_Lorenz/TPA-3rdplasmidconc1to1/tea4s15w_0_002924.tif", path "C:/Analysis_from_Movie_for_RiboTrap_Dieter/Movie_Data_Lorenz/TPA-3rdplasmidconc1to1/tea4s15w_0_002925.tif", path "C:/Analysis_from_Movie_for_RiboTrap_Dieter/Movie_Data_Lorenz/TPA-3rdplasmidconc1to1/tea4s15w_0_002926.tif", path "C:/Analysis_from_Movie_for_RiboTrap_Dieter/Movie_Data_Lorenz/TPA-3rdplasmidconc1to1/tea4s15w_0_002927.tif", path "C:/Analysis_from_Movie_for_RiboTrap_Dieter/Movie_Data_Lorenz/TPA-3rdplasmidconc1to1/tea4s15w_0_002928.tif", path "C:/Analysis_from_Movie_for_RiboTrap_Dieter/Movie_Data_Lorenz/TPA-3rdplasmidconc1to1/tea4s15w_0_002929.tif", path "C:/Analysis_from_Movie_for_RiboTrap_Dieter/Movie_Data_Lorenz/TPA-3rdplasmidconc1to1/tea4s15w_0_002930.tif", path "C:/Analysis_from_Movie_for_RiboTrap_Dieter/Movie_Data_Lorenz/TPA-3rdplasmidconc1to1/tea4s15w_0_002931.tif", path "C:/Analysis_from_Movie_for_RiboTrap_Dieter/Movie_Data_Lorenz/TPA-3rdplasmidconc1to1/tea4s15w_0_002932.tif", path "C:/Analysis_from_Movie_for_RiboTrap_Dieter/Movie_Data_Lorenz/TPA-3rdplasmidconc1to1/tea4s15w_0_002933.tif", path "C:/Analysis_from_Movie_for_RiboTrap_Dieter/Movie_Data_Lorenz/TPA-3rdplasmidconc1to1/tea4s15w_0_002934.tif", path "C:/Analysis_from_Movie_for_RiboTrap_Dieter/Movie_Data_Lorenz/TPA-3rdplasmidconc1to1/tea4s15w_0_002935.tif", path "C:/Analysis_from_Movie_for_RiboTrap_Dieter/Movie_Data_Lorenz/TPA-3rdplasmidconc1to1/tea4s15w_0_002936.tif", path "C:/Analysis_from_Movie_for_RiboTrap_Dieter/Movie_Data_Lorenz/TPA-3rdplasmidconc1to1/tea4s15w_0_002937.tif", path "C:/Analysis_from_Movie_for_RiboTrap_Dieter/Movie_Data_Lorenz/TPA-3rdplasmidconc1to1/tea4s15w_0_002938.tif", path "C:/Analysis_from_Movie_for_RiboTrap_Dieter/Movie_Data_Lorenz/TPA-3rdplasmidconc1to1/tea4s15w_0_002939.tif", path "C:/Analysis_from_Movie_for_RiboTrap_Dieter/Movie_Data_Lorenz/TPA-3rdplasmidconc1to1/tea4s15w_0_002940.tif", path "C:/Analysis_from_Movie_for_RiboTrap_Dieter/Movie_Data_Lorenz/TPA-3rdplasmidconc1to1/tea4s15w_0_002941.tif", path "C:/Analysis_from_Movie_for_RiboTrap_Dieter/Movie_Data_Lorenz/TPA-3rdplasmidconc1to1/tea4s15w_0_002942.tif", path "C:/Analysis_from_Movie_for_RiboTrap_Dieter/Movie_Data_Lorenz/TPA-3rdplasmidconc1to1/tea4s15w_0_002943.tif", path "C:/Analysis_from_Movie_for_RiboTrap_Dieter/Movie_Data_Lorenz/TPA-3rdplasmidconc1to1/tea4s15w_0_002944.tif", path "C:/Analysis_from_Movie_for_RiboTrap_Dieter/Movie_Data_Lorenz/TPA-3rdplasmidconc1to1/tea4s15w_0_002945.tif", path "C:/Analysis_from_Movie_for_RiboTrap_Dieter/Movie_Data_Lorenz/TPA-3rdplasmidconc1to1/tea4s15w_0_002946.tif", path "C:/Analysis_from_Movie_for_RiboTrap_Dieter/Movie_Data_Lorenz/TPA-3rdplasmidconc1to1/tea4s15w_0_002947.tif", path "C:/Analysis_from_Movie_for_RiboTrap_Dieter/Movie_Data_Lorenz/TPA-3rdplasmidconc1to1/tea4s15w_0_002948.tif", path "C:/Analysis_from_Movie_for_RiboTrap_Dieter/Movie_Data_Lorenz/TPA-3rdplasmidconc1to1/tea4s15w_0_002949.tif", path "C:/Analysis_from_Movie_for_RiboTrap_Dieter/Movie_Data_Lorenz/TPA-3rdplasmidconc1to1/tea4s15w_0_002950.tif", path "C:/Analysis_from_Movie_for_RiboTrap_Dieter/Movie_Data_Lorenz/TPA-3rdplasmidconc1to1/tea4s15w_0_002951.tif", path "C:/Analysis_from_Movie_for_RiboTrap_Dieter/Movie_Data_Lorenz/TPA-3rdplasmidconc1to1/tea4s15w_0_002952.tif", path "C:/Analysis_from_Movie_for_RiboTrap_Dieter/Movie_Data_Lorenz/TPA-3rdplasmidconc1to1/tea4s15w_0_002953.tif", path "C:/Analysis_from_Movie_for_RiboTrap_Dieter/Movie_Data_Lorenz/TPA-3rdplasmidconc1to1/tea4s15w_0_002954.tif", path "C:/Analysis_from_Movie_for_RiboTrap_Dieter/Movie_Data_Lorenz/TPA-3rdplasmidconc1to1/tea4s15w_0_002955.tif", path "C:/Analysis_from_Movie_for_RiboTrap_Dieter/Movie_Data_Lorenz/TPA-3rdplasmidconc1to1/tea4s15w_0_002956.tif", path "C:/Analysis_from_Movie_for_RiboTrap_Dieter/Movie_Data_Lorenz/TPA-3rdplasmidconc1to1/tea4s15w_0_002957.tif", path "C:/Analysis_from_Movie_for_RiboTrap_Dieter/Movie_Data_Lorenz/TPA-3rdplasmidconc1to1/tea4s15w_0_002958.tif", path "C:/Analysis_from_Movie_for_RiboTrap_Dieter/Movie_Data_Lorenz/TPA-3rdplasmidconc1to1/tea4s15w_0_002959.tif", path "C:/Analysis_from_Movie_for_RiboTrap_Dieter/Movie_Data_Lorenz/TPA-3rdplasmidconc1to1/tea4s15w_0_002960.tif", path "C:/Analysis_from_Movie_for_RiboTrap_Dieter/Movie_Data_Lorenz/TPA-3rdplasmidconc1to1/tea4s15w_0_002961.tif", path "C:/Analysis_from_Movie_for_RiboTrap_Dieter/Movie_Data_Lorenz/TPA-3rdplasmidconc1to1/tea4s15w_0_002962.tif", path "C:/Analysis_from_Movie_for_RiboTrap_Dieter/Movie_Data_Lorenz/TPA-3rdplasmidconc1to1/tea4s15w_0_002963.tif", path "C:/Analysis_from_Movie_for_RiboTrap_Dieter/Movie_Data_Lorenz/TPA-3rdplasmidconc1to1/tea4s15w_0_002964.tif", path "C:/Analysis_from_Movie_for_RiboTrap_Dieter/Movie_Data_Lorenz/TPA-3rdplasmidconc1to1/tea4s15w_0_002965.tif", path "C:/Analysis_from_Movie_for_RiboTrap_Dieter/Movie_Data_Lorenz/TPA-3rdplasmidconc1to1/tea4s15w_0_002966.tif", path "C:/Analysis_from_Movie_for_RiboTrap_Dieter/Movie_Data_Lorenz/TPA-3rdplasmidconc1to1/tea4s15w_0_002967.tif", path "C:/Analysis_from_Movie_for_RiboTrap_Dieter/Movie_Data_Lorenz/TPA-3rdplasmidconc1to1/tea4s15w_0_002968.tif", path "C:/Analysis_from_Movie_for_RiboTrap_Dieter/Movie_Data_Lorenz/TPA-3rdplasmidconc1to1/tea4s15w_0_002969.tif", path "C:/Analysis_from_Movie_for_RiboTrap_Dieter/Movie_Data_Lorenz/TPA-3rdplasmidconc1to1/tea4s15w_0_002970.tif", path "C:/Analysis_from_Movie_for_RiboTrap_Dieter/Movie_Data_Lorenz/TPA-3rdplasmidconc1to1/tea4s15w_0_002971.tif", path "C:/Analysis_from_Movie_for_RiboTrap_Dieter/Movie_Data_Lorenz/TPA-3rdplasmidconc1to1/tea4s15w_0_002972.tif", path "C:/Analysis_from_Movie_for_RiboTrap_Dieter/Movie_Data_Lorenz/TPA-3rdplasmidconc1to1/tea4s15w_0_002973.tif", path "C:/Analysis_from_Movie_for_RiboTrap_Dieter/Movie_Data_Lorenz/TPA-3rdplasmidconc1to1/tea4s15w_0_002974.tif", path "C:/Analysis_from_Movie_for_RiboTrap_Dieter/Movie_Data_Lorenz/TPA-3rdplasmidconc1to1/tea4s15w_0_002975.tif", path "C:/Analysis_from_Movie_for_RiboTrap_Dieter/Movie_Data_Lorenz/TPA-3rdplasmidconc1to1/tea4s15w_0_002976.tif", path "C:/Analysis_from_Movie_for_RiboTrap_Dieter/Movie_Data_Lorenz/TPA-3rdplasmidconc1to1/tea4s15w_0_002977.tif", path "C:/Analysis_from_Movie_for_RiboTrap_Dieter/Movie_Data_Lorenz/TPA-3rdplasmidconc1to1/tea4s15w_0_002978.tif", path "C:/Analysis_from_Movie_for_RiboTrap_Dieter/Movie_Data_Lorenz/TPA-3rdplasmidconc1to1/tea4s15w_0_002979.tif", path "C:/Analysis_from_Movie_for_RiboTrap_Dieter/Movie_Data_Lorenz/TPA-3rdplasmidconc1to1/tea4s15w_0_002980.tif", path "C:/Analysis_from_Movie_for_RiboTrap_Dieter/Movie_Data_Lorenz/TPA-3rdplasmidconc1to1/tea4s15w_0_002981.tif", path "C:/Analysis_from_Movie_for_RiboTrap_Dieter/Movie_Data_Lorenz/TPA-3rdplasmidconc1to1/tea4s15w_0_002982.tif", path "C:/Analysis_from_Movie_for_RiboTrap_Dieter/Movie_Data_Lorenz/TPA-3rdplasmidconc1to1/tea4s15w_0_002983.tif", path "C:/Analysis_from_Movie_for_RiboTrap_Dieter/Movie_Data_Lorenz/TPA-3rdplasmidconc1to1/tea4s15w_0_002984.tif", path "C:/Analysis_from_Movie_for_RiboTrap_Dieter/Movie_Data_Lorenz/TPA-3rdplasmidconc1to1/tea4s15w_0_002985.tif", path "C:/Analysis_from_Movie_for_RiboTrap_Dieter/Movie_Data_Lorenz/TPA-3rdplasmidconc1to1/tea4s15w_0_002986.tif", path "C:/Analysis_from_Movie_for_RiboTrap_Dieter/Movie_Data_Lorenz/TPA-3rdplasmidconc1to1/tea4s15w_0_002987.tif", path "C:/Analysis_from_Movie_for_RiboTrap_Dieter/Movie_Data_Lorenz/TPA-3rdplasmidconc1to1/tea4s15w_0_002988.tif", path "C:/Analysis_from_Movie_for_RiboTrap_Dieter/Movie_Data_Lorenz/TPA-3rdplasmidconc1to1/tea4s15w_0_002989.tif", path "C:/Analysis_from_Movie_for_RiboTrap_Dieter/Movie_Data_Lorenz/TPA-3rdplasmidconc1to1/tea4s15w_0_002990.tif", path "C:/Analysis_from_Movie_for_RiboTrap_Dieter/Movie_Data_Lorenz/TPA-3rdplasmidconc1to1/tea4s15w_0_002991.tif", path "C:/Analysis_from_Movie_for_RiboTrap_Dieter/Movie_Data_Lorenz/TPA-3rdplasmidconc1to1/tea4s15w_0_002992.tif", path "C:/Analysis_from_Movie_for_RiboTrap_Dieter/Movie_Data_Lorenz/TPA-3rdplasmidconc1to1/tea4s15w_0_002993.tif", path "C:/Analysis_from_Movie_for_RiboTrap_Dieter/Movie_Data_Lorenz/TPA-3rdplasmidconc1to1/tea4s15w_0_002994.tif", path "C:/Analysis_from_Movie_for_RiboTrap_Dieter/Movie_Data_Lorenz/TPA-3rdplasmidconc1to1/tea4s15w_0_002995.tif", path "C:/Analysis_from_Movie_for_RiboTrap_Dieter/Movie_Data_Lorenz/TPA-3rdplasmidconc1to1/tea4s15w_0_002996.tif", path "C:/Analysis_from_Movie_for_RiboTrap_Dieter/Movie_Data_Lorenz/TPA-3rdplasmidconc1to1/tea4s15w_0_002997.tif", path "C:/Analysis_from_Movie_for_RiboTrap_Dieter/Movie_Data_Lorenz/TPA-3rdplasmidconc1to1/tea4s15w_0_002998.tif", path "C:/Analysis_from_Movie_for_RiboTrap_Dieter/Movie_Data_Lorenz/TPA-3rdplasmidconc1to1/tea4s15w_0_002999.tif", path "C:/Analysis_from_Movie_for_RiboTrap_Dieter/Movie_Data_Lorenz/TPA-3rdplasmidconc1to1/tea4s15w_0_003000.tif", path "C:/Analysis_from_Movie_for_RiboTrap_Dieter/Movie_Data_Lorenz/TPA-3rdplasmidconc1to1/tea4s15w_0_003001.tif", path "C:/Analysis_from_Movie_for_RiboTrap_Dieter/Movie_Data_Lorenz/TPA-3rdplasmidconc1to1/tea4s15w_0_003002.tif", path "C:/Analysis_from_Movie_for_RiboTrap_Dieter/Movie_Data_Lorenz/TPA-3rdplasmidconc1to1/tea4s15w_0_003003.tif", path "C:/Analysis_from_Movie_for_RiboTrap_Dieter/Movie_Data_Lorenz/TPA-3rdplasmidconc1to1/tea4s15w_0_003004.tif", path "C:/Analysis_from_Movie_for_RiboTrap_Dieter/Movie_Data_Lorenz/TPA-3rdplasmidconc1to1/tea4s15w_0_003005.tif", path "C:/Analysis_from_Movie_for_RiboTrap_Dieter/Movie_Data_Lorenz/TPA-3rdplasmidconc1to1/tea4s15w_0_003006.tif", path "C:/Analysis_from_Movie_for_RiboTrap_Dieter/Movie_Data_Lorenz/TPA-3rdplasmidconc1to1/tea4s15w_0_003007.tif", path "C:/Analysis_from_Movie_for_RiboTrap_Dieter/Movie_Data_Lorenz/TPA-3rdplasmidconc1to1/tea4s15w_0_003008.tif", path "C:/Analysis_from_Movie_for_RiboTrap_Dieter/Movie_Data_Lorenz/TPA-3rdplasmidconc1to1/tea4s15w_0_003009.tif", path "C:/Analysis_from_Movie_for_RiboTrap_Dieter/Movie_Data_Lorenz/TPA-3rdplasmidconc1to1/tea4s15w_0_003010.tif", path "C:/Analysis_from_Movie_for_RiboTrap_Dieter/Movie_Data_Lorenz/TPA-3rdplasmidconc1to1/tea4s15w_0_003011.tif", path "C:/Analysis_from_Movie_for_RiboTrap_Dieter/Movie_Data_Lorenz/TPA-3rdplasmidconc1to1/tea4s15w_0_003012.tif", path "C:/Analysis_from_Movie_for_RiboTrap_Dieter/Movie_Data_Lorenz/TPA-3rdplasmidconc1to1/tea4s15w_0_003013.tif", path "C:/Analysis_from_Movie_for_RiboTrap_Dieter/Movie_Data_Lorenz/TPA-3rdplasmidconc1to1/tea4s15w_0_003014.tif", path "C:/Analysis_from_Movie_for_RiboTrap_Dieter/Movie_Data_Lorenz/TPA-3rdplasmidconc1to1/tea4s15w_0_003015.tif", path "C:/Analysis_from_Movie_for_RiboTrap_Dieter/Movie_Data_Lorenz/TPA-3rdplasmidconc1to1/tea4s15w_0_003016.tif", path "C:/Analysis_from_Movie_for_RiboTrap_Dieter/Movie_Data_Lorenz/TPA-3rdplasmidconc1to1/tea4s15w_0_003017.tif", path "C:/Analysis_from_Movie_for_RiboTrap_Dieter/Movie_Data_Lorenz/TPA-3rdplasmidconc1to1/tea4s15w_0_003018.tif", path "C:/Analysis_from_Movie_for_RiboTrap_Dieter/Movie_Data_Lorenz/TPA-3rdplasmidconc1to1/tea4s15w_0_003019.tif", path "C:/Analysis_from_Movie_for_RiboTrap_Dieter/Movie_Data_Lorenz/TPA-3rdplasmidconc1to1/tea4s15w_0_003020.tif", path "C:/Analysis_from_Movie_for_RiboTrap_Dieter/Movie_Data_Lorenz/TPA-3rdplasmidconc1to1/tea4s15w_0_003021.tif", path "C:/Analysis_from_Movie_for_RiboTrap_Dieter/Movie_Data_Lorenz/TPA-3rdplasmidconc1to1/tea4s15w_0_003022.tif", path "C:/Analysis_from_Movie_for_RiboTrap_Dieter/Movie_Data_Lorenz/TPA-3rdplasmidconc1to1/tea4s15w_0_003023.tif", path "C:/Analysis_from_Movie_for_RiboTrap_Dieter/Movie_Data_Lorenz/TPA-3rdplasmidconc1to1/tea4s15w_0_003024.tif", path "C:/Analysis_from_Movie_for_RiboTrap_Dieter/Movie_Data_Lorenz/TPA-3rdplasmidconc1to1/tea4s15w_0_003025.tif", path "C:/Analysis_from_Movie_for_RiboTrap_Dieter/Movie_Data_Lorenz/TPA-3rdplasmidconc1to1/tea4s15w_0_003026.tif", path "C:/Analysis_from_Movie_for_RiboTrap_Dieter/Movie_Data_Lorenz/TPA-3rdplasmidconc1to1/tea4s15w_0_003027.tif", path "C:/Analysis_from_Movie_for_RiboTrap_Dieter/Movie_Data_Lorenz/TPA-3rdplasmidconc1to1/tea4s15w_0_003028.tif", path "C:/Analysis_from_Movie_for_RiboTrap_Dieter/Movie_Data_Lorenz/TPA-3rdplasmidconc1to1/tea4s15w_0_003029.tif", path "C:/Analysis_from_Movie_for_RiboTrap_Dieter/Movie_Data_Lorenz/TPA-3rdplasmidconc1to1/tea4s15w_0_003030.tif", path "C:/Analysis_from_Movie_for_RiboTrap_Dieter/Movie_Data_Lorenz/TPA-3rdplasmidconc1to1/tea4s15w_0_003031.tif", path "C:/Analysis_from_Movie_for_RiboTrap_Dieter/Movie_Data_Lorenz/TPA-3rdplasmidconc1to1/tea4s15w_0_003032.tif", path "C:/Analysis_from_Movie_for_RiboTrap_Dieter/Movie_Data_Lorenz/TPA-3rdplasmidconc1to1/tea4s15w_0_003033.tif", path "C:/Analysis_from_Movie_for_RiboTrap_Dieter/Movie_Data_Lorenz/TPA-3rdplasmidconc1to1/tea4s15w_0_003034.tif", path "C:/Analysis_from_Movie_for_RiboTrap_Dieter/Movie_Data_Lorenz/TPA-3rdplasmidconc1to1/tea4s15w_0_003035.tif", path "C:/Analysis_from_Movie_for_RiboTrap_Dieter/Movie_Data_Lorenz/TPA-3rdplasmidconc1to1/tea4s15w_0_003036.tif", path "C:/Analysis_from_Movie_for_RiboTrap_Dieter/Movie_Data_Lorenz/TPA-3rdplasmidconc1to1/tea4s15w_0_003037.tif", path "C:/Analysis_from_Movie_for_RiboTrap_Dieter/Movie_Data_Lorenz/TPA-3rdplasmidconc1to1/tea4s15w_0_003038.tif", path "C:/Analysis_from_Movie_for_RiboTrap_Dieter/Movie_Data_Lorenz/TPA-3rdplasmidconc1to1/tea4s15w_0_003039.tif", path "C:/Analysis_from_Movie_for_RiboTrap_Dieter/Movie_Data_Lorenz/TPA-3rdplasmidconc1to1/tea4s15w_0_003040.tif", path "C:/Analysis_from_Movie_for_RiboTrap_Dieter/Movie_Data_Lorenz/TPA-3rdplasmidconc1to1/tea4s15w_0_003041.tif", path "C:/Analysis_from_Movie_for_RiboTrap_Dieter/Movie_Data_Lorenz/TPA-3rdplasmidconc1to1/tea4s15w_0_003042.tif", path "C:/Analysis_from_Movie_for_RiboTrap_Dieter/Movie_Data_Lorenz/TPA-3rdplasmidconc1to1/tea4s15w_0_003043.tif", path "C:/Analysis_from_Movie_for_RiboTrap_Dieter/Movie_Data_Lorenz/TPA-3rdplasmidconc1to1/tea4s15w_0_003044.tif", path "C:/Analysis_from_Movie_for_RiboTrap_Dieter/Movie_Data_Lorenz/TPA-3rdplasmidconc1to1/tea4s15w_0_003045.tif", path "C:/Analysis_from_Movie_for_RiboTrap_Dieter/Movie_Data_Lorenz/TPA-3rdplasmidconc1to1/tea4s15w_0_003046.tif", path "C:/Analysis_from_Movie_for_RiboTrap_Dieter/Movie_Data_Lorenz/TPA-3rdplasmidconc1to1/tea4s15w_0_003047.tif", path "C:/Analysis_from_Movie_for_RiboTrap_Dieter/Movie_Data_Lorenz/TPA-3rdplasmidconc1to1/tea4s15w_0_003048.tif", path "C:/Analysis_from_Movie_for_RiboTrap_Dieter/Movie_Data_Lorenz/TPA-3rdplasmidconc1to1/tea4s15w_0_003049.tif", path "C:/Analysis_from_Movie_for_RiboTrap_Dieter/Movie_Data_Lorenz/TPA-3rdplasmidconc1to1/tea4s15w_0_003050.tif", path "C:/Analysis_from_Movie_for_RiboTrap_Dieter/Movie_Data_Lorenz/TPA-3rdplasmidconc1to1/tea4s15w_0_003051.tif", path "C:/Analysis_from_Movie_for_RiboTrap_Dieter/Movie_Data_Lorenz/TPA-3rdplasmidconc1to1/tea4s15w_0_003052.tif", path "C:/Analysis_from_Movie_for_RiboTrap_Dieter/Movie_Data_Lorenz/TPA-3rdplasmidconc1to1/tea4s15w_0_003053.tif", path "C:/Analysis_from_Movie_for_RiboTrap_Dieter/Movie_Data_Lorenz/TPA-3rdplasmidconc1to1/tea4s15w_0_003054.tif", path "C:/Analysis_from_Movie_for_RiboTrap_Dieter/Movie_Data_Lorenz/TPA-3rdplasmidconc1to1/tea4s15w_0_003055.tif", path "C:/Analysis_from_Movie_for_RiboTrap_Dieter/Movie_Data_Lorenz/TPA-3rdplasmidconc1to1/tea4s15w_0_003056.tif", path "C:/Analysis_from_Movie_for_RiboTrap_Dieter/Movie_Data_Lorenz/TPA-3rdplasmidconc1to1/tea4s15w_0_003057.tif", path "C:/Analysis_from_Movie_for_RiboTrap_Dieter/Movie_Data_Lorenz/TPA-3rdplasmidconc1to1/tea4s15w_0_003058.tif", path "C:/Analysis_from_Movie_for_RiboTrap_Dieter/Movie_Data_Lorenz/TPA-3rdplasmidconc1to1/tea4s15w_0_003059.tif", path "C:/Analysis_from_Movie_for_RiboTrap_Dieter/Movie_Data_Lorenz/TPA-3rdplasmidconc1to1/tea4s15w_0_003060.tif", path "C:/Analysis_from_Movie_for_RiboTrap_Dieter/Movie_Data_Lorenz/TPA-3rdplasmidconc1to1/tea4s15w_0_003061.tif", path "C:/Analysis_from_Movie_for_RiboTrap_Dieter/Movie_Data_Lorenz/TPA-3rdplasmidconc1to1/tea4s15w_0_003062.tif", path "C:/Analysis_from_Movie_for_RiboTrap_Dieter/Movie_Data_Lorenz/TPA-3rdplasmidconc1to1/tea4s15w_0_003063.tif", path "C:/Analysis_from_Movie_for_RiboTrap_Dieter/Movie_Data_Lorenz/TPA-3rdplasmidconc1to1/tea4s15w_0_003064.tif", path "C:/Analysis_from_Movie_for_RiboTrap_Dieter/Movie_Data_Lorenz/TPA-3rdplasmidconc1to1/tea4s15w_0_003065.tif", path "C:/Analysis_from_Movie_for_RiboTrap_Dieter/Movie_Data_Lorenz/TPA-3rdplasmidconc1to1/tea4s15w_0_003066.tif", path "C:/Analysis_from_Movie_for_RiboTrap_Dieter/Movie_Data_Lorenz/TPA-3rdplasmidconc1to1/tea4s15w_0_003067.tif", path "C:/Analysis_from_Movie_for_RiboTrap_Dieter/Movie_Data_Lorenz/TPA-3rdplasmidconc1to1/tea4s15w_0_003068.tif", path "C:/Analysis_from_Movie_for_RiboTrap_Dieter/Movie_Data_Lorenz/TPA-3rdplasmidconc1to1/tea4s15w_0_003069.tif", path "C:/Analysis_from_Movie_for_RiboTrap_Dieter/Movie_Data_Lorenz/TPA-3rdplasmidconc1to1/tea4s15w_0_003070.tif", path "C:/Analysis_from_Movie_for_RiboTrap_Dieter/Movie_Data_Lorenz/TPA-3rdplasmidconc1to1/tea4s15w_0_003071.tif", path "C:/Analysis_from_Movie_for_RiboTrap_Dieter/Movie_Data_Lorenz/TPA-3rdplasmidconc1to1/tea4s15w_0_003072.tif", path "C:/Analysis_from_Movie_for_RiboTrap_Dieter/Movie_Data_Lorenz/TPA-3rdplasmidconc1to1/tea4s15w_0_003073.tif", path "C:/Analysis_from_Movie_for_RiboTrap_Dieter/Movie_Data_Lorenz/TPA-3rdplasmidconc1to1/tea4s15w_0_003074.tif", path "C:/Analysis_from_Movie_for_RiboTrap_Dieter/Movie_Data_Lorenz/TPA-3rdplasmidconc1to1/tea4s15w_0_003075.tif", path "C:/Analysis_from_Movie_for_RiboTrap_Dieter/Movie_Data_Lorenz/TPA-3rdplasmidconc1to1/tea4s15w_0_003076.tif", path "C:/Analysis_from_Movie_for_RiboTrap_Dieter/Movie_Data_Lorenz/TPA-3rdplasmidconc1to1/tea4s15w_0_003077.tif", path "C:/Analysis_from_Movie_for_RiboTrap_Dieter/Movie_Data_Lorenz/TPA-3rdplasmidconc1to1/tea4s15w_0_003078.tif", path "C:/Analysis_from_Movie_for_RiboTrap_Dieter/Movie_Data_Lorenz/TPA-3rdplasmidconc1to1/tea4s15w_0_003079.tif", path "C:/Analysis_from_Movie_for_RiboTrap_Dieter/Movie_Data_Lorenz/TPA-3rdplasmidconc1to1/tea4s15w_0_003080.tif", path "C:/Analysis_from_Movie_for_RiboTrap_Dieter/Movie_Data_Lorenz/TPA-3rdplasmidconc1to1/tea4s15w_0_003081.tif", path "C:/Analysis_from_Movie_for_RiboTrap_Dieter/Movie_Data_Lorenz/TPA-3rdplasmidconc1to1/tea4s15w_0_003082.tif", path "C:/Analysis_from_Movie_for_RiboTrap_Dieter/Movie_Data_Lorenz/TPA-3rdplasmidconc1to1/tea4s15w_0_003083.tif", path "C:/Analysis_from_Movie_for_RiboTrap_Dieter/Movie_Data_Lorenz/TPA-3rdplasmidconc1to1/tea4s15w_0_003084.tif", path "C:/Analysis_from_Movie_for_RiboTrap_Dieter/Movie_Data_Lorenz/TPA-3rdplasmidconc1to1/tea4s15w_0_003085.tif", path "C:/Analysis_from_Movie_for_RiboTrap_Dieter/Movie_Data_Lorenz/TPA-3rdplasmidconc1to1/tea4s15w_0_003086.tif", path "C:/Analysis_from_Movie_for_RiboTrap_Dieter/Movie_Data_Lorenz/TPA-3rdplasmidconc1to1/tea4s15w_0_003087.tif", path "C:/Analysis_from_Movie_for_RiboTrap_Dieter/Movie_Data_Lorenz/TPA-3rdplasmidconc1to1/tea4s15w_0_003088.tif", path "C:/Analysis_from_Movie_for_RiboTrap_Dieter/Movie_Data_Lorenz/TPA-3rdplasmidconc1to1/tea4s15w_0_003089.tif", path "C:/Analysis_from_Movie_for_RiboTrap_Dieter/Movie_Data_Lorenz/TPA-3rdplasmidconc1to1/tea4s15w_0_003090.tif", path "C:/Analysis_from_Movie_for_RiboTrap_Dieter/Movie_Data_Lorenz/TPA-3rdplasmidconc1to1/tea4s15w_0_003091.tif", path "C:/Analysis_from_Movie_for_RiboTrap_Dieter/Movie_Data_Lorenz/TPA-3rdplasmidconc1to1/tea4s15w_0_003092.tif", path "C:/Analysis_from_Movie_for_RiboTrap_Dieter/Movie_Data_Lorenz/TPA-3rdplasmidconc1to1/tea4s15w_0_003093.tif", path "C:/Analysis_from_Movie_for_RiboTrap_Dieter/Movie_Data_Lorenz/TPA-3rdplasmidconc1to1/tea4s15w_0_003094.tif", path "C:/Analysis_from_Movie_for_RiboTrap_Dieter/Movie_Data_Lorenz/TPA-3rdplasmidconc1to1/tea4s15w_0_003095.tif", path "C:/Analysis_from_Movie_for_RiboTrap_Dieter/Movie_Data_Lorenz/TPA-3rdplasmidconc1to1/tea4s15w_0_003096.tif", path "C:/Analysis_from_Movie_for_RiboTrap_Dieter/Movie_Data_Lorenz/TPA-3rdplasmidconc1to1/tea4s15w_0_003097.tif", path "C:/Analysis_from_Movie_for_RiboTrap_Dieter/Movie_Data_Lorenz/TPA-3rdplasmidconc1to1/tea4s15w_0_003098.tif", path "C:/Analysis_from_Movie_for_RiboTrap_Dieter/Movie_Data_Lorenz/TPA-3rdplasmidconc1to1/tea4s15w_0_003099.tif", path "C:/Analysis_from_Movie_for_RiboTrap_Dieter/Movie_Data_Lorenz/TPA-3rdplasmidconc1to1/tea4s15w_0_003100.tif", path "C:/Analysis_from_Movie_for_RiboTrap_Dieter/Movie_Data_Lorenz/TPA-3rdplasmidconc1to1/tea4s15w_0_003101.tif", path "C:/Analysis_from_Movie_for_RiboTrap_Dieter/Movie_Data_Lorenz/TPA-3rdplasmidconc1to1/tea4s15w_0_003102.tif", path "C:/Analysis_from_Movie_for_RiboTrap_Dieter/Movie_Data_Lorenz/TPA-3rdplasmidconc1to1/tea4s15w_0_003103.tif", path "C:/Analysis_from_Movie_for_RiboTrap_Dieter/Movie_Data_Lorenz/TPA-3rdplasmidconc1to1/tea4s15w_0_003104.tif", path "C:/Analysis_from_Movie_for_RiboTrap_Dieter/Movie_Data_Lorenz/TPA-3rdplasmidconc1to1/tea4s15w_0_003105.tif", path "C:/Analysis_from_Movie_for_RiboTrap_Dieter/Movie_Data_Lorenz/TPA-3rdplasmidconc1to1/tea4s15w_0_003106.tif", path "C:/Analysis_from_Movie_for_RiboTrap_Dieter/Movie_Data_Lorenz/TPA-3rdplasmidconc1to1/tea4s15w_0_003107.tif", path "C:/Analysis_from_Movie_for_RiboTrap_Dieter/Movie_Data_Lorenz/TPA-3rdplasmidconc1to1/tea4s15w_0_003108.tif", path "C:/Analysis_from_Movie_for_RiboTrap_Dieter/Movie_Data_Lorenz/TPA-3rdplasmidconc1to1/tea4s15w_0_003109.tif", path "C:/Analysis_from_Movie_for_RiboTrap_Dieter/Movie_Data_Lorenz/TPA-3rdplasmidconc1to1/tea4s15w_0_003110.tif", path "C:/Analysis_from_Movie_for_RiboTrap_Dieter/Movie_Data_Lorenz/TPA-3rdplasmidconc1to1/tea4s15w_0_003111.tif", path "C:/Analysis_from_Movie_for_RiboTrap_Dieter/Movie_Data_Lorenz/TPA-3rdplasmidconc1to1/tea4s15w_0_003112.tif", path "C:/Analysis_from_Movie_for_RiboTrap_Dieter/Movie_Data_Lorenz/TPA-3rdplasmidconc1to1/tea4s15w_0_003113.tif", path "C:/Analysis_from_Movie_for_RiboTrap_Dieter/Movie_Data_Lorenz/TPA-3rdplasmidconc1to1/tea4s15w_0_003114.tif", path "C:/Analysis_from_Movie_for_RiboTrap_Dieter/Movie_Data_Lorenz/TPA-3rdplasmidconc1to1/tea4s15w_0_003115.tif", path "C:/Analysis_from_Movie_for_RiboTrap_Dieter/Movie_Data_Lorenz/TPA-3rdplasmidconc1to1/tea4s15w_0_003116.tif", path "C:/Analysis_from_Movie_for_RiboTrap_Dieter/Movie_Data_Lorenz/TPA-3rdplasmidconc1to1/tea4s15w_0_003117.tif", path "C:/Analysis_from_Movie_for_RiboTrap_Dieter/Movie_Data_Lorenz/TPA-3rdplasmidconc1to1/tea4s15w_0_003118.tif", path "C:/Analysis_from_Movie_for_RiboTrap_Dieter/Movie_Data_Lorenz/TPA-3rdplasmidconc1to1/tea4s15w_0_003119.tif", path "C:/Analysis_from_Movie_for_RiboTrap_Dieter/Movie_Data_Lorenz/TPA-3rdplasmidconc1to1/tea4s15w_0_003120.tif", path "C:/Analysis_from_Movie_for_RiboTrap_Dieter/Movie_Data_Lorenz/TPA-3rdplasmidconc1to1/tea4s15w_0_003121.tif", path "C:/Analysis_from_Movie_for_RiboTrap_Dieter/Movie_Data_Lorenz/TPA-3rdplasmidconc1to1/tea4s15w_0_003122.tif", path "C:/Analysis_from_Movie_for_RiboTrap_Dieter/Movie_Data_Lorenz/TPA-3rdplasmidconc1to1/tea4s15w_0_003123.tif", path "C:/Analysis_from_Movie_for_RiboTrap_Dieter/Movie_Data_Lorenz/TPA-3rdplasmidconc1to1/tea4s15w_0_003124.tif", path "C:/Analysis_from_Movie_for_RiboTrap_Dieter/Movie_Data_Lorenz/TPA-3rdplasmidconc1to1/tea4s15w_0_003125.tif", path "C:/Analysis_from_Movie_for_RiboTrap_Dieter/Movie_Data_Lorenz/TPA-3rdplasmidconc1to1/tea4s15w_0_003126.tif", path "C:/Analysis_from_Movie_for_RiboTrap_Dieter/Movie_Data_Lorenz/TPA-3rdplasmidconc1to1/tea4s15w_0_003127.tif", path "C:/Analysis_from_Movie_for_RiboTrap_Dieter/Movie_Data_Lorenz/TPA-3rdplasmidconc1to1/tea4s15w_0_003128.tif", path "C:/Analysis_from_Movie_for_RiboTrap_Dieter/Movie_Data_Lorenz/TPA-3rdplasmidconc1to1/tea4s15w_0_003129.tif", path "C:/Analysis_from_Movie_for_RiboTrap_Dieter/Movie_Data_Lorenz/TPA-3rdplasmidconc1to1/tea4s15w_0_003130.tif", path "C:/Analysis_from_Movie_for_RiboTrap_Dieter/Movie_Data_Lorenz/TPA-3rdplasmidconc1to1/tea4s15w_0_003131.tif", path "C:/Analysis_from_Movie_for_RiboTrap_Dieter/Movie_Data_Lorenz/TPA-3rdplasmidconc1to1/tea4s15w_0_003132.tif", path "C:/Analysis_from_Movie_for_RiboTrap_Dieter/Movie_Data_Lorenz/TPA-3rdplasmidconc1to1/tea4s15w_0_003133.tif", path "C:/Analysis_from_Movie_for_RiboTrap_Dieter/Movie_Data_Lorenz/TPA-3rdplasmidconc1to1/tea4s15w_0_003134.tif", path "C:/Analysis_from_Movie_for_RiboTrap_Dieter/Movie_Data_Lorenz/TPA-3rdplasmidconc1to1/tea4s15w_0_003135.tif", path "C:/Analysis_from_Movie_for_RiboTrap_Dieter/Movie_Data_Lorenz/TPA-3rdplasmidconc1to1/tea4s15w_0_003136.tif", path "C:/Analysis_from_Movie_for_RiboTrap_Dieter/Movie_Data_Lorenz/TPA-3rdplasmidconc1to1/tea4s15w_0_003137.tif", path "C:/Analysis_from_Movie_for_RiboTrap_Dieter/Movie_Data_Lorenz/TPA-3rdplasmidconc1to1/tea4s15w_0_003138.tif", path "C:/Analysis_from_Movie_for_RiboTrap_Dieter/Movie_Data_Lorenz/TPA-3rdplasmidconc1to1/tea4s15w_0_003139.tif", path "C:/Analysis_from_Movie_for_RiboTrap_Dieter/Movie_Data_Lorenz/TPA-3rdplasmidconc1to1/tea4s15w_0_003140.tif", path "C:/Analysis_from_Movie_for_RiboTrap_Dieter/Movie_Data_Lorenz/TPA-3rdplasmidconc1to1/tea4s15w_0_003141.tif", path "C:/Analysis_from_Movie_for_RiboTrap_Dieter/Movie_Data_Lorenz/TPA-3rdplasmidconc1to1/tea4s15w_0_003142.tif", path "C:/Analysis_from_Movie_for_RiboTrap_Dieter/Movie_Data_Lorenz/TPA-3rdplasmidconc1to1/tea4s15w_0_003143.tif", path "C:/Analysis_from_Movie_for_RiboTrap_Dieter/Movie_Data_Lorenz/TPA-3rdplasmidconc1to1/tea4s15w_0_003144.tif", path "C:/Analysis_from_Movie_for_RiboTrap_Dieter/Movie_Data_Lorenz/TPA-3rdplasmidconc1to1/tea4s15w_0_003145.tif", path "C:/Analysis_from_Movie_for_RiboTrap_Dieter/Movie_Data_Lorenz/TPA-3rdplasmidconc1to1/tea4s15w_0_003146.tif", path "C:/Analysis_from_Movie_for_RiboTrap_Dieter/Movie_Data_Lorenz/TPA-3rdplasmidconc1to1/tea4s15w_0_003147.tif", path "C:/Analysis_from_Movie_for_RiboTrap_Dieter/Movie_Data_Lorenz/TPA-3rdplasmidconc1to1/tea4s15w_0_003148.tif", path "C:/Analysis_from_Movie_for_RiboTrap_Dieter/Movie_Data_Lorenz/TPA-3rdplasmidconc1to1/tea4s15w_0_003149.tif", path "C:/Analysis_from_Movie_for_RiboTrap_Dieter/Movie_Data_Lorenz/TPA-3rdplasmidconc1to1/tea4s15w_0_003150.tif", path "C:/Analysis_from_Movie_for_RiboTrap_Dieter/Movie_Data_Lorenz/TPA-3rdplasmidconc1to1/tea4s15w_0_003151.tif", path "C:/Analysis_from_Movie_for_RiboTrap_Dieter/Movie_Data_Lorenz/TPA-3rdplasmidconc1to1/tea4s15w_0_003152.tif", path "C:/Analysis_from_Movie_for_RiboTrap_Dieter/Movie_Data_Lorenz/TPA-3rdplasmidconc1to1/tea4s15w_0_003153.tif", path "C:/Analysis_from_Movie_for_RiboTrap_Dieter/Movie_Data_Lorenz/TPA-3rdplasmidconc1to1/tea4s15w_0_003154.tif", path "C:/Analysis_from_Movie_for_RiboTrap_Dieter/Movie_Data_Lorenz/TPA-3rdplasmidconc1to1/tea4s15w_0_003155.tif", path "C:/Analysis_from_Movie_for_RiboTrap_Dieter/Movie_Data_Lorenz/TPA-3rdplasmidconc1to1/tea4s15w_0_003156.tif", path "C:/Analysis_from_Movie_for_RiboTrap_Dieter/Movie_Data_Lorenz/TPA-3rdplasmidconc1to1/tea4s15w_0_003157.tif", path "C:/Analysis_from_Movie_for_RiboTrap_Dieter/Movie_Data_Lorenz/TPA-3rdplasmidconc1to1/tea4s15w_0_003158.tif", path "C:/Analysis_from_Movie_for_RiboTrap_Dieter/Movie_Data_Lorenz/TPA-3rdplasmidconc1to1/tea4s15w_0_003159.tif", path "C:/Analysis_from_Movie_for_RiboTrap_Dieter/Movie_Data_Lorenz/TPA-3rdplasmidconc1to1/tea4s15w_0_003160.tif", path "C:/Analysis_from_Movie_for_RiboTrap_Dieter/Movie_Data_Lorenz/TPA-3rdplasmidconc1to1/tea4s15w_0_003161.tif", path "C:/Analysis_from_Movie_for_RiboTrap_Dieter/Movie_Data_Lorenz/TPA-3rdplasmidconc1to1/tea4s15w_0_003162.tif", path "C:/Analysis_from_Movie_for_RiboTrap_Dieter/Movie_Data_Lorenz/TPA-3rdplasmidconc1to1/tea4s15w_0_003163.tif", path "C:/Analysis_from_Movie_for_RiboTrap_Dieter/Movie_Data_Lorenz/TPA-3rdplasmidconc1to1/tea4s15w_0_003164.tif", path "C:/Analysis_from_Movie_for_RiboTrap_Dieter/Movie_Data_Lorenz/TPA-3rdplasmidconc1to1/tea4s15w_0_003165.tif", path "C:/Analysis_from_Movie_for_RiboTrap_Dieter/Movie_Data_Lorenz/TPA-3rdplasmidconc1to1/tea4s15w_0_003166.tif", path "C:/Analysis_from_Movie_for_RiboTrap_Dieter/Movie_Data_Lorenz/TPA-3rdplasmidconc1to1/tea4s15w_0_003167.tif", path "C:/Analysis_from_Movie_for_RiboTrap_Dieter/Movie_Data_Lorenz/TPA-3rdplasmidconc1to1/tea4s15w_0_003168.tif", path "C:/Analysis_from_Movie_for_RiboTrap_Dieter/Movie_Data_Lorenz/TPA-3rdplasmidconc1to1/tea4s15w_0_003169.tif", path "C:/Analysis_from_Movie_for_RiboTrap_Dieter/Movie_Data_Lorenz/TPA-3rdplasmidconc1to1/tea4s15w_0_003170.tif", path "C:/Analysis_from_Movie_for_RiboTrap_Dieter/Movie_Data_Lorenz/TPA-3rdplasmidconc1to1/tea4s15w_0_003171.tif", path "C:/Analysis_from_Movie_for_RiboTrap_Dieter/Movie_Data_Lorenz/TPA-3rdplasmidconc1to1/tea4s15w_0_003172.tif", path "C:/Analysis_from_Movie_for_RiboTrap_Dieter/Movie_Data_Lorenz/TPA-3rdplasmidconc1to1/tea4s15w_0_003173.tif", path "C:/Analysis_from_Movie_for_RiboTrap_Dieter/Movie_Data_Lorenz/TPA-3rdplasmidconc1to1/tea4s15w_0_003174.tif", path "C:/Analysis_from_Movie_for_RiboTrap_Dieter/Movie_Data_Lorenz/TPA-3rdplasmidconc1to1/tea4s15w_0_003175.tif", path "C:/Analysis_from_Movie_for_RiboTrap_Dieter/Movie_Data_Lorenz/TPA-3rdplasmidconc1to1/tea4s15w_0_003176.tif", path "C:/Analysis_from_Movie_for_RiboTrap_Dieter/Movie_Data_Lorenz/TPA-3rdplasmidconc1to1/tea4s15w_0_003177.tif", path "C:/Analysis_from_Movie_for_RiboTrap_Dieter/Movie_Data_Lorenz/TPA-3rdplasmidconc1to1/tea4s15w_0_003178.tif", path "C:/Analysis_from_Movie_for_RiboTrap_Dieter/Movie_Data_Lorenz/TPA-3rdplasmidconc1to1/tea4s15w_0_003179.tif", path "C:/Analysis_from_Movie_for_RiboTrap_Dieter/Movie_Data_Lorenz/TPA-3rdplasmidconc1to1/tea4s15w_0_003180.tif", path "C:/Analysis_from_Movie_for_RiboTrap_Dieter/Movie_Data_Lorenz/TPA-3rdplasmidconc1to1/tea4s15w_0_003181.tif", path "C:/Analysis_from_Movie_for_RiboTrap_Dieter/Movie_Data_Lorenz/TPA-3rdplasmidconc1to1/tea4s15w_0_003182.tif", path "C:/Analysis_from_Movie_for_RiboTrap_Dieter/Movie_Data_Lorenz/TPA-3rdplasmidconc1to1/tea4s15w_0_003183.tif", path "C:/Analysis_from_Movie_for_RiboTrap_Dieter/Movie_Data_Lorenz/TPA-3rdplasmidconc1to1/tea4s15w_0_003184.tif", path "C:/Analysis_from_Movie_for_RiboTrap_Dieter/Movie_Data_Lorenz/TPA-3rdplasmidconc1to1/tea4s15w_0_003185.tif", path "C:/Analysis_from_Movie_for_RiboTrap_Dieter/Movie_Data_Lorenz/TPA-3rdplasmidconc1to1/tea4s15w_0_003186.tif", path "C:/Analysis_from_Movie_for_RiboTrap_Dieter/Movie_Data_Lorenz/TPA-3rdplasmidconc1to1/tea4s15w_0_003187.tif", path "C:/Analysis_from_Movie_for_RiboTrap_Dieter/Movie_Data_Lorenz/TPA-3rdplasmidconc1to1/tea4s15w_0_003188.tif", path "C:/Analysis_from_Movie_for_RiboTrap_Dieter/Movie_Data_Lorenz/TPA-3rdplasmidconc1to1/tea4s15w_0_003189.tif", path "C:/Analysis_from_Movie_for_RiboTrap_Dieter/Movie_Data_Lorenz/TPA-3rdplasmidconc1to1/tea4s15w_0_003190.tif", path "C:/Analysis_from_Movie_for_RiboTrap_Dieter/Movie_Data_Lorenz/TPA-3rdplasmidconc1to1/tea4s15w_0_003191.tif", path "C:/Analysis_from_Movie_for_RiboTrap_Dieter/Movie_Data_Lorenz/TPA-3rdplasmidconc1to1/tea4s15w_0_003192.tif", path "C:/Analysis_from_Movie_for_RiboTrap_Dieter/Movie_Data_Lorenz/TPA-3rdplasmidconc1to1/tea4s15w_0_003193.tif", path "C:/Analysis_from_Movie_for_RiboTrap_Dieter/Movie_Data_Lorenz/TPA-3rdplasmidconc1to1/tea4s15w_0_003194.tif", path "C:/Analysis_from_Movie_for_RiboTrap_Dieter/Movie_Data_Lorenz/TPA-3rdplasmidconc1to1/tea4s15w_0_003195.tif", path "C:/Analysis_from_Movie_for_RiboTrap_Dieter/Movie_Data_Lorenz/TPA-3rdplasmidconc1to1/tea4s15w_0_003196.tif", path "C:/Analysis_from_Movie_for_RiboTrap_Dieter/Movie_Data_Lorenz/TPA-3rdplasmidconc1to1/tea4s15w_0_003197.tif", path "C:/Analysis_from_Movie_for_RiboTrap_Dieter/Movie_Data_Lorenz/TPA-3rdplasmidconc1to1/tea4s15w_0_003198.tif", path "C:/Analysis_from_Movie_for_RiboTrap_Dieter/Movie_Data_Lorenz/TPA-3rdplasmidconc1to1/tea4s15w_0_003199.tif", path "C:/Analysis_from_Movie_for_RiboTrap_Dieter/Movie_Data_Lorenz/TPA-3rdplasmidconc1to1/tea4s15w_0_003200.tif", path "C:/Analysis_from_Movie_for_RiboTrap_Dieter/Movie_Data_Lorenz/TPA-3rdplasmidconc1to1/tea4s15w_0_003201.tif", path "C:/Analysis_from_Movie_for_RiboTrap_Dieter/Movie_Data_Lorenz/TPA-3rdplasmidconc1to1/tea4s15w_0_003202.tif", path "C:/Analysis_from_Movie_for_RiboTrap_Dieter/Movie_Data_Lorenz/TPA-3rdplasmidconc1to1/tea4s15w_0_003203.tif", path "C:/Analysis_from_Movie_for_RiboTrap_Dieter/Movie_Data_Lorenz/TPA-3rdplasmidconc1to1/tea4s15w_0_003204.tif", path "C:/Analysis_from_Movie_for_RiboTrap_Dieter/Movie_Data_Lorenz/TPA-3rdplasmidconc1to1/tea4s15w_0_003205.tif", path "C:/Analysis_from_Movie_for_RiboTrap_Dieter/Movie_Data_Lorenz/TPA-3rdplasmidconc1to1/tea4s15w_0_003206.tif", path "C:/Analysis_from_Movie_for_RiboTrap_Dieter/Movie_Data_Lorenz/TPA-3rdplasmidconc1to1/tea4s15w_0_003207.tif", path "C:/Analysis_from_Movie_for_RiboTrap_Dieter/Movie_Data_Lorenz/TPA-3rdplasmidconc1to1/tea4s15w_0_003208.tif", path "C:/Analysis_from_Movie_for_RiboTrap_Dieter/Movie_Data_Lorenz/TPA-3rdplasmidconc1to1/tea4s15w_0_003209.tif", path "C:/Analysis_from_Movie_for_RiboTrap_Dieter/Movie_Data_Lorenz/TPA-3rdplasmidconc1to1/tea4s15w_0_003210.tif", path "C:/Analysis_from_Movie_for_RiboTrap_Dieter/Movie_Data_Lorenz/TPA-3rdplasmidconc1to1/tea4s15w_0_003211.tif", path "C:/Analysis_from_Movie_for_RiboTrap_Dieter/Movie_Data_Lorenz/TPA-3rdplasmidconc1to1/tea4s15w_0_003212.tif", path "C:/Analysis_from_Movie_for_RiboTrap_Dieter/Movie_Data_Lorenz/TPA-3rdplasmidconc1to1/tea4s15w_0_003213.tif", path "C:/Analysis_from_Movie_for_RiboTrap_Dieter/Movie_Data_Lorenz/TPA-3rdplasmidconc1to1/tea4s15w_0_003214.tif", path "C:/Analysis_from_Movie_for_RiboTrap_Dieter/Movie_Data_Lorenz/TPA-3rdplasmidconc1to1/tea4s15w_0_003215.tif", path "C:/Analysis_from_Movie_for_RiboTrap_Dieter/Movie_Data_Lorenz/TPA-3rdplasmidconc1to1/tea4s15w_0_003216.tif", path "C:/Analysis_from_Movie_for_RiboTrap_Dieter/Movie_Data_Lorenz/TPA-3rdplasmidconc1to1/tea4s15w_0_003217.tif", path "C:/Analysis_from_Movie_for_RiboTrap_Dieter/Movie_Data_Lorenz/TPA-3rdplasmidconc1to1/tea4s15w_0_003218.tif", path "C:/Analysis_from_Movie_for_RiboTrap_Dieter/Movie_Data_Lorenz/TPA-3rdplasmidconc1to1/tea4s15w_0_003219.tif", path "C:/Analysis_from_Movie_for_RiboTrap_Dieter/Movie_Data_Lorenz/TPA-3rdplasmidconc1to1/tea4s15w_0_003220.tif", path "C:/Analysis_from_Movie_for_RiboTrap_Dieter/Movie_Data_Lorenz/TPA-3rdplasmidconc1to1/tea4s15w_0_003221.tif", path "C:/Analysis_from_Movie_for_RiboTrap_Dieter/Movie_Data_Lorenz/TPA-3rdplasmidconc1to1/tea4s15w_0_003222.tif", path "C:/Analysis_from_Movie_for_RiboTrap_Dieter/Movie_Data_Lorenz/TPA-3rdplasmidconc1to1/tea4s15w_0_003223.tif", path "C:/Analysis_from_Movie_for_RiboTrap_Dieter/Movie_Data_Lorenz/TPA-3rdplasmidconc1to1/tea4s15w_0_003224.tif", path "C:/Analysis_from_Movie_for_RiboTrap_Dieter/Movie_Data_Lorenz/TPA-3rdplasmidconc1to1/tea4s15w_0_003225.tif", path "C:/Analysis_from_Movie_for_RiboTrap_Dieter/Movie_Data_Lorenz/TPA-3rdplasmidconc1to1/tea4s15w_0_003226.tif", path "C:/Analysis_from_Movie_for_RiboTrap_Dieter/Movie_Data_Lorenz/TPA-3rdplasmidconc1to1/tea4s15w_0_003227.tif", path "C:/Analysis_from_Movie_for_RiboTrap_Dieter/Movie_Data_Lorenz/TPA-3rdplasmidconc1to1/tea4s15w_0_003228.tif", path "C:/Analysis_from_Movie_for_RiboTrap_Dieter/Movie_Data_Lorenz/TPA-3rdplasmidconc1to1/tea4s15w_0_003229.tif", path "C:/Analysis_from_Movie_for_RiboTrap_Dieter/Movie_Data_Lorenz/TPA-3rdplasmidconc1to1/tea4s15w_0_003230.tif", path "C:/Analysis_from_Movie_for_RiboTrap_Dieter/Movie_Data_Lorenz/TPA-3rdplasmidconc1to1/tea4s15w_0_003231.tif", path "C:/Analysis_from_Movie_for_RiboTrap_Dieter/Movie_Data_Lorenz/TPA-3rdplasmidconc1to1/tea4s15w_0_003232.tif", path "C:/Analysis_from_Movie_for_RiboTrap_Dieter/Movie_Data_Lorenz/TPA-3rdplasmidconc1to1/tea4s15w_0_003233.tif", path "C:/Analysis_from_Movie_for_RiboTrap_Dieter/Movie_Data_Lorenz/TPA-3rdplasmidconc1to1/tea4s15w_0_003234.tif", path "C:/Analysis_from_Movie_for_RiboTrap_Dieter/Movie_Data_Lorenz/TPA-3rdplasmidconc1to1/tea4s15w_0_003235.tif", path "C:/Analysis_from_Movie_for_RiboTrap_Dieter/Movie_Data_Lorenz/TPA-3rdplasmidconc1to1/tea4s15w_0_003236.tif", path "C:/Analysis_from_Movie_for_RiboTrap_Dieter/Movie_Data_Lorenz/TPA-3rdplasmidconc1to1/tea4s15w_0_003237.tif", path "C:/Analysis_from_Movie_for_RiboTrap_Dieter/Movie_Data_Lorenz/TPA-3rdplasmidconc1to1/tea4s15w_0_003238.tif", path "C:/Analysis_from_Movie_for_RiboTrap_Dieter/Movie_Data_Lorenz/TPA-3rdplasmidconc1to1/tea4s15w_0_003239.tif", path "C:/Analysis_from_Movie_for_RiboTrap_Dieter/Movie_Data_Lorenz/TPA-3rdplasmidconc1to1/tea4s15w_0_003240.tif", path "C:/Analysis_from_Movie_for_RiboTrap_Dieter/Movie_Data_Lorenz/TPA-3rdplasmidconc1to1/tea4s15w_0_003241.tif", path "C:/Analysis_from_Movie_for_RiboTrap_Dieter/Movie_Data_Lorenz/TPA-3rdplasmidconc1to1/tea4s15w_0_003242.tif", path "C:/Analysis_from_Movie_for_RiboTrap_Dieter/Movie_Data_Lorenz/TPA-3rdplasmidconc1to1/tea4s15w_0_003243.tif", path "C:/Analysis_from_Movie_for_RiboTrap_Dieter/Movie_Data_Lorenz/TPA-3rdplasmidconc1to1/tea4s15w_0_003244.tif", path "C:/Analysis_from_Movie_for_RiboTrap_Dieter/Movie_Data_Lorenz/TPA-3rdplasmidconc1to1/tea4s15w_0_003245.tif", path "C:/Analysis_from_Movie_for_RiboTrap_Dieter/Movie_Data_Lorenz/TPA-3rdplasmidconc1to1/tea4s15w_0_003246.tif", path "C:/Analysis_from_Movie_for_RiboTrap_Dieter/Movie_Data_Lorenz/TPA-3rdplasmidconc1to1/tea4s15w_0_003247.tif", path "C:/Analysis_from_Movie_for_RiboTrap_Dieter/Movie_Data_Lorenz/TPA-3rdplasmidconc1to1/tea4s15w_0_003248.tif", path "C:/Analysis_from_Movie_for_RiboTrap_Dieter/Movie_Data_Lorenz/TPA-3rdplasmidconc1to1/tea4s15w_0_003249.tif", path "C:/Analysis_from_Movie_for_RiboTrap_Dieter/Movie_Data_Lorenz/TPA-3rdplasmidconc1to1/tea4s15w_0_003250.tif", path "C:/Analysis_from_Movie_for_RiboTrap_Dieter/Movie_Data_Lorenz/TPA-3rdplasmidconc1to1/tea4s15w_0_003251.tif", path "C:/Analysis_from_Movie_for_RiboTrap_Dieter/Movie_Data_Lorenz/TPA-3rdplasmidconc1to1/tea4s15w_0_003252.tif", path "C:/Analysis_from_Movie_for_RiboTrap_Dieter/Movie_Data_Lorenz/TPA-3rdplasmidconc1to1/tea4s15w_0_003253.tif", path "C:/Analysis_from_Movie_for_RiboTrap_Dieter/Movie_Data_Lorenz/TPA-3rdplasmidconc1to1/tea4s15w_0_003254.tif", path "C:/Analysis_from_Movie_for_RiboTrap_Dieter/Movie_Data_Lorenz/TPA-3rdplasmidconc1to1/tea4s15w_0_003255.tif", path "C:/Analysis_from_Movie_for_RiboTrap_Dieter/Movie_Data_Lorenz/TPA-3rdplasmidconc1to1/tea4s15w_0_003256.tif", path "C:/Analysis_from_Movie_for_RiboTrap_Dieter/Movie_Data_Lorenz/TPA-3rdplasmidconc1to1/tea4s15w_0_003257.tif", path "C:/Analysis_from_Movie_for_RiboTrap_Dieter/Movie_Data_Lorenz/TPA-3rdplasmidconc1to1/tea4s15w_0_003258.tif", path "C:/Analysis_from_Movie_for_RiboTrap_Dieter/Movie_Data_Lorenz/TPA-3rdplasmidconc1to1/tea4s15w_0_003259.tif", path "C:/Analysis_from_Movie_for_RiboTrap_Dieter/Movie_Data_Lorenz/TPA-3rdplasmidconc1to1/tea4s15w_0_003260.tif", path "C:/Analysis_from_Movie_for_RiboTrap_Dieter/Movie_Data_Lorenz/TPA-3rdplasmidconc1to1/tea4s15w_0_003261.tif", path "C:/Analysis_from_Movie_for_RiboTrap_Dieter/Movie_Data_Lorenz/TPA-3rdplasmidconc1to1/tea4s15w_0_003262.tif", path "C:/Analysis_from_Movie_for_RiboTrap_Dieter/Movie_Data_Lorenz/TPA-3rdplasmidconc1to1/tea4s15w_0_003263.tif", path "C:/Analysis_from_Movie_for_RiboTrap_Dieter/Movie_Data_Lorenz/TPA-3rdplasmidconc1to1/tea4s15w_0_003264.tif", path "C:/Analysis_from_Movie_for_RiboTrap_Dieter/Movie_Data_Lorenz/TPA-3rdplasmidconc1to1/tea4s15w_0_003265.tif", path "C:/Analysis_from_Movie_for_RiboTrap_Dieter/Movie_Data_Lorenz/TPA-3rdplasmidconc1to1/tea4s15w_0_003266.tif", path "C:/Analysis_from_Movie_for_RiboTrap_Dieter/Movie_Data_Lorenz/TPA-3rdplasmidconc1to1/tea4s15w_0_003267.tif", path "C:/Analysis_from_Movie_for_RiboTrap_Dieter/Movie_Data_Lorenz/TPA-3rdplasmidconc1to1/tea4s15w_0_003268.tif", path "C:/Analysis_from_Movie_for_RiboTrap_Dieter/Movie_Data_Lorenz/TPA-3rdplasmidconc1to1/tea4s15w_0_003269.tif", path "C:/Analysis_from_Movie_for_RiboTrap_Dieter/Movie_Data_Lorenz/TPA-3rdplasmidconc1to1/tea4s15w_0_003270.tif", path "C:/Analysis_from_Movie_for_RiboTrap_Dieter/Movie_Data_Lorenz/TPA-3rdplasmidconc1to1/tea4s15w_0_003271.tif", path "C:/Analysis_from_Movie_for_RiboTrap_Dieter/Movie_Data_Lorenz/TPA-3rdplasmidconc1to1/tea4s15w_0_003272.tif", path "C:/Analysis_from_Movie_for_RiboTrap_Dieter/Movie_Data_Lorenz/TPA-3rdplasmidconc1to1/tea4s15w_0_003273.tif", path "C:/Analysis_from_Movie_for_RiboTrap_Dieter/Movie_Data_Lorenz/TPA-3rdplasmidconc1to1/tea4s15w_0_003274.tif", path "C:/Analysis_from_Movie_for_RiboTrap_Dieter/Movie_Data_Lorenz/TPA-3rdplasmidconc1to1/tea4s15w_0_003275.tif", path "C:/Analysis_from_Movie_for_RiboTrap_Dieter/Movie_Data_Lorenz/TPA-3rdplasmidconc1to1/tea4s15w_0_003276.tif", path "C:/Analysis_from_Movie_for_RiboTrap_Dieter/Movie_Data_Lorenz/TPA-3rdplasmidconc1to1/tea4s15w_0_003277.tif", path "C:/Analysis_from_Movie_for_RiboTrap_Dieter/Movie_Data_Lorenz/TPA-3rdplasmidconc1to1/tea4s15w_0_003278.tif", path "C:/Analysis_from_Movie_for_RiboTrap_Dieter/Movie_Data_Lorenz/TPA-3rdplasmidconc1to1/tea4s15w_0_003279.tif", path "C:/Analysis_from_Movie_for_RiboTrap_Dieter/Movie_Data_Lorenz/TPA-3rdplasmidconc1to1/tea4s15w_0_003280.tif", path "C:/Analysis_from_Movie_for_RiboTrap_Dieter/Movie_Data_Lorenz/TPA-3rdplasmidconc1to1/tea4s15w_0_003281.tif", path "C:/Analysis_from_Movie_for_RiboTrap_Dieter/Movie_Data_Lorenz/TPA-3rdplasmidconc1to1/tea4s15w_0_003282.tif", path "C:/Analysis_from_Movie_for_RiboTrap_Dieter/Movie_Data_Lorenz/TPA-3rdplasmidconc1to1/tea4s15w_0_003283.tif", path "C:/Analysis_from_Movie_for_RiboTrap_Dieter/Movie_Data_Lorenz/TPA-3rdplasmidconc1to1/tea4s15w_0_003284.tif", path "C:/Analysis_from_Movie_for_RiboTrap_Dieter/Movie_Data_Lorenz/TPA-3rdplasmidconc1to1/tea4s15w_0_003285.tif", path "C:/Analysis_from_Movie_for_RiboTrap_Dieter/Movie_Data_Lorenz/TPA-3rdplasmidconc1to1/tea4s15w_0_003286.tif", path "C:/Analysis_from_Movie_for_RiboTrap_Dieter/Movie_Data_Lorenz/TPA-3rdplasmidconc1to1/tea4s15w_0_003287.tif", path "C:/Analysis_from_Movie_for_RiboTrap_Dieter/Movie_Data_Lorenz/TPA-3rdplasmidconc1to1/tea4s15w_0_003288.tif", path "C:/Analysis_from_Movie_for_RiboTrap_Dieter/Movie_Data_Lorenz/TPA-3rdplasmidconc1to1/tea4s15w_0_003289.tif", path "C:/Analysis_from_Movie_for_RiboTrap_Dieter/Movie_Data_Lorenz/TPA-3rdplasmidconc1to1/tea4s15w_0_003290.tif", path "C:/Analysis_from_Movie_for_RiboTrap_Dieter/Movie_Data_Lorenz/TPA-3rdplasmidconc1to1/tea4s15w_0_003291.tif", path "C:/Analysis_from_Movie_for_RiboTrap_Dieter/Movie_Data_Lorenz/TPA-3rdplasmidconc1to1/tea4s15w_0_003292.tif", path "C:/Analysis_from_Movie_for_RiboTrap_Dieter/Movie_Data_Lorenz/TPA-3rdplasmidconc1to1/tea4s15w_0_003293.tif", path "C:/Analysis_from_Movie_for_RiboTrap_Dieter/Movie_Data_Lorenz/TPA-3rdplasmidconc1to1/tea4s15w_0_003294.tif", path "C:/Analysis_from_Movie_for_RiboTrap_Dieter/Movie_Data_Lorenz/TPA-3rdplasmidconc1to1/tea4s15w_0_003295.tif", path "C:/Analysis_from_Movie_for_RiboTrap_Dieter/Movie_Data_Lorenz/TPA-3rdplasmidconc1to1/tea4s15w_0_003296.tif", path "C:/Analysis_from_Movie_for_RiboTrap_Dieter/Movie_Data_Lorenz/TPA-3rdplasmidconc1to1/tea4s15w_0_003297.tif", path "C:/Analysis_from_Movie_for_RiboTrap_Dieter/Movie_Data_Lorenz/TPA-3rdplasmidconc1to1/tea4s15w_0_003298.tif", path "C:/Analysis_from_Movie_for_RiboTrap_Dieter/Movie_Data_Lorenz/TPA-3rdplasmidconc1to1/tea4s15w_0_003299.tif", path "C:/Analysis_from_Movie_for_RiboTrap_Dieter/Movie_Data_Lorenz/TPA-3rdplasmidconc1to1/tea4s15w_0_003300.tif", path "C:/Analysis_from_Movie_for_RiboTrap_Dieter/Movie_Data_Lorenz/TPA-3rdplasmidconc1to1/tea4s15w_0_003301.tif", path "C:/Analysis_from_Movie_for_RiboTrap_Dieter/Movie_Data_Lorenz/TPA-3rdplasmidconc1to1/tea4s15w_0_003302.tif", path "C:/Analysis_from_Movie_for_RiboTrap_Dieter/Movie_Data_Lorenz/TPA-3rdplasmidconc1to1/tea4s15w_0_003303.tif", path "C:/Analysis_from_Movie_for_RiboTrap_Dieter/Movie_Data_Lorenz/TPA-3rdplasmidconc1to1/tea4s15w_0_003304.tif", path "C:/Analysis_from_Movie_for_RiboTrap_Dieter/Movie_Data_Lorenz/TPA-3rdplasmidconc1to1/tea4s15w_0_003305.tif", path "C:/Analysis_from_Movie_for_RiboTrap_Dieter/Movie_Data_Lorenz/TPA-3rdplasmidconc1to1/tea4s15w_0_003306.tif", path "C:/Analysis_from_Movie_for_RiboTrap_Dieter/Movie_Data_Lorenz/TPA-3rdplasmidconc1to1/tea4s15w_0_003307.tif", path "C:/Analysis_from_Movie_for_RiboTrap_Dieter/Movie_Data_Lorenz/TPA-3rdplasmidconc1to1/tea4s15w_0_003308.tif", path "C:/Analysis_from_Movie_for_RiboTrap_Dieter/Movie_Data_Lorenz/TPA-3rdplasmidconc1to1/tea4s15w_0_003309.tif", path "C:/Analysis_from_Movie_for_RiboTrap_Dieter/Movie_Data_Lorenz/TPA-3rdplasmidconc1to1/tea4s15w_0_003310.tif", path "C:/Analysis_from_Movie_for_RiboTrap_Dieter/Movie_Data_Lorenz/TPA-3rdplasmidconc1to1/tea4s15w_0_003311.tif", path "C:/Analysis_from_Movie_for_RiboTrap_Dieter/Movie_Data_Lorenz/TPA-3rdplasmidconc1to1/tea4s15w_0_003312.tif", path "C:/Analysis_from_Movie_for_RiboTrap_Dieter/Movie_Data_Lorenz/TPA-3rdplasmidconc1to1/tea4s15w_0_003313.tif", path "C:/Analysis_from_Movie_for_RiboTrap_Dieter/Movie_Data_Lorenz/TPA-3rdplasmidconc1to1/tea4s15w_0_003314.tif", path "C:/Analysis_from_Movie_for_RiboTrap_Dieter/Movie_Data_Lorenz/TPA-3rdplasmidconc1to1/tea4s15w_0_003315.tif", path "C:/Analysis_from_Movie_for_RiboTrap_Dieter/Movie_Data_Lorenz/TPA-3rdplasmidconc1to1/tea4s15w_0_003316.tif", path "C:/Analysis_from_Movie_for_RiboTrap_Dieter/Movie_Data_Lorenz/TPA-3rdplasmidconc1to1/tea4s15w_0_003317.tif", path "C:/Analysis_from_Movie_for_RiboTrap_Dieter/Movie_Data_Lorenz/TPA-3rdplasmidconc1to1/tea4s15w_0_003318.tif", path "C:/Analysis_from_Movie_for_RiboTrap_Dieter/Movie_Data_Lorenz/TPA-3rdplasmidconc1to1/tea4s15w_0_003319.tif", path "C:/Analysis_from_Movie_for_RiboTrap_Dieter/Movie_Data_Lorenz/TPA-3rdplasmidconc1to1/tea4s15w_0_003320.tif", path "C:/Analysis_from_Movie_for_RiboTrap_Dieter/Movie_Data_Lorenz/TPA-3rdplasmidconc1to1/tea4s15w_0_003321.tif", path "C:/Analysis_from_Movie_for_RiboTrap_Dieter/Movie_Data_Lorenz/TPA-3rdplasmidconc1to1/tea4s15w_0_003322.tif", path "C:/Analysis_from_Movie_for_RiboTrap_Dieter/Movie_Data_Lorenz/TPA-3rdplasmidconc1to1/tea4s15w_0_003323.tif", path "C:/Analysis_from_Movie_for_RiboTrap_Dieter/Movie_Data_Lorenz/TPA-3rdplasmidconc1to1/tea4s15w_0_003324.tif", path "C:/Analysis_from_Movie_for_RiboTrap_Dieter/Movie_Data_Lorenz/TPA-3rdplasmidconc1to1/tea4s15w_0_003325.tif", path "C:/Analysis_from_Movie_for_RiboTrap_Dieter/Movie_Data_Lorenz/TPA-3rdplasmidconc1to1/tea4s15w_0_003326.tif", path "C:/Analysis_from_Movie_for_RiboTrap_Dieter/Movie_Data_Lorenz/TPA-3rdplasmidconc1to1/tea4s15w_0_003327.tif", path "C:/Analysis_from_Movie_for_RiboTrap_Dieter/Movie_Data_Lorenz/TPA-3rdplasmidconc1to1/tea4s15w_0_003328.tif", path "C:/Analysis_from_Movie_for_RiboTrap_Dieter/Movie_Data_Lorenz/TPA-3rdplasmidconc1to1/tea4s15w_0_003329.tif", path "C:/Analysis_from_Movie_for_RiboTrap_Dieter/Movie_Data_Lorenz/TPA-3rdplasmidconc1to1/tea4s15w_0_003330.tif", path "C:/Analysis_from_Movie_for_RiboTrap_Dieter/Movie_Data_Lorenz/TPA-3rdplasmidconc1to1/tea4s15w_0_003331.tif", path "C:/Analysis_from_Movie_for_RiboTrap_Dieter/Movie_Data_Lorenz/TPA-3rdplasmidconc1to1/tea4s15w_0_003332.tif", path "C:/Analysis_from_Movie_for_RiboTrap_Dieter/Movie_Data_Lorenz/TPA-3rdplasmidconc1to1/tea4s15w_0_003333.tif", path "C:/Analysis_from_Movie_for_RiboTrap_Dieter/Movie_Data_Lorenz/TPA-3rdplasmidconc1to1/tea4s15w_0_003334.tif", path "C:/Analysis_from_Movie_for_RiboTrap_Dieter/Movie_Data_Lorenz/TPA-3rdplasmidconc1to1/tea4s15w_0_003335.tif", path "C:/Analysis_from_Movie_for_RiboTrap_Dieter/Movie_Data_Lorenz/TPA-3rdplasmidconc1to1/tea4s15w_0_003336.tif", path "C:/Analysis_from_Movie_for_RiboTrap_Dieter/Movie_Data_Lorenz/TPA-3rdplasmidconc1to1/tea4s15w_0_003337.tif", path "C:/Analysis_from_Movie_for_RiboTrap_Dieter/Movie_Data_Lorenz/TPA-3rdplasmidconc1to1/tea4s15w_0_003338.tif", path "C:/Analysis_from_Movie_for_RiboTrap_Dieter/Movie_Data_Lorenz/TPA-3rdplasmidconc1to1/tea4s15w_0_003339.tif", path "C:/Analysis_from_Movie_for_RiboTrap_Dieter/Movie_Data_Lorenz/TPA-3rdplasmidconc1to1/tea4s15w_0_003340.tif", path "C:/Analysis_from_Movie_for_RiboTrap_Dieter/Movie_Data_Lorenz/TPA-3rdplasmidconc1to1/tea4s15w_0_003341.tif", path "C:/Analysis_from_Movie_for_RiboTrap_Dieter/Movie_Data_Lorenz/TPA-3rdplasmidconc1to1/tea4s15w_0_003342.tif", path "C:/Analysis_from_Movie_for_RiboTrap_Dieter/Movie_Data_Lorenz/TPA-3rdplasmidconc1to1/tea4s15w_0_003343.tif", path "C:/Analysis_from_Movie_for_RiboTrap_Dieter/Movie_Data_Lorenz/TPA-3rdplasmidconc1to1/tea4s15w_0_003344.tif", path "C:/Analysis_from_Movie_for_RiboTrap_Dieter/Movie_Data_Lorenz/TPA-3rdplasmidconc1to1/tea4s15w_0_003345.tif", path "C:/Analysis_from_Movie_for_RiboTrap_Dieter/Movie_Data_Lorenz/TPA-3rdplasmidconc1to1/tea4s15w_0_003346.tif", path "C:/Analysis_from_Movie_for_RiboTrap_Dieter/Movie_Data_Lorenz/TPA-3rdplasmidconc1to1/tea4s15w_0_003347.tif", path "C:/Analysis_from_Movie_for_RiboTrap_Dieter/Movie_Data_Lorenz/TPA-3rdplasmidconc1to1/tea4s15w_0_003348.tif", path "C:/Analysis_from_Movie_for_RiboTrap_Dieter/Movie_Data_Lorenz/TPA-3rdplasmidconc1to1/tea4s15w_0_003349.tif", path "C:/Analysis_from_Movie_for_RiboTrap_Dieter/Movie_Data_Lorenz/TPA-3rdplasmidconc1to1/tea4s15w_0_003350.tif", path "C:/Analysis_from_Movie_for_RiboTrap_Dieter/Movie_Data_Lorenz/TPA-3rdplasmidconc1to1/tea4s15w_0_003351.tif", path "C:/Analysis_from_Movie_for_RiboTrap_Dieter/Movie_Data_Lorenz/TPA-3rdplasmidconc1to1/tea4s15w_0_003352.tif", path "C:/Analysis_from_Movie_for_RiboTrap_Dieter/Movie_Data_Lorenz/TPA-3rdplasmidconc1to1/tea4s15w_0_003353.tif", path "C:/Analysis_from_Movie_for_RiboTrap_Dieter/Movie_Data_Lorenz/TPA-3rdplasmidconc1to1/tea4s15w_0_003354.tif", path "C:/Analysis_from_Movie_for_RiboTrap_Dieter/Movie_Data_Lorenz/TPA-3rdplasmidconc1to1/tea4s15w_0_003355.tif", path "C:/Analysis_from_Movie_for_RiboTrap_Dieter/Movie_Data_Lorenz/TPA-3rdplasmidconc1to1/tea4s15w_0_003356.tif", path "C:/Analysis_from_Movie_for_RiboTrap_Dieter/Movie_Data_Lorenz/TPA-3rdplasmidconc1to1/tea4s15w_0_003357.tif", path "C:/Analysis_from_Movie_for_RiboTrap_Dieter/Movie_Data_Lorenz/TPA-3rdplasmidconc1to1/tea4s15w_0_003358.tif", path "C:/Analysis_from_Movie_for_RiboTrap_Dieter/Movie_Data_Lorenz/TPA-3rdplasmidconc1to1/tea4s15w_0_003359.tif", path "C:/Analysis_from_Movie_for_RiboTrap_Dieter/Movie_Data_Lorenz/TPA-3rdplasmidconc1to1/tea4s15w_0_003360.tif", path "C:/Analysis_from_Movie_for_RiboTrap_Dieter/Movie_Data_Lorenz/TPA-3rdplasmidconc1to1/tea4s15w_0_003361.tif", path "C:/Analysis_from_Movie_for_RiboTrap_Dieter/Movie_Data_Lorenz/TPA-3rdplasmidconc1to1/tea4s15w_0_003362.tif", path "C:/Analysis_from_Movie_for_RiboTrap_Dieter/Movie_Data_Lorenz/TPA-3rdplasmidconc1to1/tea4s15w_0_003363.tif", path "C:/Analysis_from_Movie_for_RiboTrap_Dieter/Movie_Data_Lorenz/TPA-3rdplasmidconc1to1/tea4s15w_0_003364.tif", path "C:/Analysis_from_Movie_for_RiboTrap_Dieter/Movie_Data_Lorenz/TPA-3rdplasmidconc1to1/tea4s15w_0_003365.tif", path "C:/Analysis_from_Movie_for_RiboTrap_Dieter/Movie_Data_Lorenz/TPA-3rdplasmidconc1to1/tea4s15w_0_003366.tif", path "C:/Analysis_from_Movie_for_RiboTrap_Dieter/Movie_Data_Lorenz/TPA-3rdplasmidconc1to1/tea4s15w_0_003367.tif", path "C:/Analysis_from_Movie_for_RiboTrap_Dieter/Movie_Data_Lorenz/TPA-3rdplasmidconc1to1/tea4s15w_0_003368.tif", path "C:/Analysis_from_Movie_for_RiboTrap_Dieter/Movie_Data_Lorenz/TPA-3rdplasmidconc1to1/tea4s15w_0_003369.tif", path "C:/Analysis_from_Movie_for_RiboTrap_Dieter/Movie_Data_Lorenz/TPA-3rdplasmidconc1to1/tea4s15w_0_003370.tif", path "C:/Analysis_from_Movie_for_RiboTrap_Dieter/Movie_Data_Lorenz/TPA-3rdplasmidconc1to1/tea4s15w_0_003371.tif", path "C:/Analysis_from_Movie_for_RiboTrap_Dieter/Movie_Data_Lorenz/TPA-3rdplasmidconc1to1/tea4s15w_0_003372.tif", path "C:/Analysis_from_Movie_for_RiboTrap_Dieter/Movie_Data_Lorenz/TPA-3rdplasmidconc1to1/tea4s15w_0_003373.tif", path "C:/Analysis_from_Movie_for_RiboTrap_Dieter/Movie_Data_Lorenz/TPA-3rdplasmidconc1to1/tea4s15w_0_003374.tif", path "C:/Analysis_from_Movie_for_RiboTrap_Dieter/Movie_Data_Lorenz/TPA-3rdplasmidconc1to1/tea4s15w_0_003375.tif", path "C:/Analysis_from_Movie_for_RiboTrap_Dieter/Movie_Data_Lorenz/TPA-3rdplasmidconc1to1/tea4s15w_0_003376.tif", path "C:/Analysis_from_Movie_for_RiboTrap_Dieter/Movie_Data_Lorenz/TPA-3rdplasmidconc1to1/tea4s15w_0_003377.tif", path "C:/Analysis_from_Movie_for_RiboTrap_Dieter/Movie_Data_Lorenz/TPA-3rdplasmidconc1to1/tea4s15w_0_003378.tif", path "C:/Analysis_from_Movie_for_RiboTrap_Dieter/Movie_Data_Lorenz/TPA-3rdplasmidconc1to1/tea4s15w_0_003379.tif", path "C:/Analysis_from_Movie_for_RiboTrap_Dieter/Movie_Data_Lorenz/TPA-3rdplasmidconc1to1/tea4s15w_0_003380.tif", path "C:/Analysis_from_Movie_for_RiboTrap_Dieter/Movie_Data_Lorenz/TPA-3rdplasmidconc1to1/tea4s15w_0_003381.tif", path "C:/Analysis_from_Movie_for_RiboTrap_Dieter/Movie_Data_Lorenz/TPA-3rdplasmidconc1to1/tea4s15w_0_003382.tif", path "C:/Analysis_from_Movie_for_RiboTrap_Dieter/Movie_Data_Lorenz/TPA-3rdplasmidconc1to1/tea4s15w_0_003383.tif", path "C:/Analysis_from_Movie_for_RiboTrap_Dieter/Movie_Data_Lorenz/TPA-3rdplasmidconc1to1/tea4s15w_0_003384.tif", path "C:/Analysis_from_Movie_for_RiboTrap_Dieter/Movie_Data_Lorenz/TPA-3rdplasmidconc1to1/tea4s15w_0_003385.tif", path "C:/Analysis_from_Movie_for_RiboTrap_Dieter/Movie_Data_Lorenz/TPA-3rdplasmidconc1to1/tea4s15w_0_003386.tif", path "C:/Analysis_from_Movie_for_RiboTrap_Dieter/Movie_Data_Lorenz/TPA-3rdplasmidconc1to1/tea4s15w_0_003387.tif", path "C:/Analysis_from_Movie_for_RiboTrap_Dieter/Movie_Data_Lorenz/TPA-3rdplasmidconc1to1/tea4s15w_0_003388.tif", path "C:/Analysis_from_Movie_for_RiboTrap_Dieter/Movie_Data_Lorenz/TPA-3rdplasmidconc1to1/tea4s15w_0_003389.tif", path "C:/Analysis_from_Movie_for_RiboTrap_Dieter/Movie_Data_Lorenz/TPA-3rdplasmidconc1to1/tea4s15w_0_003390.tif", path "C:/Analysis_from_Movie_for_RiboTrap_Dieter/Movie_Data_Lorenz/TPA-3rdplasmidconc1to1/tea4s15w_0_003391.tif", path "C:/Analysis_from_Movie_for_RiboTrap_Dieter/Movie_Data_Lorenz/TPA-3rdplasmidconc1to1/tea4s15w_0_003392.tif", path "C:/Analysis_from_Movie_for_RiboTrap_Dieter/Movie_Data_Lorenz/TPA-3rdplasmidconc1to1/tea4s15w_0_003393.tif", path "C:/Analysis_from_Movie_for_RiboTrap_Dieter/Movie_Data_Lorenz/TPA-3rdplasmidconc1to1/tea4s15w_0_003394.tif", path "C:/Analysis_from_Movie_for_RiboTrap_Dieter/Movie_Data_Lorenz/TPA-3rdplasmidconc1to1/tea4s15w_0_003395.tif", path "C:/Analysis_from_Movie_for_RiboTrap_Dieter/Movie_Data_Lorenz/TPA-3rdplasmidconc1to1/tea4s15w_0_003396.tif", path "C:/Analysis_from_Movie_for_RiboTrap_Dieter/Movie_Data_Lorenz/TPA-3rdplasmidconc1to1/tea4s15w_0_003397.tif", path "C:/Analysis_from_Movie_for_RiboTrap_Dieter/Movie_Data_Lorenz/TPA-3rdplasmidconc1to1/tea4s15w_0_003398.tif", path "C:/Analysis_from_Movie_for_RiboTrap_Dieter/Movie_Data_Lorenz/TPA-3rdplasmidconc1to1/tea4s15w_0_003399.tif", path "C:/Analysis_from_Movie_for_RiboTrap_Dieter/Movie_Data_Lorenz/TPA-3rdplasmidconc1to1/tea4s15w_0_003400.tif", path "C:/Analysis_from_Movie_for_RiboTrap_Dieter/Movie_Data_Lorenz/TPA-3rdplasmidconc1to1/tea4s15w_0_003401.tif", path "C:/Analysis_from_Movie_for_RiboTrap_Dieter/Movie_Data_Lorenz/TPA-3rdplasmidconc1to1/tea4s15w_0_003402.tif", path "C:/Analysis_from_Movie_for_RiboTrap_Dieter/Movie_Data_Lorenz/TPA-3rdplasmidconc1to1/tea4s15w_0_003403.tif", path "C:/Analysis_from_Movie_for_RiboTrap_Dieter/Movie_Data_Lorenz/TPA-3rdplasmidconc1to1/tea4s15w_0_003404.tif", path "C:/Analysis_from_Movie_for_RiboTrap_Dieter/Movie_Data_Lorenz/TPA-3rdplasmidconc1to1/tea4s15w_0_003405.tif", path "C:/Analysis_from_Movie_for_RiboTrap_Dieter/Movie_Data_Lorenz/TPA-3rdplasmidconc1to1/tea4s15w_0_003406.tif", path "C:/Analysis_from_Movie_for_RiboTrap_Dieter/Movie_Data_Lorenz/TPA-3rdplasmidconc1to1/tea4s15w_0_003407.tif", path "C:/Analysis_from_Movie_for_RiboTrap_Dieter/Movie_Data_Lorenz/TPA-3rdplasmidconc1to1/tea4s15w_0_003408.tif", path "C:/Analysis_from_Movie_for_RiboTrap_Dieter/Movie_Data_Lorenz/TPA-3rdplasmidconc1to1/tea4s15w_0_003409.tif", path "C:/Analysis_from_Movie_for_RiboTrap_Dieter/Movie_Data_Lorenz/TPA-3rdplasmidconc1to1/tea4s15w_0_003410.tif", path "C:/Analysis_from_Movie_for_RiboTrap_Dieter/Movie_Data_Lorenz/TPA-3rdplasmidconc1to1/tea4s15w_0_003411.tif", path "C:/Analysis_from_Movie_for_RiboTrap_Dieter/Movie_Data_Lorenz/TPA-3rdplasmidconc1to1/tea4s15w_0_003412.tif", path "C:/Analysis_from_Movie_for_RiboTrap_Dieter/Movie_Data_Lorenz/TPA-3rdplasmidconc1to1/tea4s15w_0_003413.tif", path "C:/Analysis_from_Movie_for_RiboTrap_Dieter/Movie_Data_Lorenz/TPA-3rdplasmidconc1to1/tea4s15w_0_003414.tif", path "C:/Analysis_from_Movie_for_RiboTrap_Dieter/Movie_Data_Lorenz/TPA-3rdplasmidconc1to1/tea4s15w_0_003415.tif", path "C:/Analysis_from_Movie_for_RiboTrap_Dieter/Movie_Data_Lorenz/TPA-3rdplasmidconc1to1/tea4s15w_0_003416.tif", path "C:/Analysis_from_Movie_for_RiboTrap_Dieter/Movie_Data_Lorenz/TPA-3rdplasmidconc1to1/tea4s15w_0_003417.tif", path "C:/Analysis_from_Movie_for_RiboTrap_Dieter/Movie_Data_Lorenz/TPA-3rdplasmidconc1to1/tea4s15w_0_003418.tif", path "C:/Analysis_from_Movie_for_RiboTrap_Dieter/Movie_Data_Lorenz/TPA-3rdplasmidconc1to1/tea4s15w_0_003419.tif", path "C:/Analysis_from_Movie_for_RiboTrap_Dieter/Movie_Data_Lorenz/TPA-3rdplasmidconc1to1/tea4s15w_0_003420.tif", path "C:/Analysis_from_Movie_for_RiboTrap_Dieter/Movie_Data_Lorenz/TPA-3rdplasmidconc1to1/tea4s15w_0_003421.tif", path "C:/Analysis_from_Movie_for_RiboTrap_Dieter/Movie_Data_Lorenz/TPA-3rdplasmidconc1to1/tea4s15w_0_003422.tif", path "C:/Analysis_from_Movie_for_RiboTrap_Dieter/Movie_Data_Lorenz/TPA-3rdplasmidconc1to1/tea4s15w_0_003423.tif", path "C:/Analysis_from_Movie_for_RiboTrap_Dieter/Movie_Data_Lorenz/TPA-3rdplasmidconc1to1/tea4s15w_0_003424.tif", path "C:/Analysis_from_Movie_for_RiboTrap_Dieter/Movie_Data_Lorenz/TPA-3rdplasmidconc1to1/tea4s15w_0_003425.tif", path "C:/Analysis_from_Movie_for_RiboTrap_Dieter/Movie_Data_Lorenz/TPA-3rdplasmidconc1to1/tea4s15w_0_003426.tif", path "C:/Analysis_from_Movie_for_RiboTrap_Dieter/Movie_Data_Lorenz/TPA-3rdplasmidconc1to1/tea4s15w_0_003427.tif", path "C:/Analysis_from_Movie_for_RiboTrap_Dieter/Movie_Data_Lorenz/TPA-3rdplasmidconc1to1/tea4s15w_0_003428.tif", path "C:/Analysis_from_Movie_for_RiboTrap_Dieter/Movie_Data_Lorenz/TPA-3rdplasmidconc1to1/tea4s15w_0_003429.tif", path "C:/Analysis_from_Movie_for_RiboTrap_Dieter/Movie_Data_Lorenz/TPA-3rdplasmidconc1to1/tea4s15w_0_003430.tif", path "C:/Analysis_from_Movie_for_RiboTrap_Dieter/Movie_Data_Lorenz/TPA-3rdplasmidconc1to1/tea4s15w_0_003431.tif", path "C:/Analysis_from_Movie_for_RiboTrap_Dieter/Movie_Data_Lorenz/TPA-3rdplasmidconc1to1/tea4s15w_0_003432.tif", path "C:/Analysis_from_Movie_for_RiboTrap_Dieter/Movie_Data_Lorenz/TPA-3rdplasmidconc1to1/tea4s15w_0_003433.tif", path "C:/Analysis_from_Movie_for_RiboTrap_Dieter/Movie_Data_Lorenz/TPA-3rdplasmidconc1to1/tea4s15w_0_003434.tif", path "C:/Analysis_from_Movie_for_RiboTrap_Dieter/Movie_Data_Lorenz/TPA-3rdplasmidconc1to1/tea4s15w_0_003435.tif", path "C:/Analysis_from_Movie_for_RiboTrap_Dieter/Movie_Data_Lorenz/TPA-3rdplasmidconc1to1/tea4s15w_0_003436.tif", path "C:/Analysis_from_Movie_for_RiboTrap_Dieter/Movie_Data_Lorenz/TPA-3rdplasmidconc1to1/tea4s15w_0_003437.tif", path "C:/Analysis_from_Movie_for_RiboTrap_Dieter/Movie_Data_Lorenz/TPA-3rdplasmidconc1to1/tea4s15w_0_003438.tif", path "C:/Analysis_from_Movie_for_RiboTrap_Dieter/Movie_Data_Lorenz/TPA-3rdplasmidconc1to1/tea4s15w_0_003439.tif", path "C:/Analysis_from_Movie_for_RiboTrap_Dieter/Movie_Data_Lorenz/TPA-3rdplasmidconc1to1/tea4s15w_0_003440.tif", path "C:/Analysis_from_Movie_for_RiboTrap_Dieter/Movie_Data_Lorenz/TPA-3rdplasmidconc1to1/tea4s15w_0_003441.tif", path "C:/Analysis_from_Movie_for_RiboTrap_Dieter/Movie_Data_Lorenz/TPA-3rdplasmidconc1to1/tea4s15w_0_003442.tif", path "C:/Analysis_from_Movie_for_RiboTrap_Dieter/Movie_Data_Lorenz/TPA-3rdplasmidconc1to1/tea4s15w_0_003443.tif", path "C:/Analysis_from_Movie_for_RiboTrap_Dieter/Movie_Data_Lorenz/TPA-3rdplasmidconc1to1/tea4s15w_0_003444.tif", path "C:/Analysis_from_Movie_for_RiboTrap_Dieter/Movie_Data_Lorenz/TPA-3rdplasmidconc1to1/tea4s15w_0_003445.tif", path "C:/Analysis_from_Movie_for_RiboTrap_Dieter/Movie_Data_Lorenz/TPA-3rdplasmidconc1to1/tea4s15w_0_003446.tif", path "C:/Analysis_from_Movie_for_RiboTrap_Dieter/Movie_Data_Lorenz/TPA-3rdplasmidconc1to1/tea4s15w_0_003447.tif", path "C:/Analysis_from_Movie_for_RiboTrap_Dieter/Movie_Data_Lorenz/TPA-3rdplasmidconc1to1/tea4s15w_0_003448.tif", path "C:/Analysis_from_Movie_for_RiboTrap_Dieter/Movie_Data_Lorenz/TPA-3rdplasmidconc1to1/tea4s15w_0_003449.tif", path "C:/Analysis_from_Movie_for_RiboTrap_Dieter/Movie_Data_Lorenz/TPA-3rdplasmidconc1to1/tea4s15w_0_003450.tif", path "C:/Analysis_from_Movie_for_RiboTrap_Dieter/Movie_Data_Lorenz/TPA-3rdplasmidconc1to1/tea4s15w_0_003451.tif", path "C:/Analysis_from_Movie_for_RiboTrap_Dieter/Movie_Data_Lorenz/TPA-3rdplasmidconc1to1/tea4s15w_0_003452.tif", path "C:/Analysis_from_Movie_for_RiboTrap_Dieter/Movie_Data_Lorenz/TPA-3rdplasmidconc1to1/tea4s15w_0_003453.tif", path "C:/Analysis_from_Movie_for_RiboTrap_Dieter/Movie_Data_Lorenz/TPA-3rdplasmidconc1to1/tea4s15w_0_003454.tif", path "C:/Analysis_from_Movie_for_RiboTrap_Dieter/Movie_Data_Lorenz/TPA-3rdplasmidconc1to1/tea4s15w_0_003455.tif", path "C:/Analysis_from_Movie_for_RiboTrap_Dieter/Movie_Data_Lorenz/TPA-3rdplasmidconc1to1/tea4s15w_0_003456.tif", path "C:/Analysis_from_Movie_for_RiboTrap_Dieter/Movie_Data_Lorenz/TPA-3rdplasmidconc1to1/tea4s15w_0_003457.tif", path "C:/Analysis_from_Movie_for_RiboTrap_Dieter/Movie_Data_Lorenz/TPA-3rdplasmidconc1to1/tea4s15w_0_003458.tif", path "C:/Analysis_from_Movie_for_RiboTrap_Dieter/Movie_Data_Lorenz/TPA-3rdplasmidconc1to1/tea4s15w_0_003459.tif", path "C:/Analysis_from_Movie_for_RiboTrap_Dieter/Movie_Data_Lorenz/TPA-3rdplasmidconc1to1/tea4s15w_0_003460.tif", path "C:/Analysis_from_Movie_for_RiboTrap_Dieter/Movie_Data_Lorenz/TPA-3rdplasmidconc1to1/tea4s15w_0_003461.tif", path "C:/Analysis_from_Movie_for_RiboTrap_Dieter/Movie_Data_Lorenz/TPA-3rdplasmidconc1to1/tea4s15w_0_003462.tif", path "C:/Analysis_from_Movie_for_RiboTrap_Dieter/Movie_Data_Lorenz/TPA-3rdplasmidconc1to1/tea4s15w_0_003463.tif", path "C:/Analysis_from_Movie_for_RiboTrap_Dieter/Movie_Data_Lorenz/TPA-3rdplasmidconc1to1/tea4s15w_0_003464.tif", path "C:/Analysis_from_Movie_for_RiboTrap_Dieter/Movie_Data_Lorenz/TPA-3rdplasmidconc1to1/tea4s15w_0_003465.tif", path "C:/Analysis_from_Movie_for_RiboTrap_Dieter/Movie_Data_Lorenz/TPA-3rdplasmidconc1to1/tea4s15w_0_003466.tif", path "C:/Analysis_from_Movie_for_RiboTrap_Dieter/Movie_Data_Lorenz/TPA-3rdplasmidconc1to1/tea4s15w_0_003467.tif", path "C:/Analysis_from_Movie_for_RiboTrap_Dieter/Movie_Data_Lorenz/TPA-3rdplasmidconc1to1/tea4s15w_0_003468.tif", path "C:/Analysis_from_Movie_for_RiboTrap_Dieter/Movie_Data_Lorenz/TPA-3rdplasmidconc1to1/tea4s15w_0_003469.tif", path "C:/Analysis_from_Movie_for_RiboTrap_Dieter/Movie_Data_Lorenz/TPA-3rdplasmidconc1to1/tea4s15w_0_003470.tif", path "C:/Analysis_from_Movie_for_RiboTrap_Dieter/Movie_Data_Lorenz/TPA-3rdplasmidconc1to1/tea4s15w_0_003471.tif", path "C:/Analysis_from_Movie_for_RiboTrap_Dieter/Movie_Data_Lorenz/TPA-3rdplasmidconc1to1/tea4s15w_0_003472.tif", path "C:/Analysis_from_Movie_for_RiboTrap_Dieter/Movie_Data_Lorenz/TPA-3rdplasmidconc1to1/tea4s15w_0_003473.tif", path "C:/Analysis_from_Movie_for_RiboTrap_Dieter/Movie_Data_Lorenz/TPA-3rdplasmidconc1to1/tea4s15w_0_003474.tif", path "C:/Analysis_from_Movie_for_RiboTrap_Dieter/Movie_Data_Lorenz/TPA-3rdplasmidconc1to1/tea4s15w_0_003475.tif", path "C:/Analysis_from_Movie_for_RiboTrap_Dieter/Movie_Data_Lorenz/TPA-3rdplasmidconc1to1/tea4s15w_0_003476.tif", path "C:/Analysis_from_Movie_for_RiboTrap_Dieter/Movie_Data_Lorenz/TPA-3rdplasmidconc1to1/tea4s15w_0_003477.tif", path "C:/Analysis_from_Movie_for_RiboTrap_Dieter/Movie_Data_Lorenz/TPA-3rdplasmidconc1to1/tea4s15w_0_003478.tif", path "C:/Analysis_from_Movie_for_RiboTrap_Dieter/Movie_Data_Lorenz/TPA-3rdplasmidconc1to1/tea4s15w_0_003479.tif", path "C:/Analysis_from_Movie_for_RiboTrap_Dieter/Movie_Data_Lorenz/TPA-3rdplasmidconc1to1/tea4s15w_0_003480.tif", path "C:/Analysis_from_Movie_for_RiboTrap_Dieter/Movie_Data_Lorenz/TPA-3rdplasmidconc1to1/tea4s15w_0_003481.tif", path "C:/Analysis_from_Movie_for_RiboTrap_Dieter/Movie_Data_Lorenz/TPA-3rdplasmidconc1to1/tea4s15w_0_003482.tif", path "C:/Analysis_from_Movie_for_RiboTrap_Dieter/Movie_Data_Lorenz/TPA-3rdplasmidconc1to1/tea4s15w_0_003483.tif", path "C:/Analysis_from_Movie_for_RiboTrap_Dieter/Movie_Data_Lorenz/TPA-3rdplasmidconc1to1/tea4s15w_0_003484.tif", path "C:/Analysis_from_Movie_for_RiboTrap_Dieter/Movie_Data_Lorenz/TPA-3rdplasmidconc1to1/tea4s15w_0_003485.tif", path "C:/Analysis_from_Movie_for_RiboTrap_Dieter/Movie_Data_Lorenz/TPA-3rdplasmidconc1to1/tea4s15w_0_003486.tif", path "C:/Analysis_from_Movie_for_RiboTrap_Dieter/Movie_Data_Lorenz/TPA-3rdplasmidconc1to1/tea4s15w_0_003487.tif", path "C:/Analysis_from_Movie_for_RiboTrap_Dieter/Movie_Data_Lorenz/TPA-3rdplasmidconc1to1/tea4s15w_0_003488.tif", path "C:/Analysis_from_Movie_for_RiboTrap_Dieter/Movie_Data_Lorenz/TPA-3rdplasmidconc1to1/tea4s15w_0_003489.tif", path "C:/Analysis_from_Movie_for_RiboTrap_Dieter/Movie_Data_Lorenz/TPA-3rdplasmidconc1to1/tea4s15w_0_003490.tif", path "C:/Analysis_from_Movie_for_RiboTrap_Dieter/Movie_Data_Lorenz/TPA-3rdplasmidconc1to1/tea4s15w_0_003491.tif", path "C:/Analysis_from_Movie_for_RiboTrap_Dieter/Movie_Data_Lorenz/TPA-3rdplasmidconc1to1/tea4s15w_0_003492.tif", path "C:/Analysis_from_Movie_for_RiboTrap_Dieter/Movie_Data_Lorenz/TPA-3rdplasmidconc1to1/tea4s15w_0_003493.tif", path "C:/Analysis_from_Movie_for_RiboTrap_Dieter/Movie_Data_Lorenz/TPA-3rdplasmidconc1to1/tea4s15w_0_003494.tif", path "C:/Analysis_from_Movie_for_RiboTrap_Dieter/Movie_Data_Lorenz/TPA-3rdplasmidconc1to1/tea4s15w_0_003495.tif", path "C:/Analysis_from_Movie_for_RiboTrap_Dieter/Movie_Data_Lorenz/TPA-3rdplasmidconc1to1/tea4s15w_0_003496.tif", path "C:/Analysis_from_Movie_for_RiboTrap_Dieter/Movie_Data_Lorenz/TPA-3rdplasmidconc1to1/tea4s15w_0_003497.tif", path "C:/Analysis_from_Movie_for_RiboTrap_Dieter/Movie_Data_Lorenz/TPA-3rdplasmidconc1to1/tea4s15w_0_003498.tif", path "C:/Analysis_from_Movie_for_RiboTrap_Dieter/Movie_Data_Lorenz/TPA-3rdplasmidconc1to1/tea4s15w_0_003499.tif", path "C:/Analysis_from_Movie_for_RiboTrap_Dieter/Movie_Data_Lorenz/TPA-3rdplasmidconc1to1/tea4s15w_0_003500.tif", path "C:/Analysis_from_Movie_for_RiboTrap_Dieter/Movie_Data_Lorenz/TPA-3rdplasmidconc1to1/tea4s15w_0_003501.tif", path "C:/Analysis_from_Movie_for_RiboTrap_Dieter/Movie_Data_Lorenz/TPA-3rdplasmidconc1to1/tea4s15w_0_003502.tif", path "C:/Analysis_from_Movie_for_RiboTrap_Dieter/Movie_Data_Lorenz/TPA-3rdplasmidconc1to1/tea4s15w_0_003503.tif", path "C:/Analysis_from_Movie_for_RiboTrap_Dieter/Movie_Data_Lorenz/TPA-3rdplasmidconc1to1/tea4s15w_0_003504.tif", path "C:/Analysis_from_Movie_for_RiboTrap_Dieter/Movie_Data_Lorenz/TPA-3rdplasmidconc1to1/tea4s15w_0_003505.tif", path "C:/Analysis_from_Movie_for_RiboTrap_Dieter/Movie_Data_Lorenz/TPA-3rdplasmidconc1to1/tea4s15w_0_003506.tif", path "C:/Analysis_from_Movie_for_RiboTrap_Dieter/Movie_Data_Lorenz/TPA-3rdplasmidconc1to1/tea4s15w_0_003507.tif", path "C:/Analysis_from_Movie_for_RiboTrap_Dieter/Movie_Data_Lorenz/TPA-3rdplasmidconc1to1/tea4s15w_0_003508.tif", path "C:/Analysis_from_Movie_for_RiboTrap_Dieter/Movie_Data_Lorenz/TPA-3rdplasmidconc1to1/tea4s15w_0_003509.tif", path "C:/Analysis_from_Movie_for_RiboTrap_Dieter/Movie_Data_Lorenz/TPA-3rdplasmidconc1to1/tea4s15w_0_003510.tif", path "C:/Analysis_from_Movie_for_RiboTrap_Dieter/Movie_Data_Lorenz/TPA-3rdplasmidconc1to1/tea4s15w_0_003511.tif", path "C:/Analysis_from_Movie_for_RiboTrap_Dieter/Movie_Data_Lorenz/TPA-3rdplasmidconc1to1/tea4s15w_0_003512.tif", path "C:/Analysis_from_Movie_for_RiboTrap_Dieter/Movie_Data_Lorenz/TPA-3rdplasmidconc1to1/tea4s15w_0_003513.tif", path "C:/Analysis_from_Movie_for_RiboTrap_Dieter/Movie_Data_Lorenz/TPA-3rdplasmidconc1to1/tea4s15w_0_003514.tif", path "C:/Analysis_from_Movie_for_RiboTrap_Dieter/Movie_Data_Lorenz/TPA-3rdplasmidconc1to1/tea4s15w_0_003515.tif", path "C:/Analysis_from_Movie_for_RiboTrap_Dieter/Movie_Data_Lorenz/TPA-3rdplasmidconc1to1/tea4s15w_0_003516.tif", path "C:/Analysis_from_Movie_for_RiboTrap_Dieter/Movie_Data_Lorenz/TPA-3rdplasmidconc1to1/tea4s15w_0_003517.tif", path "C:/Analysis_from_Movie_for_RiboTrap_Dieter/Movie_Data_Lorenz/TPA-3rdplasmidconc1to1/tea4s15w_0_003518.tif", path "C:/Analysis_from_Movie_for_RiboTrap_Dieter/Movie_Data_Lorenz/TPA-3rdplasmidconc1to1/tea4s15w_0_003519.tif", path "C:/Analysis_from_Movie_for_RiboTrap_Dieter/Movie_Data_Lorenz/TPA-3rdplasmidconc1to1/tea4s15w_0_003520.tif", path "C:/Analysis_from_Movie_for_RiboTrap_Dieter/Movie_Data_Lorenz/TPA-3rdplasmidconc1to1/tea4s15w_0_003521.tif", path "C:/Analysis_from_Movie_for_RiboTrap_Dieter/Movie_Data_Lorenz/TPA-3rdplasmidconc1to1/tea4s15w_0_003522.tif", path "C:/Analysis_from_Movie_for_RiboTrap_Dieter/Movie_Data_Lorenz/TPA-3rdplasmidconc1to1/tea4s15w_0_003523.tif", path "C:/Analysis_from_Movie_for_RiboTrap_Dieter/Movie_Data_Lorenz/TPA-3rdplasmidconc1to1/tea4s15w_0_003524.tif", path "C:/Analysis_from_Movie_for_RiboTrap_Dieter/Movie_Data_Lorenz/TPA-3rdplasmidconc1to1/tea4s15w_0_003525.tif", path "C:/Analysis_from_Movie_for_RiboTrap_Dieter/Movie_Data_Lorenz/TPA-3rdplasmidconc1to1/tea4s15w_0_003526.tif", path "C:/Analysis_from_Movie_for_RiboTrap_Dieter/Movie_Data_Lorenz/TPA-3rdplasmidconc1to1/tea4s15w_0_003527.tif", path "C:/Analysis_from_Movie_for_RiboTrap_Dieter/Movie_Data_Lorenz/TPA-3rdplasmidconc1to1/tea4s15w_0_003528.tif", path "C:/Analysis_from_Movie_for_RiboTrap_Dieter/Movie_Data_Lorenz/TPA-3rdplasmidconc1to1/tea4s15w_0_003529.tif", path "C:/Analysis_from_Movie_for_RiboTrap_Dieter/Movie_Data_Lorenz/TPA-3rdplasmidconc1to1/tea4s15w_0_003530.tif", path "C:/Analysis_from_Movie_for_RiboTrap_Dieter/Movie_Data_Lorenz/TPA-3rdplasmidconc1to1/tea4s15w_0_003531.tif", path "C:/Analysis_from_Movie_for_RiboTrap_Dieter/Movie_Data_Lorenz/TPA-3rdplasmidconc1to1/tea4s15w_0_003532.tif", path "C:/Analysis_from_Movie_for_RiboTrap_Dieter/Movie_Data_Lorenz/TPA-3rdplasmidconc1to1/tea4s15w_0_003533.tif", path "C:/Analysis_from_Movie_for_RiboTrap_Dieter/Movie_Data_Lorenz/TPA-3rdplasmidconc1to1/tea4s15w_0_003534.tif", path "C:/Analysis_from_Movie_for_RiboTrap_Dieter/Movie_Data_Lorenz/TPA-3rdplasmidconc1to1/tea4s15w_0_003535.tif", path "C:/Analysis_from_Movie_for_RiboTrap_Dieter/Movie_Data_Lorenz/TPA-3rdplasmidconc1to1/tea4s15w_0_003536.tif", path "C:/Analysis_from_Movie_for_RiboTrap_Dieter/Movie_Data_Lorenz/TPA-3rdplasmidconc1to1/tea4s15w_0_003537.tif", path "C:/Analysis_from_Movie_for_RiboTrap_Dieter/Movie_Data_Lorenz/TPA-3rdplasmidconc1to1/tea4s15w_0_003538.tif", path "C:/Analysis_from_Movie_for_RiboTrap_Dieter/Movie_Data_Lorenz/TPA-3rdplasmidconc1to1/tea4s15w_0_003539.tif", path "C:/Analysis_from_Movie_for_RiboTrap_Dieter/Movie_Data_Lorenz/TPA-3rdplasmidconc1to1/tea4s15w_0_003540.tif", path "C:/Analysis_from_Movie_for_RiboTrap_Dieter/Movie_Data_Lorenz/TPA-3rdplasmidconc1to1/tea4s15w_0_003541.tif", path "C:/Analysis_from_Movie_for_RiboTrap_Dieter/Movie_Data_Lorenz/TPA-3rdplasmidconc1to1/tea4s15w_0_003542.tif", path "C:/Analysis_from_Movie_for_RiboTrap_Dieter/Movie_Data_Lorenz/TPA-3rdplasmidconc1to1/tea4s15w_0_003543.tif", path "C:/Analysis_from_Movie_for_RiboTrap_Dieter/Movie_Data_Lorenz/TPA-3rdplasmidconc1to1/tea4s15w_0_003544.tif", path "C:/Analysis_from_Movie_for_RiboTrap_Dieter/Movie_Data_Lorenz/TPA-3rdplasmidconc1to1/tea4s15w_0_003545.tif", path "C:/Analysis_from_Movie_for_RiboTrap_Dieter/Movie_Data_Lorenz/TPA-3rdplasmidconc1to1/tea4s15w_0_003546.tif", path "C:/Analysis_from_Movie_for_RiboTrap_Dieter/Movie_Data_Lorenz/TPA-3rdplasmidconc1to1/tea4s15w_0_003547.tif", path "C:/Analysis_from_Movie_for_RiboTrap_Dieter/Movie_Data_Lorenz/TPA-3rdplasmidconc1to1/tea4s15w_0_003548.tif", path "C:/Analysis_from_Movie_for_RiboTrap_Dieter/Movie_Data_Lorenz/TPA-3rdplasmidconc1to1/tea4s15w_0_003549.tif", path "C:/Analysis_from_Movie_for_RiboTrap_Dieter/Movie_Data_Lorenz/TPA-3rdplasmidconc1to1/tea4s15w_0_003550.tif", path "C:/Analysis_from_Movie_for_RiboTrap_Dieter/Movie_Data_Lorenz/TPA-3rdplasmidconc1to1/tea4s15w_0_003551.tif", path "C:/Analysis_from_Movie_for_RiboTrap_Dieter/Movie_Data_Lorenz/TPA-3rdplasmidconc1to1/tea4s15w_0_003552.tif", path "C:/Analysis_from_Movie_for_RiboTrap_Dieter/Movie_Data_Lorenz/TPA-3rdplasmidconc1to1/tea4s15w_0_003553.tif", path "C:/Analysis_from_Movie_for_RiboTrap_Dieter/Movie_Data_Lorenz/TPA-3rdplasmidconc1to1/tea4s15w_0_003554.tif", path "C:/Analysis_from_Movie_for_RiboTrap_Dieter/Movie_Data_Lorenz/TPA-3rdplasmidconc1to1/tea4s15w_0_003555.tif", path "C:/Analysis_from_Movie_for_RiboTrap_Dieter/Movie_Data_Lorenz/TPA-3rdplasmidconc1to1/tea4s15w_0_003556.tif", path "C:/Analysis_from_Movie_for_RiboTrap_Dieter/Movie_Data_Lorenz/TPA-3rdplasmidconc1to1/tea4s15w_0_003557.tif", path "C:/Analysis_from_Movie_for_RiboTrap_Dieter/Movie_Data_Lorenz/TPA-3rdplasmidconc1to1/tea4s15w_0_003558.tif", path "C:/Analysis_from_Movie_for_RiboTrap_Dieter/Movie_Data_Lorenz/TPA-3rdplasmidconc1to1/tea4s15w_0_003559.tif", path "C:/Analysis_from_Movie_for_RiboTrap_Dieter/Movie_Data_Lorenz/TPA-3rdplasmidconc1to1/tea4s15w_0_003560.tif", path "C:/Analysis_from_Movie_for_RiboTrap_Dieter/Movie_Data_Lorenz/TPA-3rdplasmidconc1to1/tea4s15w_0_003561.tif", path "C:/Analysis_from_Movie_for_RiboTrap_Dieter/Movie_Data_Lorenz/TPA-3rdplasmidconc1to1/tea4s15w_0_003562.tif", path "C:/Analysis_from_Movie_for_RiboTrap_Dieter/Movie_Data_Lorenz/TPA-3rdplasmidconc1to1/tea4s15w_0_003563.tif", path "C:/Analysis_from_Movie_for_RiboTrap_Dieter/Movie_Data_Lorenz/TPA-3rdplasmidconc1to1/tea4s15w_0_003564.tif", path "C:/Analysis_from_Movie_for_RiboTrap_Dieter/Movie_Data_Lorenz/TPA-3rdplasmidconc1to1/tea4s15w_0_003565.tif"], 3 "Film length":i32=1467)   [LabVIEW 2014]
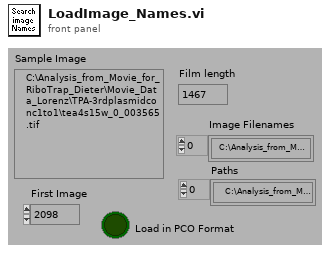
[diagram p1: front panel]
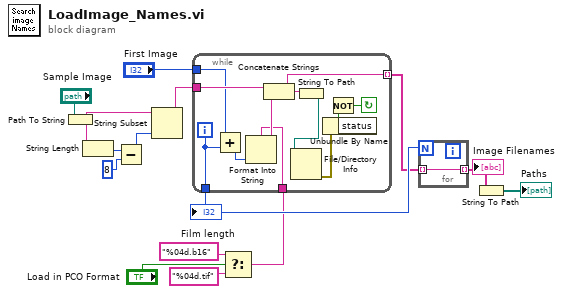
[diagram p0: block diagram]
diagram:
  n1 = Path To String(path="Sample Image") -> (string=w10:string)
  n2 = String Length(string=w10) -> (length=w13:i32)
  n3 = Subtract(x=w13, y=8) -> (x-y=w11:i32)
  n4 = String Subset(string=w10, length (rest)=w11) -> (substring=w9:string)  [unwired: 1 in]
  n5 = Select(t="%04d.b16", s="Load in PCO Format", f="%04d.tif" ("Format String")) -> (s? t:f=w1:string)
  n6 = while {
    tunnel: "First Image" -> [w20]
    tunnel: [w22] -> w8 mode=indexing
    tunnel: w9 -> [w24]
    tunnel: [w16] -> w15
    tunnel: w1 -> [w17]
    i -> [w16]
    stop <- w25 continue-if-true
    n7 = Add(x=w20, y=w16) -> (x+y=w21:i32)
    n8 = Format Into String(format string=w17, w21) -> (resulting string=w23:string)  [unwired: 2 in, 1 out]
    n9 = Concatenate Strings(w24, w23) -> (w22:string)
    n10 = String To Path(string=w22) -> (path=w18:path)
    n11 = File/Directory Info(path=w18) -> (error out=w19:errorcluster)  [unwired: 1 in, 6 out]
    n12 = Unbundle By Name(w19) -> ("status"=w26:bool)
    n13 = Not(x=w26) -> (.not. x?=w25:bool)
  }
  "Film length" <- w15
  n14 = for {
    N: w15 -> [_]
    tunnel: [w27] -> w7 mode=indexing
    tunnel: w8 -> [w27] mode=indexing
  }
  "Image Filenames" <- w7
  n15 = String To Path(string=w7) -> (path=→"Paths":path[])
